vi "SO-FSRS Analysis 3.0.vi"() -> ()   [LabVIEW 2015]
uses:
  LabView vis/Control 1.ctl
  LabView vis/Control 3.ctl
  <vilib>/Math Plots/3D Math Plots/3D Surface/3D Surface XCtrl/3D Surface.xctl
  <vilib>/Math Plots/3D Math Plots/3D Scatter/3D Scatter XCtrl/3D Scatter.xctl
  <vilib>/gmath/NumericalOptimization/LM model function reference.ctl
  <vilib>/Utility/file.llb/Read Delimited Spreadsheet (DBL).vi
  <vilib>/Math Plots/3D Math Plots/3D Scatter/3D Scatter Datatype/Public/Plot Helper (Matrix).vi
  <vilib>/Math Plots/3D Math Plots/3D Surface/3D Surface Datatype/Public/Plot Helper (Vector).vi
  <vilib>/Utility/file.llb/Write Delimited Spreadsheet (DBL).vi
  <vilib>/gmath/NumericalOptimization/Nonlinear Curve Fit LM.vi
  <vilib>/Math Plots/3D Math Plots/3D Scatter/3D Scatter Datatype/Public/Plot Helper (Vector).vi
  <vilib>/Math Plots/3D Math Plots/3D Surface/3D Surface Datatype/3D Surface Datatype.lvclass
  <vilib>/Math Plots/3D Math Plots/3D Scatter/3D Scatter Datatype/3D Scatter Datatype.lvclass
  <vilib>/gmath/NI_Gmath.lvlib
  <vilib>/Analysis/NI_AALPro.lvlib
panel:
  out "Shiftx":T1=[-400.0, -600.0, -200.0, -2100.0, -10.0, 570.0, 1700.0, 980.0, 10000.0, -1100.0, 150.0, 320.0, -850.0, -1500.0, -5000.0]
  in  "Load shiftx":bool
  in  "error in":errorcluster
  out "error out":errorcluster
  in  "Main Tab":T2(tab)
  in  "Shorter Name":string
  in  "Do it?":bool
  in  "Index":i32
  in  "What you gonna do":u16(ring) items=["Delete", "Flip"]
  in  "Folder - Batch Files":path
  out "Built Arrays":dbl[][](graph)
  in  "?":bool
  in  "File Names":u16(ring) items=["pero_EGF1_h_0_0gr", "pero_EGF1_h_0_1gr", "pero_EGF1_h_0_2gr", "pero_EGF1_h_10_0gr", "pero_EGF1_h_10_1gr", "pero_EGF1_h_10_2gr", "pero_EGF1_h_11_0gr", "pero_EGF1_h_11_1gr", "pero_EGF1_h_11_2gr", "pero_EGF1_h_12_0gr", "pero_EGF1_h_12_1gr", "pero_EGF1_h_12_2gr", "pero_EGF1_h_13_0gr", "pero_EGF1_h_13_1gr", "pero_EGF1_h_13_2gr", "pero_EGF1_h_14_0gr", "pero_EGF1_h_14_1gr", "pero_EGF1_h_14_2gr", "pero_EGF1_h_15_0gr", "pero_EGF1_h_15_1gr", "pero_EGF1_h_15_2gr", "pero_EGF1_h_16_0gr", "pero_EGF1_h_16_1gr", "pero_EGF1_h_16_2gr", "pero_EGF1_h_17_0gr", "pero_EGF1_h_1_0gr", "pero_EGF1_h_1_1gr", "pero_EGF1_h_1_2gr", "pero_EGF1_h_2_0gr", "pero_EGF1_h_2_1gr", "pero_EGF1_h_2_2gr", "pero_EGF1_h_3_0gr", "pero_EGF1_h_3_1gr", "pero_EGF1_h_3_2gr", "pero_EGF1_h_4_0gr", "pero_EGF1_h_4_1gr", "pero_EGF1_h_4_2gr", "pero_EGF1_h_5_0gr", "pero_EGF1_h_5_1gr", "pero_EGF1_h_5_2gr", "pero_EGF1_h_6_0gr", "pero_EGF1_h_6_1gr", "pero_EGF1_h_6_2gr", "pero_EGF1_h_7_0gr", "pero_EGF1_h_7_1gr", "pero_EGF1_h_7_2gr", "pero_EGF1_h_8_0gr", "pero_EGF1_h_8_1gr", "pero_EGF1_h_8_2gr", "pero_EGF1_h_9_0gr", "pero_EGF1_h_9_1gr", "pero_EGF1_h_9_2gr", "pero_EGF1_h_m1m1_m0exe0", "pero_EGF1_h_m1m1_m0exe1", "pero_EGF1_h_m1m1_m0exe10", "pero_EGF1_h_m1m1_m0exe11", "pero_EGF1_h_m1m1_m0exe12", "pero_EGF1_h_m1m1_m0exe13", "pero_EGF1_h_m1m1_m0exe14", "pero_EGF1_h_m1m1_m0exe15", "pero_EGF1_h_m1m1_m0exe16", "pero_EGF1_h_m1m1_m0exe2", "pero_EGF1_h_m1m1_m0exe3", "pero_EGF1_h_m1m1_m0exe4", "pero_EGF1_h_m1m1_m0exe5", "pero_EGF1_h_m1m1_m0exe6", "pero_EGF1_h_m1m1_m0exe7", "pero_EGF1_h_m1m1_m0exe8", "pero_EGF1_h_m1m1_m0exe9", "pero_EGF1_h_m1m1_m100exe0", "pero_EGF1_h_m1m1_m100exe1", "pero_EGF1_h_m1m1_m100exe10", "pero_EGF1_h_m1m1_m100exe11", "pero_EGF1_h_m1m1_m100exe12", "pero_EGF1_h_m1m1_m100exe13", "pero_EGF1_h_m1m1_m100exe14", "pero_EGF1_h_m1m1_m100exe15", "pero_EGF1_h_m1m1_m100exe16", "pero_EGF1_h_m1m1_m100exe2", "pero_EGF1_h_m1m1_m100exe3", "pero_EGF1_h_m1m1_m100exe4", "pero_EGF1_h_m1m1_m100exe5", "pero_EGF1_h_m1m1_m100exe6", "pero_EGF1_h_m1m1_m100exe7", "pero_EGF1_h_m1m1_m100exe8", "pero_EGF1_h_m1m1_m100exe9", "pero_EGF1_h_m1m1_m200exe0", "pero_EGF1_h_m1m1_m200exe1", "pero_EGF1_h_m1m1_m200exe10", "pero_EGF1_h_m1m1_m200exe11", "pero_EGF1_h_m1m1_m200exe12", "pero_EGF1_h_m1m1_m200exe13", "pero_EGF1_h_m1m1_m200exe14", "pero_EGF1_h_m1m1_m200exe15", "pero_EGF1_h_m1m1_m200exe16", "pero_EGF1_h_m1m1_m200exe2", "pero_EGF1_h_m1m1_m200exe3", "pero_EGF1_h_m1m1_m200exe4", "pero_EGF1_h_m1m1_m200exe5", "pero_EGF1_h_m1m1_m200exe6", "pero_EGF1_h_m1m1_m200exe7", "pero_EGF1_h_m1m1_m200exe8", "pero_EGF1_h_m1m1_m200exe9", "pero_EGF1_h_m1m1_m300exe0", "pero_EGF1_h_m1m1_m300exe1", "pero_EGF1_h_m1m1_m300exe10", "pero_EGF1_h_m1m1_m300exe11", "pero_EGF1_h_m1m1_m300exe12", "pero_EGF1_h_m1m1_m300exe13", "pero_EGF1_h_m1m1_m300exe14", "pero_EGF1_h_m1m1_m300exe15", "pero_EGF1_h_m1m1_m300exe16", "pero_EGF1_h_m1m1_m300exe2", "pero_EGF1_h_m1m1_m300exe3", "pero_EGF1_h_m1m1_m300exe4", "pero_EGF1_h_m1m1_m300exe5", "pero_EGF1_h_m1m1_m300exe6", "pero_EGF1_h_m1m1_m300exe7", "pero_EGF1_h_m1m1_m300exe8", "pero_EGF1_h_m1m1_m300exe9", "pero_EGF1_h_m1m1_m5000exe0", "pero_EGF1_h_m1m1_m5000exe1", "pero_EGF1_h_m1m1_m5000exe10", "pero_EGF1_h_m1m1_m5000exe12", "pero_EGF1_h_m1m1_m5000exe13", "pero_EGF1_h_m1m1_m5000exe14", "pero_EGF1_h_m1m1_m5000exe15", "pero_EGF1_h_m1m1_m5000exe16", "pero_EGF1_h_m1m1_m5000exe2", "pero_EGF1_h_m1m1_m5000exe3", "pero_EGF1_h_m1m1_m5000exe4", "pero_EGF1_h_m1m1_m5000exe5", "pero_EGF1_h_m1m1_m5000exe6", "pero_EGF1_h_m1m1_m5000exe7", "pero_EGF1_h_m1m1_m5000exe8", "pero_EGF1_h_m1m1_m5000exe9", "pero_EGF1_h_m1m1_m500exe0", "pero_EGF1_h_m1m1_m500exe1", "pero_EGF1_h_m1m1_m500exe10", "pero_EGF1_h_m1m1_m500exe11", "pero_EGF1_h_m1m1_m500exe12", "pero_EGF1_h_m1m1_m500exe13", "pero_EGF1_h_m1m1_m500exe14", "pero_EGF1_h_m1m1_m500exe15", "pero_EGF1_h_m1m1_m500exe16", "pero_EGF1_h_m1m1_m500exe2", "pero_EGF1_h_m1m1_m500exe3", "pero_EGF1_h_m1m1_m500exe4", "pero_EGF1_h_m1m1_m500exe5", "pero_EGF1_h_m1m1_m500exe6", "pero_EGF1_h_m1m1_m500exe7", "pero_EGF1_h_m1m1_m500exe8", "pero_EGF1_h_m1m1_m500exe9", "pero_EGF1_h_m1m1_p100000exe0", "pero_EGF1_h_m1m1_p100000exe1", "pero_EGF1_h_m1m1_p100000exe10", "pero_EGF1_h_m1m1_p100000exe11", "pero_EGF1_h_m1m1_p100000exe12", "pero_EGF1_h_m1m1_p100000exe13", "pero_EGF1_h_m1m1_p100000exe14", "pero_EGF1_h_m1m1_p100000exe15", "pero_EGF1_h_m1m1_p100000exe16", "pero_EGF1_h_m1m1_p100000exe2", "pero_EGF1_h_m1m1_p100000exe3", "pero_EGF1_h_m1m1_p100000exe4", "pero_EGF1_h_m1m1_p100000exe5", "pero_EGF1_h_m1m1_p100000exe6", "pero_EGF1_h_m1m1_p100000exe7", "pero_EGF1_h_m1m1_p100000exe8", "pero_EGF1_h_m1m1_p100000exe9", "pero_EGF1_h_m1m1_p10000exe0", "pero_EGF1_h_m1m1_p10000exe1", "pero_EGF1_h_m1m1_p10000exe10", "pero_EGF1_h_m1m1_p10000exe11", "pero_EGF1_h_m1m1_p10000exe12", "pero_EGF1_h_m1m1_p10000exe13", "pero_EGF1_h_m1m1_p10000exe14", "pero_EGF1_h_m1m1_p10000exe15", "pero_EGF1_h_m1m1_p10000exe16", "pero_EGF1_h_m1m1_p10000exe2", "pero_EGF1_h_m1m1_p10000exe3", "pero_EGF1_h_m1m1_p10000exe4", "pero_EGF1_h_m1m1_p10000exe5", "pero_EGF1_h_m1m1_p10000exe6", "pero_EGF1_h_m1m1_p10000exe7", "pero_EGF1_h_m1m1_p10000exe8", "pero_EGF1_h_m1m1_p10000exe9", "pero_EGF1_h_m1m1_p1000exe0", "pero_EGF1_h_m1m1_p1000exe1", "pero_EGF1_h_m1m1_p1000exe10", "pero_EGF1_h_m1m1_p1000exe11", "pero_EGF1_h_m1m1_p1000exe12", "pero_EGF1_h_m1m1_p1000exe13", "pero_EGF1_h_m1m1_p1000exe14", "pero_EGF1_h_m1m1_p1000exe15", "pero_EGF1_h_m1m1_p1000exe16", "pero_EGF1_h_m1m1_p1000exe17", "pero_EGF1_h_m1m1_p1000exe2", "pero_EGF1_h_m1m1_p1000exe3", "pero_EGF1_h_m1m1_p1000exe4", "pero_EGF1_h_m1m1_p1000exe5", "pero_EGF1_h_m1m1_p1000exe6", "pero_EGF1_h_m1m1_p1000exe7", "pero_EGF1_h_m1m1_p1000exe8", "pero_EGF1_h_m1m1_p1000exe9", "pero_EGF1_h_m1m1_p100exe0", "pero_EGF1_h_m1m1_p100exe1", "pero_EGF1_h_m1m1_p100exe10", "pero_EGF1_h_m1m1_p100exe11", "pero_EGF1_h_m1m1_p100exe12", "pero_EGF1_h_m1m1_p100exe13", "pero_EGF1_h_m1m1_p100exe14", "pero_EGF1_h_m1m1_p100exe15", "pero_EGF1_h_m1m1_p100exe16", "pero_EGF1_h_m1m1_p100exe2", "pero_EGF1_h_m1m1_p100exe3", "pero_EGF1_h_m1m1_p100exe4", "pero_EGF1_h_m1m1_p100exe5", "pero_EGF1_h_m1m1_p100exe6", "pero_EGF1_h_m1m1_p100exe7", "pero_EGF1_h_m1m1_p100exe8", "pero_EGF1_h_m1m1_p100exe9", "pero_EGF1_h_m1m1_p1100exe0", "pero_EGF1_h_m1m1_p1100exe1", "pero_EGF1_h_m1m1_p1100exe10", "pero_EGF1_h_m1m1_p1100exe11", "pero_EGF1_h_m1m1_p1100exe12", "pero_EGF1_h_m1m1_p1100exe13", "pero_EGF1_h_m1m1_p1100exe14", "pero_EGF1_h_m1m1_p1100exe15", "pero_EGF1_h_m1m1_p1100exe16", "pero_EGF1_h_m1m1_p1100exe2", "pero_EGF1_h_m1m1_p1100exe3", "pero_EGF1_h_m1m1_p1100exe4", "pero_EGF1_h_m1m1_p1100exe5", "pero_EGF1_h_m1m1_p1100exe6", "pero_EGF1_h_m1m1_p1100exe7", "pero_EGF1_h_m1m1_p1100exe8", "pero_EGF1_h_m1m1_p1100exe9", "pero_EGF1_h_m1m1_p120000exe0", "pero_EGF1_h_m1m1_p120000exe1", "pero_EGF1_h_m1m1_p120000exe10", "pero_EGF1_h_m1m1_p120000exe11", "pero_EGF1_h_m1m1_p120000exe12", "pero_EGF1_h_m1m1_p120000exe13", "pero_EGF1_h_m1m1_p120000exe14", "pero_EGF1_h_m1m1_p120000exe15", "pero_EGF1_h_m1m1_p120000exe16", "pero_EGF1_h_m1m1_p120000exe2", "pero_EGF1_h_m1m1_p120000exe3", "pero_EGF1_h_m1m1_p120000exe4", "pero_EGF1_h_m1m1_p120000exe5", "pero_EGF1_h_m1m1_p120000exe6", "pero_EGF1_h_m1m1_p120000exe7", "pero_EGF1_h_m1m1_p120000exe8", "pero_EGF1_h_m1m1_p120000exe9", "pero_EGF1_h_m1m1_p1200exe0", "pero_EGF1_h_m1m1_p1200exe1", "pero_EGF1_h_m1m1_p1200exe10", "pero_EGF1_h_m1m1_p1200exe11", "pero_EGF1_h_m1m1_p1200exe12", "pero_EGF1_h_m1m1_p1200exe13", "pero_EGF1_h_m1m1_p1200exe14", "pero_EGF1_h_m1m1_p1200exe15", "pero_EGF1_h_m1m1_p1200exe16", "pero_EGF1_h_m1m1_p1200exe2", "pero_EGF1_h_m1m1_p1200exe3", "pero_EGF1_h_m1m1_p1200exe4", "pero_EGF1_h_m1m1_p1200exe5", "pero_EGF1_h_m1m1_p1200exe6", "pero_EGF1_h_m1m1_p1200exe7", "pero_EGF1_h_m1m1_p1200exe8", "pero_EGF1_h_m1m1_p1200exe9", "pero_EGF1_h_m1m1_p1300exe0", "pero_EGF1_h_m1m1_p1300exe1", "pero_EGF1_h_m1m1_p1300exe10", "pero_EGF1_h_m1m1_p1300exe11", "pero_EGF1_h_m1m1_p1300exe12", "pero_EGF1_h_m1m1_p1300exe13", "pero_EGF1_h_m1m1_p1300exe14", "pero_EGF1_h_m1m1_p1300exe15", "pero_EGF1_h_m1m1_p1300exe16", "pero_EGF1_h_m1m1_p1300exe2", "pero_EGF1_h_m1m1_p1300exe3", "pero_EGF1_h_m1m1_p1300exe4", "pero_EGF1_h_m1m1_p1300exe5", "pero_EGF1_h_m1m1_p1300exe6", "pero_EGF1_h_m1m1_p1300exe7", "pero_EGF1_h_m1m1_p1300exe8", "pero_EGF1_h_m1m1_p1300exe9", "pero_EGF1_h_m1m1_p140000exe0", "pero_EGF1_h_m1m1_p140000exe1", "pero_EGF1_h_m1m1_p140000exe10", "pero_EGF1_h_m1m1_p140000exe11", "pero_EGF1_h_m1m1_p140000exe12", "pero_EGF1_h_m1m1_p140000exe13", "pero_EGF1_h_m1m1_p140000exe14", "pero_EGF1_h_m1m1_p140000exe15", "pero_EGF1_h_m1m1_p140000exe16", "pero_EGF1_h_m1m1_p140000exe2", "pero_EGF1_h_m1m1_p140000exe3", "pero_EGF1_h_m1m1_p140000exe4", "pero_EGF1_h_m1m1_p140000exe5", "pero_EGF1_h_m1m1_p140000exe6", "pero_EGF1_h_m1m1_p140000exe7", "pero_EGF1_h_m1m1_p140000exe8", "pero_EGF1_h_m1m1_p140000exe9", "pero_EGF1_h_m1m1_p1400exe0", "pero_EGF1_h_m1m1_p1400exe1", "pero_EGF1_h_m1m1_p1400exe10", "pero_EGF1_h_m1m1_p1400exe11", "pero_EGF1_h_m1m1_p1400exe12", "pero_EGF1_h_m1m1_p1400exe13", "pero_EGF1_h_m1m1_p1400exe14", "pero_EGF1_h_m1m1_p1400exe15", "pero_EGF1_h_m1m1_p1400exe16", "pero_EGF1_h_m1m1_p1400exe2", "pero_EGF1_h_m1m1_p1400exe3", "pero_EGF1_h_m1m1_p1400exe4", "pero_EGF1_h_m1m1_p1400exe5", "pero_EGF1_h_m1m1_p1400exe6", "pero_EGF1_h_m1m1_p1400exe7", "pero_EGF1_h_m1m1_p1400exe8", "pero_EGF1_h_m1m1_p1400exe9", "pero_EGF1_h_m1m1_p1500exe0", "pero_EGF1_h_m1m1_p1500exe1", "pero_EGF1_h_m1m1_p1500exe10", "pero_EGF1_h_m1m1_p1500exe11", "pero_EGF1_h_m1m1_p1500exe12", "pero_EGF1_h_m1m1_p1500exe13", "pero_EGF1_h_m1m1_p1500exe14", "pero_EGF1_h_m1m1_p1500exe15", "pero_EGF1_h_m1m1_p1500exe16", "pero_EGF1_h_m1m1_p1500exe2", "pero_EGF1_h_m1m1_p1500exe3", "pero_EGF1_h_m1m1_p1500exe4", "pero_EGF1_h_m1m1_p1500exe5", "pero_EGF1_h_m1m1_p1500exe6", "pero_EGF1_h_m1m1_p1500exe7", "pero_EGF1_h_m1m1_p1500exe8", "pero_EGF1_h_m1m1_p1500exe9", "pero_EGF1_h_m1m1_p160000exe0", "pero_EGF1_h_m1m1_p160000exe1", "pero_EGF1_h_m1m1_p160000exe10", "pero_EGF1_h_m1m1_p160000exe11", "pero_EGF1_h_m1m1_p160000exe12", "pero_EGF1_h_m1m1_p160000exe13", "pero_EGF1_h_m1m1_p160000exe14", "pero_EGF1_h_m1m1_p160000exe15", "pero_EGF1_h_m1m1_p160000exe16", "pero_EGF1_h_m1m1_p160000exe2", "pero_EGF1_h_m1m1_p160000exe3", "pero_EGF1_h_m1m1_p160000exe4", "pero_EGF1_h_m1m1_p160000exe5", "pero_EGF1_h_m1m1_p160000exe6", "pero_EGF1_h_m1m1_p160000exe7", "pero_EGF1_h_m1m1_p160000exe8", "pero_EGF1_h_m1m1_p160000exe9", "pero_EGF1_h_m1m1_p1600exe0", "pero_EGF1_h_m1m1_p1600exe1", "pero_EGF1_h_m1m1_p1600exe10", "pero_EGF1_h_m1m1_p1600exe11", "pero_EGF1_h_m1m1_p1600exe12", "pero_EGF1_h_m1m1_p1600exe13", "pero_EGF1_h_m1m1_p1600exe14", "pero_EGF1_h_m1m1_p1600exe15", "pero_EGF1_h_m1m1_p1600exe16", "pero_EGF1_h_m1m1_p1600exe2", "pero_EGF1_h_m1m1_p1600exe3", "pero_EGF1_h_m1m1_p1600exe4", "pero_EGF1_h_m1m1_p1600exe5", "pero_EGF1_h_m1m1_p1600exe6", "pero_EGF1_h_m1m1_p1600exe7", "pero_EGF1_h_m1m1_p1600exe8", "pero_EGF1_h_m1m1_p1600exe9", "pero_EGF1_h_m1m1_p1700exe0", "pero_EGF1_h_m1m1_p1700exe1", "pero_EGF1_h_m1m1_p1700exe10", "pero_EGF1_h_m1m1_p1700exe11", "pero_EGF1_h_m1m1_p1700exe12", "pero_EGF1_h_m1m1_p1700exe13", "pero_EGF1_h_m1m1_p1700exe14", "pero_EGF1_h_m1m1_p1700exe15", "pero_EGF1_h_m1m1_p1700exe16", "pero_EGF1_h_m1m1_p1700exe2", "pero_EGF1_h_m1m1_p1700exe3", "pero_EGF1_h_m1m1_p1700exe4", "pero_EGF1_h_m1m1_p1700exe5", "pero_EGF1_h_m1m1_p1700exe6", "pero_EGF1_h_m1m1_p1700exe7", "pero_EGF1_h_m1m1_p1700exe8", "pero_EGF1_h_m1m1_p1700exe9", "pero_EGF1_h_m1m1_p180000exe0", "pero_EGF1_h_m1m1_p180000exe1", "pero_EGF1_h_m1m1_p180000exe10", "pero_EGF1_h_m1m1_p180000exe11", "pero_EGF1_h_m1m1_p180000exe12", "pero_EGF1_h_m1m1_p180000exe13", "pero_EGF1_h_m1m1_p180000exe14", "pero_EGF1_h_m1m1_p180000exe15", "pero_EGF1_h_m1m1_p180000exe16", "pero_EGF1_h_m1m1_p180000exe2", "pero_EGF1_h_m1m1_p180000exe3", "pero_EGF1_h_m1m1_p180000exe4", "pero_EGF1_h_m1m1_p180000exe5", "pero_EGF1_h_m1m1_p180000exe6", "pero_EGF1_h_m1m1_p180000exe7", "pero_EGF1_h_m1m1_p180000exe8", "pero_EGF1_h_m1m1_p180000exe9", "pero_EGF1_h_m1m1_p1800exe0", "pero_EGF1_h_m1m1_p1800exe1", "pero_EGF1_h_m1m1_p1800exe10", "pero_EGF1_h_m1m1_p1800exe11", "pero_EGF1_h_m1m1_p1800exe12", "pero_EGF1_h_m1m1_p1800exe13", "pero_EGF1_h_m1m1_p1800exe14", "pero_EGF1_h_m1m1_p1800exe15", "pero_EGF1_h_m1m1_p1800exe16", "pero_EGF1_h_m1m1_p1800exe2", "pero_EGF1_h_m1m1_p1800exe3", "pero_EGF1_h_m1m1_p1800exe4", "pero_EGF1_h_m1m1_p1800exe5", "pero_EGF1_h_m1m1_p1800exe6", "pero_EGF1_h_m1m1_p1800exe7", "pero_EGF1_h_m1m1_p1800exe8", "pero_EGF1_h_m1m1_p1800exe9", "pero_EGF1_h_m1m1_p1900exe0", "pero_EGF1_h_m1m1_p1900exe1", "pero_EGF1_h_m1m1_p1900exe10", "pero_EGF1_h_m1m1_p1900exe11", "pero_EGF1_h_m1m1_p1900exe12", "pero_EGF1_h_m1m1_p1900exe13", "pero_EGF1_h_m1m1_p1900exe14", "pero_EGF1_h_m1m1_p1900exe15", "pero_EGF1_h_m1m1_p1900exe16", "pero_EGF1_h_m1m1_p1900exe17", "pero_EGF1_h_m1m1_p1900exe2", "pero_EGF1_h_m1m1_p1900exe3", "pero_EGF1_h_m1m1_p1900exe4", "pero_EGF1_h_m1m1_p1900exe5", "pero_EGF1_h_m1m1_p1900exe6", "pero_EGF1_h_m1m1_p1900exe7", "pero_EGF1_h_m1m1_p1900exe8", "pero_EGF1_h_m1m1_p1900exe9", "pero_EGF1_h_m1m1_p200000exe0", "pero_EGF1_h_m1m1_p200000exe1", "pero_EGF1_h_m1m1_p200000exe10", "pero_EGF1_h_m1m1_p200000exe11", "pero_EGF1_h_m1m1_p200000exe12", "pero_EGF1_h_m1m1_p200000exe13", "pero_EGF1_h_m1m1_p200000exe14", "pero_EGF1_h_m1m1_p200000exe15", "pero_EGF1_h_m1m1_p200000exe16", "pero_EGF1_h_m1m1_p200000exe2", "pero_EGF1_h_m1m1_p200000exe3", "pero_EGF1_h_m1m1_p200000exe4", "pero_EGF1_h_m1m1_p200000exe5", "pero_EGF1_h_m1m1_p200000exe6", "pero_EGF1_h_m1m1_p200000exe7", "pero_EGF1_h_m1m1_p200000exe8", "pero_EGF1_h_m1m1_p200000exe9", "pero_EGF1_h_m1m1_p20000exe0", "pero_EGF1_h_m1m1_p20000exe1", "pero_EGF1_h_m1m1_p20000exe10", "pero_EGF1_h_m1m1_p20000exe11", "pero_EGF1_h_m1m1_p20000exe12", "pero_EGF1_h_m1m1_p20000exe13", "pero_EGF1_h_m1m1_p20000exe14", "pero_EGF1_h_m1m1_p20000exe15", "pero_EGF1_h_m1m1_p20000exe16", "pero_EGF1_h_m1m1_p20000exe2", "pero_EGF1_h_m1m1_p20000exe3", "pero_EGF1_h_m1m1_p20000exe4", "pero_EGF1_h_m1m1_p20000exe5", "pero_EGF1_h_m1m1_p20000exe6", "pero_EGF1_h_m1m1_p20000exe7", "pero_EGF1_h_m1m1_p20000exe8", "pero_EGF1_h_m1m1_p20000exe9", "pero_EGF1_h_m1m1_p2000exe0", "pero_EGF1_h_m1m1_p2000exe1", "pero_EGF1_h_m1m1_p2000exe10", "pero_EGF1_h_m1m1_p2000exe11", "pero_EGF1_h_m1m1_p2000exe12", "pero_EGF1_h_m1m1_p2000exe13", "pero_EGF1_h_m1m1_p2000exe14", "pero_EGF1_h_m1m1_p2000exe15", "pero_EGF1_h_m1m1_p2000exe16", "pero_EGF1_h_m1m1_p2000exe2", "pero_EGF1_h_m1m1_p2000exe3", "pero_EGF1_h_m1m1_p2000exe4", "pero_EGF1_h_m1m1_p2000exe5", "pero_EGF1_h_m1m1_p2000exe6", "pero_EGF1_h_m1m1_p2000exe7", "pero_EGF1_h_m1m1_p2000exe8", "pero_EGF1_h_m1m1_p2000exe9", "pero_EGF1_h_m1m1_p200exe0", "pero_EGF1_h_m1m1_p200exe1", "pero_EGF1_h_m1m1_p200exe10", "pero_EGF1_h_m1m1_p200exe11", "pero_EGF1_h_m1m1_p200exe12", "pero_EGF1_h_m1m1_p200exe13", "pero_EGF1_h_m1m1_p200exe14", "pero_EGF1_h_m1m1_p200exe15", "pero_EGF1_h_m1m1_p200exe16", "pero_EGF1_h_m1m1_p200exe2", "pero_EGF1_h_m1m1_p200exe3", "pero_EGF1_h_m1m1_p200exe4", "pero_EGF1_h_m1m1_p200exe5", "pero_EGF1_h_m1m1_p200exe6", "pero_EGF1_h_m1m1_p200exe7", "pero_EGF1_h_m1m1_p200exe8", "pero_EGF1_h_m1m1_p200exe9", "pero_EGF1_h_m1m1_p2100exe0", "pero_EGF1_h_m1m1_p2100exe1", "pero_EGF1_h_m1m1_p2100exe10", "pero_EGF1_h_m1m1_p2100exe11", "pero_EGF1_h_m1m1_p2100exe12", "pero_EGF1_h_m1m1_p2100exe13", "pero_EGF1_h_m1m1_p2100exe14", "pero_EGF1_h_m1m1_p2100exe15", "pero_EGF1_h_m1m1_p2100exe16", "pero_EGF1_h_m1m1_p2100exe2", "pero_EGF1_h_m1m1_p2100exe3", "pero_EGF1_h_m1m1_p2100exe4", "pero_EGF1_h_m1m1_p2100exe5", "pero_EGF1_h_m1m1_p2100exe6", "pero_EGF1_h_m1m1_p2100exe7", "pero_EGF1_h_m1m1_p2100exe8", "pero_EGF1_h_m1m1_p2100exe9", "pero_EGF1_h_m1m1_p220000exe0", "pero_EGF1_h_m1m1_p220000exe1", "pero_EGF1_h_m1m1_p220000exe10", "pero_EGF1_h_m1m1_p220000exe11", "pero_EGF1_h_m1m1_p220000exe12", "pero_EGF1_h_m1m1_p220000exe13", "pero_EGF1_h_m1m1_p220000exe14", "pero_EGF1_h_m1m1_p220000exe15", "pero_EGF1_h_m1m1_p220000exe16", "pero_EGF1_h_m1m1_p220000exe2", "pero_EGF1_h_m1m1_p220000exe3", "pero_EGF1_h_m1m1_p220000exe4", "pero_EGF1_h_m1m1_p220000exe5", "pero_EGF1_h_m1m1_p220000exe6", "pero_EGF1_h_m1m1_p220000exe7", "pero_EGF1_h_m1m1_p220000exe8", "pero_EGF1_h_m1m1_p220000exe9", "pero_EGF1_h_m1m1_p2200exe0", "pero_EGF1_h_m1m1_p2200exe1", "pero_EGF1_h_m1m1_p2200exe10", "pero_EGF1_h_m1m1_p2200exe11", "pero_EGF1_h_m1m1_p2200exe12", "pero_EGF1_h_m1m1_p2200exe13", "pero_EGF1_h_m1m1_p2200exe14", "pero_EGF1_h_m1m1_p2200exe15", "pero_EGF1_h_m1m1_p2200exe16", "pero_EGF1_h_m1m1_p2200exe2", "pero_EGF1_h_m1m1_p2200exe3", "pero_EGF1_h_m1m1_p2200exe4", "pero_EGF1_h_m1m1_p2200exe5", "pero_EGF1_h_m1m1_p2200exe6", "pero_EGF1_h_m1m1_p2200exe7", "pero_EGF1_h_m1m1_p2200exe8", "pero_EGF1_h_m1m1_p2200exe9", "pero_EGF1_h_m1m1_p2300exe0", "pero_EGF1_h_m1m1_p2300exe1", "pero_EGF1_h_m1m1_p2300exe10", "pero_EGF1_h_m1m1_p2300exe11", "pero_EGF1_h_m1m1_p2300exe12", "pero_EGF1_h_m1m1_p2300exe13", "pero_EGF1_h_m1m1_p2300exe14", "pero_EGF1_h_m1m1_p2300exe15", "pero_EGF1_h_m1m1_p2300exe16", "pero_EGF1_h_m1m1_p2300exe17", "pero_EGF1_h_m1m1_p2300exe2", "pero_EGF1_h_m1m1_p2300exe3", "pero_EGF1_h_m1m1_p2300exe4", "pero_EGF1_h_m1m1_p2300exe5", "pero_EGF1_h_m1m1_p2300exe6", "pero_EGF1_h_m1m1_p2300exe7", "pero_EGF1_h_m1m1_p2300exe8", "pero_EGF1_h_m1m1_p2300exe9", "pero_EGF1_h_m1m1_p240000exe0", "pero_EGF1_h_m1m1_p240000exe1", "pero_EGF1_h_m1m1_p240000exe10", "pero_EGF1_h_m1m1_p240000exe11", "pero_EGF1_h_m1m1_p240000exe12", "pero_EGF1_h_m1m1_p240000exe13", "pero_EGF1_h_m1m1_p240000exe14", "pero_EGF1_h_m1m1_p240000exe15", "pero_EGF1_h_m1m1_p240000exe16", "pero_EGF1_h_m1m1_p240000exe2", "pero_EGF1_h_m1m1_p240000exe3", "pero_EGF1_h_m1m1_p240000exe4", "pero_EGF1_h_m1m1_p240000exe5", "pero_EGF1_h_m1m1_p240000exe6", "pero_EGF1_h_m1m1_p240000exe7", "pero_EGF1_h_m1m1_p240000exe8", "pero_EGF1_h_m1m1_p240000exe9", "pero_EGF1_h_m1m1_p2400exe0", "pero_EGF1_h_m1m1_p2400exe1", "pero_EGF1_h_m1m1_p2400exe10", "pero_EGF1_h_m1m1_p2400exe11", "pero_EGF1_h_m1m1_p2400exe12", "pero_EGF1_h_m1m1_p2400exe13", "pero_EGF1_h_m1m1_p2400exe14", "pero_EGF1_h_m1m1_p2400exe15", "pero_EGF1_h_m1m1_p2400exe16", "pero_EGF1_h_m1m1_p2400exe2", "pero_EGF1_h_m1m1_p2400exe3", "pero_EGF1_h_m1m1_p2400exe4", "pero_EGF1_h_m1m1_p2400exe5", "pero_EGF1_h_m1m1_p2400exe6", "pero_EGF1_h_m1m1_p2400exe7", "pero_EGF1_h_m1m1_p2400exe8", "pero_EGF1_h_m1m1_p2400exe9", "pero_EGF1_h_m1m1_p2500exe0", "pero_EGF1_h_m1m1_p2500exe1", "pero_EGF1_h_m1m1_p2500exe10", "pero_EGF1_h_m1m1_p2500exe11", "pero_EGF1_h_m1m1_p2500exe12", "pero_EGF1_h_m1m1_p2500exe13", "pero_EGF1_h_m1m1_p2500exe14", "pero_EGF1_h_m1m1_p2500exe15", "pero_EGF1_h_m1m1_p2500exe16", "pero_EGF1_h_m1m1_p2500exe2", "pero_EGF1_h_m1m1_p2500exe3", "pero_EGF1_h_m1m1_p2500exe4", "pero_EGF1_h_m1m1_p2500exe5", "pero_EGF1_h_m1m1_p2500exe6", "pero_EGF1_h_m1m1_p2500exe7", "pero_EGF1_h_m1m1_p2500exe8", "pero_EGF1_h_m1m1_p2500exe9", "pero_EGF1_h_m1m1_p260000exe0", "pero_EGF1_h_m1m1_p260000exe1", "pero_EGF1_h_m1m1_p260000exe10", "pero_EGF1_h_m1m1_p260000exe11", "pero_EGF1_h_m1m1_p260000exe12", "pero_EGF1_h_m1m1_p260000exe13", "pero_EGF1_h_m1m1_p260000exe14", "pero_EGF1_h_m1m1_p260000exe15", "pero_EGF1_h_m1m1_p260000exe16", "pero_EGF1_h_m1m1_p260000exe2", "pero_EGF1_h_m1m1_p260000exe3", "pero_EGF1_h_m1m1_p260000exe4", "pero_EGF1_h_m1m1_p260000exe5", "pero_EGF1_h_m1m1_p260000exe6", "pero_EGF1_h_m1m1_p260000exe7", "pero_EGF1_h_m1m1_p260000exe8", "pero_EGF1_h_m1m1_p260000exe9", "pero_EGF1_h_m1m1_p2600exe0", "pero_EGF1_h_m1m1_p2600exe1", "pero_EGF1_h_m1m1_p2600exe10", "pero_EGF1_h_m1m1_p2600exe11", "pero_EGF1_h_m1m1_p2600exe12", "pero_EGF1_h_m1m1_p2600exe13", "pero_EGF1_h_m1m1_p2600exe14", "pero_EGF1_h_m1m1_p2600exe15", "pero_EGF1_h_m1m1_p2600exe16", "pero_EGF1_h_m1m1_p2600exe2", "pero_EGF1_h_m1m1_p2600exe3", "pero_EGF1_h_m1m1_p2600exe4", "pero_EGF1_h_m1m1_p2600exe5", "pero_EGF1_h_m1m1_p2600exe6", "pero_EGF1_h_m1m1_p2600exe7", "pero_EGF1_h_m1m1_p2600exe8", "pero_EGF1_h_m1m1_p2600exe9", "pero_EGF1_h_m1m1_p2700exe0", "pero_EGF1_h_m1m1_p2700exe1", "pero_EGF1_h_m1m1_p2700exe10", "pero_EGF1_h_m1m1_p2700exe11", "pero_EGF1_h_m1m1_p2700exe12", "pero_EGF1_h_m1m1_p2700exe13", "pero_EGF1_h_m1m1_p2700exe14", "pero_EGF1_h_m1m1_p2700exe15", "pero_EGF1_h_m1m1_p2700exe16", "pero_EGF1_h_m1m1_p2700exe2", "pero_EGF1_h_m1m1_p2700exe3", "pero_EGF1_h_m1m1_p2700exe4", "pero_EGF1_h_m1m1_p2700exe5", "pero_EGF1_h_m1m1_p2700exe6", "pero_EGF1_h_m1m1_p2700exe7", "pero_EGF1_h_m1m1_p2700exe8", "pero_EGF1_h_m1m1_p2700exe9", "pero_EGF1_h_m1m1_p280000exe0", "pero_EGF1_h_m1m1_p280000exe1", "pero_EGF1_h_m1m1_p280000exe10", "pero_EGF1_h_m1m1_p280000exe11", "pero_EGF1_h_m1m1_p280000exe12", "pero_EGF1_h_m1m1_p280000exe13", "pero_EGF1_h_m1m1_p280000exe14", "pero_EGF1_h_m1m1_p280000exe15", "pero_EGF1_h_m1m1_p280000exe16", "pero_EGF1_h_m1m1_p280000exe2", "pero_EGF1_h_m1m1_p280000exe3", "pero_EGF1_h_m1m1_p280000exe4", "pero_EGF1_h_m1m1_p280000exe5", "pero_EGF1_h_m1m1_p280000exe6", "pero_EGF1_h_m1m1_p280000exe7", "pero_EGF1_h_m1m1_p280000exe8", "pero_EGF1_h_m1m1_p280000exe9", "pero_EGF1_h_m1m1_p2800exe0", "pero_EGF1_h_m1m1_p2800exe1", "pero_EGF1_h_m1m1_p2800exe10", "pero_EGF1_h_m1m1_p2800exe11", "pero_EGF1_h_m1m1_p2800exe12", "pero_EGF1_h_m1m1_p2800exe13", "pero_EGF1_h_m1m1_p2800exe14", "pero_EGF1_h_m1m1_p2800exe15", "pero_EGF1_h_m1m1_p2800exe16", "pero_EGF1_h_m1m1_p2800exe2", "pero_EGF1_h_m1m1_p2800exe3", "pero_EGF1_h_m1m1_p2800exe4", "pero_EGF1_h_m1m1_p2800exe5", "pero_EGF1_h_m1m1_p2800exe6", "pero_EGF1_h_m1m1_p2800exe7", "pero_EGF1_h_m1m1_p2800exe8", "pero_EGF1_h_m1m1_p2800exe9", "pero_EGF1_h_m1m1_p2900exe0", "pero_EGF1_h_m1m1_p2900exe1", "pero_EGF1_h_m1m1_p2900exe10", "pero_EGF1_h_m1m1_p2900exe11", "pero_EGF1_h_m1m1_p2900exe12", "pero_EGF1_h_m1m1_p2900exe13", "pero_EGF1_h_m1m1_p2900exe14", "pero_EGF1_h_m1m1_p2900exe15", "pero_EGF1_h_m1m1_p2900exe16", "pero_EGF1_h_m1m1_p2900exe2", "pero_EGF1_h_m1m1_p2900exe3", "pero_EGF1_h_m1m1_p2900exe4", "pero_EGF1_h_m1m1_p2900exe5", "pero_EGF1_h_m1m1_p2900exe6", "pero_EGF1_h_m1m1_p2900exe7", "pero_EGF1_h_m1m1_p2900exe8", "pero_EGF1_h_m1m1_p2900exe9", "pero_EGF1_h_m1m1_p300000exe0", "pero_EGF1_h_m1m1_p300000exe1", "pero_EGF1_h_m1m1_p300000exe10", "pero_EGF1_h_m1m1_p300000exe11", "pero_EGF1_h_m1m1_p300000exe12", "pero_EGF1_h_m1m1_p300000exe13", "pero_EGF1_h_m1m1_p300000exe14", "pero_EGF1_h_m1m1_p300000exe15", "pero_EGF1_h_m1m1_p300000exe16", "pero_EGF1_h_m1m1_p300000exe2", "pero_EGF1_h_m1m1_p300000exe3", "pero_EGF1_h_m1m1_p300000exe4", "pero_EGF1_h_m1m1_p300000exe5", "pero_EGF1_h_m1m1_p300000exe6", "pero_EGF1_h_m1m1_p300000exe7", "pero_EGF1_h_m1m1_p300000exe8", "pero_EGF1_h_m1m1_p300000exe9", "pero_EGF1_h_m1m1_p30000exe0", "pero_EGF1_h_m1m1_p30000exe1", "pero_EGF1_h_m1m1_p30000exe10", "pero_EGF1_h_m1m1_p30000exe11", "pero_EGF1_h_m1m1_p30000exe12", "pero_EGF1_h_m1m1_p30000exe13", "pero_EGF1_h_m1m1_p30000exe14", "pero_EGF1_h_m1m1_p30000exe15", "pero_EGF1_h_m1m1_p30000exe16", "pero_EGF1_h_m1m1_p30000exe2", "pero_EGF1_h_m1m1_p30000exe3", "pero_EGF1_h_m1m1_p30000exe4", "pero_EGF1_h_m1m1_p30000exe5", "pero_EGF1_h_m1m1_p30000exe6", "pero_EGF1_h_m1m1_p30000exe7", "pero_EGF1_h_m1m1_p30000exe8", "pero_EGF1_h_m1m1_p30000exe9", "pero_EGF1_h_m1m1_p3000exe0", "pero_EGF1_h_m1m1_p3000exe1", "pero_EGF1_h_m1m1_p3000exe10", "pero_EGF1_h_m1m1_p3000exe11", "pero_EGF1_h_m1m1_p3000exe12", "pero_EGF1_h_m1m1_p3000exe13", "pero_EGF1_h_m1m1_p3000exe14", "pero_EGF1_h_m1m1_p3000exe15", "pero_EGF1_h_m1m1_p3000exe16", "pero_EGF1_h_m1m1_p3000exe17", "pero_EGF1_h_m1m1_p3000exe2", "pero_EGF1_h_m1m1_p3000exe3", "pero_EGF1_h_m1m1_p3000exe4", "pero_EGF1_h_m1m1_p3000exe5", "pero_EGF1_h_m1m1_p3000exe6", "pero_EGF1_h_m1m1_p3000exe7", "pero_EGF1_h_m1m1_p3000exe8", "pero_EGF1_h_m1m1_p3000exe9", "pero_EGF1_h_m1m1_p300exe0", "pero_EGF1_h_m1m1_p300exe1", "pero_EGF1_h_m1m1_p300exe10", "pero_EGF1_h_m1m1_p300exe11", "pero_EGF1_h_m1m1_p300exe12", "pero_EGF1_h_m1m1_p300exe13", "pero_EGF1_h_m1m1_p300exe14", "pero_EGF1_h_m1m1_p300exe15", "pero_EGF1_h_m1m1_p300exe16", "pero_EGF1_h_m1m1_p300exe2", "pero_EGF1_h_m1m1_p300exe3", "pero_EGF1_h_m1m1_p300exe4", "pero_EGF1_h_m1m1_p300exe5", "pero_EGF1_h_m1m1_p300exe6", "pero_EGF1_h_m1m1_p300exe7", "pero_EGF1_h_m1m1_p300exe8", "pero_EGF1_h_m1m1_p300exe9", "pero_EGF1_h_m1m1_p320000exe0", "pero_EGF1_h_m1m1_p320000exe1", "pero_EGF1_h_m1m1_p320000exe10", "pero_EGF1_h_m1m1_p320000exe11", "pero_EGF1_h_m1m1_p320000exe12", "pero_EGF1_h_m1m1_p320000exe13", "pero_EGF1_h_m1m1_p320000exe14", "pero_EGF1_h_m1m1_p320000exe15", "pero_EGF1_h_m1m1_p320000exe16", "pero_EGF1_h_m1m1_p320000exe2", "pero_EGF1_h_m1m1_p320000exe3", "pero_EGF1_h_m1m1_p320000exe4", "pero_EGF1_h_m1m1_p320000exe5", "pero_EGF1_h_m1m1_p320000exe6", "pero_EGF1_h_m1m1_p320000exe7", "pero_EGF1_h_m1m1_p320000exe8", "pero_EGF1_h_m1m1_p320000exe9", "pero_EGF1_h_m1m1_p340000exe0", "pero_EGF1_h_m1m1_p340000exe1", "pero_EGF1_h_m1m1_p340000exe10", "pero_EGF1_h_m1m1_p340000exe11", "pero_EGF1_h_m1m1_p340000exe12", "pero_EGF1_h_m1m1_p340000exe13", "pero_EGF1_h_m1m1_p340000exe14", "pero_EGF1_h_m1m1_p340000exe15", "pero_EGF1_h_m1m1_p340000exe16", "pero_EGF1_h_m1m1_p340000exe2", "pero_EGF1_h_m1m1_p340000exe3", "pero_EGF1_h_m1m1_p340000exe4", "pero_EGF1_h_m1m1_p340000exe5", "pero_EGF1_h_m1m1_p340000exe6", "pero_EGF1_h_m1m1_p340000exe7", "pero_EGF1_h_m1m1_p340000exe8", "pero_EGF1_h_m1m1_p340000exe9", "pero_EGF1_h_m1m1_p360000exe0", "pero_EGF1_h_m1m1_p360000exe1", "pero_EGF1_h_m1m1_p360000exe10", "pero_EGF1_h_m1m1_p360000exe11", "pero_EGF1_h_m1m1_p360000exe12", "pero_EGF1_h_m1m1_p360000exe13", "pero_EGF1_h_m1m1_p360000exe14", "pero_EGF1_h_m1m1_p360000exe15", "pero_EGF1_h_m1m1_p360000exe16", "pero_EGF1_h_m1m1_p360000exe2", "pero_EGF1_h_m1m1_p360000exe3", "pero_EGF1_h_m1m1_p360000exe4", "pero_EGF1_h_m1m1_p360000exe5", "pero_EGF1_h_m1m1_p360000exe6", "pero_EGF1_h_m1m1_p360000exe7", "pero_EGF1_h_m1m1_p360000exe8", "pero_EGF1_h_m1m1_p360000exe9", "pero_EGF1_h_m1m1_p380000exe0", "pero_EGF1_h_m1m1_p380000exe1", "pero_EGF1_h_m1m1_p380000exe10", "pero_EGF1_h_m1m1_p380000exe11", "pero_EGF1_h_m1m1_p380000exe12", "pero_EGF1_h_m1m1_p380000exe13", "pero_EGF1_h_m1m1_p380000exe14", "pero_EGF1_h_m1m1_p380000exe15", "pero_EGF1_h_m1m1_p380000exe16", "pero_EGF1_h_m1m1_p380000exe2", "pero_EGF1_h_m1m1_p380000exe3", "pero_EGF1_h_m1m1_p380000exe4", "pero_EGF1_h_m1m1_p380000exe5", "pero_EGF1_h_m1m1_p380000exe6", "pero_EGF1_h_m1m1_p380000exe7", "pero_EGF1_h_m1m1_p380000exe8", "pero_EGF1_h_m1m1_p380000exe9", "pero_EGF1_h_m1m1_p400000exe0", "pero_EGF1_h_m1m1_p400000exe1", "pero_EGF1_h_m1m1_p400000exe10", "pero_EGF1_h_m1m1_p400000exe11", "pero_EGF1_h_m1m1_p400000exe12", "pero_EGF1_h_m1m1_p400000exe13", "pero_EGF1_h_m1m1_p400000exe14", "pero_EGF1_h_m1m1_p400000exe15", "pero_EGF1_h_m1m1_p400000exe16", "pero_EGF1_h_m1m1_p400000exe2", "pero_EGF1_h_m1m1_p400000exe3", "pero_EGF1_h_m1m1_p400000exe4", "pero_EGF1_h_m1m1_p400000exe5", "pero_EGF1_h_m1m1_p400000exe6", "pero_EGF1_h_m1m1_p400000exe7", "pero_EGF1_h_m1m1_p400000exe8", "pero_EGF1_h_m1m1_p400000exe9", "pero_EGF1_h_m1m1_p40000exe0", "pero_EGF1_h_m1m1_p40000exe1", "pero_EGF1_h_m1m1_p40000exe10", "pero_EGF1_h_m1m1_p40000exe11", "pero_EGF1_h_m1m1_p40000exe12", "pero_EGF1_h_m1m1_p40000exe13", "pero_EGF1_h_m1m1_p40000exe14", "pero_EGF1_h_m1m1_p40000exe15", "pero_EGF1_h_m1m1_p40000exe16", "pero_EGF1_h_m1m1_p40000exe2", "pero_EGF1_h_m1m1_p40000exe3", "pero_EGF1_h_m1m1_p40000exe4", "pero_EGF1_h_m1m1_p40000exe5", "pero_EGF1_h_m1m1_p40000exe6", "pero_EGF1_h_m1m1_p40000exe7", "pero_EGF1_h_m1m1_p40000exe8", "pero_EGF1_h_m1m1_p40000exe9", "pero_EGF1_h_m1m1_p4000exe0", "pero_EGF1_h_m1m1_p4000exe1", "pero_EGF1_h_m1m1_p4000exe10", "pero_EGF1_h_m1m1_p4000exe11", "pero_EGF1_h_m1m1_p4000exe12", "pero_EGF1_h_m1m1_p4000exe13", "pero_EGF1_h_m1m1_p4000exe14", "pero_EGF1_h_m1m1_p4000exe15", "pero_EGF1_h_m1m1_p4000exe16", "pero_EGF1_h_m1m1_p4000exe2", "pero_EGF1_h_m1m1_p4000exe3", "pero_EGF1_h_m1m1_p4000exe4", "pero_EGF1_h_m1m1_p4000exe5", "pero_EGF1_h_m1m1_p4000exe6", "pero_EGF1_h_m1m1_p4000exe7", "pero_EGF1_h_m1m1_p4000exe8", "pero_EGF1_h_m1m1_p4000exe9", "pero_EGF1_h_m1m1_p400exe0", "pero_EGF1_h_m1m1_p400exe1", "pero_EGF1_h_m1m1_p400exe10", "pero_EGF1_h_m1m1_p400exe11", "pero_EGF1_h_m1m1_p400exe12", "pero_EGF1_h_m1m1_p400exe13", "pero_EGF1_h_m1m1_p400exe14", "pero_EGF1_h_m1m1_p400exe15", "pero_EGF1_h_m1m1_p400exe16", "pero_EGF1_h_m1m1_p400exe2", "pero_EGF1_h_m1m1_p400exe3", "pero_EGF1_h_m1m1_p400exe4", "pero_EGF1_h_m1m1_p400exe5", "pero_EGF1_h_m1m1_p400exe6", "pero_EGF1_h_m1m1_p400exe7", "pero_EGF1_h_m1m1_p400exe8", "pero_EGF1_h_m1m1_p400exe9", "pero_EGF1_h_m1m1_p420000exe0", "pero_EGF1_h_m1m1_p420000exe1", "pero_EGF1_h_m1m1_p420000exe10", "pero_EGF1_h_m1m1_p420000exe11", "pero_EGF1_h_m1m1_p420000exe12", "pero_EGF1_h_m1m1_p420000exe13", "pero_EGF1_h_m1m1_p420000exe14", "pero_EGF1_h_m1m1_p420000exe15", "pero_EGF1_h_m1m1_p420000exe16", "pero_EGF1_h_m1m1_p420000exe2", "pero_EGF1_h_m1m1_p420000exe3", "pero_EGF1_h_m1m1_p420000exe4", "pero_EGF1_h_m1m1_p420000exe5", "pero_EGF1_h_m1m1_p420000exe6", "pero_EGF1_h_m1m1_p420000exe7", "pero_EGF1_h_m1m1_p420000exe8", "pero_EGF1_h_m1m1_p420000exe9", "pero_EGF1_h_m1m1_p440000exe0", "pero_EGF1_h_m1m1_p440000exe1", "pero_EGF1_h_m1m1_p440000exe10", "pero_EGF1_h_m1m1_p440000exe11", "pero_EGF1_h_m1m1_p440000exe12", "pero_EGF1_h_m1m1_p440000exe13", "pero_EGF1_h_m1m1_p440000exe14", "pero_EGF1_h_m1m1_p440000exe15", "pero_EGF1_h_m1m1_p440000exe16", "pero_EGF1_h_m1m1_p440000exe2", "pero_EGF1_h_m1m1_p440000exe3", "pero_EGF1_h_m1m1_p440000exe4", "pero_EGF1_h_m1m1_p440000exe5", "pero_EGF1_h_m1m1_p440000exe6", "pero_EGF1_h_m1m1_p440000exe7", "pero_EGF1_h_m1m1_p440000exe8", "pero_EGF1_h_m1m1_p440000exe9", "pero_EGF1_h_m1m1_p480000exe0", "pero_EGF1_h_m1m1_p480000exe1", "pero_EGF1_h_m1m1_p480000exe10", "pero_EGF1_h_m1m1_p480000exe11", "pero_EGF1_h_m1m1_p480000exe12", "pero_EGF1_h_m1m1_p480000exe13", "pero_EGF1_h_m1m1_p480000exe14", "pero_EGF1_h_m1m1_p480000exe15", "pero_EGF1_h_m1m1_p480000exe16", "pero_EGF1_h_m1m1_p480000exe2", "pero_EGF1_h_m1m1_p480000exe3", "pero_EGF1_h_m1m1_p480000exe4", "pero_EGF1_h_m1m1_p480000exe5", "pero_EGF1_h_m1m1_p480000exe6", "pero_EGF1_h_m1m1_p480000exe7", "pero_EGF1_h_m1m1_p480000exe8", "pero_EGF1_h_m1m1_p480000exe9", "pero_EGF1_h_m1m1_p500000exe0", "pero_EGF1_h_m1m1_p500000exe1", "pero_EGF1_h_m1m1_p500000exe10", "pero_EGF1_h_m1m1_p500000exe11", "pero_EGF1_h_m1m1_p500000exe12", "pero_EGF1_h_m1m1_p500000exe13", "pero_EGF1_h_m1m1_p500000exe14", "pero_EGF1_h_m1m1_p500000exe15", "pero_EGF1_h_m1m1_p500000exe16", "pero_EGF1_h_m1m1_p500000exe2", "pero_EGF1_h_m1m1_p500000exe3", "pero_EGF1_h_m1m1_p500000exe4", "pero_EGF1_h_m1m1_p500000exe5", "pero_EGF1_h_m1m1_p500000exe6", "pero_EGF1_h_m1m1_p500000exe7", "pero_EGF1_h_m1m1_p500000exe8", "pero_EGF1_h_m1m1_p500000exe9", "pero_EGF1_h_m1m1_p50000exe0", "pero_EGF1_h_m1m1_p50000exe1", "pero_EGF1_h_m1m1_p50000exe10", "pero_EGF1_h_m1m1_p50000exe11", "pero_EGF1_h_m1m1_p50000exe12", "pero_EGF1_h_m1m1_p50000exe13", "pero_EGF1_h_m1m1_p50000exe14", "pero_EGF1_h_m1m1_p50000exe15", "pero_EGF1_h_m1m1_p50000exe16", "pero_EGF1_h_m1m1_p50000exe2", "pero_EGF1_h_m1m1_p50000exe3", "pero_EGF1_h_m1m1_p50000exe4", "pero_EGF1_h_m1m1_p50000exe5", "pero_EGF1_h_m1m1_p50000exe6", "pero_EGF1_h_m1m1_p50000exe7", "pero_EGF1_h_m1m1_p50000exe8", "pero_EGF1_h_m1m1_p50000exe9", "pero_EGF1_h_m1m1_p500exe0", "pero_EGF1_h_m1m1_p500exe1", "pero_EGF1_h_m1m1_p500exe10", "pero_EGF1_h_m1m1_p500exe11", "pero_EGF1_h_m1m1_p500exe12", "pero_EGF1_h_m1m1_p500exe13", "pero_EGF1_h_m1m1_p500exe14", "pero_EGF1_h_m1m1_p500exe15", "pero_EGF1_h_m1m1_p500exe16", "pero_EGF1_h_m1m1_p500exe2", "pero_EGF1_h_m1m1_p500exe3", "pero_EGF1_h_m1m1_p500exe4", "pero_EGF1_h_m1m1_p500exe5", "pero_EGF1_h_m1m1_p500exe6", "pero_EGF1_h_m1m1_p500exe7", "pero_EGF1_h_m1m1_p500exe8", "pero_EGF1_h_m1m1_p500exe9", "pero_EGF1_h_m1m1_p60000exe0", "pero_EGF1_h_m1m1_p60000exe1", "pero_EGF1_h_m1m1_p60000exe10", "pero_EGF1_h_m1m1_p60000exe11", "pero_EGF1_h_m1m1_p60000exe12", "pero_EGF1_h_m1m1_p60000exe13", "pero_EGF1_h_m1m1_p60000exe14", "pero_EGF1_h_m1m1_p60000exe15", "pero_EGF1_h_m1m1_p60000exe16", "pero_EGF1_h_m1m1_p60000exe2", "pero_EGF1_h_m1m1_p60000exe3", "pero_EGF1_h_m1m1_p60000exe4", "pero_EGF1_h_m1m1_p60000exe5", "pero_EGF1_h_m1m1_p60000exe6", "pero_EGF1_h_m1m1_p60000exe7", "pero_EGF1_h_m1m1_p60000exe8", "pero_EGF1_h_m1m1_p60000exe9", "pero_EGF1_h_m1m1_p6000exe0", "pero_EGF1_h_m1m1_p6000exe1", "pero_EGF1_h_m1m1_p6000exe10", "pero_EGF1_h_m1m1_p6000exe11", "pero_EGF1_h_m1m1_p6000exe12", "pero_EGF1_h_m1m1_p6000exe13", "pero_EGF1_h_m1m1_p6000exe14", "pero_EGF1_h_m1m1_p6000exe15", "pero_EGF1_h_m1m1_p6000exe16", "pero_EGF1_h_m1m1_p6000exe2", "pero_EGF1_h_m1m1_p6000exe3", "pero_EGF1_h_m1m1_p6000exe4", "pero_EGF1_h_m1m1_p6000exe5", "pero_EGF1_h_m1m1_p6000exe6", "pero_EGF1_h_m1m1_p6000exe7", "pero_EGF1_h_m1m1_p6000exe8", "pero_EGF1_h_m1m1_p6000exe9", "pero_EGF1_h_m1m1_p600exe0", "pero_EGF1_h_m1m1_p600exe1", "pero_EGF1_h_m1m1_p600exe10", "pero_EGF1_h_m1m1_p600exe11", "pero_EGF1_h_m1m1_p600exe12", "pero_EGF1_h_m1m1_p600exe13", "pero_EGF1_h_m1m1_p600exe14", "pero_EGF1_h_m1m1_p600exe15", "pero_EGF1_h_m1m1_p600exe16", "pero_EGF1_h_m1m1_p600exe17", "pero_EGF1_h_m1m1_p600exe2", "pero_EGF1_h_m1m1_p600exe3", "pero_EGF1_h_m1m1_p600exe4", "pero_EGF1_h_m1m1_p600exe5", "pero_EGF1_h_m1m1_p600exe6", "pero_EGF1_h_m1m1_p600exe7", "pero_EGF1_h_m1m1_p600exe8", "pero_EGF1_h_m1m1_p600exe9", "pero_EGF1_h_m1m1_p700exe0", "pero_EGF1_h_m1m1_p700exe1", "pero_EGF1_h_m1m1_p700exe10", "pero_EGF1_h_m1m1_p700exe11", "pero_EGF1_h_m1m1_p700exe12", "pero_EGF1_h_m1m1_p700exe13", "pero_EGF1_h_m1m1_p700exe14", "pero_EGF1_h_m1m1_p700exe15", "pero_EGF1_h_m1m1_p700exe16", "pero_EGF1_h_m1m1_p700exe2", "pero_EGF1_h_m1m1_p700exe3", "pero_EGF1_h_m1m1_p700exe4", "pero_EGF1_h_m1m1_p700exe5", "pero_EGF1_h_m1m1_p700exe6", "pero_EGF1_h_m1m1_p700exe7", "pero_EGF1_h_m1m1_p700exe8", "pero_EGF1_h_m1m1_p700exe9", "pero_EGF1_h_m1m1_p80000exe0", "pero_EGF1_h_m1m1_p80000exe1", "pero_EGF1_h_m1m1_p80000exe10", "pero_EGF1_h_m1m1_p80000exe11", "pero_EGF1_h_m1m1_p80000exe12", "pero_EGF1_h_m1m1_p80000exe13", "pero_EGF1_h_m1m1_p80000exe14", "pero_EGF1_h_m1m1_p80000exe15", "pero_EGF1_h_m1m1_p80000exe16", "pero_EGF1_h_m1m1_p80000exe2", "pero_EGF1_h_m1m1_p80000exe3", "pero_EGF1_h_m1m1_p80000exe4", "pero_EGF1_h_m1m1_p80000exe5", "pero_EGF1_h_m1m1_p80000exe6", "pero_EGF1_h_m1m1_p80000exe7", "pero_EGF1_h_m1m1_p80000exe8", "pero_EGF1_h_m1m1_p80000exe9", "pero_EGF1_h_m1m1_p800exe0", "pero_EGF1_h_m1m1_p800exe1", "pero_EGF1_h_m1m1_p800exe10", "pero_EGF1_h_m1m1_p800exe11", "pero_EGF1_h_m1m1_p800exe12", "pero_EGF1_h_m1m1_p800exe13", "pero_EGF1_h_m1m1_p800exe14", "pero_EGF1_h_m1m1_p800exe15", "pero_EGF1_h_m1m1_p800exe16", "pero_EGF1_h_m1m1_p800exe2", "pero_EGF1_h_m1m1_p800exe3", "pero_EGF1_h_m1m1_p800exe4", "pero_EGF1_h_m1m1_p800exe5", "pero_EGF1_h_m1m1_p800exe6", "pero_EGF1_h_m1m1_p800exe7", "pero_EGF1_h_m1m1_p800exe8", "pero_EGF1_h_m1m1_p800exe9", "pero_EGF1_h_m1m1_p900exe0", "pero_EGF1_h_m1m1_p900exe1", "pero_EGF1_h_m1m1_p900exe10", "pero_EGF1_h_m1m1_p900exe11", "pero_EGF1_h_m1m1_p900exe12", "pero_EGF1_h_m1m1_p900exe13", "pero_EGF1_h_m1m1_p900exe14", "pero_EGF1_h_m1m1_p900exe15", "pero_EGF1_h_m1m1_p900exe16", "pero_EGF1_h_m1m1_p900exe2", "pero_EGF1_h_m1m1_p900exe3", "pero_EGF1_h_m1m1_p900exe4", "pero_EGF1_h_m1m1_p900exe5", "pero_EGF1_h_m1m1_p900exe6", "pero_EGF1_h_m1m1_p900exe7", "pero_EGF1_h_m1m1_p900exe8", "pero_EGF1_h_m1m1_p900exe9", "pero_EGF1_h_m1p0_m0exe0", "pero_EGF1_h_m1p0_m0exe1", "pero_EGF1_h_m1p0_m0exe10", "pero_EGF1_h_m1p0_m0exe11", "pero_EGF1_h_m1p0_m0exe12", "pero_EGF1_h_m1p0_m0exe13", "pero_EGF1_h_m1p0_m0exe14", "pero_EGF1_h_m1p0_m0exe15", "pero_EGF1_h_m1p0_m0exe16", "pero_EGF1_h_m1p0_m0exe2", "pero_EGF1_h_m1p0_m0exe3", "pero_EGF1_h_m1p0_m0exe4", "pero_EGF1_h_m1p0_m0exe5", "pero_EGF1_h_m1p0_m0exe6", "pero_EGF1_h_m1p0_m0exe7", "pero_EGF1_h_m1p0_m0exe8", "pero_EGF1_h_m1p0_m0exe9", "pero_EGF1_h_m1p0_m100exe0", "pero_EGF1_h_m1p0_m100exe1", "pero_EGF1_h_m1p0_m100exe10", "pero_EGF1_h_m1p0_m100exe11", "pero_EGF1_h_m1p0_m100exe12", "pero_EGF1_h_m1p0_m100exe13", "pero_EGF1_h_m1p0_m100exe14", "pero_EGF1_h_m1p0_m100exe15", "pero_EGF1_h_m1p0_m100exe16", "pero_EGF1_h_m1p0_m100exe2", "pero_EGF1_h_m1p0_m100exe3", "pero_EGF1_h_m1p0_m100exe4", "pero_EGF1_h_m1p0_m100exe5", "pero_EGF1_h_m1p0_m100exe6", "pero_EGF1_h_m1p0_m100exe7", "pero_EGF1_h_m1p0_m100exe8", "pero_EGF1_h_m1p0_m100exe9", "pero_EGF1_h_m1p0_m200exe0", "pero_EGF1_h_m1p0_m200exe1", "pero_EGF1_h_m1p0_m200exe10", "pero_EGF1_h_m1p0_m200exe11", "pero_EGF1_h_m1p0_m200exe12", "pero_EGF1_h_m1p0_m200exe13", "pero_EGF1_h_m1p0_m200exe14", "pero_EGF1_h_m1p0_m200exe15", "pero_EGF1_h_m1p0_m200exe16", "pero_EGF1_h_m1p0_m200exe2", "pero_EGF1_h_m1p0_m200exe3", "pero_EGF1_h_m1p0_m200exe4", "pero_EGF1_h_m1p0_m200exe5", "pero_EGF1_h_m1p0_m200exe6", "pero_EGF1_h_m1p0_m200exe7", "pero_EGF1_h_m1p0_m200exe8", "pero_EGF1_h_m1p0_m200exe9", "pero_EGF1_h_m1p0_m300exe0", "pero_EGF1_h_m1p0_m300exe1", "pero_EGF1_h_m1p0_m300exe10", "pero_EGF1_h_m1p0_m300exe11", "pero_EGF1_h_m1p0_m300exe12", "pero_EGF1_h_m1p0_m300exe13", "pero_EGF1_h_m1p0_m300exe14", "pero_EGF1_h_m1p0_m300exe15", "pero_EGF1_h_m1p0_m300exe16", "pero_EGF1_h_m1p0_m300exe2", "pero_EGF1_h_m1p0_m300exe3", "pero_EGF1_h_m1p0_m300exe4", "pero_EGF1_h_m1p0_m300exe5", "pero_EGF1_h_m1p0_m300exe6", "pero_EGF1_h_m1p0_m300exe7", "pero_EGF1_h_m1p0_m300exe8", "pero_EGF1_h_m1p0_m300exe9", "pero_EGF1_h_m1p0_m5000exe0", "pero_EGF1_h_m1p0_m5000exe1", "pero_EGF1_h_m1p0_m5000exe10", "pero_EGF1_h_m1p0_m5000exe11", "pero_EGF1_h_m1p0_m5000exe12", "pero_EGF1_h_m1p0_m5000exe13", "pero_EGF1_h_m1p0_m5000exe14", "pero_EGF1_h_m1p0_m5000exe15", "pero_EGF1_h_m1p0_m5000exe16", "pero_EGF1_h_m1p0_m5000exe2", "pero_EGF1_h_m1p0_m5000exe3", "pero_EGF1_h_m1p0_m5000exe4", "pero_EGF1_h_m1p0_m5000exe5", "pero_EGF1_h_m1p0_m5000exe6", "pero_EGF1_h_m1p0_m5000exe7", "pero_EGF1_h_m1p0_m5000exe8", "pero_EGF1_h_m1p0_m5000exe9", "pero_EGF1_h_m1p0_m500exe0", "pero_EGF1_h_m1p0_m500exe1", "pero_EGF1_h_m1p0_m500exe10", "pero_EGF1_h_m1p0_m500exe11", "pero_EGF1_h_m1p0_m500exe12", "pero_EGF1_h_m1p0_m500exe13", "pero_EGF1_h_m1p0_m500exe14", "pero_EGF1_h_m1p0_m500exe15", "pero_EGF1_h_m1p0_m500exe16", "pero_EGF1_h_m1p0_m500exe2", "pero_EGF1_h_m1p0_m500exe3", "pero_EGF1_h_m1p0_m500exe4", "pero_EGF1_h_m1p0_m500exe5", "pero_EGF1_h_m1p0_m500exe6", "pero_EGF1_h_m1p0_m500exe7", "pero_EGF1_h_m1p0_m500exe8", "pero_EGF1_h_m1p0_m500exe9", "pero_EGF1_h_m1p0_p100000exe0", "pero_EGF1_h_m1p0_p100000exe1", "pero_EGF1_h_m1p0_p100000exe10", "pero_EGF1_h_m1p0_p100000exe11", "pero_EGF1_h_m1p0_p100000exe12", "pero_EGF1_h_m1p0_p100000exe13", "pero_EGF1_h_m1p0_p100000exe14", "pero_EGF1_h_m1p0_p100000exe15", "pero_EGF1_h_m1p0_p100000exe16", "pero_EGF1_h_m1p0_p100000exe2", "pero_EGF1_h_m1p0_p100000exe3", "pero_EGF1_h_m1p0_p100000exe4", "pero_EGF1_h_m1p0_p100000exe5", "pero_EGF1_h_m1p0_p100000exe6", "pero_EGF1_h_m1p0_p100000exe7", "pero_EGF1_h_m1p0_p100000exe8", "pero_EGF1_h_m1p0_p100000exe9", "pero_EGF1_h_m1p0_p10000exe0", "pero_EGF1_h_m1p0_p10000exe1", "pero_EGF1_h_m1p0_p10000exe10", "pero_EGF1_h_m1p0_p10000exe11", "pero_EGF1_h_m1p0_p10000exe12", "pero_EGF1_h_m1p0_p10000exe13", "pero_EGF1_h_m1p0_p10000exe14", "pero_EGF1_h_m1p0_p10000exe15", "pero_EGF1_h_m1p0_p10000exe16", "pero_EGF1_h_m1p0_p10000exe2", "pero_EGF1_h_m1p0_p10000exe3", "pero_EGF1_h_m1p0_p10000exe4", "pero_EGF1_h_m1p0_p10000exe5", "pero_EGF1_h_m1p0_p10000exe6", "pero_EGF1_h_m1p0_p10000exe7", "pero_EGF1_h_m1p0_p10000exe8", "pero_EGF1_h_m1p0_p10000exe9", "pero_EGF1_h_m1p0_p1000exe0", "pero_EGF1_h_m1p0_p1000exe1", "pero_EGF1_h_m1p0_p1000exe10", "pero_EGF1_h_m1p0_p1000exe11", "pero_EGF1_h_m1p0_p1000exe12", "pero_EGF1_h_m1p0_p1000exe13", "pero_EGF1_h_m1p0_p1000exe14", "pero_EGF1_h_m1p0_p1000exe15", "pero_EGF1_h_m1p0_p1000exe16", "pero_EGF1_h_m1p0_p1000exe17", "pero_EGF1_h_m1p0_p1000exe2", "pero_EGF1_h_m1p0_p1000exe3", "pero_EGF1_h_m1p0_p1000exe4", "pero_EGF1_h_m1p0_p1000exe5", "pero_EGF1_h_m1p0_p1000exe6", "pero_EGF1_h_m1p0_p1000exe7", "pero_EGF1_h_m1p0_p1000exe8", "pero_EGF1_h_m1p0_p1000exe9", "pero_EGF1_h_m1p0_p100exe0", "pero_EGF1_h_m1p0_p100exe1", "pero_EGF1_h_m1p0_p100exe10", "pero_EGF1_h_m1p0_p100exe11", "pero_EGF1_h_m1p0_p100exe12", "pero_EGF1_h_m1p0_p100exe13", "pero_EGF1_h_m1p0_p100exe14", "pero_EGF1_h_m1p0_p100exe15", "pero_EGF1_h_m1p0_p100exe16", "pero_EGF1_h_m1p0_p100exe2", "pero_EGF1_h_m1p0_p100exe3", "pero_EGF1_h_m1p0_p100exe4", "pero_EGF1_h_m1p0_p100exe5", "pero_EGF1_h_m1p0_p100exe6", "pero_EGF1_h_m1p0_p100exe7", "pero_EGF1_h_m1p0_p100exe8", "pero_EGF1_h_m1p0_p100exe9", "pero_EGF1_h_m1p0_p1100exe0", "pero_EGF1_h_m1p0_p1100exe1", "pero_EGF1_h_m1p0_p1100exe10", "pero_EGF1_h_m1p0_p1100exe11", "pero_EGF1_h_m1p0_p1100exe12", "pero_EGF1_h_m1p0_p1100exe13", "pero_EGF1_h_m1p0_p1100exe14", "pero_EGF1_h_m1p0_p1100exe15", "pero_EGF1_h_m1p0_p1100exe16", "pero_EGF1_h_m1p0_p1100exe2", "pero_EGF1_h_m1p0_p1100exe3", "pero_EGF1_h_m1p0_p1100exe4", "pero_EGF1_h_m1p0_p1100exe5", "pero_EGF1_h_m1p0_p1100exe6", "pero_EGF1_h_m1p0_p1100exe7", "pero_EGF1_h_m1p0_p1100exe8", "pero_EGF1_h_m1p0_p1100exe9", "pero_EGF1_h_m1p0_p120000exe0", "pero_EGF1_h_m1p0_p120000exe1", "pero_EGF1_h_m1p0_p120000exe10", "pero_EGF1_h_m1p0_p120000exe11", "pero_EGF1_h_m1p0_p120000exe12", "pero_EGF1_h_m1p0_p120000exe13", "pero_EGF1_h_m1p0_p120000exe14", "pero_EGF1_h_m1p0_p120000exe15", "pero_EGF1_h_m1p0_p120000exe16", "pero_EGF1_h_m1p0_p120000exe2", "pero_EGF1_h_m1p0_p120000exe3", "pero_EGF1_h_m1p0_p120000exe4", "pero_EGF1_h_m1p0_p120000exe5", "pero_EGF1_h_m1p0_p120000exe6", "pero_EGF1_h_m1p0_p120000exe7", "pero_EGF1_h_m1p0_p120000exe8", "pero_EGF1_h_m1p0_p120000exe9", "pero_EGF1_h_m1p0_p1200exe0", "pero_EGF1_h_m1p0_p1200exe1", "pero_EGF1_h_m1p0_p1200exe10", "pero_EGF1_h_m1p0_p1200exe11", "pero_EGF1_h_m1p0_p1200exe12", "pero_EGF1_h_m1p0_p1200exe13", "pero_EGF1_h_m1p0_p1200exe14", "pero_EGF1_h_m1p0_p1200exe15", "pero_EGF1_h_m1p0_p1200exe16", "pero_EGF1_h_m1p0_p1200exe2", "pero_EGF1_h_m1p0_p1200exe3", "pero_EGF1_h_m1p0_p1200exe4", "pero_EGF1_h_m1p0_p1200exe5", "pero_EGF1_h_m1p0_p1200exe6", "pero_EGF1_h_m1p0_p1200exe7", "pero_EGF1_h_m1p0_p1200exe8", "pero_EGF1_h_m1p0_p1200exe9", "pero_EGF1_h_m1p0_p1300exe0", "pero_EGF1_h_m1p0_p1300exe1", "pero_EGF1_h_m1p0_p1300exe10", "pero_EGF1_h_m1p0_p1300exe11", "pero_EGF1_h_m1p0_p1300exe12", "pero_EGF1_h_m1p0_p1300exe13", "pero_EGF1_h_m1p0_p1300exe14", "pero_EGF1_h_m1p0_p1300exe15", "pero_EGF1_h_m1p0_p1300exe16", "pero_EGF1_h_m1p0_p1300exe2", "pero_EGF1_h_m1p0_p1300exe3", "pero_EGF1_h_m1p0_p1300exe4", "pero_EGF1_h_m1p0_p1300exe5", "pero_EGF1_h_m1p0_p1300exe6", "pero_EGF1_h_m1p0_p1300exe7", "pero_EGF1_h_m1p0_p1300exe8", "pero_EGF1_h_m1p0_p1300exe9", "pero_EGF1_h_m1p0_p140000exe0", "pero_EGF1_h_m1p0_p140000exe1", "pero_EGF1_h_m1p0_p140000exe10", "pero_EGF1_h_m1p0_p140000exe11", "pero_EGF1_h_m1p0_p140000exe12", "pero_EGF1_h_m1p0_p140000exe13", "pero_EGF1_h_m1p0_p140000exe14", "pero_EGF1_h_m1p0_p140000exe15", "pero_EGF1_h_m1p0_p140000exe16", "pero_EGF1_h_m1p0_p140000exe2", "pero_EGF1_h_m1p0_p140000exe3", "pero_EGF1_h_m1p0_p140000exe4", "pero_EGF1_h_m1p0_p140000exe5", "pero_EGF1_h_m1p0_p140000exe6", "pero_EGF1_h_m1p0_p140000exe7", "pero_EGF1_h_m1p0_p140000exe8", "pero_EGF1_h_m1p0_p140000exe9", "pero_EGF1_h_m1p0_p1400exe0", "pero_EGF1_h_m1p0_p1400exe1", "pero_EGF1_h_m1p0_p1400exe10", "pero_EGF1_h_m1p0_p1400exe11", "pero_EGF1_h_m1p0_p1400exe12", "pero_EGF1_h_m1p0_p1400exe13", "pero_EGF1_h_m1p0_p1400exe14", "pero_EGF1_h_m1p0_p1400exe15", "pero_EGF1_h_m1p0_p1400exe16", "pero_EGF1_h_m1p0_p1400exe2", "pero_EGF1_h_m1p0_p1400exe3", "pero_EGF1_h_m1p0_p1400exe4", "pero_EGF1_h_m1p0_p1400exe5", "pero_EGF1_h_m1p0_p1400exe6", "pero_EGF1_h_m1p0_p1400exe7", "pero_EGF1_h_m1p0_p1400exe8", "pero_EGF1_h_m1p0_p1400exe9", "pero_EGF1_h_m1p0_p1500exe0", "pero_EGF1_h_m1p0_p1500exe1", "pero_EGF1_h_m1p0_p1500exe10", "pero_EGF1_h_m1p0_p1500exe11", "pero_EGF1_h_m1p0_p1500exe12", "pero_EGF1_h_m1p0_p1500exe13", "pero_EGF1_h_m1p0_p1500exe14", "pero_EGF1_h_m1p0_p1500exe15", "pero_EGF1_h_m1p0_p1500exe16", "pero_EGF1_h_m1p0_p1500exe2", "pero_EGF1_h_m1p0_p1500exe3", "pero_EGF1_h_m1p0_p1500exe4", "pero_EGF1_h_m1p0_p1500exe5", "pero_EGF1_h_m1p0_p1500exe6", "pero_EGF1_h_m1p0_p1500exe7", "pero_EGF1_h_m1p0_p1500exe8", "pero_EGF1_h_m1p0_p1500exe9", "pero_EGF1_h_m1p0_p160000exe0", "pero_EGF1_h_m1p0_p160000exe1", "pero_EGF1_h_m1p0_p160000exe10", "pero_EGF1_h_m1p0_p160000exe11", "pero_EGF1_h_m1p0_p160000exe12", "pero_EGF1_h_m1p0_p160000exe13", "pero_EGF1_h_m1p0_p160000exe14", "pero_EGF1_h_m1p0_p160000exe15", "pero_EGF1_h_m1p0_p160000exe16", "pero_EGF1_h_m1p0_p160000exe2", "pero_EGF1_h_m1p0_p160000exe3", "pero_EGF1_h_m1p0_p160000exe4", "pero_EGF1_h_m1p0_p160000exe5", "pero_EGF1_h_m1p0_p160000exe6", "pero_EGF1_h_m1p0_p160000exe7", "pero_EGF1_h_m1p0_p160000exe8", "pero_EGF1_h_m1p0_p160000exe9", "pero_EGF1_h_m1p0_p1600exe0", "pero_EGF1_h_m1p0_p1600exe1", "pero_EGF1_h_m1p0_p1600exe10", "pero_EGF1_h_m1p0_p1600exe11", "pero_EGF1_h_m1p0_p1600exe12", "pero_EGF1_h_m1p0_p1600exe13", "pero_EGF1_h_m1p0_p1600exe14", "pero_EGF1_h_m1p0_p1600exe15", "pero_EGF1_h_m1p0_p1600exe16", "pero_EGF1_h_m1p0_p1600exe2", "pero_EGF1_h_m1p0_p1600exe3", "pero_EGF1_h_m1p0_p1600exe4", "pero_EGF1_h_m1p0_p1600exe5", "pero_EGF1_h_m1p0_p1600exe6", "pero_EGF1_h_m1p0_p1600exe7", "pero_EGF1_h_m1p0_p1600exe8", "pero_EGF1_h_m1p0_p1600exe9", "pero_EGF1_h_m1p0_p1700exe0", "pero_EGF1_h_m1p0_p1700exe1", "pero_EGF1_h_m1p0_p1700exe10", "pero_EGF1_h_m1p0_p1700exe11", "pero_EGF1_h_m1p0_p1700exe12", "pero_EGF1_h_m1p0_p1700exe13", "pero_EGF1_h_m1p0_p1700exe14", "pero_EGF1_h_m1p0_p1700exe15", "pero_EGF1_h_m1p0_p1700exe16", "pero_EGF1_h_m1p0_p1700exe2", "pero_EGF1_h_m1p0_p1700exe3", "pero_EGF1_h_m1p0_p1700exe4", "pero_EGF1_h_m1p0_p1700exe5", "pero_EGF1_h_m1p0_p1700exe6", "pero_EGF1_h_m1p0_p1700exe7", "pero_EGF1_h_m1p0_p1700exe8", "pero_EGF1_h_m1p0_p1700exe9", "pero_EGF1_h_m1p0_p180000exe0", "pero_EGF1_h_m1p0_p180000exe1", "pero_EGF1_h_m1p0_p180000exe10", "pero_EGF1_h_m1p0_p180000exe11", "pero_EGF1_h_m1p0_p180000exe12", "pero_EGF1_h_m1p0_p180000exe13", "pero_EGF1_h_m1p0_p180000exe14", "pero_EGF1_h_m1p0_p180000exe15", "pero_EGF1_h_m1p0_p180000exe16", "pero_EGF1_h_m1p0_p180000exe2", "pero_EGF1_h_m1p0_p180000exe3", "pero_EGF1_h_m1p0_p180000exe4", "pero_EGF1_h_m1p0_p180000exe5", "pero_EGF1_h_m1p0_p180000exe6", "pero_EGF1_h_m1p0_p180000exe7", "pero_EGF1_h_m1p0_p180000exe8", "pero_EGF1_h_m1p0_p180000exe9", "pero_EGF1_h_m1p0_p1800exe0", "pero_EGF1_h_m1p0_p1800exe1", "pero_EGF1_h_m1p0_p1800exe10", "pero_EGF1_h_m1p0_p1800exe11", "pero_EGF1_h_m1p0_p1800exe12", "pero_EGF1_h_m1p0_p1800exe13", "pero_EGF1_h_m1p0_p1800exe14", "pero_EGF1_h_m1p0_p1800exe15", "pero_EGF1_h_m1p0_p1800exe16", "pero_EGF1_h_m1p0_p1800exe2", "pero_EGF1_h_m1p0_p1800exe3", "pero_EGF1_h_m1p0_p1800exe4", "pero_EGF1_h_m1p0_p1800exe5", "pero_EGF1_h_m1p0_p1800exe6", "pero_EGF1_h_m1p0_p1800exe7", "pero_EGF1_h_m1p0_p1800exe8", "pero_EGF1_h_m1p0_p1800exe9", "pero_EGF1_h_m1p0_p1900exe0", "pero_EGF1_h_m1p0_p1900exe1", "pero_EGF1_h_m1p0_p1900exe10", "pero_EGF1_h_m1p0_p1900exe11", "pero_EGF1_h_m1p0_p1900exe12", "pero_EGF1_h_m1p0_p1900exe13", "pero_EGF1_h_m1p0_p1900exe14", "pero_EGF1_h_m1p0_p1900exe15", "pero_EGF1_h_m1p0_p1900exe16", "pero_EGF1_h_m1p0_p1900exe17", "pero_EGF1_h_m1p0_p1900exe2", "pero_EGF1_h_m1p0_p1900exe3", "pero_EGF1_h_m1p0_p1900exe4", "pero_EGF1_h_m1p0_p1900exe5", "pero_EGF1_h_m1p0_p1900exe6", "pero_EGF1_h_m1p0_p1900exe7", "pero_EGF1_h_m1p0_p1900exe8", "pero_EGF1_h_m1p0_p1900exe9", "pero_EGF1_h_m1p0_p200000exe0", "pero_EGF1_h_m1p0_p200000exe1", "pero_EGF1_h_m1p0_p200000exe10", "pero_EGF1_h_m1p0_p200000exe11", "pero_EGF1_h_m1p0_p200000exe12", "pero_EGF1_h_m1p0_p200000exe13", "pero_EGF1_h_m1p0_p200000exe14", "pero_EGF1_h_m1p0_p200000exe15", "pero_EGF1_h_m1p0_p200000exe16", "pero_EGF1_h_m1p0_p200000exe2", "pero_EGF1_h_m1p0_p200000exe3", "pero_EGF1_h_m1p0_p200000exe4", "pero_EGF1_h_m1p0_p200000exe5", "pero_EGF1_h_m1p0_p200000exe6", "pero_EGF1_h_m1p0_p200000exe7", "pero_EGF1_h_m1p0_p200000exe8", "pero_EGF1_h_m1p0_p200000exe9", "pero_EGF1_h_m1p0_p20000exe0", "pero_EGF1_h_m1p0_p20000exe1", "pero_EGF1_h_m1p0_p20000exe10", "pero_EGF1_h_m1p0_p20000exe11", "pero_EGF1_h_m1p0_p20000exe12", "pero_EGF1_h_m1p0_p20000exe13", "pero_EGF1_h_m1p0_p20000exe14", "pero_EGF1_h_m1p0_p20000exe15", "pero_EGF1_h_m1p0_p20000exe16", "pero_EGF1_h_m1p0_p20000exe2", "pero_EGF1_h_m1p0_p20000exe3", "pero_EGF1_h_m1p0_p20000exe4", "pero_EGF1_h_m1p0_p20000exe5", "pero_EGF1_h_m1p0_p20000exe6", "pero_EGF1_h_m1p0_p20000exe7", "pero_EGF1_h_m1p0_p20000exe8", "pero_EGF1_h_m1p0_p20000exe9", "pero_EGF1_h_m1p0_p2000exe0", "pero_EGF1_h_m1p0_p2000exe1", "pero_EGF1_h_m1p0_p2000exe10", "pero_EGF1_h_m1p0_p2000exe11", "pero_EGF1_h_m1p0_p2000exe12", "pero_EGF1_h_m1p0_p2000exe13", "pero_EGF1_h_m1p0_p2000exe14", "pero_EGF1_h_m1p0_p2000exe15", "pero_EGF1_h_m1p0_p2000exe16", "pero_EGF1_h_m1p0_p2000exe2", "pero_EGF1_h_m1p0_p2000exe3", "pero_EGF1_h_m1p0_p2000exe4", "pero_EGF1_h_m1p0_p2000exe5", "pero_EGF1_h_m1p0_p2000exe6", "pero_EGF1_h_m1p0_p2000exe7", "pero_EGF1_h_m1p0_p2000exe8", "pero_EGF1_h_m1p0_p2000exe9", "pero_EGF1_h_m1p0_p200exe0", "pero_EGF1_h_m1p0_p200exe1", "pero_EGF1_h_m1p0_p200exe10", "pero_EGF1_h_m1p0_p200exe11", "pero_EGF1_h_m1p0_p200exe12", "pero_EGF1_h_m1p0_p200exe13", "pero_EGF1_h_m1p0_p200exe14", "pero_EGF1_h_m1p0_p200exe15", "pero_EGF1_h_m1p0_p200exe16", "pero_EGF1_h_m1p0_p200exe2", "pero_EGF1_h_m1p0_p200exe3", "pero_EGF1_h_m1p0_p200exe4", "pero_EGF1_h_m1p0_p200exe5", "pero_EGF1_h_m1p0_p200exe6", "pero_EGF1_h_m1p0_p200exe7", "pero_EGF1_h_m1p0_p200exe8", "pero_EGF1_h_m1p0_p200exe9", "pero_EGF1_h_m1p0_p2100exe0", "pero_EGF1_h_m1p0_p2100exe1", "pero_EGF1_h_m1p0_p2100exe10", "pero_EGF1_h_m1p0_p2100exe11", "pero_EGF1_h_m1p0_p2100exe12", "pero_EGF1_h_m1p0_p2100exe13", "pero_EGF1_h_m1p0_p2100exe14", "pero_EGF1_h_m1p0_p2100exe15", "pero_EGF1_h_m1p0_p2100exe16", "pero_EGF1_h_m1p0_p2100exe2", "pero_EGF1_h_m1p0_p2100exe3", "pero_EGF1_h_m1p0_p2100exe4", "pero_EGF1_h_m1p0_p2100exe5", "pero_EGF1_h_m1p0_p2100exe6", "pero_EGF1_h_m1p0_p2100exe7", "pero_EGF1_h_m1p0_p2100exe8", "pero_EGF1_h_m1p0_p2100exe9", "pero_EGF1_h_m1p0_p220000exe0", "pero_EGF1_h_m1p0_p220000exe1", "pero_EGF1_h_m1p0_p220000exe10", "pero_EGF1_h_m1p0_p220000exe11", "pero_EGF1_h_m1p0_p220000exe12", "pero_EGF1_h_m1p0_p220000exe13", "pero_EGF1_h_m1p0_p220000exe14", "pero_EGF1_h_m1p0_p220000exe15", "pero_EGF1_h_m1p0_p220000exe16", "pero_EGF1_h_m1p0_p220000exe2", "pero_EGF1_h_m1p0_p220000exe3", "pero_EGF1_h_m1p0_p220000exe4", "pero_EGF1_h_m1p0_p220000exe5", "pero_EGF1_h_m1p0_p220000exe6", "pero_EGF1_h_m1p0_p220000exe7", "pero_EGF1_h_m1p0_p220000exe8", "pero_EGF1_h_m1p0_p220000exe9", "pero_EGF1_h_m1p0_p2200exe0", "pero_EGF1_h_m1p0_p2200exe1", "pero_EGF1_h_m1p0_p2200exe10", "pero_EGF1_h_m1p0_p2200exe11", "pero_EGF1_h_m1p0_p2200exe12", "pero_EGF1_h_m1p0_p2200exe13", "pero_EGF1_h_m1p0_p2200exe14", "pero_EGF1_h_m1p0_p2200exe15", "pero_EGF1_h_m1p0_p2200exe16", "pero_EGF1_h_m1p0_p2200exe2", "pero_EGF1_h_m1p0_p2200exe3", "pero_EGF1_h_m1p0_p2200exe4", "pero_EGF1_h_m1p0_p2200exe5", "pero_EGF1_h_m1p0_p2200exe6", "pero_EGF1_h_m1p0_p2200exe7", "pero_EGF1_h_m1p0_p2200exe8", "pero_EGF1_h_m1p0_p2200exe9", "pero_EGF1_h_m1p0_p2300exe0", "pero_EGF1_h_m1p0_p2300exe1", "pero_EGF1_h_m1p0_p2300exe10", "pero_EGF1_h_m1p0_p2300exe11", "pero_EGF1_h_m1p0_p2300exe12", "pero_EGF1_h_m1p0_p2300exe13", "pero_EGF1_h_m1p0_p2300exe14", "pero_EGF1_h_m1p0_p2300exe15", "pero_EGF1_h_m1p0_p2300exe16", "pero_EGF1_h_m1p0_p2300exe17", "pero_EGF1_h_m1p0_p2300exe2", "pero_EGF1_h_m1p0_p2300exe3", "pero_EGF1_h_m1p0_p2300exe4", "pero_EGF1_h_m1p0_p2300exe5", "pero_EGF1_h_m1p0_p2300exe6", "pero_EGF1_h_m1p0_p2300exe7", "pero_EGF1_h_m1p0_p2300exe8", "pero_EGF1_h_m1p0_p2300exe9", "pero_EGF1_h_m1p0_p240000exe0", "pero_EGF1_h_m1p0_p240000exe1", "pero_EGF1_h_m1p0_p240000exe10", "pero_EGF1_h_m1p0_p240000exe11", "pero_EGF1_h_m1p0_p240000exe12", "pero_EGF1_h_m1p0_p240000exe13", "pero_EGF1_h_m1p0_p240000exe14", "pero_EGF1_h_m1p0_p240000exe15", "pero_EGF1_h_m1p0_p240000exe16", "pero_EGF1_h_m1p0_p240000exe2", "pero_EGF1_h_m1p0_p240000exe3", "pero_EGF1_h_m1p0_p240000exe4", "pero_EGF1_h_m1p0_p240000exe5", "pero_EGF1_h_m1p0_p240000exe6", "pero_EGF1_h_m1p0_p240000exe7", "pero_EGF1_h_m1p0_p240000exe8", "pero_EGF1_h_m1p0_p240000exe9", "pero_EGF1_h_m1p0_p2400exe0", "pero_EGF1_h_m1p0_p2400exe1", "pero_EGF1_h_m1p0_p2400exe10", "pero_EGF1_h_m1p0_p2400exe11", "pero_EGF1_h_m1p0_p2400exe12", "pero_EGF1_h_m1p0_p2400exe13", "pero_EGF1_h_m1p0_p2400exe14", "pero_EGF1_h_m1p0_p2400exe15", "pero_EGF1_h_m1p0_p2400exe16", "pero_EGF1_h_m1p0_p2400exe2", "pero_EGF1_h_m1p0_p2400exe3", "pero_EGF1_h_m1p0_p2400exe4", "pero_EGF1_h_m1p0_p2400exe5", "pero_EGF1_h_m1p0_p2400exe6", "pero_EGF1_h_m1p0_p2400exe7", "pero_EGF1_h_m1p0_p2400exe8", "pero_EGF1_h_m1p0_p2400exe9", "pero_EGF1_h_m1p0_p2500exe0", "pero_EGF1_h_m1p0_p2500exe1", "pero_EGF1_h_m1p0_p2500exe10", "pero_EGF1_h_m1p0_p2500exe11", "pero_EGF1_h_m1p0_p2500exe12", "pero_EGF1_h_m1p0_p2500exe13", "pero_EGF1_h_m1p0_p2500exe14", "pero_EGF1_h_m1p0_p2500exe15", "pero_EGF1_h_m1p0_p2500exe16", "pero_EGF1_h_m1p0_p2500exe2", "pero_EGF1_h_m1p0_p2500exe3", "pero_EGF1_h_m1p0_p2500exe4", "pero_EGF1_h_m1p0_p2500exe5", "pero_EGF1_h_m1p0_p2500exe6", "pero_EGF1_h_m1p0_p2500exe7", "pero_EGF1_h_m1p0_p2500exe8", "pero_EGF1_h_m1p0_p2500exe9", "pero_EGF1_h_m1p0_p260000exe0", "pero_EGF1_h_m1p0_p260000exe1", "pero_EGF1_h_m1p0_p260000exe10", "pero_EGF1_h_m1p0_p260000exe11", "pero_EGF1_h_m1p0_p260000exe12", "pero_EGF1_h_m1p0_p260000exe13", "pero_EGF1_h_m1p0_p260000exe14", "pero_EGF1_h_m1p0_p260000exe15", "pero_EGF1_h_m1p0_p260000exe16", "pero_EGF1_h_m1p0_p260000exe2", "pero_EGF1_h_m1p0_p260000exe3", "pero_EGF1_h_m1p0_p260000exe4", "pero_EGF1_h_m1p0_p260000exe5", "pero_EGF1_h_m1p0_p260000exe6", "pero_EGF1_h_m1p0_p260000exe7", "pero_EGF1_h_m1p0_p260000exe8", "pero_EGF1_h_m1p0_p260000exe9", "pero_EGF1_h_m1p0_p2600exe0", "pero_EGF1_h_m1p0_p2600exe1", "pero_EGF1_h_m1p0_p2600exe10", "pero_EGF1_h_m1p0_p2600exe11", "pero_EGF1_h_m1p0_p2600exe12", "pero_EGF1_h_m1p0_p2600exe13", "pero_EGF1_h_m1p0_p2600exe14", "pero_EGF1_h_m1p0_p2600exe15", "pero_EGF1_h_m1p0_p2600exe16", "pero_EGF1_h_m1p0_p2600exe2", "pero_EGF1_h_m1p0_p2600exe3", "pero_EGF1_h_m1p0_p2600exe4", "pero_EGF1_h_m1p0_p2600exe5", "pero_EGF1_h_m1p0_p2600exe6", "pero_EGF1_h_m1p0_p2600exe7", "pero_EGF1_h_m1p0_p2600exe8", "pero_EGF1_h_m1p0_p2600exe9", "pero_EGF1_h_m1p0_p2700exe0", "pero_EGF1_h_m1p0_p2700exe1", "pero_EGF1_h_m1p0_p2700exe10", "pero_EGF1_h_m1p0_p2700exe11", "pero_EGF1_h_m1p0_p2700exe12", "pero_EGF1_h_m1p0_p2700exe13", "pero_EGF1_h_m1p0_p2700exe14", "pero_EGF1_h_m1p0_p2700exe15", "pero_EGF1_h_m1p0_p2700exe16", "pero_EGF1_h_m1p0_p2700exe2", "pero_EGF1_h_m1p0_p2700exe3", "pero_EGF1_h_m1p0_p2700exe4", "pero_EGF1_h_m1p0_p2700exe5", "pero_EGF1_h_m1p0_p2700exe6", "pero_EGF1_h_m1p0_p2700exe7", "pero_EGF1_h_m1p0_p2700exe8", "pero_EGF1_h_m1p0_p2700exe9", "pero_EGF1_h_m1p0_p280000exe0", "pero_EGF1_h_m1p0_p280000exe1", "pero_EGF1_h_m1p0_p280000exe10", "pero_EGF1_h_m1p0_p280000exe11", "pero_EGF1_h_m1p0_p280000exe12", "pero_EGF1_h_m1p0_p280000exe13", "pero_EGF1_h_m1p0_p280000exe14", "pero_EGF1_h_m1p0_p280000exe15", "pero_EGF1_h_m1p0_p280000exe16", "pero_EGF1_h_m1p0_p280000exe2", "pero_EGF1_h_m1p0_p280000exe3", "pero_EGF1_h_m1p0_p280000exe4", "pero_EGF1_h_m1p0_p280000exe5", "pero_EGF1_h_m1p0_p280000exe6", "pero_EGF1_h_m1p0_p280000exe7", "pero_EGF1_h_m1p0_p280000exe8", "pero_EGF1_h_m1p0_p280000exe9", "pero_EGF1_h_m1p0_p2800exe0", "pero_EGF1_h_m1p0_p2800exe1", "pero_EGF1_h_m1p0_p2800exe10", "pero_EGF1_h_m1p0_p2800exe11", "pero_EGF1_h_m1p0_p2800exe12", "pero_EGF1_h_m1p0_p2800exe13", "pero_EGF1_h_m1p0_p2800exe14", "pero_EGF1_h_m1p0_p2800exe15", "pero_EGF1_h_m1p0_p2800exe16", "pero_EGF1_h_m1p0_p2800exe2", "pero_EGF1_h_m1p0_p2800exe3", "pero_EGF1_h_m1p0_p2800exe4", "pero_EGF1_h_m1p0_p2800exe5", "pero_EGF1_h_m1p0_p2800exe6", "pero_EGF1_h_m1p0_p2800exe7", "pero_EGF1_h_m1p0_p2800exe8", "pero_EGF1_h_m1p0_p2800exe9", "pero_EGF1_h_m1p0_p2900exe0", "pero_EGF1_h_m1p0_p2900exe1", "pero_EGF1_h_m1p0_p2900exe10", "pero_EGF1_h_m1p0_p2900exe11", "pero_EGF1_h_m1p0_p2900exe12", "pero_EGF1_h_m1p0_p2900exe13", "pero_EGF1_h_m1p0_p2900exe14", "pero_EGF1_h_m1p0_p2900exe15", "pero_EGF1_h_m1p0_p2900exe16", "pero_EGF1_h_m1p0_p2900exe2", "pero_EGF1_h_m1p0_p2900exe3", "pero_EGF1_h_m1p0_p2900exe4", "pero_EGF1_h_m1p0_p2900exe5", "pero_EGF1_h_m1p0_p2900exe6", "pero_EGF1_h_m1p0_p2900exe7", "pero_EGF1_h_m1p0_p2900exe8", "pero_EGF1_h_m1p0_p2900exe9", "pero_EGF1_h_m1p0_p300000exe0", "pero_EGF1_h_m1p0_p300000exe1", "pero_EGF1_h_m1p0_p300000exe10", "pero_EGF1_h_m1p0_p300000exe11", "pero_EGF1_h_m1p0_p300000exe12", "pero_EGF1_h_m1p0_p300000exe13", "pero_EGF1_h_m1p0_p300000exe14", "pero_EGF1_h_m1p0_p300000exe15", "pero_EGF1_h_m1p0_p300000exe16", "pero_EGF1_h_m1p0_p300000exe2", "pero_EGF1_h_m1p0_p300000exe3", "pero_EGF1_h_m1p0_p300000exe4", "pero_EGF1_h_m1p0_p300000exe5", "pero_EGF1_h_m1p0_p300000exe6", "pero_EGF1_h_m1p0_p300000exe7", "pero_EGF1_h_m1p0_p300000exe8", "pero_EGF1_h_m1p0_p300000exe9", "pero_EGF1_h_m1p0_p30000exe0", "pero_EGF1_h_m1p0_p30000exe1", "pero_EGF1_h_m1p0_p30000exe10", "pero_EGF1_h_m1p0_p30000exe11", "pero_EGF1_h_m1p0_p30000exe12", "pero_EGF1_h_m1p0_p30000exe13", "pero_EGF1_h_m1p0_p30000exe14", "pero_EGF1_h_m1p0_p30000exe15", "pero_EGF1_h_m1p0_p30000exe16", "pero_EGF1_h_m1p0_p30000exe2", "pero_EGF1_h_m1p0_p30000exe3", "pero_EGF1_h_m1p0_p30000exe4", "pero_EGF1_h_m1p0_p30000exe5", "pero_EGF1_h_m1p0_p30000exe6", "pero_EGF1_h_m1p0_p30000exe7", "pero_EGF1_h_m1p0_p30000exe8", "pero_EGF1_h_m1p0_p30000exe9", "pero_EGF1_h_m1p0_p3000exe0", "pero_EGF1_h_m1p0_p3000exe1", "pero_EGF1_h_m1p0_p3000exe10", "pero_EGF1_h_m1p0_p3000exe11", "pero_EGF1_h_m1p0_p3000exe12", "pero_EGF1_h_m1p0_p3000exe13", "pero_EGF1_h_m1p0_p3000exe14", "pero_EGF1_h_m1p0_p3000exe15", "pero_EGF1_h_m1p0_p3000exe16", "pero_EGF1_h_m1p0_p3000exe17", "pero_EGF1_h_m1p0_p3000exe2", "pero_EGF1_h_m1p0_p3000exe3", "pero_EGF1_h_m1p0_p3000exe4", "pero_EGF1_h_m1p0_p3000exe5", "pero_EGF1_h_m1p0_p3000exe6", "pero_EGF1_h_m1p0_p3000exe7", "pero_EGF1_h_m1p0_p3000exe8", "pero_EGF1_h_m1p0_p3000exe9", "pero_EGF1_h_m1p0_p300exe0", "pero_EGF1_h_m1p0_p300exe1", "pero_EGF1_h_m1p0_p300exe10", "pero_EGF1_h_m1p0_p300exe11", "pero_EGF1_h_m1p0_p300exe12", "pero_EGF1_h_m1p0_p300exe13", "pero_EGF1_h_m1p0_p300exe14", "pero_EGF1_h_m1p0_p300exe15", "pero_EGF1_h_m1p0_p300exe16", "pero_EGF1_h_m1p0_p300exe2", "pero_EGF1_h_m1p0_p300exe3", "pero_EGF1_h_m1p0_p300exe4", "pero_EGF1_h_m1p0_p300exe5", "pero_EGF1_h_m1p0_p300exe6", "pero_EGF1_h_m1p0_p300exe7", "pero_EGF1_h_m1p0_p300exe8", "pero_EGF1_h_m1p0_p300exe9", "pero_EGF1_h_m1p0_p320000exe0", "pero_EGF1_h_m1p0_p320000exe1", "pero_EGF1_h_m1p0_p320000exe10", "pero_EGF1_h_m1p0_p320000exe11", "pero_EGF1_h_m1p0_p320000exe12", "pero_EGF1_h_m1p0_p320000exe13", "pero_EGF1_h_m1p0_p320000exe14", "pero_EGF1_h_m1p0_p320000exe15", "pero_EGF1_h_m1p0_p320000exe16", "pero_EGF1_h_m1p0_p320000exe2", "pero_EGF1_h_m1p0_p320000exe3", "pero_EGF1_h_m1p0_p320000exe4", "pero_EGF1_h_m1p0_p320000exe5", "pero_EGF1_h_m1p0_p320000exe6", "pero_EGF1_h_m1p0_p320000exe7", "pero_EGF1_h_m1p0_p320000exe8", "pero_EGF1_h_m1p0_p320000exe9", "pero_EGF1_h_m1p0_p340000exe0", "pero_EGF1_h_m1p0_p340000exe1", "pero_EGF1_h_m1p0_p340000exe10", "pero_EGF1_h_m1p0_p340000exe11", "pero_EGF1_h_m1p0_p340000exe12", "pero_EGF1_h_m1p0_p340000exe13", "pero_EGF1_h_m1p0_p340000exe14", "pero_EGF1_h_m1p0_p340000exe15", "pero_EGF1_h_m1p0_p340000exe16", "pero_EGF1_h_m1p0_p340000exe2", "pero_EGF1_h_m1p0_p340000exe3", "pero_EGF1_h_m1p0_p340000exe4", "pero_EGF1_h_m1p0_p340000exe5", "pero_EGF1_h_m1p0_p340000exe6", "pero_EGF1_h_m1p0_p340000exe7", "pero_EGF1_h_m1p0_p340000exe8", "pero_EGF1_h_m1p0_p340000exe9", "pero_EGF1_h_m1p0_p360000exe0", "pero_EGF1_h_m1p0_p360000exe1", "pero_EGF1_h_m1p0_p360000exe10", "pero_EGF1_h_m1p0_p360000exe11", "pero_EGF1_h_m1p0_p360000exe12", "pero_EGF1_h_m1p0_p360000exe13", "pero_EGF1_h_m1p0_p360000exe14", "pero_EGF1_h_m1p0_p360000exe15", "pero_EGF1_h_m1p0_p360000exe16", "pero_EGF1_h_m1p0_p360000exe2", "pero_EGF1_h_m1p0_p360000exe3", "pero_EGF1_h_m1p0_p360000exe4", "pero_EGF1_h_m1p0_p360000exe5", "pero_EGF1_h_m1p0_p360000exe6", "pero_EGF1_h_m1p0_p360000exe7", "pero_EGF1_h_m1p0_p360000exe8", "pero_EGF1_h_m1p0_p360000exe9", "pero_EGF1_h_m1p0_p380000exe0", "pero_EGF1_h_m1p0_p380000exe1", "pero_EGF1_h_m1p0_p380000exe10", "pero_EGF1_h_m1p0_p380000exe11", "pero_EGF1_h_m1p0_p380000exe12", "pero_EGF1_h_m1p0_p380000exe13", "pero_EGF1_h_m1p0_p380000exe14", "pero_EGF1_h_m1p0_p380000exe15", "pero_EGF1_h_m1p0_p380000exe16", "pero_EGF1_h_m1p0_p380000exe2", "pero_EGF1_h_m1p0_p380000exe3", "pero_EGF1_h_m1p0_p380000exe4", "pero_EGF1_h_m1p0_p380000exe5", "pero_EGF1_h_m1p0_p380000exe6", "pero_EGF1_h_m1p0_p380000exe7", "pero_EGF1_h_m1p0_p380000exe8", "pero_EGF1_h_m1p0_p380000exe9", "pero_EGF1_h_m1p0_p400000exe0", "pero_EGF1_h_m1p0_p400000exe1", "pero_EGF1_h_m1p0_p400000exe10", "pero_EGF1_h_m1p0_p400000exe11", "pero_EGF1_h_m1p0_p400000exe12", "pero_EGF1_h_m1p0_p400000exe13", "pero_EGF1_h_m1p0_p400000exe14", "pero_EGF1_h_m1p0_p400000exe15", "pero_EGF1_h_m1p0_p400000exe16", "pero_EGF1_h_m1p0_p400000exe2", "pero_EGF1_h_m1p0_p400000exe3", "pero_EGF1_h_m1p0_p400000exe4", "pero_EGF1_h_m1p0_p400000exe5", "pero_EGF1_h_m1p0_p400000exe6", "pero_EGF1_h_m1p0_p400000exe7", "pero_EGF1_h_m1p0_p400000exe8", "pero_EGF1_h_m1p0_p400000exe9", "pero_EGF1_h_m1p0_p40000exe0", "pero_EGF1_h_m1p0_p40000exe1", "pero_EGF1_h_m1p0_p40000exe10", "pero_EGF1_h_m1p0_p40000exe11", "pero_EGF1_h_m1p0_p40000exe12", "pero_EGF1_h_m1p0_p40000exe13", "pero_EGF1_h_m1p0_p40000exe14", "pero_EGF1_h_m1p0_p40000exe15", "pero_EGF1_h_m1p0_p40000exe16", "pero_EGF1_h_m1p0_p40000exe2", "pero_EGF1_h_m1p0_p40000exe3", "pero_EGF1_h_m1p0_p40000exe4", "pero_EGF1_h_m1p0_p40000exe5", "pero_EGF1_h_m1p0_p40000exe6", "pero_EGF1_h_m1p0_p40000exe7", "pero_EGF1_h_m1p0_p40000exe8", "pero_EGF1_h_m1p0_p40000exe9", "pero_EGF1_h_m1p0_p4000exe0", "pero_EGF1_h_m1p0_p4000exe1", "pero_EGF1_h_m1p0_p4000exe10", "pero_EGF1_h_m1p0_p4000exe11", "pero_EGF1_h_m1p0_p4000exe12", "pero_EGF1_h_m1p0_p4000exe13", "pero_EGF1_h_m1p0_p4000exe14", "pero_EGF1_h_m1p0_p4000exe15", "pero_EGF1_h_m1p0_p4000exe16", "pero_EGF1_h_m1p0_p4000exe2", "pero_EGF1_h_m1p0_p4000exe3", "pero_EGF1_h_m1p0_p4000exe4", "pero_EGF1_h_m1p0_p4000exe5", "pero_EGF1_h_m1p0_p4000exe6", "pero_EGF1_h_m1p0_p4000exe7", "pero_EGF1_h_m1p0_p4000exe8", "pero_EGF1_h_m1p0_p4000exe9", "pero_EGF1_h_m1p0_p400exe0", "pero_EGF1_h_m1p0_p400exe1", "pero_EGF1_h_m1p0_p400exe10", "pero_EGF1_h_m1p0_p400exe11", "pero_EGF1_h_m1p0_p400exe12", "pero_EGF1_h_m1p0_p400exe13", "pero_EGF1_h_m1p0_p400exe14", "pero_EGF1_h_m1p0_p400exe15", "pero_EGF1_h_m1p0_p400exe16", "pero_EGF1_h_m1p0_p400exe2", "pero_EGF1_h_m1p0_p400exe3", "pero_EGF1_h_m1p0_p400exe4", "pero_EGF1_h_m1p0_p400exe5", "pero_EGF1_h_m1p0_p400exe6", "pero_EGF1_h_m1p0_p400exe7", "pero_EGF1_h_m1p0_p400exe8", "pero_EGF1_h_m1p0_p400exe9", "pero_EGF1_h_m1p0_p420000exe0", "pero_EGF1_h_m1p0_p420000exe1", "pero_EGF1_h_m1p0_p420000exe10", "pero_EGF1_h_m1p0_p420000exe11", "pero_EGF1_h_m1p0_p420000exe12", "pero_EGF1_h_m1p0_p420000exe13", "pero_EGF1_h_m1p0_p420000exe14", "pero_EGF1_h_m1p0_p420000exe15", "pero_EGF1_h_m1p0_p420000exe16", "pero_EGF1_h_m1p0_p420000exe2", "pero_EGF1_h_m1p0_p420000exe3", "pero_EGF1_h_m1p0_p420000exe4", "pero_EGF1_h_m1p0_p420000exe5", "pero_EGF1_h_m1p0_p420000exe6", "pero_EGF1_h_m1p0_p420000exe7", "pero_EGF1_h_m1p0_p420000exe8", "pero_EGF1_h_m1p0_p420000exe9", "pero_EGF1_h_m1p0_p440000exe0", "pero_EGF1_h_m1p0_p440000exe1", "pero_EGF1_h_m1p0_p440000exe10", "pero_EGF1_h_m1p0_p440000exe11", "pero_EGF1_h_m1p0_p440000exe12", "pero_EGF1_h_m1p0_p440000exe13", "pero_EGF1_h_m1p0_p440000exe14", "pero_EGF1_h_m1p0_p440000exe15", "pero_EGF1_h_m1p0_p440000exe16", "pero_EGF1_h_m1p0_p440000exe2", "pero_EGF1_h_m1p0_p440000exe3", "pero_EGF1_h_m1p0_p440000exe4", "pero_EGF1_h_m1p0_p440000exe5", "pero_EGF1_h_m1p0_p440000exe6", "pero_EGF1_h_m1p0_p440000exe7", "pero_EGF1_h_m1p0_p440000exe8", "pero_EGF1_h_m1p0_p440000exe9", "pero_EGF1_h_m1p0_p480000exe0", "pero_EGF1_h_m1p0_p480000exe1", "pero_EGF1_h_m1p0_p480000exe10", "pero_EGF1_h_m1p0_p480000exe11", "pero_EGF1_h_m1p0_p480000exe12", "pero_EGF1_h_m1p0_p480000exe13", "pero_EGF1_h_m1p0_p480000exe14", "pero_EGF1_h_m1p0_p480000exe15", "pero_EGF1_h_m1p0_p480000exe16", "pero_EGF1_h_m1p0_p480000exe2", "pero_EGF1_h_m1p0_p480000exe3", "pero_EGF1_h_m1p0_p480000exe4", "pero_EGF1_h_m1p0_p480000exe5", "pero_EGF1_h_m1p0_p480000exe6", "pero_EGF1_h_m1p0_p480000exe7", "pero_EGF1_h_m1p0_p480000exe8", "pero_EGF1_h_m1p0_p480000exe9", "pero_EGF1_h_m1p0_p500000exe0", "pero_EGF1_h_m1p0_p500000exe1", "pero_EGF1_h_m1p0_p500000exe10", "pero_EGF1_h_m1p0_p500000exe11", "pero_EGF1_h_m1p0_p500000exe12", "pero_EGF1_h_m1p0_p500000exe13", "pero_EGF1_h_m1p0_p500000exe14", "pero_EGF1_h_m1p0_p500000exe15", "pero_EGF1_h_m1p0_p500000exe16", "pero_EGF1_h_m1p0_p500000exe2", "pero_EGF1_h_m1p0_p500000exe3", "pero_EGF1_h_m1p0_p500000exe4", "pero_EGF1_h_m1p0_p500000exe5", "pero_EGF1_h_m1p0_p500000exe6", "pero_EGF1_h_m1p0_p500000exe7", "pero_EGF1_h_m1p0_p500000exe8", "pero_EGF1_h_m1p0_p500000exe9", "pero_EGF1_h_m1p0_p50000exe0", "pero_EGF1_h_m1p0_p50000exe1", "pero_EGF1_h_m1p0_p50000exe10", "pero_EGF1_h_m1p0_p50000exe11", "pero_EGF1_h_m1p0_p50000exe12", "pero_EGF1_h_m1p0_p50000exe13", "pero_EGF1_h_m1p0_p50000exe14", "pero_EGF1_h_m1p0_p50000exe15", "pero_EGF1_h_m1p0_p50000exe16", "pero_EGF1_h_m1p0_p50000exe2", "pero_EGF1_h_m1p0_p50000exe3", "pero_EGF1_h_m1p0_p50000exe4", "pero_EGF1_h_m1p0_p50000exe5", "pero_EGF1_h_m1p0_p50000exe6", "pero_EGF1_h_m1p0_p50000exe7", "pero_EGF1_h_m1p0_p50000exe8", "pero_EGF1_h_m1p0_p50000exe9", "pero_EGF1_h_m1p0_p500exe0", "pero_EGF1_h_m1p0_p500exe1", "pero_EGF1_h_m1p0_p500exe10", "pero_EGF1_h_m1p0_p500exe11", "pero_EGF1_h_m1p0_p500exe12", "pero_EGF1_h_m1p0_p500exe13", "pero_EGF1_h_m1p0_p500exe14", "pero_EGF1_h_m1p0_p500exe15", "pero_EGF1_h_m1p0_p500exe16", "pero_EGF1_h_m1p0_p500exe2", "pero_EGF1_h_m1p0_p500exe3", "pero_EGF1_h_m1p0_p500exe4", "pero_EGF1_h_m1p0_p500exe5", "pero_EGF1_h_m1p0_p500exe6", "pero_EGF1_h_m1p0_p500exe7", "pero_EGF1_h_m1p0_p500exe8", "pero_EGF1_h_m1p0_p500exe9", "pero_EGF1_h_m1p0_p60000exe0", "pero_EGF1_h_m1p0_p60000exe1", "pero_EGF1_h_m1p0_p60000exe10", "pero_EGF1_h_m1p0_p60000exe11", "pero_EGF1_h_m1p0_p60000exe12", "pero_EGF1_h_m1p0_p60000exe13", "pero_EGF1_h_m1p0_p60000exe14", "pero_EGF1_h_m1p0_p60000exe15", "pero_EGF1_h_m1p0_p60000exe16", "pero_EGF1_h_m1p0_p60000exe2", "pero_EGF1_h_m1p0_p60000exe3", "pero_EGF1_h_m1p0_p60000exe4", "pero_EGF1_h_m1p0_p60000exe5", "pero_EGF1_h_m1p0_p60000exe6", "pero_EGF1_h_m1p0_p60000exe7", "pero_EGF1_h_m1p0_p60000exe8", "pero_EGF1_h_m1p0_p60000exe9", "pero_EGF1_h_m1p0_p6000exe0", "pero_EGF1_h_m1p0_p6000exe1", "pero_EGF1_h_m1p0_p6000exe10", "pero_EGF1_h_m1p0_p6000exe11", "pero_EGF1_h_m1p0_p6000exe12", "pero_EGF1_h_m1p0_p6000exe13", "pero_EGF1_h_m1p0_p6000exe14", "pero_EGF1_h_m1p0_p6000exe15", "pero_EGF1_h_m1p0_p6000exe16", "pero_EGF1_h_m1p0_p6000exe2", "pero_EGF1_h_m1p0_p6000exe3", "pero_EGF1_h_m1p0_p6000exe4", "pero_EGF1_h_m1p0_p6000exe5", "pero_EGF1_h_m1p0_p6000exe6", "pero_EGF1_h_m1p0_p6000exe7", "pero_EGF1_h_m1p0_p6000exe8", "pero_EGF1_h_m1p0_p6000exe9", "pero_EGF1_h_m1p0_p600exe0", "pero_EGF1_h_m1p0_p600exe1", "pero_EGF1_h_m1p0_p600exe10", "pero_EGF1_h_m1p0_p600exe11", "pero_EGF1_h_m1p0_p600exe12", "pero_EGF1_h_m1p0_p600exe13", "pero_EGF1_h_m1p0_p600exe14", "pero_EGF1_h_m1p0_p600exe15", "pero_EGF1_h_m1p0_p600exe16", "pero_EGF1_h_m1p0_p600exe17", "pero_EGF1_h_m1p0_p600exe2", "pero_EGF1_h_m1p0_p600exe3", "pero_EGF1_h_m1p0_p600exe4", "pero_EGF1_h_m1p0_p600exe5", "pero_EGF1_h_m1p0_p600exe6", "pero_EGF1_h_m1p0_p600exe7", "pero_EGF1_h_m1p0_p600exe8", "pero_EGF1_h_m1p0_p600exe9", "pero_EGF1_h_m1p0_p700exe0", "pero_EGF1_h_m1p0_p700exe1", "pero_EGF1_h_m1p0_p700exe10", "pero_EGF1_h_m1p0_p700exe11", "pero_EGF1_h_m1p0_p700exe12", "pero_EGF1_h_m1p0_p700exe13", "pero_EGF1_h_m1p0_p700exe14", "pero_EGF1_h_m1p0_p700exe15", "pero_EGF1_h_m1p0_p700exe16", "pero_EGF1_h_m1p0_p700exe2", "pero_EGF1_h_m1p0_p700exe3", "pero_EGF1_h_m1p0_p700exe4", "pero_EGF1_h_m1p0_p700exe5", "pero_EGF1_h_m1p0_p700exe6", "pero_EGF1_h_m1p0_p700exe7", "pero_EGF1_h_m1p0_p700exe8", "pero_EGF1_h_m1p0_p700exe9", "pero_EGF1_h_m1p0_p80000exe0", "pero_EGF1_h_m1p0_p80000exe1", "pero_EGF1_h_m1p0_p80000exe10", "pero_EGF1_h_m1p0_p80000exe11", "pero_EGF1_h_m1p0_p80000exe12", "pero_EGF1_h_m1p0_p80000exe13", "pero_EGF1_h_m1p0_p80000exe14", "pero_EGF1_h_m1p0_p80000exe15", "pero_EGF1_h_m1p0_p80000exe16", "pero_EGF1_h_m1p0_p80000exe2", "pero_EGF1_h_m1p0_p80000exe3", "pero_EGF1_h_m1p0_p80000exe4", "pero_EGF1_h_m1p0_p80000exe5", "pero_EGF1_h_m1p0_p80000exe6", "pero_EGF1_h_m1p0_p80000exe7", "pero_EGF1_h_m1p0_p80000exe8", "pero_EGF1_h_m1p0_p80000exe9", "pero_EGF1_h_m1p0_p800exe0", "pero_EGF1_h_m1p0_p800exe1", "pero_EGF1_h_m1p0_p800exe10", "pero_EGF1_h_m1p0_p800exe11", "pero_EGF1_h_m1p0_p800exe12", "pero_EGF1_h_m1p0_p800exe13", "pero_EGF1_h_m1p0_p800exe14", "pero_EGF1_h_m1p0_p800exe15", "pero_EGF1_h_m1p0_p800exe16", "pero_EGF1_h_m1p0_p800exe2", "pero_EGF1_h_m1p0_p800exe3", "pero_EGF1_h_m1p0_p800exe4", "pero_EGF1_h_m1p0_p800exe5", "pero_EGF1_h_m1p0_p800exe6", "pero_EGF1_h_m1p0_p800exe7", "pero_EGF1_h_m1p0_p800exe8", "pero_EGF1_h_m1p0_p800exe9", "pero_EGF1_h_m1p0_p900exe0", "pero_EGF1_h_m1p0_p900exe1", "pero_EGF1_h_m1p0_p900exe10", "pero_EGF1_h_m1p0_p900exe11", "pero_EGF1_h_m1p0_p900exe12", "pero_EGF1_h_m1p0_p900exe13", "pero_EGF1_h_m1p0_p900exe14", "pero_EGF1_h_m1p0_p900exe15", "pero_EGF1_h_m1p0_p900exe16", "pero_EGF1_h_m1p0_p900exe2", "pero_EGF1_h_m1p0_p900exe3", "pero_EGF1_h_m1p0_p900exe4", "pero_EGF1_h_m1p0_p900exe5", "pero_EGF1_h_m1p0_p900exe6", "pero_EGF1_h_m1p0_p900exe7", "pero_EGF1_h_m1p0_p900exe8", "pero_EGF1_h_m1p0_p900exe9", "pero_EGF1_h_m1p1_m0exe0", "pero_EGF1_h_m1p1_m0exe1", "pero_EGF1_h_m1p1_m0exe10", "pero_EGF1_h_m1p1_m0exe11", "pero_EGF1_h_m1p1_m0exe12", "pero_EGF1_h_m1p1_m0exe13", "pero_EGF1_h_m1p1_m0exe14", "pero_EGF1_h_m1p1_m0exe15", "pero_EGF1_h_m1p1_m0exe16", "pero_EGF1_h_m1p1_m0exe2", "pero_EGF1_h_m1p1_m0exe3", "pero_EGF1_h_m1p1_m0exe4", "pero_EGF1_h_m1p1_m0exe5", "pero_EGF1_h_m1p1_m0exe6", "pero_EGF1_h_m1p1_m0exe7", "pero_EGF1_h_m1p1_m0exe8", "pero_EGF1_h_m1p1_m0exe9", "pero_EGF1_h_m1p1_m100exe0", "pero_EGF1_h_m1p1_m100exe1", "pero_EGF1_h_m1p1_m100exe10", "pero_EGF1_h_m1p1_m100exe11", "pero_EGF1_h_m1p1_m100exe12", "pero_EGF1_h_m1p1_m100exe13", "pero_EGF1_h_m1p1_m100exe14", "pero_EGF1_h_m1p1_m100exe15", "pero_EGF1_h_m1p1_m100exe16", "pero_EGF1_h_m1p1_m100exe2", "pero_EGF1_h_m1p1_m100exe3", "pero_EGF1_h_m1p1_m100exe4", "pero_EGF1_h_m1p1_m100exe5", "pero_EGF1_h_m1p1_m100exe6", "pero_EGF1_h_m1p1_m100exe7", "pero_EGF1_h_m1p1_m100exe8", "pero_EGF1_h_m1p1_m100exe9", "pero_EGF1_h_m1p1_m200exe0", "pero_EGF1_h_m1p1_m200exe1", "pero_EGF1_h_m1p1_m200exe10", "pero_EGF1_h_m1p1_m200exe11", "pero_EGF1_h_m1p1_m200exe12", "pero_EGF1_h_m1p1_m200exe13", "pero_EGF1_h_m1p1_m200exe14", "pero_EGF1_h_m1p1_m200exe15", "pero_EGF1_h_m1p1_m200exe16", "pero_EGF1_h_m1p1_m200exe2", "pero_EGF1_h_m1p1_m200exe3", "pero_EGF1_h_m1p1_m200exe4", "pero_EGF1_h_m1p1_m200exe5", "pero_EGF1_h_m1p1_m200exe6", "pero_EGF1_h_m1p1_m200exe7", "pero_EGF1_h_m1p1_m200exe8", "pero_EGF1_h_m1p1_m200exe9", "pero_EGF1_h_m1p1_m300exe0", "pero_EGF1_h_m1p1_m300exe1", "pero_EGF1_h_m1p1_m300exe10", "pero_EGF1_h_m1p1_m300exe11", "pero_EGF1_h_m1p1_m300exe12", "pero_EGF1_h_m1p1_m300exe13", "pero_EGF1_h_m1p1_m300exe14", "pero_EGF1_h_m1p1_m300exe15", "pero_EGF1_h_m1p1_m300exe16", "pero_EGF1_h_m1p1_m300exe2", "pero_EGF1_h_m1p1_m300exe3", "pero_EGF1_h_m1p1_m300exe4", "pero_EGF1_h_m1p1_m300exe5", "pero_EGF1_h_m1p1_m300exe6", "pero_EGF1_h_m1p1_m300exe7", "pero_EGF1_h_m1p1_m300exe8", "pero_EGF1_h_m1p1_m300exe9", "pero_EGF1_h_m1p1_m5000exe0", "pero_EGF1_h_m1p1_m5000exe1", "pero_EGF1_h_m1p1_m5000exe10", "pero_EGF1_h_m1p1_m5000exe11", "pero_EGF1_h_m1p1_m5000exe12", "pero_EGF1_h_m1p1_m5000exe13", "pero_EGF1_h_m1p1_m5000exe14", "pero_EGF1_h_m1p1_m5000exe15", "pero_EGF1_h_m1p1_m5000exe16", "pero_EGF1_h_m1p1_m5000exe2", "pero_EGF1_h_m1p1_m5000exe3", "pero_EGF1_h_m1p1_m5000exe4", "pero_EGF1_h_m1p1_m5000exe5", "pero_EGF1_h_m1p1_m5000exe6", "pero_EGF1_h_m1p1_m5000exe7", "pero_EGF1_h_m1p1_m5000exe8", "pero_EGF1_h_m1p1_m5000exe9", "pero_EGF1_h_m1p1_m500exe0", "pero_EGF1_h_m1p1_m500exe1", "pero_EGF1_h_m1p1_m500exe10", "pero_EGF1_h_m1p1_m500exe11", "pero_EGF1_h_m1p1_m500exe12", "pero_EGF1_h_m1p1_m500exe13", "pero_EGF1_h_m1p1_m500exe14", "pero_EGF1_h_m1p1_m500exe15", "pero_EGF1_h_m1p1_m500exe16", "pero_EGF1_h_m1p1_m500exe2", "pero_EGF1_h_m1p1_m500exe3", "pero_EGF1_h_m1p1_m500exe4", "pero_EGF1_h_m1p1_m500exe5", "pero_EGF1_h_m1p1_m500exe6", "pero_EGF1_h_m1p1_m500exe7", "pero_EGF1_h_m1p1_m500exe8", "pero_EGF1_h_m1p1_m500exe9", "pero_EGF1_h_m1p1_p100000exe0", "pero_EGF1_h_m1p1_p100000exe1", "pero_EGF1_h_m1p1_p100000exe10", "pero_EGF1_h_m1p1_p100000exe11", "pero_EGF1_h_m1p1_p100000exe12", "pero_EGF1_h_m1p1_p100000exe13", "pero_EGF1_h_m1p1_p100000exe14", "pero_EGF1_h_m1p1_p100000exe15", "pero_EGF1_h_m1p1_p100000exe16", "pero_EGF1_h_m1p1_p100000exe2", "pero_EGF1_h_m1p1_p100000exe3", "pero_EGF1_h_m1p1_p100000exe4", "pero_EGF1_h_m1p1_p100000exe5", "pero_EGF1_h_m1p1_p100000exe6", "pero_EGF1_h_m1p1_p100000exe7", "pero_EGF1_h_m1p1_p100000exe8", "pero_EGF1_h_m1p1_p100000exe9", "pero_EGF1_h_m1p1_p10000exe0", "pero_EGF1_h_m1p1_p10000exe1", "pero_EGF1_h_m1p1_p10000exe10", "pero_EGF1_h_m1p1_p10000exe11", "pero_EGF1_h_m1p1_p10000exe12", "pero_EGF1_h_m1p1_p10000exe13", "pero_EGF1_h_m1p1_p10000exe14", "pero_EGF1_h_m1p1_p10000exe15", "pero_EGF1_h_m1p1_p10000exe16", "pero_EGF1_h_m1p1_p10000exe2", "pero_EGF1_h_m1p1_p10000exe3", "pero_EGF1_h_m1p1_p10000exe4", "pero_EGF1_h_m1p1_p10000exe5", "pero_EGF1_h_m1p1_p10000exe6", "pero_EGF1_h_m1p1_p10000exe7", "pero_EGF1_h_m1p1_p10000exe8", "pero_EGF1_h_m1p1_p10000exe9", "pero_EGF1_h_m1p1_p1000exe0", "pero_EGF1_h_m1p1_p1000exe1", "pero_EGF1_h_m1p1_p1000exe10", "pero_EGF1_h_m1p1_p1000exe11", "pero_EGF1_h_m1p1_p1000exe12", "pero_EGF1_h_m1p1_p1000exe13", "pero_EGF1_h_m1p1_p1000exe14", "pero_EGF1_h_m1p1_p1000exe15", "pero_EGF1_h_m1p1_p1000exe16", "pero_EGF1_h_m1p1_p1000exe17", "pero_EGF1_h_m1p1_p1000exe2", "pero_EGF1_h_m1p1_p1000exe3", "pero_EGF1_h_m1p1_p1000exe4", "pero_EGF1_h_m1p1_p1000exe5", "pero_EGF1_h_m1p1_p1000exe6", "pero_EGF1_h_m1p1_p1000exe7", "pero_EGF1_h_m1p1_p1000exe8", "pero_EGF1_h_m1p1_p1000exe9", "pero_EGF1_h_m1p1_p100exe0", "pero_EGF1_h_m1p1_p100exe1", "pero_EGF1_h_m1p1_p100exe10", "pero_EGF1_h_m1p1_p100exe11", "pero_EGF1_h_m1p1_p100exe12", "pero_EGF1_h_m1p1_p100exe13", "pero_EGF1_h_m1p1_p100exe14", "pero_EGF1_h_m1p1_p100exe15", "pero_EGF1_h_m1p1_p100exe16", "pero_EGF1_h_m1p1_p100exe2", "pero_EGF1_h_m1p1_p100exe3", "pero_EGF1_h_m1p1_p100exe4", "pero_EGF1_h_m1p1_p100exe5", "pero_EGF1_h_m1p1_p100exe6", "pero_EGF1_h_m1p1_p100exe7", "pero_EGF1_h_m1p1_p100exe8", "pero_EGF1_h_m1p1_p100exe9", "pero_EGF1_h_m1p1_p1100exe0", "pero_EGF1_h_m1p1_p1100exe1", "pero_EGF1_h_m1p1_p1100exe10", "pero_EGF1_h_m1p1_p1100exe11", "pero_EGF1_h_m1p1_p1100exe12", "pero_EGF1_h_m1p1_p1100exe13", "pero_EGF1_h_m1p1_p1100exe14", "pero_EGF1_h_m1p1_p1100exe15", "pero_EGF1_h_m1p1_p1100exe16", "pero_EGF1_h_m1p1_p1100exe2", "pero_EGF1_h_m1p1_p1100exe3", "pero_EGF1_h_m1p1_p1100exe4", "pero_EGF1_h_m1p1_p1100exe5", "pero_EGF1_h_m1p1_p1100exe6", "pero_EGF1_h_m1p1_p1100exe7", "pero_EGF1_h_m1p1_p1100exe8", "pero_EGF1_h_m1p1_p1100exe9", "pero_EGF1_h_m1p1_p120000exe0", "pero_EGF1_h_m1p1_p120000exe1", "pero_EGF1_h_m1p1_p120000exe10", "pero_EGF1_h_m1p1_p120000exe11", "pero_EGF1_h_m1p1_p120000exe12", "pero_EGF1_h_m1p1_p120000exe13", "pero_EGF1_h_m1p1_p120000exe14", "pero_EGF1_h_m1p1_p120000exe15", "pero_EGF1_h_m1p1_p120000exe16", "pero_EGF1_h_m1p1_p120000exe2", "pero_EGF1_h_m1p1_p120000exe3", "pero_EGF1_h_m1p1_p120000exe4", "pero_EGF1_h_m1p1_p120000exe5", "pero_EGF1_h_m1p1_p120000exe6", "pero_EGF1_h_m1p1_p120000exe7", "pero_EGF1_h_m1p1_p120000exe8", "pero_EGF1_h_m1p1_p120000exe9", "pero_EGF1_h_m1p1_p1200exe0", "pero_EGF1_h_m1p1_p1200exe1", "pero_EGF1_h_m1p1_p1200exe10", "pero_EGF1_h_m1p1_p1200exe11", "pero_EGF1_h_m1p1_p1200exe12", "pero_EGF1_h_m1p1_p1200exe13", "pero_EGF1_h_m1p1_p1200exe14", "pero_EGF1_h_m1p1_p1200exe15", "pero_EGF1_h_m1p1_p1200exe16", "pero_EGF1_h_m1p1_p1200exe2", "pero_EGF1_h_m1p1_p1200exe3", "pero_EGF1_h_m1p1_p1200exe4", "pero_EGF1_h_m1p1_p1200exe5", "pero_EGF1_h_m1p1_p1200exe6", "pero_EGF1_h_m1p1_p1200exe7", "pero_EGF1_h_m1p1_p1200exe8", "pero_EGF1_h_m1p1_p1200exe9", "pero_EGF1_h_m1p1_p1300exe0", "pero_EGF1_h_m1p1_p1300exe1", "pero_EGF1_h_m1p1_p1300exe10", "pero_EGF1_h_m1p1_p1300exe11", "pero_EGF1_h_m1p1_p1300exe12", "pero_EGF1_h_m1p1_p1300exe13", "pero_EGF1_h_m1p1_p1300exe14", "pero_EGF1_h_m1p1_p1300exe15", "pero_EGF1_h_m1p1_p1300exe16", "pero_EGF1_h_m1p1_p1300exe2", "pero_EGF1_h_m1p1_p1300exe3", "pero_EGF1_h_m1p1_p1300exe4", "pero_EGF1_h_m1p1_p1300exe5", "pero_EGF1_h_m1p1_p1300exe6", "pero_EGF1_h_m1p1_p1300exe7", "pero_EGF1_h_m1p1_p1300exe8", "pero_EGF1_h_m1p1_p1300exe9", "pero_EGF1_h_m1p1_p140000exe0", "pero_EGF1_h_m1p1_p140000exe1", "pero_EGF1_h_m1p1_p140000exe10", "pero_EGF1_h_m1p1_p140000exe11", "pero_EGF1_h_m1p1_p140000exe12", "pero_EGF1_h_m1p1_p140000exe13", "pero_EGF1_h_m1p1_p140000exe14", "pero_EGF1_h_m1p1_p140000exe15", "pero_EGF1_h_m1p1_p140000exe16", "pero_EGF1_h_m1p1_p140000exe2", "pero_EGF1_h_m1p1_p140000exe3", "pero_EGF1_h_m1p1_p140000exe4", "pero_EGF1_h_m1p1_p140000exe5", "pero_EGF1_h_m1p1_p140000exe6", "pero_EGF1_h_m1p1_p140000exe7", "pero_EGF1_h_m1p1_p140000exe8", "pero_EGF1_h_m1p1_p140000exe9", "pero_EGF1_h_m1p1_p1400exe0", "pero_EGF1_h_m1p1_p1400exe1", "pero_EGF1_h_m1p1_p1400exe10", "pero_EGF1_h_m1p1_p1400exe11", "pero_EGF1_h_m1p1_p1400exe12", "pero_EGF1_h_m1p1_p1400exe13", "pero_EGF1_h_m1p1_p1400exe14", "pero_EGF1_h_m1p1_p1400exe15", "pero_EGF1_h_m1p1_p1400exe16", "pero_EGF1_h_m1p1_p1400exe2", "pero_EGF1_h_m1p1_p1400exe3", "pero_EGF1_h_m1p1_p1400exe4", "pero_EGF1_h_m1p1_p1400exe5", "pero_EGF1_h_m1p1_p1400exe6", "pero_EGF1_h_m1p1_p1400exe7", "pero_EGF1_h_m1p1_p1400exe8", "pero_EGF1_h_m1p1_p1400exe9", "pero_EGF1_h_m1p1_p1500exe0", "pero_EGF1_h_m1p1_p1500exe1", "pero_EGF1_h_m1p1_p1500exe10", "pero_EGF1_h_m1p1_p1500exe11", "pero_EGF1_h_m1p1_p1500exe12", "pero_EGF1_h_m1p1_p1500exe13", "pero_EGF1_h_m1p1_p1500exe14", "pero_EGF1_h_m1p1_p1500exe15", "pero_EGF1_h_m1p1_p1500exe16", "pero_EGF1_h_m1p1_p1500exe2", "pero_EGF1_h_m1p1_p1500exe3", "pero_EGF1_h_m1p1_p1500exe4", "pero_EGF1_h_m1p1_p1500exe5", "pero_EGF1_h_m1p1_p1500exe6", "pero_EGF1_h_m1p1_p1500exe7", "pero_EGF1_h_m1p1_p1500exe8", "pero_EGF1_h_m1p1_p1500exe9", "pero_EGF1_h_m1p1_p160000exe0", "pero_EGF1_h_m1p1_p160000exe1", "pero_EGF1_h_m1p1_p160000exe10", "pero_EGF1_h_m1p1_p160000exe11", "pero_EGF1_h_m1p1_p160000exe12", "pero_EGF1_h_m1p1_p160000exe13", "pero_EGF1_h_m1p1_p160000exe14", "pero_EGF1_h_m1p1_p160000exe15", "pero_EGF1_h_m1p1_p160000exe16", "pero_EGF1_h_m1p1_p160000exe2", "pero_EGF1_h_m1p1_p160000exe3", "pero_EGF1_h_m1p1_p160000exe4", "pero_EGF1_h_m1p1_p160000exe5", "pero_EGF1_h_m1p1_p160000exe6", "pero_EGF1_h_m1p1_p160000exe7", "pero_EGF1_h_m1p1_p160000exe8", "pero_EGF1_h_m1p1_p160000exe9", "pero_EGF1_h_m1p1_p1600exe0", "pero_EGF1_h_m1p1_p1600exe1", "pero_EGF1_h_m1p1_p1600exe10", "pero_EGF1_h_m1p1_p1600exe11", "pero_EGF1_h_m1p1_p1600exe12", "pero_EGF1_h_m1p1_p1600exe13", "pero_EGF1_h_m1p1_p1600exe14", "pero_EGF1_h_m1p1_p1600exe15", "pero_EGF1_h_m1p1_p1600exe16", "pero_EGF1_h_m1p1_p1600exe2", "pero_EGF1_h_m1p1_p1600exe3", "pero_EGF1_h_m1p1_p1600exe4", "pero_EGF1_h_m1p1_p1600exe5", "pero_EGF1_h_m1p1_p1600exe6", "pero_EGF1_h_m1p1_p1600exe7", "pero_EGF1_h_m1p1_p1600exe8", "pero_EGF1_h_m1p1_p1600exe9", "pero_EGF1_h_m1p1_p1700exe0", "pero_EGF1_h_m1p1_p1700exe1", "pero_EGF1_h_m1p1_p1700exe10", "pero_EGF1_h_m1p1_p1700exe11", "pero_EGF1_h_m1p1_p1700exe12", "pero_EGF1_h_m1p1_p1700exe13", "pero_EGF1_h_m1p1_p1700exe14", "pero_EGF1_h_m1p1_p1700exe15", "pero_EGF1_h_m1p1_p1700exe16", "pero_EGF1_h_m1p1_p1700exe2", "pero_EGF1_h_m1p1_p1700exe3", "pero_EGF1_h_m1p1_p1700exe4", "pero_EGF1_h_m1p1_p1700exe5", "pero_EGF1_h_m1p1_p1700exe6", "pero_EGF1_h_m1p1_p1700exe7", "pero_EGF1_h_m1p1_p1700exe8", "pero_EGF1_h_m1p1_p1700exe9", "pero_EGF1_h_m1p1_p180000exe0", "pero_EGF1_h_m1p1_p180000exe1", "pero_EGF1_h_m1p1_p180000exe10", "pero_EGF1_h_m1p1_p180000exe11", "pero_EGF1_h_m1p1_p180000exe12", "pero_EGF1_h_m1p1_p180000exe13", "pero_EGF1_h_m1p1_p180000exe14", "pero_EGF1_h_m1p1_p180000exe15", "pero_EGF1_h_m1p1_p180000exe16", "pero_EGF1_h_m1p1_p180000exe2", "pero_EGF1_h_m1p1_p180000exe3", "pero_EGF1_h_m1p1_p180000exe4", "pero_EGF1_h_m1p1_p180000exe5", "pero_EGF1_h_m1p1_p180000exe6", "pero_EGF1_h_m1p1_p180000exe7", "pero_EGF1_h_m1p1_p180000exe8", "pero_EGF1_h_m1p1_p180000exe9", "pero_EGF1_h_m1p1_p1800exe0", "pero_EGF1_h_m1p1_p1800exe1", "pero_EGF1_h_m1p1_p1800exe10", "pero_EGF1_h_m1p1_p1800exe11", "pero_EGF1_h_m1p1_p1800exe12", "pero_EGF1_h_m1p1_p1800exe13", "pero_EGF1_h_m1p1_p1800exe14", "pero_EGF1_h_m1p1_p1800exe15", "pero_EGF1_h_m1p1_p1800exe16", "pero_EGF1_h_m1p1_p1800exe2", "pero_EGF1_h_m1p1_p1800exe3", "pero_EGF1_h_m1p1_p1800exe4", "pero_EGF1_h_m1p1_p1800exe5", "pero_EGF1_h_m1p1_p1800exe6", "pero_EGF1_h_m1p1_p1800exe7", "pero_EGF1_h_m1p1_p1800exe8", "pero_EGF1_h_m1p1_p1800exe9", "pero_EGF1_h_m1p1_p1900exe0", "pero_EGF1_h_m1p1_p1900exe1", "pero_EGF1_h_m1p1_p1900exe10", "pero_EGF1_h_m1p1_p1900exe11", "pero_EGF1_h_m1p1_p1900exe12", "pero_EGF1_h_m1p1_p1900exe13", "pero_EGF1_h_m1p1_p1900exe14", "pero_EGF1_h_m1p1_p1900exe15", "pero_EGF1_h_m1p1_p1900exe16", "pero_EGF1_h_m1p1_p1900exe17", "pero_EGF1_h_m1p1_p1900exe2", "pero_EGF1_h_m1p1_p1900exe3", "pero_EGF1_h_m1p1_p1900exe4", "pero_EGF1_h_m1p1_p1900exe5", "pero_EGF1_h_m1p1_p1900exe6", "pero_EGF1_h_m1p1_p1900exe7", "pero_EGF1_h_m1p1_p1900exe8", "pero_EGF1_h_m1p1_p1900exe9", "pero_EGF1_h_m1p1_p200000exe0", "pero_EGF1_h_m1p1_p200000exe1", "pero_EGF1_h_m1p1_p200000exe10", "pero_EGF1_h_m1p1_p200000exe11", "pero_EGF1_h_m1p1_p200000exe12", "pero_EGF1_h_m1p1_p200000exe13", "pero_EGF1_h_m1p1_p200000exe14", "pero_EGF1_h_m1p1_p200000exe15", "pero_EGF1_h_m1p1_p200000exe16", "pero_EGF1_h_m1p1_p200000exe2", "pero_EGF1_h_m1p1_p200000exe3", "pero_EGF1_h_m1p1_p200000exe4", "pero_EGF1_h_m1p1_p200000exe5", "pero_EGF1_h_m1p1_p200000exe6", "pero_EGF1_h_m1p1_p200000exe7", "pero_EGF1_h_m1p1_p200000exe8", "pero_EGF1_h_m1p1_p200000exe9", "pero_EGF1_h_m1p1_p20000exe0", "pero_EGF1_h_m1p1_p20000exe1", "pero_EGF1_h_m1p1_p20000exe10", "pero_EGF1_h_m1p1_p20000exe11", "pero_EGF1_h_m1p1_p20000exe12", "pero_EGF1_h_m1p1_p20000exe13", "pero_EGF1_h_m1p1_p20000exe14", "pero_EGF1_h_m1p1_p20000exe15", "pero_EGF1_h_m1p1_p20000exe16", "pero_EGF1_h_m1p1_p20000exe2", "pero_EGF1_h_m1p1_p20000exe3", "pero_EGF1_h_m1p1_p20000exe4", "pero_EGF1_h_m1p1_p20000exe5", "pero_EGF1_h_m1p1_p20000exe6", "pero_EGF1_h_m1p1_p20000exe7", "pero_EGF1_h_m1p1_p20000exe8", "pero_EGF1_h_m1p1_p20000exe9", "pero_EGF1_h_m1p1_p2000exe0", "pero_EGF1_h_m1p1_p2000exe1", "pero_EGF1_h_m1p1_p2000exe10", "pero_EGF1_h_m1p1_p2000exe11", "pero_EGF1_h_m1p1_p2000exe12", "pero_EGF1_h_m1p1_p2000exe13", "pero_EGF1_h_m1p1_p2000exe14", "pero_EGF1_h_m1p1_p2000exe15", "pero_EGF1_h_m1p1_p2000exe16", "pero_EGF1_h_m1p1_p2000exe2", "pero_EGF1_h_m1p1_p2000exe3", "pero_EGF1_h_m1p1_p2000exe4", "pero_EGF1_h_m1p1_p2000exe5", "pero_EGF1_h_m1p1_p2000exe6", "pero_EGF1_h_m1p1_p2000exe7", "pero_EGF1_h_m1p1_p2000exe8", "pero_EGF1_h_m1p1_p2000exe9", "pero_EGF1_h_m1p1_p200exe0", "pero_EGF1_h_m1p1_p200exe1", "pero_EGF1_h_m1p1_p200exe10", "pero_EGF1_h_m1p1_p200exe11", "pero_EGF1_h_m1p1_p200exe12", "pero_EGF1_h_m1p1_p200exe13", "pero_EGF1_h_m1p1_p200exe14", "pero_EGF1_h_m1p1_p200exe15", "pero_EGF1_h_m1p1_p200exe16", "pero_EGF1_h_m1p1_p200exe2", "pero_EGF1_h_m1p1_p200exe3", "pero_EGF1_h_m1p1_p200exe4", "pero_EGF1_h_m1p1_p200exe5", "pero_EGF1_h_m1p1_p200exe6", "pero_EGF1_h_m1p1_p200exe7", "pero_EGF1_h_m1p1_p200exe8", "pero_EGF1_h_m1p1_p200exe9", "pero_EGF1_h_m1p1_p2100exe0", "pero_EGF1_h_m1p1_p2100exe1", "pero_EGF1_h_m1p1_p2100exe10", "pero_EGF1_h_m1p1_p2100exe11", "pero_EGF1_h_m1p1_p2100exe12", "pero_EGF1_h_m1p1_p2100exe13", "pero_EGF1_h_m1p1_p2100exe14", "pero_EGF1_h_m1p1_p2100exe15", "pero_EGF1_h_m1p1_p2100exe16", "pero_EGF1_h_m1p1_p2100exe2", "pero_EGF1_h_m1p1_p2100exe3", "pero_EGF1_h_m1p1_p2100exe4", "pero_EGF1_h_m1p1_p2100exe5", "pero_EGF1_h_m1p1_p2100exe6", "pero_EGF1_h_m1p1_p2100exe7", "pero_EGF1_h_m1p1_p2100exe8", "pero_EGF1_h_m1p1_p2100exe9", "pero_EGF1_h_m1p1_p220000exe0", "pero_EGF1_h_m1p1_p220000exe1", "pero_EGF1_h_m1p1_p220000exe10", "pero_EGF1_h_m1p1_p220000exe11", "pero_EGF1_h_m1p1_p220000exe12", "pero_EGF1_h_m1p1_p220000exe13", "pero_EGF1_h_m1p1_p220000exe14", "pero_EGF1_h_m1p1_p220000exe15", "pero_EGF1_h_m1p1_p220000exe16", "pero_EGF1_h_m1p1_p220000exe2", "pero_EGF1_h_m1p1_p220000exe3", "pero_EGF1_h_m1p1_p220000exe4", "pero_EGF1_h_m1p1_p220000exe5", "pero_EGF1_h_m1p1_p220000exe6", "pero_EGF1_h_m1p1_p220000exe7", "pero_EGF1_h_m1p1_p220000exe8", "pero_EGF1_h_m1p1_p220000exe9", "pero_EGF1_h_m1p1_p2200exe0", "pero_EGF1_h_m1p1_p2200exe1", "pero_EGF1_h_m1p1_p2200exe10", "pero_EGF1_h_m1p1_p2200exe11", "pero_EGF1_h_m1p1_p2200exe12", "pero_EGF1_h_m1p1_p2200exe13", "pero_EGF1_h_m1p1_p2200exe14", "pero_EGF1_h_m1p1_p2200exe15", "pero_EGF1_h_m1p1_p2200exe16", "pero_EGF1_h_m1p1_p2200exe2", "pero_EGF1_h_m1p1_p2200exe3", "pero_EGF1_h_m1p1_p2200exe4", "pero_EGF1_h_m1p1_p2200exe5", "pero_EGF1_h_m1p1_p2200exe6", "pero_EGF1_h_m1p1_p2200exe7", "pero_EGF1_h_m1p1_p2200exe8", "pero_EGF1_h_m1p1_p2200exe9", "pero_EGF1_h_m1p1_p2300exe0", "pero_EGF1_h_m1p1_p2300exe1", "pero_EGF1_h_m1p1_p2300exe10", "pero_EGF1_h_m1p1_p2300exe11", "pero_EGF1_h_m1p1_p2300exe12", "pero_EGF1_h_m1p1_p2300exe13", "pero_EGF1_h_m1p1_p2300exe14", "pero_EGF1_h_m1p1_p2300exe15", "pero_EGF1_h_m1p1_p2300exe16", "pero_EGF1_h_m1p1_p2300exe17", "pero_EGF1_h_m1p1_p2300exe2", "pero_EGF1_h_m1p1_p2300exe3", "pero_EGF1_h_m1p1_p2300exe4", "pero_EGF1_h_m1p1_p2300exe5", "pero_EGF1_h_m1p1_p2300exe6", "pero_EGF1_h_m1p1_p2300exe7", "pero_EGF1_h_m1p1_p2300exe8", "pero_EGF1_h_m1p1_p2300exe9", "pero_EGF1_h_m1p1_p240000exe0", "pero_EGF1_h_m1p1_p240000exe1", "pero_EGF1_h_m1p1_p240000exe10", "pero_EGF1_h_m1p1_p240000exe11", "pero_EGF1_h_m1p1_p240000exe12", "pero_EGF1_h_m1p1_p240000exe13", "pero_EGF1_h_m1p1_p240000exe14", "pero_EGF1_h_m1p1_p240000exe15", "pero_EGF1_h_m1p1_p240000exe16", "pero_EGF1_h_m1p1_p240000exe2", "pero_EGF1_h_m1p1_p240000exe3", "pero_EGF1_h_m1p1_p240000exe4", "pero_EGF1_h_m1p1_p240000exe5", "pero_EGF1_h_m1p1_p240000exe6", "pero_EGF1_h_m1p1_p240000exe7", "pero_EGF1_h_m1p1_p240000exe8", "pero_EGF1_h_m1p1_p240000exe9", "pero_EGF1_h_m1p1_p2400exe0", "pero_EGF1_h_m1p1_p2400exe1", "pero_EGF1_h_m1p1_p2400exe10", "pero_EGF1_h_m1p1_p2400exe11", "pero_EGF1_h_m1p1_p2400exe12", "pero_EGF1_h_m1p1_p2400exe13", "pero_EGF1_h_m1p1_p2400exe14", "pero_EGF1_h_m1p1_p2400exe15", "pero_EGF1_h_m1p1_p2400exe16", "pero_EGF1_h_m1p1_p2400exe2", "pero_EGF1_h_m1p1_p2400exe3", "pero_EGF1_h_m1p1_p2400exe4", "pero_EGF1_h_m1p1_p2400exe5", "pero_EGF1_h_m1p1_p2400exe6", "pero_EGF1_h_m1p1_p2400exe7", "pero_EGF1_h_m1p1_p2400exe8", "pero_EGF1_h_m1p1_p2400exe9", "pero_EGF1_h_m1p1_p2500exe0", "pero_EGF1_h_m1p1_p2500exe1", "pero_EGF1_h_m1p1_p2500exe10", "pero_EGF1_h_m1p1_p2500exe11", "pero_EGF1_h_m1p1_p2500exe12", "pero_EGF1_h_m1p1_p2500exe13", "pero_EGF1_h_m1p1_p2500exe14", "pero_EGF1_h_m1p1_p2500exe15", "pero_EGF1_h_m1p1_p2500exe16", "pero_EGF1_h_m1p1_p2500exe2", "pero_EGF1_h_m1p1_p2500exe3", "pero_EGF1_h_m1p1_p2500exe4", "pero_EGF1_h_m1p1_p2500exe5", "pero_EGF1_h_m1p1_p2500exe6", "pero_EGF1_h_m1p1_p2500exe7", "pero_EGF1_h_m1p1_p2500exe8", "pero_EGF1_h_m1p1_p2500exe9", "pero_EGF1_h_m1p1_p260000exe0", "pero_EGF1_h_m1p1_p260000exe1", "pero_EGF1_h_m1p1_p260000exe10", "pero_EGF1_h_m1p1_p260000exe11", "pero_EGF1_h_m1p1_p260000exe12", "pero_EGF1_h_m1p1_p260000exe13", "pero_EGF1_h_m1p1_p260000exe14", "pero_EGF1_h_m1p1_p260000exe15", "pero_EGF1_h_m1p1_p260000exe16", "pero_EGF1_h_m1p1_p260000exe2", "pero_EGF1_h_m1p1_p260000exe3", "pero_EGF1_h_m1p1_p260000exe4", "pero_EGF1_h_m1p1_p260000exe5", "pero_EGF1_h_m1p1_p260000exe6", "pero_EGF1_h_m1p1_p260000exe7", "pero_EGF1_h_m1p1_p260000exe8", "pero_EGF1_h_m1p1_p260000exe9", "pero_EGF1_h_m1p1_p2600exe0", "pero_EGF1_h_m1p1_p2600exe1", "pero_EGF1_h_m1p1_p2600exe10", "pero_EGF1_h_m1p1_p2600exe11", "pero_EGF1_h_m1p1_p2600exe12", "pero_EGF1_h_m1p1_p2600exe13", "pero_EGF1_h_m1p1_p2600exe14", "pero_EGF1_h_m1p1_p2600exe15", "pero_EGF1_h_m1p1_p2600exe16", "pero_EGF1_h_m1p1_p2600exe2", "pero_EGF1_h_m1p1_p2600exe3", "pero_EGF1_h_m1p1_p2600exe4", "pero_EGF1_h_m1p1_p2600exe5", "pero_EGF1_h_m1p1_p2600exe6", "pero_EGF1_h_m1p1_p2600exe7", "pero_EGF1_h_m1p1_p2600exe8", "pero_EGF1_h_m1p1_p2600exe9", "pero_EGF1_h_m1p1_p2700exe0", "pero_EGF1_h_m1p1_p2700exe1", "pero_EGF1_h_m1p1_p2700exe10", "pero_EGF1_h_m1p1_p2700exe11", "pero_EGF1_h_m1p1_p2700exe12", "pero_EGF1_h_m1p1_p2700exe13", "pero_EGF1_h_m1p1_p2700exe14", "pero_EGF1_h_m1p1_p2700exe15", "pero_EGF1_h_m1p1_p2700exe16", "pero_EGF1_h_m1p1_p2700exe2", "pero_EGF1_h_m1p1_p2700exe3", "pero_EGF1_h_m1p1_p2700exe4", "pero_EGF1_h_m1p1_p2700exe5", "pero_EGF1_h_m1p1_p2700exe6", "pero_EGF1_h_m1p1_p2700exe7", "pero_EGF1_h_m1p1_p2700exe8", "pero_EGF1_h_m1p1_p2700exe9", "pero_EGF1_h_m1p1_p280000exe0", "pero_EGF1_h_m1p1_p280000exe1", "pero_EGF1_h_m1p1_p280000exe10", "pero_EGF1_h_m1p1_p280000exe11", "pero_EGF1_h_m1p1_p280000exe12", "pero_EGF1_h_m1p1_p280000exe13", "pero_EGF1_h_m1p1_p280000exe14", "pero_EGF1_h_m1p1_p280000exe15", "pero_EGF1_h_m1p1_p280000exe16", "pero_EGF1_h_m1p1_p280000exe2", "pero_EGF1_h_m1p1_p280000exe3", "pero_EGF1_h_m1p1_p280000exe4", "pero_EGF1_h_m1p1_p280000exe5", "pero_EGF1_h_m1p1_p280000exe6", "pero_EGF1_h_m1p1_p280000exe7", "pero_EGF1_h_m1p1_p280000exe8", "pero_EGF1_h_m1p1_p280000exe9", "pero_EGF1_h_m1p1_p2800exe0", "pero_EGF1_h_m1p1_p2800exe1", "pero_EGF1_h_m1p1_p2800exe10", "pero_EGF1_h_m1p1_p2800exe11", "pero_EGF1_h_m1p1_p2800exe12", "pero_EGF1_h_m1p1_p2800exe13", "pero_EGF1_h_m1p1_p2800exe14", "pero_EGF1_h_m1p1_p2800exe15", "pero_EGF1_h_m1p1_p2800exe16", "pero_EGF1_h_m1p1_p2800exe2", "pero_EGF1_h_m1p1_p2800exe3", "pero_EGF1_h_m1p1_p2800exe4", "pero_EGF1_h_m1p1_p2800exe5", "pero_EGF1_h_m1p1_p2800exe6", "pero_EGF1_h_m1p1_p2800exe7", "pero_EGF1_h_m1p1_p2800exe8", "pero_EGF1_h_m1p1_p2800exe9", "pero_EGF1_h_m1p1_p2900exe0", "pero_EGF1_h_m1p1_p2900exe1", "pero_EGF1_h_m1p1_p2900exe10", "pero_EGF1_h_m1p1_p2900exe11", "pero_EGF1_h_m1p1_p2900exe12", "pero_EGF1_h_m1p1_p2900exe13", "pero_EGF1_h_m1p1_p2900exe14", "pero_EGF1_h_m1p1_p2900exe15", "pero_EGF1_h_m1p1_p2900exe16", "pero_EGF1_h_m1p1_p2900exe2", "pero_EGF1_h_m1p1_p2900exe3", "pero_EGF1_h_m1p1_p2900exe4", "pero_EGF1_h_m1p1_p2900exe5", "pero_EGF1_h_m1p1_p2900exe6", "pero_EGF1_h_m1p1_p2900exe7", "pero_EGF1_h_m1p1_p2900exe8", "pero_EGF1_h_m1p1_p2900exe9", "pero_EGF1_h_m1p1_p300000exe0", "pero_EGF1_h_m1p1_p300000exe1", "pero_EGF1_h_m1p1_p300000exe10", "pero_EGF1_h_m1p1_p300000exe11", "pero_EGF1_h_m1p1_p300000exe12", "pero_EGF1_h_m1p1_p300000exe13", "pero_EGF1_h_m1p1_p300000exe14", "pero_EGF1_h_m1p1_p300000exe15", "pero_EGF1_h_m1p1_p300000exe16", "pero_EGF1_h_m1p1_p300000exe2", "pero_EGF1_h_m1p1_p300000exe3", "pero_EGF1_h_m1p1_p300000exe4", "pero_EGF1_h_m1p1_p300000exe5", "pero_EGF1_h_m1p1_p300000exe6", "pero_EGF1_h_m1p1_p300000exe7", "pero_EGF1_h_m1p1_p300000exe8", "pero_EGF1_h_m1p1_p300000exe9", "pero_EGF1_h_m1p1_p30000exe0", "pero_EGF1_h_m1p1_p30000exe1", "pero_EGF1_h_m1p1_p30000exe10", "pero_EGF1_h_m1p1_p30000exe11", "pero_EGF1_h_m1p1_p30000exe12", "pero_EGF1_h_m1p1_p30000exe13", "pero_EGF1_h_m1p1_p30000exe14", "pero_EGF1_h_m1p1_p30000exe15", "pero_EGF1_h_m1p1_p30000exe16", "pero_EGF1_h_m1p1_p30000exe2", "pero_EGF1_h_m1p1_p30000exe3", "pero_EGF1_h_m1p1_p30000exe4", "pero_EGF1_h_m1p1_p30000exe5", "pero_EGF1_h_m1p1_p30000exe6", "pero_EGF1_h_m1p1_p30000exe7", "pero_EGF1_h_m1p1_p30000exe8", "pero_EGF1_h_m1p1_p30000exe9", "pero_EGF1_h_m1p1_p3000exe0", "pero_EGF1_h_m1p1_p3000exe1", "pero_EGF1_h_m1p1_p3000exe10", "pero_EGF1_h_m1p1_p3000exe11", "pero_EGF1_h_m1p1_p3000exe12", "pero_EGF1_h_m1p1_p3000exe13", "pero_EGF1_h_m1p1_p3000exe14", "pero_EGF1_h_m1p1_p3000exe15", "pero_EGF1_h_m1p1_p3000exe16", "pero_EGF1_h_m1p1_p3000exe17", "pero_EGF1_h_m1p1_p3000exe2", "pero_EGF1_h_m1p1_p3000exe3", "pero_EGF1_h_m1p1_p3000exe4", "pero_EGF1_h_m1p1_p3000exe5", "pero_EGF1_h_m1p1_p3000exe6", "pero_EGF1_h_m1p1_p3000exe7", "pero_EGF1_h_m1p1_p3000exe8", "pero_EGF1_h_m1p1_p3000exe9", "pero_EGF1_h_m1p1_p300exe0", "pero_EGF1_h_m1p1_p300exe1", "pero_EGF1_h_m1p1_p300exe10", "pero_EGF1_h_m1p1_p300exe11", "pero_EGF1_h_m1p1_p300exe12", "pero_EGF1_h_m1p1_p300exe13", "pero_EGF1_h_m1p1_p300exe14", "pero_EGF1_h_m1p1_p300exe15", "pero_EGF1_h_m1p1_p300exe16", "pero_EGF1_h_m1p1_p300exe2", "pero_EGF1_h_m1p1_p300exe3", "pero_EGF1_h_m1p1_p300exe4", "pero_EGF1_h_m1p1_p300exe5", "pero_EGF1_h_m1p1_p300exe6", "pero_EGF1_h_m1p1_p300exe7", "pero_EGF1_h_m1p1_p300exe8", "pero_EGF1_h_m1p1_p300exe9", "pero_EGF1_h_m1p1_p320000exe0", "pero_EGF1_h_m1p1_p320000exe1", "pero_EGF1_h_m1p1_p320000exe10", "pero_EGF1_h_m1p1_p320000exe11", "pero_EGF1_h_m1p1_p320000exe12", "pero_EGF1_h_m1p1_p320000exe13", "pero_EGF1_h_m1p1_p320000exe14", "pero_EGF1_h_m1p1_p320000exe15", "pero_EGF1_h_m1p1_p320000exe16", "pero_EGF1_h_m1p1_p320000exe2", "pero_EGF1_h_m1p1_p320000exe3", "pero_EGF1_h_m1p1_p320000exe4", "pero_EGF1_h_m1p1_p320000exe5", "pero_EGF1_h_m1p1_p320000exe6", "pero_EGF1_h_m1p1_p320000exe7", "pero_EGF1_h_m1p1_p320000exe8", "pero_EGF1_h_m1p1_p320000exe9", "pero_EGF1_h_m1p1_p340000exe0", "pero_EGF1_h_m1p1_p340000exe1", "pero_EGF1_h_m1p1_p340000exe10", "pero_EGF1_h_m1p1_p340000exe11", "pero_EGF1_h_m1p1_p340000exe12", "pero_EGF1_h_m1p1_p340000exe13", "pero_EGF1_h_m1p1_p340000exe14", "pero_EGF1_h_m1p1_p340000exe15", "pero_EGF1_h_m1p1_p340000exe16", "pero_EGF1_h_m1p1_p340000exe2", "pero_EGF1_h_m1p1_p340000exe3", "pero_EGF1_h_m1p1_p340000exe4", "pero_EGF1_h_m1p1_p340000exe5", "pero_EGF1_h_m1p1_p340000exe6", "pero_EGF1_h_m1p1_p340000exe7", "pero_EGF1_h_m1p1_p340000exe8", "pero_EGF1_h_m1p1_p340000exe9", "pero_EGF1_h_m1p1_p360000exe0", "pero_EGF1_h_m1p1_p360000exe1", "pero_EGF1_h_m1p1_p360000exe10", "pero_EGF1_h_m1p1_p360000exe11", "pero_EGF1_h_m1p1_p360000exe12", "pero_EGF1_h_m1p1_p360000exe13", "pero_EGF1_h_m1p1_p360000exe14", "pero_EGF1_h_m1p1_p360000exe15", "pero_EGF1_h_m1p1_p360000exe16", "pero_EGF1_h_m1p1_p360000exe2", "pero_EGF1_h_m1p1_p360000exe3", "pero_EGF1_h_m1p1_p360000exe4", "pero_EGF1_h_m1p1_p360000exe5", "pero_EGF1_h_m1p1_p360000exe6", "pero_EGF1_h_m1p1_p360000exe7", "pero_EGF1_h_m1p1_p360000exe8", "pero_EGF1_h_m1p1_p360000exe9", "pero_EGF1_h_m1p1_p380000exe0", "pero_EGF1_h_m1p1_p380000exe1", "pero_EGF1_h_m1p1_p380000exe10", "pero_EGF1_h_m1p1_p380000exe11", "pero_EGF1_h_m1p1_p380000exe12", "pero_EGF1_h_m1p1_p380000exe13", "pero_EGF1_h_m1p1_p380000exe14", "pero_EGF1_h_m1p1_p380000exe15", "pero_EGF1_h_m1p1_p380000exe16", "pero_EGF1_h_m1p1_p380000exe2", "pero_EGF1_h_m1p1_p380000exe3", "pero_EGF1_h_m1p1_p380000exe4", "pero_EGF1_h_m1p1_p380000exe5", "pero_EGF1_h_m1p1_p380000exe6", "pero_EGF1_h_m1p1_p380000exe7", "pero_EGF1_h_m1p1_p380000exe8", "pero_EGF1_h_m1p1_p380000exe9", "pero_EGF1_h_m1p1_p400000exe0", "pero_EGF1_h_m1p1_p400000exe1", "pero_EGF1_h_m1p1_p400000exe10", "pero_EGF1_h_m1p1_p400000exe11", "pero_EGF1_h_m1p1_p400000exe12", "pero_EGF1_h_m1p1_p400000exe13", "pero_EGF1_h_m1p1_p400000exe14", "pero_EGF1_h_m1p1_p400000exe15", "pero_EGF1_h_m1p1_p400000exe16", "pero_EGF1_h_m1p1_p400000exe2", "pero_EGF1_h_m1p1_p400000exe3", "pero_EGF1_h_m1p1_p400000exe4", "pero_EGF1_h_m1p1_p400000exe5", "pero_EGF1_h_m1p1_p400000exe6", "pero_EGF1_h_m1p1_p400000exe7", "pero_EGF1_h_m1p1_p400000exe8", "pero_EGF1_h_m1p1_p400000exe9", "pero_EGF1_h_m1p1_p40000exe0", "pero_EGF1_h_m1p1_p40000exe1", "pero_EGF1_h_m1p1_p40000exe10", "pero_EGF1_h_m1p1_p40000exe11", "pero_EGF1_h_m1p1_p40000exe12", "pero_EGF1_h_m1p1_p40000exe13", "pero_EGF1_h_m1p1_p40000exe14", "pero_EGF1_h_m1p1_p40000exe15", "pero_EGF1_h_m1p1_p40000exe16", "pero_EGF1_h_m1p1_p40000exe2", "pero_EGF1_h_m1p1_p40000exe3", "pero_EGF1_h_m1p1_p40000exe4", "pero_EGF1_h_m1p1_p40000exe5", "pero_EGF1_h_m1p1_p40000exe6", "pero_EGF1_h_m1p1_p40000exe7", "pero_EGF1_h_m1p1_p40000exe8", "pero_EGF1_h_m1p1_p40000exe9", "pero_EGF1_h_m1p1_p4000exe0", "pero_EGF1_h_m1p1_p4000exe1", "pero_EGF1_h_m1p1_p4000exe10", "pero_EGF1_h_m1p1_p4000exe11", "pero_EGF1_h_m1p1_p4000exe12", "pero_EGF1_h_m1p1_p4000exe13", "pero_EGF1_h_m1p1_p4000exe14", "pero_EGF1_h_m1p1_p4000exe15", "pero_EGF1_h_m1p1_p4000exe16", "pero_EGF1_h_m1p1_p4000exe2", "pero_EGF1_h_m1p1_p4000exe3", "pero_EGF1_h_m1p1_p4000exe4", "pero_EGF1_h_m1p1_p4000exe5", "pero_EGF1_h_m1p1_p4000exe6", "pero_EGF1_h_m1p1_p4000exe7", "pero_EGF1_h_m1p1_p4000exe8", "pero_EGF1_h_m1p1_p4000exe9", "pero_EGF1_h_m1p1_p400exe0", "pero_EGF1_h_m1p1_p400exe1", "pero_EGF1_h_m1p1_p400exe10", "pero_EGF1_h_m1p1_p400exe11", "pero_EGF1_h_m1p1_p400exe12", "pero_EGF1_h_m1p1_p400exe13", "pero_EGF1_h_m1p1_p400exe14", "pero_EGF1_h_m1p1_p400exe15", "pero_EGF1_h_m1p1_p400exe16", "pero_EGF1_h_m1p1_p400exe2", "pero_EGF1_h_m1p1_p400exe3", "pero_EGF1_h_m1p1_p400exe4", "pero_EGF1_h_m1p1_p400exe5", "pero_EGF1_h_m1p1_p400exe6", "pero_EGF1_h_m1p1_p400exe7", "pero_EGF1_h_m1p1_p400exe8", "pero_EGF1_h_m1p1_p400exe9", "pero_EGF1_h_m1p1_p420000exe0", "pero_EGF1_h_m1p1_p420000exe1", "pero_EGF1_h_m1p1_p420000exe10", "pero_EGF1_h_m1p1_p420000exe11", "pero_EGF1_h_m1p1_p420000exe12", "pero_EGF1_h_m1p1_p420000exe13", "pero_EGF1_h_m1p1_p420000exe14", "pero_EGF1_h_m1p1_p420000exe15", "pero_EGF1_h_m1p1_p420000exe16", "pero_EGF1_h_m1p1_p420000exe2", "pero_EGF1_h_m1p1_p420000exe3", "pero_EGF1_h_m1p1_p420000exe4", "pero_EGF1_h_m1p1_p420000exe5", "pero_EGF1_h_m1p1_p420000exe6", "pero_EGF1_h_m1p1_p420000exe7", "pero_EGF1_h_m1p1_p420000exe8", "pero_EGF1_h_m1p1_p420000exe9", "pero_EGF1_h_m1p1_p440000exe0", "pero_EGF1_h_m1p1_p440000exe1", "pero_EGF1_h_m1p1_p440000exe10", "pero_EGF1_h_m1p1_p440000exe11", "pero_EGF1_h_m1p1_p440000exe12", "pero_EGF1_h_m1p1_p440000exe13", "pero_EGF1_h_m1p1_p440000exe14", "pero_EGF1_h_m1p1_p440000exe15", "pero_EGF1_h_m1p1_p440000exe16", "pero_EGF1_h_m1p1_p440000exe2", "pero_EGF1_h_m1p1_p440000exe3", "pero_EGF1_h_m1p1_p440000exe4", "pero_EGF1_h_m1p1_p440000exe5", "pero_EGF1_h_m1p1_p440000exe6", "pero_EGF1_h_m1p1_p440000exe7", "pero_EGF1_h_m1p1_p440000exe8", "pero_EGF1_h_m1p1_p440000exe9", "pero_EGF1_h_m1p1_p480000exe0", "pero_EGF1_h_m1p1_p480000exe1", "pero_EGF1_h_m1p1_p480000exe10", "pero_EGF1_h_m1p1_p480000exe11", "pero_EGF1_h_m1p1_p480000exe12", "pero_EGF1_h_m1p1_p480000exe13", "pero_EGF1_h_m1p1_p480000exe14", "pero_EGF1_h_m1p1_p480000exe15", "pero_EGF1_h_m1p1_p480000exe16", "pero_EGF1_h_m1p1_p480000exe2", "pero_EGF1_h_m1p1_p480000exe3", "pero_EGF1_h_m1p1_p480000exe4", "pero_EGF1_h_m1p1_p480000exe5", "pero_EGF1_h_m1p1_p480000exe6", "pero_EGF1_h_m1p1_p480000exe7", "pero_EGF1_h_m1p1_p480000exe8", "pero_EGF1_h_m1p1_p480000exe9", "pero_EGF1_h_m1p1_p500000exe0", "pero_EGF1_h_m1p1_p500000exe1", "pero_EGF1_h_m1p1_p500000exe10", "pero_EGF1_h_m1p1_p500000exe11", "pero_EGF1_h_m1p1_p500000exe12", "pero_EGF1_h_m1p1_p500000exe13", "pero_EGF1_h_m1p1_p500000exe14", "pero_EGF1_h_m1p1_p500000exe15", "pero_EGF1_h_m1p1_p500000exe16", "pero_EGF1_h_m1p1_p500000exe2", "pero_EGF1_h_m1p1_p500000exe3", "pero_EGF1_h_m1p1_p500000exe4", "pero_EGF1_h_m1p1_p500000exe5", "pero_EGF1_h_m1p1_p500000exe6", "pero_EGF1_h_m1p1_p500000exe7", "pero_EGF1_h_m1p1_p500000exe8", "pero_EGF1_h_m1p1_p500000exe9", "pero_EGF1_h_m1p1_p50000exe0", "pero_EGF1_h_m1p1_p50000exe1", "pero_EGF1_h_m1p1_p50000exe10", "pero_EGF1_h_m1p1_p50000exe11", "pero_EGF1_h_m1p1_p50000exe12", "pero_EGF1_h_m1p1_p50000exe13", "pero_EGF1_h_m1p1_p50000exe14", "pero_EGF1_h_m1p1_p50000exe15", "pero_EGF1_h_m1p1_p50000exe16", "pero_EGF1_h_m1p1_p50000exe2", "pero_EGF1_h_m1p1_p50000exe3", "pero_EGF1_h_m1p1_p50000exe4", "pero_EGF1_h_m1p1_p50000exe5", "pero_EGF1_h_m1p1_p50000exe6", "pero_EGF1_h_m1p1_p50000exe7", "pero_EGF1_h_m1p1_p50000exe8", "pero_EGF1_h_m1p1_p50000exe9", "pero_EGF1_h_m1p1_p500exe0", "pero_EGF1_h_m1p1_p500exe1", "pero_EGF1_h_m1p1_p500exe10", "pero_EGF1_h_m1p1_p500exe11", "pero_EGF1_h_m1p1_p500exe12", "pero_EGF1_h_m1p1_p500exe13", "pero_EGF1_h_m1p1_p500exe14", "pero_EGF1_h_m1p1_p500exe15", "pero_EGF1_h_m1p1_p500exe16", "pero_EGF1_h_m1p1_p500exe2", "pero_EGF1_h_m1p1_p500exe3", "pero_EGF1_h_m1p1_p500exe4", "pero_EGF1_h_m1p1_p500exe5", "pero_EGF1_h_m1p1_p500exe6", "pero_EGF1_h_m1p1_p500exe7", "pero_EGF1_h_m1p1_p500exe8", "pero_EGF1_h_m1p1_p500exe9", "pero_EGF1_h_m1p1_p60000exe0", "pero_EGF1_h_m1p1_p60000exe1", "pero_EGF1_h_m1p1_p60000exe10", "pero_EGF1_h_m1p1_p60000exe11", "pero_EGF1_h_m1p1_p60000exe12", "pero_EGF1_h_m1p1_p60000exe13", "pero_EGF1_h_m1p1_p60000exe14", "pero_EGF1_h_m1p1_p60000exe15", "pero_EGF1_h_m1p1_p60000exe16", "pero_EGF1_h_m1p1_p60000exe2", "pero_EGF1_h_m1p1_p60000exe3", "pero_EGF1_h_m1p1_p60000exe4", "pero_EGF1_h_m1p1_p60000exe5", "pero_EGF1_h_m1p1_p60000exe6", "pero_EGF1_h_m1p1_p60000exe7", "pero_EGF1_h_m1p1_p60000exe8", "pero_EGF1_h_m1p1_p60000exe9", "pero_EGF1_h_m1p1_p6000exe0", "pero_EGF1_h_m1p1_p6000exe1", "pero_EGF1_h_m1p1_p6000exe10", "pero_EGF1_h_m1p1_p6000exe11", "pero_EGF1_h_m1p1_p6000exe12", "pero_EGF1_h_m1p1_p6000exe13", "pero_EGF1_h_m1p1_p6000exe14", "pero_EGF1_h_m1p1_p6000exe15", "pero_EGF1_h_m1p1_p6000exe16", "pero_EGF1_h_m1p1_p6000exe2", "pero_EGF1_h_m1p1_p6000exe3", "pero_EGF1_h_m1p1_p6000exe4", "pero_EGF1_h_m1p1_p6000exe5", "pero_EGF1_h_m1p1_p6000exe6", "pero_EGF1_h_m1p1_p6000exe7", "pero_EGF1_h_m1p1_p6000exe8", "pero_EGF1_h_m1p1_p6000exe9", "pero_EGF1_h_m1p1_p600exe0", "pero_EGF1_h_m1p1_p600exe1", "pero_EGF1_h_m1p1_p600exe10", "pero_EGF1_h_m1p1_p600exe11", "pero_EGF1_h_m1p1_p600exe12", "pero_EGF1_h_m1p1_p600exe13", "pero_EGF1_h_m1p1_p600exe14", "pero_EGF1_h_m1p1_p600exe15", "pero_EGF1_h_m1p1_p600exe16", "pero_EGF1_h_m1p1_p600exe17", "pero_EGF1_h_m1p1_p600exe2", "pero_EGF1_h_m1p1_p600exe3", "pero_EGF1_h_m1p1_p600exe4", "pero_EGF1_h_m1p1_p600exe5", "pero_EGF1_h_m1p1_p600exe6", "pero_EGF1_h_m1p1_p600exe7", "pero_EGF1_h_m1p1_p600exe8", "pero_EGF1_h_m1p1_p600exe9", "pero_EGF1_h_m1p1_p700exe0", "pero_EGF1_h_m1p1_p700exe1", "pero_EGF1_h_m1p1_p700exe10", "pero_EGF1_h_m1p1_p700exe11", "pero_EGF1_h_m1p1_p700exe12", "pero_EGF1_h_m1p1_p700exe13", "pero_EGF1_h_m1p1_p700exe14", "pero_EGF1_h_m1p1_p700exe15", "pero_EGF1_h_m1p1_p700exe16", "pero_EGF1_h_m1p1_p700exe2", "pero_EGF1_h_m1p1_p700exe3", "pero_EGF1_h_m1p1_p700exe4", "pero_EGF1_h_m1p1_p700exe5", "pero_EGF1_h_m1p1_p700exe6", "pero_EGF1_h_m1p1_p700exe7", "pero_EGF1_h_m1p1_p700exe8", "pero_EGF1_h_m1p1_p700exe9", "pero_EGF1_h_m1p1_p80000exe0", "pero_EGF1_h_m1p1_p80000exe1", "pero_EGF1_h_m1p1_p80000exe10", "pero_EGF1_h_m1p1_p80000exe11", "pero_EGF1_h_m1p1_p80000exe12", "pero_EGF1_h_m1p1_p80000exe13", "pero_EGF1_h_m1p1_p80000exe14", "pero_EGF1_h_m1p1_p80000exe15", "pero_EGF1_h_m1p1_p80000exe16", "pero_EGF1_h_m1p1_p80000exe2", "pero_EGF1_h_m1p1_p80000exe3", "pero_EGF1_h_m1p1_p80000exe4", "pero_EGF1_h_m1p1_p80000exe5", "pero_EGF1_h_m1p1_p80000exe6", "pero_EGF1_h_m1p1_p80000exe7", "pero_EGF1_h_m1p1_p80000exe8", "pero_EGF1_h_m1p1_p80000exe9", "pero_EGF1_h_m1p1_p800exe0", "pero_EGF1_h_m1p1_p800exe1", "pero_EGF1_h_m1p1_p800exe10", "pero_EGF1_h_m1p1_p800exe11", "pero_EGF1_h_m1p1_p800exe12", "pero_EGF1_h_m1p1_p800exe13", "pero_EGF1_h_m1p1_p800exe14", "pero_EGF1_h_m1p1_p800exe15", "pero_EGF1_h_m1p1_p800exe16", "pero_EGF1_h_m1p1_p800exe2", "pero_EGF1_h_m1p1_p800exe3", "pero_EGF1_h_m1p1_p800exe4", "pero_EGF1_h_m1p1_p800exe5", "pero_EGF1_h_m1p1_p800exe6", "pero_EGF1_h_m1p1_p800exe7", "pero_EGF1_h_m1p1_p800exe8", "pero_EGF1_h_m1p1_p800exe9", "pero_EGF1_h_m1p1_p900exe0", "pero_EGF1_h_m1p1_p900exe1", "pero_EGF1_h_m1p1_p900exe10", "pero_EGF1_h_m1p1_p900exe11", "pero_EGF1_h_m1p1_p900exe12", "pero_EGF1_h_m1p1_p900exe13", "pero_EGF1_h_m1p1_p900exe14", "pero_EGF1_h_m1p1_p900exe15", "pero_EGF1_h_m1p1_p900exe16", "pero_EGF1_h_m1p1_p900exe2", "pero_EGF1_h_m1p1_p900exe3", "pero_EGF1_h_m1p1_p900exe4", "pero_EGF1_h_m1p1_p900exe5", "pero_EGF1_h_m1p1_p900exe6", "pero_EGF1_h_m1p1_p900exe7", "pero_EGF1_h_m1p1_p900exe8", "pero_EGF1_h_m1p1_p900exe9", "pero_EGF1_h_p0m1_m0exe0", "pero_EGF1_h_p0m1_m0exe1", "pero_EGF1_h_p0m1_m0exe10", "pero_EGF1_h_p0m1_m0exe11", "pero_EGF1_h_p0m1_m0exe12", "pero_EGF1_h_p0m1_m0exe13", "pero_EGF1_h_p0m1_m0exe14", "pero_EGF1_h_p0m1_m0exe15", "pero_EGF1_h_p0m1_m0exe16", "pero_EGF1_h_p0m1_m0exe2", "pero_EGF1_h_p0m1_m0exe3", "pero_EGF1_h_p0m1_m0exe4", "pero_EGF1_h_p0m1_m0exe5", "pero_EGF1_h_p0m1_m0exe6", "pero_EGF1_h_p0m1_m0exe7", "pero_EGF1_h_p0m1_m0exe8", "pero_EGF1_h_p0m1_m0exe9", "pero_EGF1_h_p0m1_m100exe0", "pero_EGF1_h_p0m1_m100exe1", "pero_EGF1_h_p0m1_m100exe10", "pero_EGF1_h_p0m1_m100exe11", "pero_EGF1_h_p0m1_m100exe12", "pero_EGF1_h_p0m1_m100exe13", "pero_EGF1_h_p0m1_m100exe14", "pero_EGF1_h_p0m1_m100exe15", "pero_EGF1_h_p0m1_m100exe16", "pero_EGF1_h_p0m1_m100exe2", "pero_EGF1_h_p0m1_m100exe3", "pero_EGF1_h_p0m1_m100exe4", "pero_EGF1_h_p0m1_m100exe5", "pero_EGF1_h_p0m1_m100exe6", "pero_EGF1_h_p0m1_m100exe7", "pero_EGF1_h_p0m1_m100exe8", "pero_EGF1_h_p0m1_m100exe9", "pero_EGF1_h_p0m1_m200exe0", "pero_EGF1_h_p0m1_m200exe1", "pero_EGF1_h_p0m1_m200exe10", "pero_EGF1_h_p0m1_m200exe11", "pero_EGF1_h_p0m1_m200exe12", "pero_EGF1_h_p0m1_m200exe13", "pero_EGF1_h_p0m1_m200exe14", "pero_EGF1_h_p0m1_m200exe15", "pero_EGF1_h_p0m1_m200exe16", "pero_EGF1_h_p0m1_m200exe2", "pero_EGF1_h_p0m1_m200exe3", "pero_EGF1_h_p0m1_m200exe4", "pero_EGF1_h_p0m1_m200exe5", "pero_EGF1_h_p0m1_m200exe6", "pero_EGF1_h_p0m1_m200exe7", "pero_EGF1_h_p0m1_m200exe8", "pero_EGF1_h_p0m1_m200exe9", "pero_EGF1_h_p0m1_m300exe0", "pero_EGF1_h_p0m1_m300exe1", "pero_EGF1_h_p0m1_m300exe10", "pero_EGF1_h_p0m1_m300exe11", "pero_EGF1_h_p0m1_m300exe12", "pero_EGF1_h_p0m1_m300exe13", "pero_EGF1_h_p0m1_m300exe14", "pero_EGF1_h_p0m1_m300exe15", "pero_EGF1_h_p0m1_m300exe16", "pero_EGF1_h_p0m1_m300exe2", "pero_EGF1_h_p0m1_m300exe3", "pero_EGF1_h_p0m1_m300exe4", "pero_EGF1_h_p0m1_m300exe5", "pero_EGF1_h_p0m1_m300exe6", "pero_EGF1_h_p0m1_m300exe7", "pero_EGF1_h_p0m1_m300exe8", "pero_EGF1_h_p0m1_m300exe9", "pero_EGF1_h_p0m1_m5000exe0", "pero_EGF1_h_p0m1_m5000exe1", "pero_EGF1_h_p0m1_m5000exe10", "pero_EGF1_h_p0m1_m5000exe11", "pero_EGF1_h_p0m1_m5000exe12", "pero_EGF1_h_p0m1_m5000exe13", "pero_EGF1_h_p0m1_m5000exe14", "pero_EGF1_h_p0m1_m5000exe15", "pero_EGF1_h_p0m1_m5000exe16", "pero_EGF1_h_p0m1_m5000exe2", "pero_EGF1_h_p0m1_m5000exe3", "pero_EGF1_h_p0m1_m5000exe4", "pero_EGF1_h_p0m1_m5000exe5", "pero_EGF1_h_p0m1_m5000exe6", "pero_EGF1_h_p0m1_m5000exe7", "pero_EGF1_h_p0m1_m5000exe8", "pero_EGF1_h_p0m1_m5000exe9", "pero_EGF1_h_p0m1_m500exe0", "pero_EGF1_h_p0m1_m500exe1", "pero_EGF1_h_p0m1_m500exe10", "pero_EGF1_h_p0m1_m500exe11", "pero_EGF1_h_p0m1_m500exe12", "pero_EGF1_h_p0m1_m500exe13", "pero_EGF1_h_p0m1_m500exe14", "pero_EGF1_h_p0m1_m500exe15", "pero_EGF1_h_p0m1_m500exe16", "pero_EGF1_h_p0m1_m500exe2", "pero_EGF1_h_p0m1_m500exe3", "pero_EGF1_h_p0m1_m500exe4", "pero_EGF1_h_p0m1_m500exe5", "pero_EGF1_h_p0m1_m500exe6", "pero_EGF1_h_p0m1_m500exe7", "pero_EGF1_h_p0m1_m500exe8", "pero_EGF1_h_p0m1_m500exe9", "pero_EGF1_h_p0m1_p100000exe0", "pero_EGF1_h_p0m1_p100000exe1", "pero_EGF1_h_p0m1_p100000exe10", "pero_EGF1_h_p0m1_p100000exe11", "pero_EGF1_h_p0m1_p100000exe12", "pero_EGF1_h_p0m1_p100000exe13", "pero_EGF1_h_p0m1_p100000exe14", "pero_EGF1_h_p0m1_p100000exe15", "pero_EGF1_h_p0m1_p100000exe16", "pero_EGF1_h_p0m1_p100000exe2", "pero_EGF1_h_p0m1_p100000exe3", "pero_EGF1_h_p0m1_p100000exe4", "pero_EGF1_h_p0m1_p100000exe5", "pero_EGF1_h_p0m1_p100000exe6", "pero_EGF1_h_p0m1_p100000exe7", "pero_EGF1_h_p0m1_p100000exe8", "pero_EGF1_h_p0m1_p100000exe9", "pero_EGF1_h_p0m1_p10000exe0", "pero_EGF1_h_p0m1_p10000exe1", "pero_EGF1_h_p0m1_p10000exe10", "pero_EGF1_h_p0m1_p10000exe11", "pero_EGF1_h_p0m1_p10000exe12", "pero_EGF1_h_p0m1_p10000exe13", "pero_EGF1_h_p0m1_p10000exe14", "pero_EGF1_h_p0m1_p10000exe15", "pero_EGF1_h_p0m1_p10000exe16", "pero_EGF1_h_p0m1_p10000exe2", "pero_EGF1_h_p0m1_p10000exe3", "pero_EGF1_h_p0m1_p10000exe4", "pero_EGF1_h_p0m1_p10000exe5", "pero_EGF1_h_p0m1_p10000exe6", "pero_EGF1_h_p0m1_p10000exe7", "pero_EGF1_h_p0m1_p10000exe8", "pero_EGF1_h_p0m1_p10000exe9", "pero_EGF1_h_p0m1_p1000exe0", "pero_EGF1_h_p0m1_p1000exe1", "pero_EGF1_h_p0m1_p1000exe10", "pero_EGF1_h_p0m1_p1000exe11", "pero_EGF1_h_p0m1_p1000exe12", "pero_EGF1_h_p0m1_p1000exe13", "pero_EGF1_h_p0m1_p1000exe14", "pero_EGF1_h_p0m1_p1000exe15", "pero_EGF1_h_p0m1_p1000exe16", "pero_EGF1_h_p0m1_p1000exe17", "pero_EGF1_h_p0m1_p1000exe2", "pero_EGF1_h_p0m1_p1000exe3", "pero_EGF1_h_p0m1_p1000exe4", "pero_EGF1_h_p0m1_p1000exe5", "pero_EGF1_h_p0m1_p1000exe6", "pero_EGF1_h_p0m1_p1000exe7", "pero_EGF1_h_p0m1_p1000exe8", "pero_EGF1_h_p0m1_p1000exe9", "pero_EGF1_h_p0m1_p100exe0", "pero_EGF1_h_p0m1_p100exe1", "pero_EGF1_h_p0m1_p100exe10", "pero_EGF1_h_p0m1_p100exe11", "pero_EGF1_h_p0m1_p100exe12", "pero_EGF1_h_p0m1_p100exe13", "pero_EGF1_h_p0m1_p100exe14", "pero_EGF1_h_p0m1_p100exe15", "pero_EGF1_h_p0m1_p100exe16", "pero_EGF1_h_p0m1_p100exe2", "pero_EGF1_h_p0m1_p100exe3", "pero_EGF1_h_p0m1_p100exe4", "pero_EGF1_h_p0m1_p100exe5", "pero_EGF1_h_p0m1_p100exe6", "pero_EGF1_h_p0m1_p100exe7", "pero_EGF1_h_p0m1_p100exe8", "pero_EGF1_h_p0m1_p100exe9", "pero_EGF1_h_p0m1_p1100exe0", "pero_EGF1_h_p0m1_p1100exe1", "pero_EGF1_h_p0m1_p1100exe10", "pero_EGF1_h_p0m1_p1100exe11", "pero_EGF1_h_p0m1_p1100exe12", "pero_EGF1_h_p0m1_p1100exe13", "pero_EGF1_h_p0m1_p1100exe14", "pero_EGF1_h_p0m1_p1100exe15", "pero_EGF1_h_p0m1_p1100exe16", "pero_EGF1_h_p0m1_p1100exe2", "pero_EGF1_h_p0m1_p1100exe3", "pero_EGF1_h_p0m1_p1100exe4", "pero_EGF1_h_p0m1_p1100exe5", "pero_EGF1_h_p0m1_p1100exe6", "pero_EGF1_h_p0m1_p1100exe7", "pero_EGF1_h_p0m1_p1100exe8", "pero_EGF1_h_p0m1_p1100exe9", "pero_EGF1_h_p0m1_p120000exe0", "pero_EGF1_h_p0m1_p120000exe1", "pero_EGF1_h_p0m1_p120000exe10", "pero_EGF1_h_p0m1_p120000exe11", "pero_EGF1_h_p0m1_p120000exe12", "pero_EGF1_h_p0m1_p120000exe13", "pero_EGF1_h_p0m1_p120000exe14", "pero_EGF1_h_p0m1_p120000exe15", "pero_EGF1_h_p0m1_p120000exe16", "pero_EGF1_h_p0m1_p120000exe2", "pero_EGF1_h_p0m1_p120000exe3", "pero_EGF1_h_p0m1_p120000exe4", "pero_EGF1_h_p0m1_p120000exe5", "pero_EGF1_h_p0m1_p120000exe6", "pero_EGF1_h_p0m1_p120000exe7", "pero_EGF1_h_p0m1_p120000exe8", "pero_EGF1_h_p0m1_p120000exe9", "pero_EGF1_h_p0m1_p1200exe0", "pero_EGF1_h_p0m1_p1200exe1", "pero_EGF1_h_p0m1_p1200exe10", "pero_EGF1_h_p0m1_p1200exe11", "pero_EGF1_h_p0m1_p1200exe12", "pero_EGF1_h_p0m1_p1200exe13", "pero_EGF1_h_p0m1_p1200exe14", "pero_EGF1_h_p0m1_p1200exe15", "pero_EGF1_h_p0m1_p1200exe16", "pero_EGF1_h_p0m1_p1200exe2", "pero_EGF1_h_p0m1_p1200exe3", "pero_EGF1_h_p0m1_p1200exe4", "pero_EGF1_h_p0m1_p1200exe5", "pero_EGF1_h_p0m1_p1200exe6", "pero_EGF1_h_p0m1_p1200exe7", "pero_EGF1_h_p0m1_p1200exe8", "pero_EGF1_h_p0m1_p1200exe9", "pero_EGF1_h_p0m1_p1300exe0", "pero_EGF1_h_p0m1_p1300exe1", "pero_EGF1_h_p0m1_p1300exe10", "pero_EGF1_h_p0m1_p1300exe11", "pero_EGF1_h_p0m1_p1300exe12", "pero_EGF1_h_p0m1_p1300exe13", "pero_EGF1_h_p0m1_p1300exe14", "pero_EGF1_h_p0m1_p1300exe15", "pero_EGF1_h_p0m1_p1300exe16", "pero_EGF1_h_p0m1_p1300exe2", "pero_EGF1_h_p0m1_p1300exe3", "pero_EGF1_h_p0m1_p1300exe4", "pero_EGF1_h_p0m1_p1300exe5", "pero_EGF1_h_p0m1_p1300exe6", "pero_EGF1_h_p0m1_p1300exe7", "pero_EGF1_h_p0m1_p1300exe8", "pero_EGF1_h_p0m1_p1300exe9", "pero_EGF1_h_p0m1_p140000exe0", "pero_EGF1_h_p0m1_p140000exe1", "pero_EGF1_h_p0m1_p140000exe10", "pero_EGF1_h_p0m1_p140000exe11", "pero_EGF1_h_p0m1_p140000exe12", "pero_EGF1_h_p0m1_p140000exe13", "pero_EGF1_h_p0m1_p140000exe14", "pero_EGF1_h_p0m1_p140000exe15", "pero_EGF1_h_p0m1_p140000exe16", "pero_EGF1_h_p0m1_p140000exe2", "pero_EGF1_h_p0m1_p140000exe3", "pero_EGF1_h_p0m1_p140000exe4", "pero_EGF1_h_p0m1_p140000exe5", "pero_EGF1_h_p0m1_p140000exe6", "pero_EGF1_h_p0m1_p140000exe7", "pero_EGF1_h_p0m1_p140000exe8", "pero_EGF1_h_p0m1_p140000exe9", "pero_EGF1_h_p0m1_p1400exe0", "pero_EGF1_h_p0m1_p1400exe1", "pero_EGF1_h_p0m1_p1400exe10", "pero_EGF1_h_p0m1_p1400exe11", "pero_EGF1_h_p0m1_p1400exe12", "pero_EGF1_h_p0m1_p1400exe13", "pero_EGF1_h_p0m1_p1400exe14", "pero_EGF1_h_p0m1_p1400exe15", "pero_EGF1_h_p0m1_p1400exe16", "pero_EGF1_h_p0m1_p1400exe2", "pero_EGF1_h_p0m1_p1400exe3", "pero_EGF1_h_p0m1_p1400exe4", "pero_EGF1_h_p0m1_p1400exe5", "pero_EGF1_h_p0m1_p1400exe6", "pero_EGF1_h_p0m1_p1400exe7", "pero_EGF1_h_p0m1_p1400exe8", "pero_EGF1_h_p0m1_p1400exe9", "pero_EGF1_h_p0m1_p1500exe0", "pero_EGF1_h_p0m1_p1500exe1", "pero_EGF1_h_p0m1_p1500exe10", "pero_EGF1_h_p0m1_p1500exe11", "pero_EGF1_h_p0m1_p1500exe12", "pero_EGF1_h_p0m1_p1500exe13", "pero_EGF1_h_p0m1_p1500exe14", "pero_EGF1_h_p0m1_p1500exe15", "pero_EGF1_h_p0m1_p1500exe16", "pero_EGF1_h_p0m1_p1500exe2", "pero_EGF1_h_p0m1_p1500exe3", "pero_EGF1_h_p0m1_p1500exe4", "pero_EGF1_h_p0m1_p1500exe5", "pero_EGF1_h_p0m1_p1500exe6", "pero_EGF1_h_p0m1_p1500exe7", "pero_EGF1_h_p0m1_p1500exe8", "pero_EGF1_h_p0m1_p1500exe9", "pero_EGF1_h_p0m1_p160000exe0", "pero_EGF1_h_p0m1_p160000exe1", "pero_EGF1_h_p0m1_p160000exe10", "pero_EGF1_h_p0m1_p160000exe11", "pero_EGF1_h_p0m1_p160000exe12", "pero_EGF1_h_p0m1_p160000exe13", "pero_EGF1_h_p0m1_p160000exe14", "pero_EGF1_h_p0m1_p160000exe15", "pero_EGF1_h_p0m1_p160000exe16", "pero_EGF1_h_p0m1_p160000exe2", "pero_EGF1_h_p0m1_p160000exe3", "pero_EGF1_h_p0m1_p160000exe4", "pero_EGF1_h_p0m1_p160000exe5", "pero_EGF1_h_p0m1_p160000exe6", "pero_EGF1_h_p0m1_p160000exe7", "pero_EGF1_h_p0m1_p160000exe8", "pero_EGF1_h_p0m1_p160000exe9", "pero_EGF1_h_p0m1_p1600exe0", "pero_EGF1_h_p0m1_p1600exe1", "pero_EGF1_h_p0m1_p1600exe10", "pero_EGF1_h_p0m1_p1600exe11", "pero_EGF1_h_p0m1_p1600exe12", "pero_EGF1_h_p0m1_p1600exe13", "pero_EGF1_h_p0m1_p1600exe14", "pero_EGF1_h_p0m1_p1600exe15", "pero_EGF1_h_p0m1_p1600exe16", "pero_EGF1_h_p0m1_p1600exe2", "pero_EGF1_h_p0m1_p1600exe3", "pero_EGF1_h_p0m1_p1600exe4", "pero_EGF1_h_p0m1_p1600exe5", "pero_EGF1_h_p0m1_p1600exe6", "pero_EGF1_h_p0m1_p1600exe7", "pero_EGF1_h_p0m1_p1600exe8", "pero_EGF1_h_p0m1_p1600exe9", "pero_EGF1_h_p0m1_p1700exe0", "pero_EGF1_h_p0m1_p1700exe1", "pero_EGF1_h_p0m1_p1700exe10", "pero_EGF1_h_p0m1_p1700exe11", "pero_EGF1_h_p0m1_p1700exe12", "pero_EGF1_h_p0m1_p1700exe13", "pero_EGF1_h_p0m1_p1700exe14", "pero_EGF1_h_p0m1_p1700exe15", "pero_EGF1_h_p0m1_p1700exe16", "pero_EGF1_h_p0m1_p1700exe2", "pero_EGF1_h_p0m1_p1700exe3", "pero_EGF1_h_p0m1_p1700exe4", "pero_EGF1_h_p0m1_p1700exe5", "pero_EGF1_h_p0m1_p1700exe6", "pero_EGF1_h_p0m1_p1700exe7", "pero_EGF1_h_p0m1_p1700exe8", "pero_EGF1_h_p0m1_p1700exe9", "pero_EGF1_h_p0m1_p180000exe0", "pero_EGF1_h_p0m1_p180000exe1", "pero_EGF1_h_p0m1_p180000exe10", "pero_EGF1_h_p0m1_p180000exe11", "pero_EGF1_h_p0m1_p180000exe12", "pero_EGF1_h_p0m1_p180000exe13", "pero_EGF1_h_p0m1_p180000exe14", "pero_EGF1_h_p0m1_p180000exe15", "pero_EGF1_h_p0m1_p180000exe16", "pero_EGF1_h_p0m1_p180000exe2", "pero_EGF1_h_p0m1_p180000exe3", "pero_EGF1_h_p0m1_p180000exe4", "pero_EGF1_h_p0m1_p180000exe5", "pero_EGF1_h_p0m1_p180000exe6", "pero_EGF1_h_p0m1_p180000exe7", "pero_EGF1_h_p0m1_p180000exe8", "pero_EGF1_h_p0m1_p180000exe9", "pero_EGF1_h_p0m1_p1800exe0", "pero_EGF1_h_p0m1_p1800exe1", "pero_EGF1_h_p0m1_p1800exe10", "pero_EGF1_h_p0m1_p1800exe11", "pero_EGF1_h_p0m1_p1800exe12", "pero_EGF1_h_p0m1_p1800exe13", "pero_EGF1_h_p0m1_p1800exe14", "pero_EGF1_h_p0m1_p1800exe15", "pero_EGF1_h_p0m1_p1800exe16", "pero_EGF1_h_p0m1_p1800exe2", "pero_EGF1_h_p0m1_p1800exe3", "pero_EGF1_h_p0m1_p1800exe4", "pero_EGF1_h_p0m1_p1800exe5", "pero_EGF1_h_p0m1_p1800exe6", "pero_EGF1_h_p0m1_p1800exe7", "pero_EGF1_h_p0m1_p1800exe8", "pero_EGF1_h_p0m1_p1800exe9", "pero_EGF1_h_p0m1_p1900exe0", "pero_EGF1_h_p0m1_p1900exe1", "pero_EGF1_h_p0m1_p1900exe10", "pero_EGF1_h_p0m1_p1900exe11", "pero_EGF1_h_p0m1_p1900exe12", "pero_EGF1_h_p0m1_p1900exe13", "pero_EGF1_h_p0m1_p1900exe14", "pero_EGF1_h_p0m1_p1900exe15", "pero_EGF1_h_p0m1_p1900exe16", "pero_EGF1_h_p0m1_p1900exe17", "pero_EGF1_h_p0m1_p1900exe2", "pero_EGF1_h_p0m1_p1900exe3", "pero_EGF1_h_p0m1_p1900exe4", "pero_EGF1_h_p0m1_p1900exe5", "pero_EGF1_h_p0m1_p1900exe6", "pero_EGF1_h_p0m1_p1900exe7", "pero_EGF1_h_p0m1_p1900exe8", "pero_EGF1_h_p0m1_p1900exe9", "pero_EGF1_h_p0m1_p200000exe0", "pero_EGF1_h_p0m1_p200000exe1", "pero_EGF1_h_p0m1_p200000exe10", "pero_EGF1_h_p0m1_p200000exe11", "pero_EGF1_h_p0m1_p200000exe12", "pero_EGF1_h_p0m1_p200000exe13", "pero_EGF1_h_p0m1_p200000exe14", "pero_EGF1_h_p0m1_p200000exe15", "pero_EGF1_h_p0m1_p200000exe16", "pero_EGF1_h_p0m1_p200000exe2", "pero_EGF1_h_p0m1_p200000exe3", "pero_EGF1_h_p0m1_p200000exe4", "pero_EGF1_h_p0m1_p200000exe5", "pero_EGF1_h_p0m1_p200000exe6", "pero_EGF1_h_p0m1_p200000exe7", "pero_EGF1_h_p0m1_p200000exe8", "pero_EGF1_h_p0m1_p200000exe9", "pero_EGF1_h_p0m1_p20000exe0", "pero_EGF1_h_p0m1_p20000exe1", "pero_EGF1_h_p0m1_p20000exe10", "pero_EGF1_h_p0m1_p20000exe11", "pero_EGF1_h_p0m1_p20000exe12", "pero_EGF1_h_p0m1_p20000exe13", "pero_EGF1_h_p0m1_p20000exe14", "pero_EGF1_h_p0m1_p20000exe15", "pero_EGF1_h_p0m1_p20000exe16", "pero_EGF1_h_p0m1_p20000exe2", "pero_EGF1_h_p0m1_p20000exe3", "pero_EGF1_h_p0m1_p20000exe4", "pero_EGF1_h_p0m1_p20000exe5", "pero_EGF1_h_p0m1_p20000exe6", "pero_EGF1_h_p0m1_p20000exe7", "pero_EGF1_h_p0m1_p20000exe8", "pero_EGF1_h_p0m1_p20000exe9", "pero_EGF1_h_p0m1_p2000exe0", "pero_EGF1_h_p0m1_p2000exe1", "pero_EGF1_h_p0m1_p2000exe10", "pero_EGF1_h_p0m1_p2000exe11", "pero_EGF1_h_p0m1_p2000exe12", "pero_EGF1_h_p0m1_p2000exe13", "pero_EGF1_h_p0m1_p2000exe14", "pero_EGF1_h_p0m1_p2000exe15", "pero_EGF1_h_p0m1_p2000exe16", "pero_EGF1_h_p0m1_p2000exe2", "pero_EGF1_h_p0m1_p2000exe3", "pero_EGF1_h_p0m1_p2000exe4", "pero_EGF1_h_p0m1_p2000exe5", "pero_EGF1_h_p0m1_p2000exe6", "pero_EGF1_h_p0m1_p2000exe7", "pero_EGF1_h_p0m1_p2000exe8", "pero_EGF1_h_p0m1_p2000exe9", "pero_EGF1_h_p0m1_p200exe0", "pero_EGF1_h_p0m1_p200exe1", "pero_EGF1_h_p0m1_p200exe10", "pero_EGF1_h_p0m1_p200exe11", "pero_EGF1_h_p0m1_p200exe12", "pero_EGF1_h_p0m1_p200exe13", "pero_EGF1_h_p0m1_p200exe14", "pero_EGF1_h_p0m1_p200exe15", "pero_EGF1_h_p0m1_p200exe16", "pero_EGF1_h_p0m1_p200exe2", "pero_EGF1_h_p0m1_p200exe3", "pero_EGF1_h_p0m1_p200exe4", "pero_EGF1_h_p0m1_p200exe5", "pero_EGF1_h_p0m1_p200exe6", "pero_EGF1_h_p0m1_p200exe7", "pero_EGF1_h_p0m1_p200exe8", "pero_EGF1_h_p0m1_p200exe9", "pero_EGF1_h_p0m1_p2100exe0", "pero_EGF1_h_p0m1_p2100exe1", "pero_EGF1_h_p0m1_p2100exe10", "pero_EGF1_h_p0m1_p2100exe11", "pero_EGF1_h_p0m1_p2100exe12", "pero_EGF1_h_p0m1_p2100exe13", "pero_EGF1_h_p0m1_p2100exe14", "pero_EGF1_h_p0m1_p2100exe15", "pero_EGF1_h_p0m1_p2100exe16", "pero_EGF1_h_p0m1_p2100exe2", "pero_EGF1_h_p0m1_p2100exe3", "pero_EGF1_h_p0m1_p2100exe4", "pero_EGF1_h_p0m1_p2100exe5", "pero_EGF1_h_p0m1_p2100exe6", "pero_EGF1_h_p0m1_p2100exe7", "pero_EGF1_h_p0m1_p2100exe8", "pero_EGF1_h_p0m1_p2100exe9", "pero_EGF1_h_p0m1_p220000exe0", "pero_EGF1_h_p0m1_p220000exe1", "pero_EGF1_h_p0m1_p220000exe10", "pero_EGF1_h_p0m1_p220000exe11", "pero_EGF1_h_p0m1_p220000exe12", "pero_EGF1_h_p0m1_p220000exe13", "pero_EGF1_h_p0m1_p220000exe14", "pero_EGF1_h_p0m1_p220000exe15", "pero_EGF1_h_p0m1_p220000exe16", "pero_EGF1_h_p0m1_p220000exe2", "pero_EGF1_h_p0m1_p220000exe3", "pero_EGF1_h_p0m1_p220000exe4", "pero_EGF1_h_p0m1_p220000exe5", "pero_EGF1_h_p0m1_p220000exe6", "pero_EGF1_h_p0m1_p220000exe7", "pero_EGF1_h_p0m1_p220000exe8", "pero_EGF1_h_p0m1_p220000exe9", "pero_EGF1_h_p0m1_p2200exe0", "pero_EGF1_h_p0m1_p2200exe1", "pero_EGF1_h_p0m1_p2200exe10", "pero_EGF1_h_p0m1_p2200exe11", "pero_EGF1_h_p0m1_p2200exe12", "pero_EGF1_h_p0m1_p2200exe13", "pero_EGF1_h_p0m1_p2200exe14", "pero_EGF1_h_p0m1_p2200exe15", "pero_EGF1_h_p0m1_p2200exe16", "pero_EGF1_h_p0m1_p2200exe2", "pero_EGF1_h_p0m1_p2200exe3", "pero_EGF1_h_p0m1_p2200exe4", "pero_EGF1_h_p0m1_p2200exe5", "pero_EGF1_h_p0m1_p2200exe6", "pero_EGF1_h_p0m1_p2200exe7", "pero_EGF1_h_p0m1_p2200exe8", "pero_EGF1_h_p0m1_p2200exe9", "pero_EGF1_h_p0m1_p2300exe0", "pero_EGF1_h_p0m1_p2300exe1", "pero_EGF1_h_p0m1_p2300exe10", "pero_EGF1_h_p0m1_p2300exe11", "pero_EGF1_h_p0m1_p2300exe12", "pero_EGF1_h_p0m1_p2300exe13", "pero_EGF1_h_p0m1_p2300exe14", "pero_EGF1_h_p0m1_p2300exe15", "pero_EGF1_h_p0m1_p2300exe16", "pero_EGF1_h_p0m1_p2300exe17", "pero_EGF1_h_p0m1_p2300exe2", "pero_EGF1_h_p0m1_p2300exe3", "pero_EGF1_h_p0m1_p2300exe4", "pero_EGF1_h_p0m1_p2300exe5", "pero_EGF1_h_p0m1_p2300exe6", "pero_EGF1_h_p0m1_p2300exe7", "pero_EGF1_h_p0m1_p2300exe8", "pero_EGF1_h_p0m1_p2300exe9", "pero_EGF1_h_p0m1_p240000exe0", "pero_EGF1_h_p0m1_p240000exe1", "pero_EGF1_h_p0m1_p240000exe10", "pero_EGF1_h_p0m1_p240000exe11", "pero_EGF1_h_p0m1_p240000exe12", "pero_EGF1_h_p0m1_p240000exe13", "pero_EGF1_h_p0m1_p240000exe14", "pero_EGF1_h_p0m1_p240000exe15", "pero_EGF1_h_p0m1_p240000exe16", "pero_EGF1_h_p0m1_p240000exe2", "pero_EGF1_h_p0m1_p240000exe3", "pero_EGF1_h_p0m1_p240000exe4", "pero_EGF1_h_p0m1_p240000exe5", "pero_EGF1_h_p0m1_p240000exe6", "pero_EGF1_h_p0m1_p240000exe7", "pero_EGF1_h_p0m1_p240000exe8", "pero_EGF1_h_p0m1_p240000exe9", "pero_EGF1_h_p0m1_p2400exe0", "pero_EGF1_h_p0m1_p2400exe1", "pero_EGF1_h_p0m1_p2400exe10", "pero_EGF1_h_p0m1_p2400exe11", "pero_EGF1_h_p0m1_p2400exe12", "pero_EGF1_h_p0m1_p2400exe13", "pero_EGF1_h_p0m1_p2400exe14", "pero_EGF1_h_p0m1_p2400exe15", "pero_EGF1_h_p0m1_p2400exe16", "pero_EGF1_h_p0m1_p2400exe2", "pero_EGF1_h_p0m1_p2400exe3", "pero_EGF1_h_p0m1_p2400exe4", "pero_EGF1_h_p0m1_p2400exe5", "pero_EGF1_h_p0m1_p2400exe6", "pero_EGF1_h_p0m1_p2400exe7", "pero_EGF1_h_p0m1_p2400exe8", "pero_EGF1_h_p0m1_p2400exe9", "pero_EGF1_h_p0m1_p2500exe0", "pero_EGF1_h_p0m1_p2500exe1", "pero_EGF1_h_p0m1_p2500exe10", "pero_EGF1_h_p0m1_p2500exe11", "pero_EGF1_h_p0m1_p2500exe12", "pero_EGF1_h_p0m1_p2500exe13", "pero_EGF1_h_p0m1_p2500exe14", "pero_EGF1_h_p0m1_p2500exe15", "pero_EGF1_h_p0m1_p2500exe16", "pero_EGF1_h_p0m1_p2500exe2", "pero_EGF1_h_p0m1_p2500exe3", "pero_EGF1_h_p0m1_p2500exe4", "pero_EGF1_h_p0m1_p2500exe5", "pero_EGF1_h_p0m1_p2500exe6", "pero_EGF1_h_p0m1_p2500exe7", "pero_EGF1_h_p0m1_p2500exe8", "pero_EGF1_h_p0m1_p2500exe9", "pero_EGF1_h_p0m1_p260000exe0", "pero_EGF1_h_p0m1_p260000exe1", "pero_EGF1_h_p0m1_p260000exe10", "pero_EGF1_h_p0m1_p260000exe11", "pero_EGF1_h_p0m1_p260000exe12", "pero_EGF1_h_p0m1_p260000exe13", "pero_EGF1_h_p0m1_p260000exe14", "pero_EGF1_h_p0m1_p260000exe15", "pero_EGF1_h_p0m1_p260000exe16", "pero_EGF1_h_p0m1_p260000exe2", "pero_EGF1_h_p0m1_p260000exe3", "pero_EGF1_h_p0m1_p260000exe4", "pero_EGF1_h_p0m1_p260000exe5", "pero_EGF1_h_p0m1_p260000exe6", "pero_EGF1_h_p0m1_p260000exe7", "pero_EGF1_h_p0m1_p260000exe8", "pero_EGF1_h_p0m1_p260000exe9", "pero_EGF1_h_p0m1_p2600exe0", "pero_EGF1_h_p0m1_p2600exe1", "pero_EGF1_h_p0m1_p2600exe10", "pero_EGF1_h_p0m1_p2600exe11", "pero_EGF1_h_p0m1_p2600exe12", "pero_EGF1_h_p0m1_p2600exe13", "pero_EGF1_h_p0m1_p2600exe14", "pero_EGF1_h_p0m1_p2600exe15", "pero_EGF1_h_p0m1_p2600exe16", "pero_EGF1_h_p0m1_p2600exe2", "pero_EGF1_h_p0m1_p2600exe3", "pero_EGF1_h_p0m1_p2600exe4", "pero_EGF1_h_p0m1_p2600exe5", "pero_EGF1_h_p0m1_p2600exe6", "pero_EGF1_h_p0m1_p2600exe7", "pero_EGF1_h_p0m1_p2600exe8", "pero_EGF1_h_p0m1_p2600exe9", "pero_EGF1_h_p0m1_p2700exe0", "pero_EGF1_h_p0m1_p2700exe1", "pero_EGF1_h_p0m1_p2700exe10", "pero_EGF1_h_p0m1_p2700exe11", "pero_EGF1_h_p0m1_p2700exe12", "pero_EGF1_h_p0m1_p2700exe13", "pero_EGF1_h_p0m1_p2700exe14", "pero_EGF1_h_p0m1_p2700exe15", "pero_EGF1_h_p0m1_p2700exe16", "pero_EGF1_h_p0m1_p2700exe2", "pero_EGF1_h_p0m1_p2700exe3", "pero_EGF1_h_p0m1_p2700exe4", "pero_EGF1_h_p0m1_p2700exe5", "pero_EGF1_h_p0m1_p2700exe6", "pero_EGF1_h_p0m1_p2700exe7", "pero_EGF1_h_p0m1_p2700exe8", "pero_EGF1_h_p0m1_p2700exe9", "pero_EGF1_h_p0m1_p280000exe0", "pero_EGF1_h_p0m1_p280000exe1", "pero_EGF1_h_p0m1_p280000exe10", "pero_EGF1_h_p0m1_p280000exe11", "pero_EGF1_h_p0m1_p280000exe12", "pero_EGF1_h_p0m1_p280000exe13", "pero_EGF1_h_p0m1_p280000exe14", "pero_EGF1_h_p0m1_p280000exe15", "pero_EGF1_h_p0m1_p280000exe16", "pero_EGF1_h_p0m1_p280000exe2", "pero_EGF1_h_p0m1_p280000exe3", "pero_EGF1_h_p0m1_p280000exe4", "pero_EGF1_h_p0m1_p280000exe5", "pero_EGF1_h_p0m1_p280000exe6", "pero_EGF1_h_p0m1_p280000exe7", "pero_EGF1_h_p0m1_p280000exe8", "pero_EGF1_h_p0m1_p280000exe9", "pero_EGF1_h_p0m1_p2800exe0", "pero_EGF1_h_p0m1_p2800exe1", "pero_EGF1_h_p0m1_p2800exe10", "pero_EGF1_h_p0m1_p2800exe11", "pero_EGF1_h_p0m1_p2800exe12", "pero_EGF1_h_p0m1_p2800exe13", "pero_EGF1_h_p0m1_p2800exe14", "pero_EGF1_h_p0m1_p2800exe15", "pero_EGF1_h_p0m1_p2800exe16", "pero_EGF1_h_p0m1_p2800exe2", "pero_EGF1_h_p0m1_p2800exe3", "pero_EGF1_h_p0m1_p2800exe4", "pero_EGF1_h_p0m1_p2800exe5", "pero_EGF1_h_p0m1_p2800exe6", "pero_EGF1_h_p0m1_p2800exe7", "pero_EGF1_h_p0m1_p2800exe8", "pero_EGF1_h_p0m1_p2800exe9", "pero_EGF1_h_p0m1_p2900exe0", "pero_EGF1_h_p0m1_p2900exe1", "pero_EGF1_h_p0m1_p2900exe10", "pero_EGF1_h_p0m1_p2900exe11", "pero_EGF1_h_p0m1_p2900exe12", "pero_EGF1_h_p0m1_p2900exe13", "pero_EGF1_h_p0m1_p2900exe14", "pero_EGF1_h_p0m1_p2900exe15", "pero_EGF1_h_p0m1_p2900exe16", "pero_EGF1_h_p0m1_p2900exe2", "pero_EGF1_h_p0m1_p2900exe3", "pero_EGF1_h_p0m1_p2900exe4", "pero_EGF1_h_p0m1_p2900exe5", "pero_EGF1_h_p0m1_p2900exe6", "pero_EGF1_h_p0m1_p2900exe7", "pero_EGF1_h_p0m1_p2900exe8", "pero_EGF1_h_p0m1_p2900exe9", "pero_EGF1_h_p0m1_p300000exe0", "pero_EGF1_h_p0m1_p300000exe1", "pero_EGF1_h_p0m1_p300000exe10", "pero_EGF1_h_p0m1_p300000exe11", "pero_EGF1_h_p0m1_p300000exe12", "pero_EGF1_h_p0m1_p300000exe13", "pero_EGF1_h_p0m1_p300000exe14", "pero_EGF1_h_p0m1_p300000exe15", "pero_EGF1_h_p0m1_p300000exe16", "pero_EGF1_h_p0m1_p300000exe2", "pero_EGF1_h_p0m1_p300000exe3", "pero_EGF1_h_p0m1_p300000exe4", "pero_EGF1_h_p0m1_p300000exe5", "pero_EGF1_h_p0m1_p300000exe6", "pero_EGF1_h_p0m1_p300000exe7", "pero_EGF1_h_p0m1_p300000exe8", "pero_EGF1_h_p0m1_p300000exe9", "pero_EGF1_h_p0m1_p30000exe0", "pero_EGF1_h_p0m1_p30000exe1", "pero_EGF1_h_p0m1_p30000exe10", "pero_EGF1_h_p0m1_p30000exe11", "pero_EGF1_h_p0m1_p30000exe12", "pero_EGF1_h_p0m1_p30000exe13", "pero_EGF1_h_p0m1_p30000exe14", "pero_EGF1_h_p0m1_p30000exe15", "pero_EGF1_h_p0m1_p30000exe16", "pero_EGF1_h_p0m1_p30000exe2", "pero_EGF1_h_p0m1_p30000exe3", "pero_EGF1_h_p0m1_p30000exe4", "pero_EGF1_h_p0m1_p30000exe5", "pero_EGF1_h_p0m1_p30000exe6", "pero_EGF1_h_p0m1_p30000exe7", "pero_EGF1_h_p0m1_p30000exe8", "pero_EGF1_h_p0m1_p30000exe9", "pero_EGF1_h_p0m1_p3000exe0", "pero_EGF1_h_p0m1_p3000exe1", "pero_EGF1_h_p0m1_p3000exe10", "pero_EGF1_h_p0m1_p3000exe11", "pero_EGF1_h_p0m1_p3000exe12", "pero_EGF1_h_p0m1_p3000exe13", "pero_EGF1_h_p0m1_p3000exe14", "pero_EGF1_h_p0m1_p3000exe15", "pero_EGF1_h_p0m1_p3000exe16", "pero_EGF1_h_p0m1_p3000exe17", "pero_EGF1_h_p0m1_p3000exe2", "pero_EGF1_h_p0m1_p3000exe3", "pero_EGF1_h_p0m1_p3000exe4", "pero_EGF1_h_p0m1_p3000exe5", "pero_EGF1_h_p0m1_p3000exe6", "pero_EGF1_h_p0m1_p3000exe7", "pero_EGF1_h_p0m1_p3000exe8", "pero_EGF1_h_p0m1_p3000exe9", "pero_EGF1_h_p0m1_p300exe0", "pero_EGF1_h_p0m1_p300exe1", "pero_EGF1_h_p0m1_p300exe10", "pero_EGF1_h_p0m1_p300exe11", "pero_EGF1_h_p0m1_p300exe12", "pero_EGF1_h_p0m1_p300exe13", "pero_EGF1_h_p0m1_p300exe14", "pero_EGF1_h_p0m1_p300exe15", "pero_EGF1_h_p0m1_p300exe16", "pero_EGF1_h_p0m1_p300exe2", "pero_EGF1_h_p0m1_p300exe3", "pero_EGF1_h_p0m1_p300exe4", "pero_EGF1_h_p0m1_p300exe5", "pero_EGF1_h_p0m1_p300exe6", "pero_EGF1_h_p0m1_p300exe7", "pero_EGF1_h_p0m1_p300exe8", "pero_EGF1_h_p0m1_p300exe9", "pero_EGF1_h_p0m1_p320000exe0", "pero_EGF1_h_p0m1_p320000exe1", "pero_EGF1_h_p0m1_p320000exe10", "pero_EGF1_h_p0m1_p320000exe11", "pero_EGF1_h_p0m1_p320000exe12", "pero_EGF1_h_p0m1_p320000exe13", "pero_EGF1_h_p0m1_p320000exe14", "pero_EGF1_h_p0m1_p320000exe15", "pero_EGF1_h_p0m1_p320000exe16", "pero_EGF1_h_p0m1_p320000exe2", "pero_EGF1_h_p0m1_p320000exe3", "pero_EGF1_h_p0m1_p320000exe4", "pero_EGF1_h_p0m1_p320000exe5", "pero_EGF1_h_p0m1_p320000exe6", "pero_EGF1_h_p0m1_p320000exe7", "pero_EGF1_h_p0m1_p320000exe8", "pero_EGF1_h_p0m1_p320000exe9", "pero_EGF1_h_p0m1_p340000exe0", "pero_EGF1_h_p0m1_p340000exe1", "pero_EGF1_h_p0m1_p340000exe10", "pero_EGF1_h_p0m1_p340000exe11", "pero_EGF1_h_p0m1_p340000exe12", "pero_EGF1_h_p0m1_p340000exe13", "pero_EGF1_h_p0m1_p340000exe14", "pero_EGF1_h_p0m1_p340000exe15", "pero_EGF1_h_p0m1_p340000exe16", "pero_EGF1_h_p0m1_p340000exe2", "pero_EGF1_h_p0m1_p340000exe3", "pero_EGF1_h_p0m1_p340000exe4", "pero_EGF1_h_p0m1_p340000exe5", "pero_EGF1_h_p0m1_p340000exe6", "pero_EGF1_h_p0m1_p340000exe7", "pero_EGF1_h_p0m1_p340000exe8", "pero_EGF1_h_p0m1_p340000exe9", "pero_EGF1_h_p0m1_p360000exe0", "pero_EGF1_h_p0m1_p360000exe1", "pero_EGF1_h_p0m1_p360000exe10", "pero_EGF1_h_p0m1_p360000exe11", "pero_EGF1_h_p0m1_p360000exe12", "pero_EGF1_h_p0m1_p360000exe13", "pero_EGF1_h_p0m1_p360000exe14", "pero_EGF1_h_p0m1_p360000exe15", "pero_EGF1_h_p0m1_p360000exe16", "pero_EGF1_h_p0m1_p360000exe2", "pero_EGF1_h_p0m1_p360000exe3", "pero_EGF1_h_p0m1_p360000exe4", "pero_EGF1_h_p0m1_p360000exe5", "pero_EGF1_h_p0m1_p360000exe6", "pero_EGF1_h_p0m1_p360000exe7", "pero_EGF1_h_p0m1_p360000exe8", "pero_EGF1_h_p0m1_p360000exe9", "pero_EGF1_h_p0m1_p380000exe0", "pero_EGF1_h_p0m1_p380000exe1", "pero_EGF1_h_p0m1_p380000exe10", "pero_EGF1_h_p0m1_p380000exe11", "pero_EGF1_h_p0m1_p380000exe12", "pero_EGF1_h_p0m1_p380000exe13", "pero_EGF1_h_p0m1_p380000exe14", "pero_EGF1_h_p0m1_p380000exe15", "pero_EGF1_h_p0m1_p380000exe16", "pero_EGF1_h_p0m1_p380000exe2", "pero_EGF1_h_p0m1_p380000exe3", "pero_EGF1_h_p0m1_p380000exe4", "pero_EGF1_h_p0m1_p380000exe5", "pero_EGF1_h_p0m1_p380000exe6", "pero_EGF1_h_p0m1_p380000exe7", "pero_EGF1_h_p0m1_p380000exe8", "pero_EGF1_h_p0m1_p380000exe9", "pero_EGF1_h_p0m1_p400000exe0", "pero_EGF1_h_p0m1_p400000exe1", "pero_EGF1_h_p0m1_p400000exe10", "pero_EGF1_h_p0m1_p400000exe11", "pero_EGF1_h_p0m1_p400000exe12", "pero_EGF1_h_p0m1_p400000exe13", "pero_EGF1_h_p0m1_p400000exe14", "pero_EGF1_h_p0m1_p400000exe15", "pero_EGF1_h_p0m1_p400000exe16", "pero_EGF1_h_p0m1_p400000exe2", "pero_EGF1_h_p0m1_p400000exe3", "pero_EGF1_h_p0m1_p400000exe4", "pero_EGF1_h_p0m1_p400000exe5", "pero_EGF1_h_p0m1_p400000exe6", "pero_EGF1_h_p0m1_p400000exe7", "pero_EGF1_h_p0m1_p400000exe8", "pero_EGF1_h_p0m1_p400000exe9", "pero_EGF1_h_p0m1_p40000exe0", "pero_EGF1_h_p0m1_p40000exe1", "pero_EGF1_h_p0m1_p40000exe10", "pero_EGF1_h_p0m1_p40000exe11", "pero_EGF1_h_p0m1_p40000exe12", "pero_EGF1_h_p0m1_p40000exe13", "pero_EGF1_h_p0m1_p40000exe14", "pero_EGF1_h_p0m1_p40000exe15", "pero_EGF1_h_p0m1_p40000exe16", "pero_EGF1_h_p0m1_p40000exe2", "pero_EGF1_h_p0m1_p40000exe3", "pero_EGF1_h_p0m1_p40000exe4", "pero_EGF1_h_p0m1_p40000exe5", "pero_EGF1_h_p0m1_p40000exe6", "pero_EGF1_h_p0m1_p40000exe7", "pero_EGF1_h_p0m1_p40000exe8", "pero_EGF1_h_p0m1_p40000exe9", "pero_EGF1_h_p0m1_p4000exe0", "pero_EGF1_h_p0m1_p4000exe1", "pero_EGF1_h_p0m1_p4000exe10", "pero_EGF1_h_p0m1_p4000exe11", "pero_EGF1_h_p0m1_p4000exe12", "pero_EGF1_h_p0m1_p4000exe13", "pero_EGF1_h_p0m1_p4000exe14", "pero_EGF1_h_p0m1_p4000exe15", "pero_EGF1_h_p0m1_p4000exe16", "pero_EGF1_h_p0m1_p4000exe2", "pero_EGF1_h_p0m1_p4000exe3", "pero_EGF1_h_p0m1_p4000exe4", "pero_EGF1_h_p0m1_p4000exe5", "pero_EGF1_h_p0m1_p4000exe6", "pero_EGF1_h_p0m1_p4000exe7", "pero_EGF1_h_p0m1_p4000exe8", "pero_EGF1_h_p0m1_p4000exe9", "pero_EGF1_h_p0m1_p400exe0", "pero_EGF1_h_p0m1_p400exe1", "pero_EGF1_h_p0m1_p400exe10", "pero_EGF1_h_p0m1_p400exe11", "pero_EGF1_h_p0m1_p400exe12", "pero_EGF1_h_p0m1_p400exe13", "pero_EGF1_h_p0m1_p400exe14", "pero_EGF1_h_p0m1_p400exe15", "pero_EGF1_h_p0m1_p400exe16", "pero_EGF1_h_p0m1_p400exe2", "pero_EGF1_h_p0m1_p400exe3", "pero_EGF1_h_p0m1_p400exe4", "pero_EGF1_h_p0m1_p400exe5", "pero_EGF1_h_p0m1_p400exe6", "pero_EGF1_h_p0m1_p400exe7", "pero_EGF1_h_p0m1_p400exe8", "pero_EGF1_h_p0m1_p400exe9", "pero_EGF1_h_p0m1_p420000exe0", "pero_EGF1_h_p0m1_p420000exe1", "pero_EGF1_h_p0m1_p420000exe10", "pero_EGF1_h_p0m1_p420000exe11", "pero_EGF1_h_p0m1_p420000exe12", "pero_EGF1_h_p0m1_p420000exe13", "pero_EGF1_h_p0m1_p420000exe14", "pero_EGF1_h_p0m1_p420000exe15", "pero_EGF1_h_p0m1_p420000exe16", "pero_EGF1_h_p0m1_p420000exe2", "pero_EGF1_h_p0m1_p420000exe3", "pero_EGF1_h_p0m1_p420000exe4", "pero_EGF1_h_p0m1_p420000exe5", "pero_EGF1_h_p0m1_p420000exe6", "pero_EGF1_h_p0m1_p420000exe7", "pero_EGF1_h_p0m1_p420000exe8", "pero_EGF1_h_p0m1_p420000exe9", "pero_EGF1_h_p0m1_p440000exe0", "pero_EGF1_h_p0m1_p440000exe1", "pero_EGF1_h_p0m1_p440000exe10", "pero_EGF1_h_p0m1_p440000exe11", "pero_EGF1_h_p0m1_p440000exe12", "pero_EGF1_h_p0m1_p440000exe13", "pero_EGF1_h_p0m1_p440000exe14", "pero_EGF1_h_p0m1_p440000exe15", "pero_EGF1_h_p0m1_p440000exe16", "pero_EGF1_h_p0m1_p440000exe2", "pero_EGF1_h_p0m1_p440000exe3", "pero_EGF1_h_p0m1_p440000exe4", "pero_EGF1_h_p0m1_p440000exe5", "pero_EGF1_h_p0m1_p440000exe6", "pero_EGF1_h_p0m1_p440000exe7", "pero_EGF1_h_p0m1_p440000exe8", "pero_EGF1_h_p0m1_p440000exe9", "pero_EGF1_h_p0m1_p480000exe0", "pero_EGF1_h_p0m1_p480000exe1", "pero_EGF1_h_p0m1_p480000exe10", "pero_EGF1_h_p0m1_p480000exe11", "pero_EGF1_h_p0m1_p480000exe12", "pero_EGF1_h_p0m1_p480000exe13", "pero_EGF1_h_p0m1_p480000exe14", "pero_EGF1_h_p0m1_p480000exe15", "pero_EGF1_h_p0m1_p480000exe16", "pero_EGF1_h_p0m1_p480000exe2", "pero_EGF1_h_p0m1_p480000exe3", "pero_EGF1_h_p0m1_p480000exe4", "pero_EGF1_h_p0m1_p480000exe5", "pero_EGF1_h_p0m1_p480000exe6", "pero_EGF1_h_p0m1_p480000exe7", "pero_EGF1_h_p0m1_p480000exe8", "pero_EGF1_h_p0m1_p480000exe9", "pero_EGF1_h_p0m1_p500000exe0", "pero_EGF1_h_p0m1_p500000exe1", "pero_EGF1_h_p0m1_p500000exe10", "pero_EGF1_h_p0m1_p500000exe11", "pero_EGF1_h_p0m1_p500000exe12", "pero_EGF1_h_p0m1_p500000exe13", "pero_EGF1_h_p0m1_p500000exe14", "pero_EGF1_h_p0m1_p500000exe15", "pero_EGF1_h_p0m1_p500000exe16", "pero_EGF1_h_p0m1_p500000exe2", "pero_EGF1_h_p0m1_p500000exe3", "pero_EGF1_h_p0m1_p500000exe4", "pero_EGF1_h_p0m1_p500000exe5", "pero_EGF1_h_p0m1_p500000exe6", "pero_EGF1_h_p0m1_p500000exe7", "pero_EGF1_h_p0m1_p500000exe8", "pero_EGF1_h_p0m1_p500000exe9", "pero_EGF1_h_p0m1_p50000exe0", "pero_EGF1_h_p0m1_p50000exe1", "pero_EGF1_h_p0m1_p50000exe10", "pero_EGF1_h_p0m1_p50000exe11", "pero_EGF1_h_p0m1_p50000exe12", "pero_EGF1_h_p0m1_p50000exe13", "pero_EGF1_h_p0m1_p50000exe14", "pero_EGF1_h_p0m1_p50000exe15", "pero_EGF1_h_p0m1_p50000exe16", "pero_EGF1_h_p0m1_p50000exe2", "pero_EGF1_h_p0m1_p50000exe3", "pero_EGF1_h_p0m1_p50000exe4", "pero_EGF1_h_p0m1_p50000exe5", "pero_EGF1_h_p0m1_p50000exe6", "pero_EGF1_h_p0m1_p50000exe7", "pero_EGF1_h_p0m1_p50000exe8", "pero_EGF1_h_p0m1_p50000exe9", "pero_EGF1_h_p0m1_p500exe0", "pero_EGF1_h_p0m1_p500exe1", "pero_EGF1_h_p0m1_p500exe10", "pero_EGF1_h_p0m1_p500exe11", "pero_EGF1_h_p0m1_p500exe12", "pero_EGF1_h_p0m1_p500exe13", "pero_EGF1_h_p0m1_p500exe14", "pero_EGF1_h_p0m1_p500exe15", "pero_EGF1_h_p0m1_p500exe16", "pero_EGF1_h_p0m1_p500exe2", "pero_EGF1_h_p0m1_p500exe3", "pero_EGF1_h_p0m1_p500exe4", "pero_EGF1_h_p0m1_p500exe5", "pero_EGF1_h_p0m1_p500exe6", "pero_EGF1_h_p0m1_p500exe7", "pero_EGF1_h_p0m1_p500exe8", "pero_EGF1_h_p0m1_p500exe9", "pero_EGF1_h_p0m1_p60000exe0", "pero_EGF1_h_p0m1_p60000exe1", "pero_EGF1_h_p0m1_p60000exe10", "pero_EGF1_h_p0m1_p60000exe11", "pero_EGF1_h_p0m1_p60000exe12", "pero_EGF1_h_p0m1_p60000exe13", "pero_EGF1_h_p0m1_p60000exe14", "pero_EGF1_h_p0m1_p60000exe15", "pero_EGF1_h_p0m1_p60000exe16", "pero_EGF1_h_p0m1_p60000exe2", "pero_EGF1_h_p0m1_p60000exe3", "pero_EGF1_h_p0m1_p60000exe4", "pero_EGF1_h_p0m1_p60000exe5", "pero_EGF1_h_p0m1_p60000exe6", "pero_EGF1_h_p0m1_p60000exe7", "pero_EGF1_h_p0m1_p60000exe8", "pero_EGF1_h_p0m1_p60000exe9", "pero_EGF1_h_p0m1_p6000exe0", "pero_EGF1_h_p0m1_p6000exe1", "pero_EGF1_h_p0m1_p6000exe10", "pero_EGF1_h_p0m1_p6000exe11", "pero_EGF1_h_p0m1_p6000exe12", "pero_EGF1_h_p0m1_p6000exe13", "pero_EGF1_h_p0m1_p6000exe14", "pero_EGF1_h_p0m1_p6000exe15", "pero_EGF1_h_p0m1_p6000exe16", "pero_EGF1_h_p0m1_p6000exe2", "pero_EGF1_h_p0m1_p6000exe3", "pero_EGF1_h_p0m1_p6000exe4", "pero_EGF1_h_p0m1_p6000exe5", "pero_EGF1_h_p0m1_p6000exe6", "pero_EGF1_h_p0m1_p6000exe7", "pero_EGF1_h_p0m1_p6000exe8", "pero_EGF1_h_p0m1_p6000exe9", "pero_EGF1_h_p0m1_p600exe0", "pero_EGF1_h_p0m1_p600exe1", "pero_EGF1_h_p0m1_p600exe10", "pero_EGF1_h_p0m1_p600exe11", "pero_EGF1_h_p0m1_p600exe12", "pero_EGF1_h_p0m1_p600exe13", "pero_EGF1_h_p0m1_p600exe14", "pero_EGF1_h_p0m1_p600exe15", "pero_EGF1_h_p0m1_p600exe16", "pero_EGF1_h_p0m1_p600exe17", "pero_EGF1_h_p0m1_p600exe2", "pero_EGF1_h_p0m1_p600exe3", "pero_EGF1_h_p0m1_p600exe4", "pero_EGF1_h_p0m1_p600exe5", "pero_EGF1_h_p0m1_p600exe6", "pero_EGF1_h_p0m1_p600exe7", "pero_EGF1_h_p0m1_p600exe8", "pero_EGF1_h_p0m1_p600exe9", "pero_EGF1_h_p0m1_p700exe0", "pero_EGF1_h_p0m1_p700exe1", "pero_EGF1_h_p0m1_p700exe10", "pero_EGF1_h_p0m1_p700exe11", "pero_EGF1_h_p0m1_p700exe12", "pero_EGF1_h_p0m1_p700exe13", "pero_EGF1_h_p0m1_p700exe14", "pero_EGF1_h_p0m1_p700exe15", "pero_EGF1_h_p0m1_p700exe16", "pero_EGF1_h_p0m1_p700exe2", "pero_EGF1_h_p0m1_p700exe3", "pero_EGF1_h_p0m1_p700exe4", "pero_EGF1_h_p0m1_p700exe5", "pero_EGF1_h_p0m1_p700exe6", "pero_EGF1_h_p0m1_p700exe7", "pero_EGF1_h_p0m1_p700exe8", "pero_EGF1_h_p0m1_p700exe9", "pero_EGF1_h_p0m1_p80000exe0", "pero_EGF1_h_p0m1_p80000exe1", "pero_EGF1_h_p0m1_p80000exe10", "pero_EGF1_h_p0m1_p80000exe11", "pero_EGF1_h_p0m1_p80000exe12", "pero_EGF1_h_p0m1_p80000exe13", "pero_EGF1_h_p0m1_p80000exe14", "pero_EGF1_h_p0m1_p80000exe15", "pero_EGF1_h_p0m1_p80000exe16", "pero_EGF1_h_p0m1_p80000exe2", "pero_EGF1_h_p0m1_p80000exe3", "pero_EGF1_h_p0m1_p80000exe4", "pero_EGF1_h_p0m1_p80000exe5", "pero_EGF1_h_p0m1_p80000exe6", "pero_EGF1_h_p0m1_p80000exe7", "pero_EGF1_h_p0m1_p80000exe8", "pero_EGF1_h_p0m1_p80000exe9", "pero_EGF1_h_p0m1_p800exe0", "pero_EGF1_h_p0m1_p800exe1", "pero_EGF1_h_p0m1_p800exe10", "pero_EGF1_h_p0m1_p800exe11", "pero_EGF1_h_p0m1_p800exe12", "pero_EGF1_h_p0m1_p800exe13", "pero_EGF1_h_p0m1_p800exe14", "pero_EGF1_h_p0m1_p800exe15", "pero_EGF1_h_p0m1_p800exe16", "pero_EGF1_h_p0m1_p800exe2", "pero_EGF1_h_p0m1_p800exe3", "pero_EGF1_h_p0m1_p800exe4", "pero_EGF1_h_p0m1_p800exe5", "pero_EGF1_h_p0m1_p800exe6", "pero_EGF1_h_p0m1_p800exe7", "pero_EGF1_h_p0m1_p800exe8", "pero_EGF1_h_p0m1_p800exe9", "pero_EGF1_h_p0m1_p900exe0", "pero_EGF1_h_p0m1_p900exe1", "pero_EGF1_h_p0m1_p900exe10", "pero_EGF1_h_p0m1_p900exe11", "pero_EGF1_h_p0m1_p900exe12", "pero_EGF1_h_p0m1_p900exe13", "pero_EGF1_h_p0m1_p900exe14", "pero_EGF1_h_p0m1_p900exe15", "pero_EGF1_h_p0m1_p900exe16", "pero_EGF1_h_p0m1_p900exe2", "pero_EGF1_h_p0m1_p900exe3", "pero_EGF1_h_p0m1_p900exe4", "pero_EGF1_h_p0m1_p900exe5", "pero_EGF1_h_p0m1_p900exe6", "pero_EGF1_h_p0m1_p900exe7", "pero_EGF1_h_p0m1_p900exe8", "pero_EGF1_h_p0m1_p900exe9", "pero_EGF1_h_p0p0_m0exe0", "pero_EGF1_h_p0p0_m0exe1", "pero_EGF1_h_p0p0_m0exe10", "pero_EGF1_h_p0p0_m0exe11", "pero_EGF1_h_p0p0_m0exe12", "pero_EGF1_h_p0p0_m0exe13", "pero_EGF1_h_p0p0_m0exe14", "pero_EGF1_h_p0p0_m0exe15", "pero_EGF1_h_p0p0_m0exe16", "pero_EGF1_h_p0p0_m0exe2", "pero_EGF1_h_p0p0_m0exe3", "pero_EGF1_h_p0p0_m0exe4", "pero_EGF1_h_p0p0_m0exe5", "pero_EGF1_h_p0p0_m0exe6", "pero_EGF1_h_p0p0_m0exe7", "pero_EGF1_h_p0p0_m0exe8", "pero_EGF1_h_p0p0_m0exe9", "pero_EGF1_h_p0p0_m100exe0", "pero_EGF1_h_p0p0_m100exe1", "pero_EGF1_h_p0p0_m100exe10", "pero_EGF1_h_p0p0_m100exe11", "pero_EGF1_h_p0p0_m100exe12", "pero_EGF1_h_p0p0_m100exe13", "pero_EGF1_h_p0p0_m100exe14", "pero_EGF1_h_p0p0_m100exe15", "pero_EGF1_h_p0p0_m100exe16", "pero_EGF1_h_p0p0_m100exe2", "pero_EGF1_h_p0p0_m100exe3", "pero_EGF1_h_p0p0_m100exe4", "pero_EGF1_h_p0p0_m100exe5", "pero_EGF1_h_p0p0_m100exe6", "pero_EGF1_h_p0p0_m100exe7", "pero_EGF1_h_p0p0_m100exe8", "pero_EGF1_h_p0p0_m100exe9", "pero_EGF1_h_p0p0_m200exe0", "pero_EGF1_h_p0p0_m200exe1", "pero_EGF1_h_p0p0_m200exe10", "pero_EGF1_h_p0p0_m200exe11", "pero_EGF1_h_p0p0_m200exe12", "pero_EGF1_h_p0p0_m200exe13", "pero_EGF1_h_p0p0_m200exe14", "pero_EGF1_h_p0p0_m200exe15", "pero_EGF1_h_p0p0_m200exe16", "pero_EGF1_h_p0p0_m200exe2", "pero_EGF1_h_p0p0_m200exe3", "pero_EGF1_h_p0p0_m200exe4", "pero_EGF1_h_p0p0_m200exe5", "pero_EGF1_h_p0p0_m200exe6", "pero_EGF1_h_p0p0_m200exe7", "pero_EGF1_h_p0p0_m200exe8", "pero_EGF1_h_p0p0_m200exe9", "pero_EGF1_h_p0p0_m300exe0", "pero_EGF1_h_p0p0_m300exe1", "pero_EGF1_h_p0p0_m300exe10", "pero_EGF1_h_p0p0_m300exe11", "pero_EGF1_h_p0p0_m300exe12", "pero_EGF1_h_p0p0_m300exe13", "pero_EGF1_h_p0p0_m300exe14", "pero_EGF1_h_p0p0_m300exe15", "pero_EGF1_h_p0p0_m300exe16", "pero_EGF1_h_p0p0_m300exe2", "pero_EGF1_h_p0p0_m300exe3", "pero_EGF1_h_p0p0_m300exe4", "pero_EGF1_h_p0p0_m300exe5", "pero_EGF1_h_p0p0_m300exe6", "pero_EGF1_h_p0p0_m300exe7", "pero_EGF1_h_p0p0_m300exe8", "pero_EGF1_h_p0p0_m300exe9", "pero_EGF1_h_p0p0_m5000exe0", "pero_EGF1_h_p0p0_m5000exe1", "pero_EGF1_h_p0p0_m5000exe10", "pero_EGF1_h_p0p0_m5000exe11", "pero_EGF1_h_p0p0_m5000exe12", "pero_EGF1_h_p0p0_m5000exe13", "pero_EGF1_h_p0p0_m5000exe14", "pero_EGF1_h_p0p0_m5000exe15", "pero_EGF1_h_p0p0_m5000exe16", "pero_EGF1_h_p0p0_m5000exe2", "pero_EGF1_h_p0p0_m5000exe3", "pero_EGF1_h_p0p0_m5000exe4", "pero_EGF1_h_p0p0_m5000exe5", "pero_EGF1_h_p0p0_m5000exe6", "pero_EGF1_h_p0p0_m5000exe7", "pero_EGF1_h_p0p0_m5000exe8", "pero_EGF1_h_p0p0_m5000exe9", "pero_EGF1_h_p0p0_m500exe0", "pero_EGF1_h_p0p0_m500exe1", "pero_EGF1_h_p0p0_m500exe10", "pero_EGF1_h_p0p0_m500exe11", "pero_EGF1_h_p0p0_m500exe12", "pero_EGF1_h_p0p0_m500exe13", "pero_EGF1_h_p0p0_m500exe14", "pero_EGF1_h_p0p0_m500exe15", "pero_EGF1_h_p0p0_m500exe16", "pero_EGF1_h_p0p0_m500exe2", "pero_EGF1_h_p0p0_m500exe3", "pero_EGF1_h_p0p0_m500exe4", "pero_EGF1_h_p0p0_m500exe5", "pero_EGF1_h_p0p0_m500exe6", "pero_EGF1_h_p0p0_m500exe7", "pero_EGF1_h_p0p0_m500exe8", "pero_EGF1_h_p0p0_m500exe9", "pero_EGF1_h_p0p0_p100000exe0", "pero_EGF1_h_p0p0_p100000exe1", "pero_EGF1_h_p0p0_p100000exe10", "pero_EGF1_h_p0p0_p100000exe11", "pero_EGF1_h_p0p0_p100000exe12", "pero_EGF1_h_p0p0_p100000exe13", "pero_EGF1_h_p0p0_p100000exe14", "pero_EGF1_h_p0p0_p100000exe15", "pero_EGF1_h_p0p0_p100000exe16", "pero_EGF1_h_p0p0_p100000exe2", "pero_EGF1_h_p0p0_p100000exe3", "pero_EGF1_h_p0p0_p100000exe4", "pero_EGF1_h_p0p0_p100000exe5", "pero_EGF1_h_p0p0_p100000exe6", "pero_EGF1_h_p0p0_p100000exe7", "pero_EGF1_h_p0p0_p100000exe8", "pero_EGF1_h_p0p0_p100000exe9", "pero_EGF1_h_p0p0_p10000exe0", "pero_EGF1_h_p0p0_p10000exe1", "pero_EGF1_h_p0p0_p10000exe10", "pero_EGF1_h_p0p0_p10000exe11", "pero_EGF1_h_p0p0_p10000exe12", "pero_EGF1_h_p0p0_p10000exe13", "pero_EGF1_h_p0p0_p10000exe14", "pero_EGF1_h_p0p0_p10000exe15", "pero_EGF1_h_p0p0_p10000exe16", "pero_EGF1_h_p0p0_p10000exe2", "pero_EGF1_h_p0p0_p10000exe3", "pero_EGF1_h_p0p0_p10000exe4", "pero_EGF1_h_p0p0_p10000exe5", "pero_EGF1_h_p0p0_p10000exe6", "pero_EGF1_h_p0p0_p10000exe7", "pero_EGF1_h_p0p0_p10000exe8", "pero_EGF1_h_p0p0_p10000exe9", "pero_EGF1_h_p0p0_p1000exe0", "pero_EGF1_h_p0p0_p1000exe1", "pero_EGF1_h_p0p0_p1000exe10", "pero_EGF1_h_p0p0_p1000exe11", "pero_EGF1_h_p0p0_p1000exe12", "pero_EGF1_h_p0p0_p1000exe13", "pero_EGF1_h_p0p0_p1000exe14", "pero_EGF1_h_p0p0_p1000exe15", "pero_EGF1_h_p0p0_p1000exe16", "pero_EGF1_h_p0p0_p1000exe17", "pero_EGF1_h_p0p0_p1000exe2", "pero_EGF1_h_p0p0_p1000exe3", "pero_EGF1_h_p0p0_p1000exe4", "pero_EGF1_h_p0p0_p1000exe5", "pero_EGF1_h_p0p0_p1000exe6", "pero_EGF1_h_p0p0_p1000exe7", "pero_EGF1_h_p0p0_p1000exe8", "pero_EGF1_h_p0p0_p1000exe9", "pero_EGF1_h_p0p0_p100exe0", "pero_EGF1_h_p0p0_p100exe1", "pero_EGF1_h_p0p0_p100exe10", "pero_EGF1_h_p0p0_p100exe11", "pero_EGF1_h_p0p0_p100exe12", "pero_EGF1_h_p0p0_p100exe13", "pero_EGF1_h_p0p0_p100exe14", "pero_EGF1_h_p0p0_p100exe15", "pero_EGF1_h_p0p0_p100exe16", "pero_EGF1_h_p0p0_p100exe2", "pero_EGF1_h_p0p0_p100exe3", "pero_EGF1_h_p0p0_p100exe4", "pero_EGF1_h_p0p0_p100exe5", "pero_EGF1_h_p0p0_p100exe6", "pero_EGF1_h_p0p0_p100exe7", "pero_EGF1_h_p0p0_p100exe8", "pero_EGF1_h_p0p0_p100exe9", "pero_EGF1_h_p0p0_p1100exe0", "pero_EGF1_h_p0p0_p1100exe1", "pero_EGF1_h_p0p0_p1100exe10", "pero_EGF1_h_p0p0_p1100exe11", "pero_EGF1_h_p0p0_p1100exe12", "pero_EGF1_h_p0p0_p1100exe13", "pero_EGF1_h_p0p0_p1100exe14", "pero_EGF1_h_p0p0_p1100exe15", "pero_EGF1_h_p0p0_p1100exe16", "pero_EGF1_h_p0p0_p1100exe2", "pero_EGF1_h_p0p0_p1100exe3", "pero_EGF1_h_p0p0_p1100exe4", "pero_EGF1_h_p0p0_p1100exe5", "pero_EGF1_h_p0p0_p1100exe6", "pero_EGF1_h_p0p0_p1100exe7", "pero_EGF1_h_p0p0_p1100exe8", "pero_EGF1_h_p0p0_p1100exe9", "pero_EGF1_h_p0p0_p120000exe0", "pero_EGF1_h_p0p0_p120000exe1", "pero_EGF1_h_p0p0_p120000exe10", "pero_EGF1_h_p0p0_p120000exe11", "pero_EGF1_h_p0p0_p120000exe12", "pero_EGF1_h_p0p0_p120000exe13", "pero_EGF1_h_p0p0_p120000exe14", "pero_EGF1_h_p0p0_p120000exe15", "pero_EGF1_h_p0p0_p120000exe16", "pero_EGF1_h_p0p0_p120000exe2", "pero_EGF1_h_p0p0_p120000exe3", "pero_EGF1_h_p0p0_p120000exe4", "pero_EGF1_h_p0p0_p120000exe5", "pero_EGF1_h_p0p0_p120000exe6", "pero_EGF1_h_p0p0_p120000exe7", "pero_EGF1_h_p0p0_p120000exe8", "pero_EGF1_h_p0p0_p120000exe9", "pero_EGF1_h_p0p0_p1200exe0", "pero_EGF1_h_p0p0_p1200exe1", "pero_EGF1_h_p0p0_p1200exe10", "pero_EGF1_h_p0p0_p1200exe11", "pero_EGF1_h_p0p0_p1200exe12", "pero_EGF1_h_p0p0_p1200exe13", "pero_EGF1_h_p0p0_p1200exe14", "pero_EGF1_h_p0p0_p1200exe15", "pero_EGF1_h_p0p0_p1200exe16", "pero_EGF1_h_p0p0_p1200exe2", "pero_EGF1_h_p0p0_p1200exe3", "pero_EGF1_h_p0p0_p1200exe4", "pero_EGF1_h_p0p0_p1200exe5", "pero_EGF1_h_p0p0_p1200exe6", "pero_EGF1_h_p0p0_p1200exe7", "pero_EGF1_h_p0p0_p1200exe8", "pero_EGF1_h_p0p0_p1200exe9", "pero_EGF1_h_p0p0_p1300exe0", "pero_EGF1_h_p0p0_p1300exe1", "pero_EGF1_h_p0p0_p1300exe10", "pero_EGF1_h_p0p0_p1300exe11", "pero_EGF1_h_p0p0_p1300exe12", "pero_EGF1_h_p0p0_p1300exe13", "pero_EGF1_h_p0p0_p1300exe14", "pero_EGF1_h_p0p0_p1300exe15", "pero_EGF1_h_p0p0_p1300exe16", "pero_EGF1_h_p0p0_p1300exe2", "pero_EGF1_h_p0p0_p1300exe3", "pero_EGF1_h_p0p0_p1300exe4", "pero_EGF1_h_p0p0_p1300exe5", "pero_EGF1_h_p0p0_p1300exe6", "pero_EGF1_h_p0p0_p1300exe7", "pero_EGF1_h_p0p0_p1300exe8", "pero_EGF1_h_p0p0_p1300exe9", "pero_EGF1_h_p0p0_p140000exe0", "pero_EGF1_h_p0p0_p140000exe1", "pero_EGF1_h_p0p0_p140000exe10", "pero_EGF1_h_p0p0_p140000exe11", "pero_EGF1_h_p0p0_p140000exe12", "pero_EGF1_h_p0p0_p140000exe13", "pero_EGF1_h_p0p0_p140000exe14", "pero_EGF1_h_p0p0_p140000exe15", "pero_EGF1_h_p0p0_p140000exe16", "pero_EGF1_h_p0p0_p140000exe2", "pero_EGF1_h_p0p0_p140000exe3", "pero_EGF1_h_p0p0_p140000exe4", "pero_EGF1_h_p0p0_p140000exe5", "pero_EGF1_h_p0p0_p140000exe6", "pero_EGF1_h_p0p0_p140000exe7", "pero_EGF1_h_p0p0_p140000exe8", "pero_EGF1_h_p0p0_p140000exe9", "pero_EGF1_h_p0p0_p1400exe0", "pero_EGF1_h_p0p0_p1400exe1", "pero_EGF1_h_p0p0_p1400exe10", "pero_EGF1_h_p0p0_p1400exe11", "pero_EGF1_h_p0p0_p1400exe12", "pero_EGF1_h_p0p0_p1400exe13", "pero_EGF1_h_p0p0_p1400exe14", "pero_EGF1_h_p0p0_p1400exe15", "pero_EGF1_h_p0p0_p1400exe16", "pero_EGF1_h_p0p0_p1400exe2", "pero_EGF1_h_p0p0_p1400exe3", "pero_EGF1_h_p0p0_p1400exe4", "pero_EGF1_h_p0p0_p1400exe5", "pero_EGF1_h_p0p0_p1400exe6", "pero_EGF1_h_p0p0_p1400exe7", "pero_EGF1_h_p0p0_p1400exe8", "pero_EGF1_h_p0p0_p1400exe9", "pero_EGF1_h_p0p0_p1500exe0", "pero_EGF1_h_p0p0_p1500exe1", "pero_EGF1_h_p0p0_p1500exe10", "pero_EGF1_h_p0p0_p1500exe11", "pero_EGF1_h_p0p0_p1500exe12", "pero_EGF1_h_p0p0_p1500exe13", "pero_EGF1_h_p0p0_p1500exe14", "pero_EGF1_h_p0p0_p1500exe15", "pero_EGF1_h_p0p0_p1500exe16", "pero_EGF1_h_p0p0_p1500exe2", "pero_EGF1_h_p0p0_p1500exe3", "pero_EGF1_h_p0p0_p1500exe4", "pero_EGF1_h_p0p0_p1500exe5", "pero_EGF1_h_p0p0_p1500exe6", "pero_EGF1_h_p0p0_p1500exe7", "pero_EGF1_h_p0p0_p1500exe8", "pero_EGF1_h_p0p0_p1500exe9", "pero_EGF1_h_p0p0_p160000exe0", "pero_EGF1_h_p0p0_p160000exe1", "pero_EGF1_h_p0p0_p160000exe10", "pero_EGF1_h_p0p0_p160000exe11", "pero_EGF1_h_p0p0_p160000exe12", "pero_EGF1_h_p0p0_p160000exe13", "pero_EGF1_h_p0p0_p160000exe14", "pero_EGF1_h_p0p0_p160000exe15", "pero_EGF1_h_p0p0_p160000exe16", "pero_EGF1_h_p0p0_p160000exe2", "pero_EGF1_h_p0p0_p160000exe3", "pero_EGF1_h_p0p0_p160000exe4", "pero_EGF1_h_p0p0_p160000exe5", "pero_EGF1_h_p0p0_p160000exe6", "pero_EGF1_h_p0p0_p160000exe7", "pero_EGF1_h_p0p0_p160000exe8", "pero_EGF1_h_p0p0_p160000exe9", "pero_EGF1_h_p0p0_p1600exe0", "pero_EGF1_h_p0p0_p1600exe1", "pero_EGF1_h_p0p0_p1600exe10", "pero_EGF1_h_p0p0_p1600exe11", "pero_EGF1_h_p0p0_p1600exe12", "pero_EGF1_h_p0p0_p1600exe13", "pero_EGF1_h_p0p0_p1600exe14", "pero_EGF1_h_p0p0_p1600exe15", "pero_EGF1_h_p0p0_p1600exe16", "pero_EGF1_h_p0p0_p1600exe2", "pero_EGF1_h_p0p0_p1600exe3", "pero_EGF1_h_p0p0_p1600exe4", "pero_EGF1_h_p0p0_p1600exe5", "pero_EGF1_h_p0p0_p1600exe6", "pero_EGF1_h_p0p0_p1600exe7", "pero_EGF1_h_p0p0_p1600exe8", "pero_EGF1_h_p0p0_p1600exe9", "pero_EGF1_h_p0p0_p1700exe0", "pero_EGF1_h_p0p0_p1700exe1", "pero_EGF1_h_p0p0_p1700exe10", "pero_EGF1_h_p0p0_p1700exe11", "pero_EGF1_h_p0p0_p1700exe12", "pero_EGF1_h_p0p0_p1700exe13", "pero_EGF1_h_p0p0_p1700exe14", "pero_EGF1_h_p0p0_p1700exe15", "pero_EGF1_h_p0p0_p1700exe16", "pero_EGF1_h_p0p0_p1700exe2", "pero_EGF1_h_p0p0_p1700exe3", "pero_EGF1_h_p0p0_p1700exe4", "pero_EGF1_h_p0p0_p1700exe5", "pero_EGF1_h_p0p0_p1700exe6", "pero_EGF1_h_p0p0_p1700exe7", "pero_EGF1_h_p0p0_p1700exe8", "pero_EGF1_h_p0p0_p1700exe9", "pero_EGF1_h_p0p0_p180000exe0", "pero_EGF1_h_p0p0_p180000exe1", "pero_EGF1_h_p0p0_p180000exe10", "pero_EGF1_h_p0p0_p180000exe11", "pero_EGF1_h_p0p0_p180000exe12", "pero_EGF1_h_p0p0_p180000exe13", "pero_EGF1_h_p0p0_p180000exe14", "pero_EGF1_h_p0p0_p180000exe15", "pero_EGF1_h_p0p0_p180000exe16", "pero_EGF1_h_p0p0_p180000exe2", "pero_EGF1_h_p0p0_p180000exe3", "pero_EGF1_h_p0p0_p180000exe4", "pero_EGF1_h_p0p0_p180000exe5", "pero_EGF1_h_p0p0_p180000exe6", "pero_EGF1_h_p0p0_p180000exe7", "pero_EGF1_h_p0p0_p180000exe8", "pero_EGF1_h_p0p0_p180000exe9", "pero_EGF1_h_p0p0_p1800exe0", "pero_EGF1_h_p0p0_p1800exe1", "pero_EGF1_h_p0p0_p1800exe10", "pero_EGF1_h_p0p0_p1800exe11", "pero_EGF1_h_p0p0_p1800exe12", "pero_EGF1_h_p0p0_p1800exe13", "pero_EGF1_h_p0p0_p1800exe14", "pero_EGF1_h_p0p0_p1800exe15", "pero_EGF1_h_p0p0_p1800exe16", "pero_EGF1_h_p0p0_p1800exe2", "pero_EGF1_h_p0p0_p1800exe3", "pero_EGF1_h_p0p0_p1800exe4", "pero_EGF1_h_p0p0_p1800exe5", "pero_EGF1_h_p0p0_p1800exe6", "pero_EGF1_h_p0p0_p1800exe7", "pero_EGF1_h_p0p0_p1800exe8", "pero_EGF1_h_p0p0_p1800exe9", "pero_EGF1_h_p0p0_p1900exe0", "pero_EGF1_h_p0p0_p1900exe1", "pero_EGF1_h_p0p0_p1900exe10", "pero_EGF1_h_p0p0_p1900exe11", "pero_EGF1_h_p0p0_p1900exe12", "pero_EGF1_h_p0p0_p1900exe13", "pero_EGF1_h_p0p0_p1900exe14", "pero_EGF1_h_p0p0_p1900exe15", "pero_EGF1_h_p0p0_p1900exe16", "pero_EGF1_h_p0p0_p1900exe17", "pero_EGF1_h_p0p0_p1900exe2", "pero_EGF1_h_p0p0_p1900exe3", "pero_EGF1_h_p0p0_p1900exe4", "pero_EGF1_h_p0p0_p1900exe5", "pero_EGF1_h_p0p0_p1900exe6", "pero_EGF1_h_p0p0_p1900exe7", "pero_EGF1_h_p0p0_p1900exe8", "pero_EGF1_h_p0p0_p1900exe9", "pero_EGF1_h_p0p0_p200000exe0", "pero_EGF1_h_p0p0_p200000exe1", "pero_EGF1_h_p0p0_p200000exe10", "pero_EGF1_h_p0p0_p200000exe11", "pero_EGF1_h_p0p0_p200000exe12", "pero_EGF1_h_p0p0_p200000exe13", "pero_EGF1_h_p0p0_p200000exe14", "pero_EGF1_h_p0p0_p200000exe15", "pero_EGF1_h_p0p0_p200000exe16", "pero_EGF1_h_p0p0_p200000exe2", "pero_EGF1_h_p0p0_p200000exe3", "pero_EGF1_h_p0p0_p200000exe4", "pero_EGF1_h_p0p0_p200000exe5", "pero_EGF1_h_p0p0_p200000exe6", "pero_EGF1_h_p0p0_p200000exe7", "pero_EGF1_h_p0p0_p200000exe8", "pero_EGF1_h_p0p0_p200000exe9", "pero_EGF1_h_p0p0_p20000exe0", "pero_EGF1_h_p0p0_p20000exe1", "pero_EGF1_h_p0p0_p20000exe10", "pero_EGF1_h_p0p0_p20000exe11", "pero_EGF1_h_p0p0_p20000exe12", "pero_EGF1_h_p0p0_p20000exe13", "pero_EGF1_h_p0p0_p20000exe14", "pero_EGF1_h_p0p0_p20000exe15", "pero_EGF1_h_p0p0_p20000exe16", "pero_EGF1_h_p0p0_p20000exe2", "pero_EGF1_h_p0p0_p20000exe3", "pero_EGF1_h_p0p0_p20000exe4", "pero_EGF1_h_p0p0_p20000exe5", "pero_EGF1_h_p0p0_p20000exe6", "pero_EGF1_h_p0p0_p20000exe7", "pero_EGF1_h_p0p0_p20000exe8", "pero_EGF1_h_p0p0_p20000exe9", "pero_EGF1_h_p0p0_p2000exe0", "pero_EGF1_h_p0p0_p2000exe1", "pero_EGF1_h_p0p0_p2000exe10", "pero_EGF1_h_p0p0_p2000exe11", "pero_EGF1_h_p0p0_p2000exe12", "pero_EGF1_h_p0p0_p2000exe13", "pero_EGF1_h_p0p0_p2000exe14", "pero_EGF1_h_p0p0_p2000exe15", "pero_EGF1_h_p0p0_p2000exe16", "pero_EGF1_h_p0p0_p2000exe2", "pero_EGF1_h_p0p0_p2000exe3", "pero_EGF1_h_p0p0_p2000exe4", "pero_EGF1_h_p0p0_p2000exe5", "pero_EGF1_h_p0p0_p2000exe6", "pero_EGF1_h_p0p0_p2000exe7", "pero_EGF1_h_p0p0_p2000exe8", "pero_EGF1_h_p0p0_p2000exe9", "pero_EGF1_h_p0p0_p200exe0", "pero_EGF1_h_p0p0_p200exe1", "pero_EGF1_h_p0p0_p200exe10", "pero_EGF1_h_p0p0_p200exe11", "pero_EGF1_h_p0p0_p200exe12", "pero_EGF1_h_p0p0_p200exe13", "pero_EGF1_h_p0p0_p200exe14", "pero_EGF1_h_p0p0_p200exe15", "pero_EGF1_h_p0p0_p200exe16", "pero_EGF1_h_p0p0_p200exe2", "pero_EGF1_h_p0p0_p200exe3", "pero_EGF1_h_p0p0_p200exe4", "pero_EGF1_h_p0p0_p200exe5", "pero_EGF1_h_p0p0_p200exe6", "pero_EGF1_h_p0p0_p200exe7", "pero_EGF1_h_p0p0_p200exe8", "pero_EGF1_h_p0p0_p200exe9", "pero_EGF1_h_p0p0_p2100exe0", "pero_EGF1_h_p0p0_p2100exe1", "pero_EGF1_h_p0p0_p2100exe10", "pero_EGF1_h_p0p0_p2100exe11", "pero_EGF1_h_p0p0_p2100exe12", "pero_EGF1_h_p0p0_p2100exe13", "pero_EGF1_h_p0p0_p2100exe14", "pero_EGF1_h_p0p0_p2100exe15", "pero_EGF1_h_p0p0_p2100exe16", "pero_EGF1_h_p0p0_p2100exe2", "pero_EGF1_h_p0p0_p2100exe3", "pero_EGF1_h_p0p0_p2100exe4", "pero_EGF1_h_p0p0_p2100exe5", "pero_EGF1_h_p0p0_p2100exe6", "pero_EGF1_h_p0p0_p2100exe7", "pero_EGF1_h_p0p0_p2100exe8", "pero_EGF1_h_p0p0_p2100exe9", "pero_EGF1_h_p0p0_p220000exe0", "pero_EGF1_h_p0p0_p220000exe1", "pero_EGF1_h_p0p0_p220000exe10", "pero_EGF1_h_p0p0_p220000exe11", "pero_EGF1_h_p0p0_p220000exe12", "pero_EGF1_h_p0p0_p220000exe13", "pero_EGF1_h_p0p0_p220000exe14", "pero_EGF1_h_p0p0_p220000exe15", "pero_EGF1_h_p0p0_p220000exe16", "pero_EGF1_h_p0p0_p220000exe2", "pero_EGF1_h_p0p0_p220000exe3", "pero_EGF1_h_p0p0_p220000exe4", "pero_EGF1_h_p0p0_p220000exe5", "pero_EGF1_h_p0p0_p220000exe6", "pero_EGF1_h_p0p0_p220000exe7", "pero_EGF1_h_p0p0_p220000exe8", "pero_EGF1_h_p0p0_p220000exe9", "pero_EGF1_h_p0p0_p2200exe0", "pero_EGF1_h_p0p0_p2200exe1", "pero_EGF1_h_p0p0_p2200exe10", "pero_EGF1_h_p0p0_p2200exe11", "pero_EGF1_h_p0p0_p2200exe12", "pero_EGF1_h_p0p0_p2200exe13", "pero_EGF1_h_p0p0_p2200exe14", "pero_EGF1_h_p0p0_p2200exe15", "pero_EGF1_h_p0p0_p2200exe16", "pero_EGF1_h_p0p0_p2200exe2", "pero_EGF1_h_p0p0_p2200exe3", "pero_EGF1_h_p0p0_p2200exe4", "pero_EGF1_h_p0p0_p2200exe5", "pero_EGF1_h_p0p0_p2200exe6", "pero_EGF1_h_p0p0_p2200exe7", "pero_EGF1_h_p0p0_p2200exe8", "pero_EGF1_h_p0p0_p2200exe9", "pero_EGF1_h_p0p0_p2300exe0", "pero_EGF1_h_p0p0_p2300exe1", "pero_EGF1_h_p0p0_p2300exe10", "pero_EGF1_h_p0p0_p2300exe11", "pero_EGF1_h_p0p0_p2300exe12", "pero_EGF1_h_p0p0_p2300exe13", "pero_EGF1_h_p0p0_p2300exe14", "pero_EGF1_h_p0p0_p2300exe15", "pero_EGF1_h_p0p0_p2300exe16", "pero_EGF1_h_p0p0_p2300exe17", "pero_EGF1_h_p0p0_p2300exe2", "pero_EGF1_h_p0p0_p2300exe3", "pero_EGF1_h_p0p0_p2300exe4", "pero_EGF1_h_p0p0_p2300exe5", "pero_EGF1_h_p0p0_p2300exe6", "pero_EGF1_h_p0p0_p2300exe7", "pero_EGF1_h_p0p0_p2300exe8", "pero_EGF1_h_p0p0_p2300exe9", "pero_EGF1_h_p0p0_p240000exe0", "pero_EGF1_h_p0p0_p240000exe1", "pero_EGF1_h_p0p0_p240000exe10", "pero_EGF1_h_p0p0_p240000exe11", "pero_EGF1_h_p0p0_p240000exe12", "pero_EGF1_h_p0p0_p240000exe13", "pero_EGF1_h_p0p0_p240000exe14", "pero_EGF1_h_p0p0_p240000exe15", "pero_EGF1_h_p0p0_p240000exe16", "pero_EGF1_h_p0p0_p240000exe2", "pero_EGF1_h_p0p0_p240000exe3", "pero_EGF1_h_p0p0_p240000exe4", "pero_EGF1_h_p0p0_p240000exe5", "pero_EGF1_h_p0p0_p240000exe6", "pero_EGF1_h_p0p0_p240000exe7", "pero_EGF1_h_p0p0_p240000exe8", "pero_EGF1_h_p0p0_p240000exe9", "pero_EGF1_h_p0p0_p2400exe0", "pero_EGF1_h_p0p0_p2400exe1", "pero_EGF1_h_p0p0_p2400exe10", "pero_EGF1_h_p0p0_p2400exe11", "pero_EGF1_h_p0p0_p2400exe12", "pero_EGF1_h_p0p0_p2400exe13", "pero_EGF1_h_p0p0_p2400exe14", "pero_EGF1_h_p0p0_p2400exe15", "pero_EGF1_h_p0p0_p2400exe16", "pero_EGF1_h_p0p0_p2400exe2", "pero_EGF1_h_p0p0_p2400exe3", "pero_EGF1_h_p0p0_p2400exe4", "pero_EGF1_h_p0p0_p2400exe5", "pero_EGF1_h_p0p0_p2400exe6", "pero_EGF1_h_p0p0_p2400exe7", "pero_EGF1_h_p0p0_p2400exe8", "pero_EGF1_h_p0p0_p2400exe9", "pero_EGF1_h_p0p0_p2500exe0", "pero_EGF1_h_p0p0_p2500exe1", "pero_EGF1_h_p0p0_p2500exe10", "pero_EGF1_h_p0p0_p2500exe11", "pero_EGF1_h_p0p0_p2500exe12", "pero_EGF1_h_p0p0_p2500exe13", "pero_EGF1_h_p0p0_p2500exe14", "pero_EGF1_h_p0p0_p2500exe15", "pero_EGF1_h_p0p0_p2500exe16", "pero_EGF1_h_p0p0_p2500exe2", "pero_EGF1_h_p0p0_p2500exe3", "pero_EGF1_h_p0p0_p2500exe4", "pero_EGF1_h_p0p0_p2500exe5", "pero_EGF1_h_p0p0_p2500exe6", "pero_EGF1_h_p0p0_p2500exe7", "pero_EGF1_h_p0p0_p2500exe8", "pero_EGF1_h_p0p0_p2500exe9", "pero_EGF1_h_p0p0_p260000exe0", "pero_EGF1_h_p0p0_p260000exe1", "pero_EGF1_h_p0p0_p260000exe10", "pero_EGF1_h_p0p0_p260000exe11", "pero_EGF1_h_p0p0_p260000exe12", "pero_EGF1_h_p0p0_p260000exe13", "pero_EGF1_h_p0p0_p260000exe14", "pero_EGF1_h_p0p0_p260000exe15", "pero_EGF1_h_p0p0_p260000exe16", "pero_EGF1_h_p0p0_p260000exe2", "pero_EGF1_h_p0p0_p260000exe3", "pero_EGF1_h_p0p0_p260000exe4", "pero_EGF1_h_p0p0_p260000exe5", "pero_EGF1_h_p0p0_p260000exe6", "pero_EGF1_h_p0p0_p260000exe7", "pero_EGF1_h_p0p0_p260000exe8", "pero_EGF1_h_p0p0_p260000exe9", "pero_EGF1_h_p0p0_p2600exe0", "pero_EGF1_h_p0p0_p2600exe1", "pero_EGF1_h_p0p0_p2600exe10", "pero_EGF1_h_p0p0_p2600exe11", "pero_EGF1_h_p0p0_p2600exe12", "pero_EGF1_h_p0p0_p2600exe13", "pero_EGF1_h_p0p0_p2600exe14", "pero_EGF1_h_p0p0_p2600exe15", "pero_EGF1_h_p0p0_p2600exe16", "pero_EGF1_h_p0p0_p2600exe2", "pero_EGF1_h_p0p0_p2600exe3", "pero_EGF1_h_p0p0_p2600exe4", "pero_EGF1_h_p0p0_p2600exe5", "pero_EGF1_h_p0p0_p2600exe6", "pero_EGF1_h_p0p0_p2600exe7", "pero_EGF1_h_p0p0_p2600exe8", "pero_EGF1_h_p0p0_p2600exe9", "pero_EGF1_h_p0p0_p2700exe0", "pero_EGF1_h_p0p0_p2700exe1", "pero_EGF1_h_p0p0_p2700exe10", "pero_EGF1_h_p0p0_p2700exe11", "pero_EGF1_h_p0p0_p2700exe12", "pero_EGF1_h_p0p0_p2700exe13", "pero_EGF1_h_p0p0_p2700exe14", "pero_EGF1_h_p0p0_p2700exe15", "pero_EGF1_h_p0p0_p2700exe16", "pero_EGF1_h_p0p0_p2700exe2", "pero_EGF1_h_p0p0_p2700exe3", "pero_EGF1_h_p0p0_p2700exe4", "pero_EGF1_h_p0p0_p2700exe5", "pero_EGF1_h_p0p0_p2700exe6", "pero_EGF1_h_p0p0_p2700exe7", "pero_EGF1_h_p0p0_p2700exe8", "pero_EGF1_h_p0p0_p2700exe9", "pero_EGF1_h_p0p0_p280000exe0", "pero_EGF1_h_p0p0_p280000exe1", "pero_EGF1_h_p0p0_p280000exe10", "pero_EGF1_h_p0p0_p280000exe11", "pero_EGF1_h_p0p0_p280000exe12", "pero_EGF1_h_p0p0_p280000exe13", "pero_EGF1_h_p0p0_p280000exe14", "pero_EGF1_h_p0p0_p280000exe15", "pero_EGF1_h_p0p0_p280000exe16", "pero_EGF1_h_p0p0_p280000exe2", "pero_EGF1_h_p0p0_p280000exe3", "pero_EGF1_h_p0p0_p280000exe4", "pero_EGF1_h_p0p0_p280000exe5", "pero_EGF1_h_p0p0_p280000exe6", "pero_EGF1_h_p0p0_p280000exe7", "pero_EGF1_h_p0p0_p280000exe8", "pero_EGF1_h_p0p0_p280000exe9", "pero_EGF1_h_p0p0_p2800exe0", "pero_EGF1_h_p0p0_p2800exe1", "pero_EGF1_h_p0p0_p2800exe10", "pero_EGF1_h_p0p0_p2800exe11", "pero_EGF1_h_p0p0_p2800exe12", "pero_EGF1_h_p0p0_p2800exe13", "pero_EGF1_h_p0p0_p2800exe14", "pero_EGF1_h_p0p0_p2800exe15", "pero_EGF1_h_p0p0_p2800exe16", "pero_EGF1_h_p0p0_p2800exe2", "pero_EGF1_h_p0p0_p2800exe3", "pero_EGF1_h_p0p0_p2800exe4", "pero_EGF1_h_p0p0_p2800exe5", "pero_EGF1_h_p0p0_p2800exe6", "pero_EGF1_h_p0p0_p2800exe7", "pero_EGF1_h_p0p0_p2800exe8", "pero_EGF1_h_p0p0_p2800exe9", "pero_EGF1_h_p0p0_p2900exe0", "pero_EGF1_h_p0p0_p2900exe1", "pero_EGF1_h_p0p0_p2900exe10", "pero_EGF1_h_p0p0_p2900exe11", "pero_EGF1_h_p0p0_p2900exe12", "pero_EGF1_h_p0p0_p2900exe13", "pero_EGF1_h_p0p0_p2900exe14", "pero_EGF1_h_p0p0_p2900exe15", "pero_EGF1_h_p0p0_p2900exe16", "pero_EGF1_h_p0p0_p2900exe2", "pero_EGF1_h_p0p0_p2900exe3", "pero_EGF1_h_p0p0_p2900exe4", "pero_EGF1_h_p0p0_p2900exe5", "pero_EGF1_h_p0p0_p2900exe6", "pero_EGF1_h_p0p0_p2900exe7", "pero_EGF1_h_p0p0_p2900exe8", "pero_EGF1_h_p0p0_p2900exe9", "pero_EGF1_h_p0p0_p300000exe0", "pero_EGF1_h_p0p0_p300000exe1", "pero_EGF1_h_p0p0_p300000exe10", "pero_EGF1_h_p0p0_p300000exe11", "pero_EGF1_h_p0p0_p300000exe12", "pero_EGF1_h_p0p0_p300000exe13", "pero_EGF1_h_p0p0_p300000exe14", "pero_EGF1_h_p0p0_p300000exe15", "pero_EGF1_h_p0p0_p300000exe16", "pero_EGF1_h_p0p0_p300000exe2", "pero_EGF1_h_p0p0_p300000exe3", "pero_EGF1_h_p0p0_p300000exe4", "pero_EGF1_h_p0p0_p300000exe5", "pero_EGF1_h_p0p0_p300000exe6", "pero_EGF1_h_p0p0_p300000exe7", "pero_EGF1_h_p0p0_p300000exe8", "pero_EGF1_h_p0p0_p300000exe9", "pero_EGF1_h_p0p0_p30000exe0", "pero_EGF1_h_p0p0_p30000exe1", "pero_EGF1_h_p0p0_p30000exe10", "pero_EGF1_h_p0p0_p30000exe11", "pero_EGF1_h_p0p0_p30000exe12", "pero_EGF1_h_p0p0_p30000exe13", "pero_EGF1_h_p0p0_p30000exe14", "pero_EGF1_h_p0p0_p30000exe15", "pero_EGF1_h_p0p0_p30000exe16", "pero_EGF1_h_p0p0_p30000exe2", "pero_EGF1_h_p0p0_p30000exe3", "pero_EGF1_h_p0p0_p30000exe4", "pero_EGF1_h_p0p0_p30000exe5", "pero_EGF1_h_p0p0_p30000exe6", "pero_EGF1_h_p0p0_p30000exe7", "pero_EGF1_h_p0p0_p30000exe8", "pero_EGF1_h_p0p0_p30000exe9", "pero_EGF1_h_p0p0_p3000exe0", "pero_EGF1_h_p0p0_p3000exe1", "pero_EGF1_h_p0p0_p3000exe10", "pero_EGF1_h_p0p0_p3000exe11", "pero_EGF1_h_p0p0_p3000exe12", "pero_EGF1_h_p0p0_p3000exe13", "pero_EGF1_h_p0p0_p3000exe14", "pero_EGF1_h_p0p0_p3000exe15", "pero_EGF1_h_p0p0_p3000exe16", "pero_EGF1_h_p0p0_p3000exe17", "pero_EGF1_h_p0p0_p3000exe2", "pero_EGF1_h_p0p0_p3000exe3", "pero_EGF1_h_p0p0_p3000exe4", "pero_EGF1_h_p0p0_p3000exe5", "pero_EGF1_h_p0p0_p3000exe6", "pero_EGF1_h_p0p0_p3000exe7", "pero_EGF1_h_p0p0_p3000exe8", "pero_EGF1_h_p0p0_p3000exe9", "pero_EGF1_h_p0p0_p300exe0", "pero_EGF1_h_p0p0_p300exe1", "pero_EGF1_h_p0p0_p300exe10", "pero_EGF1_h_p0p0_p300exe11", "pero_EGF1_h_p0p0_p300exe12", "pero_EGF1_h_p0p0_p300exe13", "pero_EGF1_h_p0p0_p300exe14", "pero_EGF1_h_p0p0_p300exe15", "pero_EGF1_h_p0p0_p300exe16", "pero_EGF1_h_p0p0_p300exe2", "pero_EGF1_h_p0p0_p300exe3", "pero_EGF1_h_p0p0_p300exe4", "pero_EGF1_h_p0p0_p300exe5", "pero_EGF1_h_p0p0_p300exe6", "pero_EGF1_h_p0p0_p300exe7", "pero_EGF1_h_p0p0_p300exe8", "pero_EGF1_h_p0p0_p300exe9", "pero_EGF1_h_p0p0_p320000exe0", "pero_EGF1_h_p0p0_p320000exe1", "pero_EGF1_h_p0p0_p320000exe10", "pero_EGF1_h_p0p0_p320000exe11", "pero_EGF1_h_p0p0_p320000exe12", "pero_EGF1_h_p0p0_p320000exe13", "pero_EGF1_h_p0p0_p320000exe14", "pero_EGF1_h_p0p0_p320000exe15", "pero_EGF1_h_p0p0_p320000exe16", "pero_EGF1_h_p0p0_p320000exe2", "pero_EGF1_h_p0p0_p320000exe3", "pero_EGF1_h_p0p0_p320000exe4", "pero_EGF1_h_p0p0_p320000exe5", "pero_EGF1_h_p0p0_p320000exe6", "pero_EGF1_h_p0p0_p320000exe7", "pero_EGF1_h_p0p0_p320000exe8", "pero_EGF1_h_p0p0_p320000exe9", "pero_EGF1_h_p0p0_p340000exe0", "pero_EGF1_h_p0p0_p340000exe1", "pero_EGF1_h_p0p0_p340000exe10", "pero_EGF1_h_p0p0_p340000exe11", "pero_EGF1_h_p0p0_p340000exe12", "pero_EGF1_h_p0p0_p340000exe13", "pero_EGF1_h_p0p0_p340000exe14", "pero_EGF1_h_p0p0_p340000exe15", "pero_EGF1_h_p0p0_p340000exe16", "pero_EGF1_h_p0p0_p340000exe2", "pero_EGF1_h_p0p0_p340000exe3", "pero_EGF1_h_p0p0_p340000exe4", "pero_EGF1_h_p0p0_p340000exe5", "pero_EGF1_h_p0p0_p340000exe6", "pero_EGF1_h_p0p0_p340000exe7", "pero_EGF1_h_p0p0_p340000exe8", "pero_EGF1_h_p0p0_p340000exe9", "pero_EGF1_h_p0p0_p360000exe0", "pero_EGF1_h_p0p0_p360000exe1", "pero_EGF1_h_p0p0_p360000exe10", "pero_EGF1_h_p0p0_p360000exe11", "pero_EGF1_h_p0p0_p360000exe12", "pero_EGF1_h_p0p0_p360000exe13", "pero_EGF1_h_p0p0_p360000exe14", "pero_EGF1_h_p0p0_p360000exe15", "pero_EGF1_h_p0p0_p360000exe16", "pero_EGF1_h_p0p0_p360000exe2", "pero_EGF1_h_p0p0_p360000exe3", "pero_EGF1_h_p0p0_p360000exe4", "pero_EGF1_h_p0p0_p360000exe5", "pero_EGF1_h_p0p0_p360000exe6", "pero_EGF1_h_p0p0_p360000exe7", "pero_EGF1_h_p0p0_p360000exe8", "pero_EGF1_h_p0p0_p360000exe9", "pero_EGF1_h_p0p0_p380000exe0", "pero_EGF1_h_p0p0_p380000exe1", "pero_EGF1_h_p0p0_p380000exe10", "pero_EGF1_h_p0p0_p380000exe11", "pero_EGF1_h_p0p0_p380000exe12", "pero_EGF1_h_p0p0_p380000exe13", "pero_EGF1_h_p0p0_p380000exe14", "pero_EGF1_h_p0p0_p380000exe15", "pero_EGF1_h_p0p0_p380000exe16", "pero_EGF1_h_p0p0_p380000exe2", "pero_EGF1_h_p0p0_p380000exe3", "pero_EGF1_h_p0p0_p380000exe4", "pero_EGF1_h_p0p0_p380000exe5", "pero_EGF1_h_p0p0_p380000exe6", "pero_EGF1_h_p0p0_p380000exe7", "pero_EGF1_h_p0p0_p380000exe8", "pero_EGF1_h_p0p0_p380000exe9", "pero_EGF1_h_p0p0_p400000exe0", "pero_EGF1_h_p0p0_p400000exe1", "pero_EGF1_h_p0p0_p400000exe10", "pero_EGF1_h_p0p0_p400000exe11", "pero_EGF1_h_p0p0_p400000exe12", "pero_EGF1_h_p0p0_p400000exe13", "pero_EGF1_h_p0p0_p400000exe14", "pero_EGF1_h_p0p0_p400000exe15", "pero_EGF1_h_p0p0_p400000exe16", "pero_EGF1_h_p0p0_p400000exe2", "pero_EGF1_h_p0p0_p400000exe3", "pero_EGF1_h_p0p0_p400000exe4", "pero_EGF1_h_p0p0_p400000exe5", "pero_EGF1_h_p0p0_p400000exe6", "pero_EGF1_h_p0p0_p400000exe7", "pero_EGF1_h_p0p0_p400000exe8", "pero_EGF1_h_p0p0_p400000exe9", "pero_EGF1_h_p0p0_p40000exe0", "pero_EGF1_h_p0p0_p40000exe1", "pero_EGF1_h_p0p0_p40000exe10", "pero_EGF1_h_p0p0_p40000exe11", "pero_EGF1_h_p0p0_p40000exe12", "pero_EGF1_h_p0p0_p40000exe13", "pero_EGF1_h_p0p0_p40000exe14", "pero_EGF1_h_p0p0_p40000exe15", "pero_EGF1_h_p0p0_p40000exe16", "pero_EGF1_h_p0p0_p40000exe2", "pero_EGF1_h_p0p0_p40000exe3", "pero_EGF1_h_p0p0_p40000exe4", "pero_EGF1_h_p0p0_p40000exe5", "pero_EGF1_h_p0p0_p40000exe6", "pero_EGF1_h_p0p0_p40000exe7", "pero_EGF1_h_p0p0_p40000exe8", "pero_EGF1_h_p0p0_p40000exe9", "pero_EGF1_h_p0p0_p4000exe0", "pero_EGF1_h_p0p0_p4000exe1", "pero_EGF1_h_p0p0_p4000exe10", "pero_EGF1_h_p0p0_p4000exe11", "pero_EGF1_h_p0p0_p4000exe12", "pero_EGF1_h_p0p0_p4000exe13", "pero_EGF1_h_p0p0_p4000exe14", "pero_EGF1_h_p0p0_p4000exe15", "pero_EGF1_h_p0p0_p4000exe16", "pero_EGF1_h_p0p0_p4000exe2", "pero_EGF1_h_p0p0_p4000exe3", "pero_EGF1_h_p0p0_p4000exe4", "pero_EGF1_h_p0p0_p4000exe5", "pero_EGF1_h_p0p0_p4000exe6", "pero_EGF1_h_p0p0_p4000exe7", "pero_EGF1_h_p0p0_p4000exe8", "pero_EGF1_h_p0p0_p4000exe9", "pero_EGF1_h_p0p0_p400exe0", "pero_EGF1_h_p0p0_p400exe1", "pero_EGF1_h_p0p0_p400exe10", "pero_EGF1_h_p0p0_p400exe11", "pero_EGF1_h_p0p0_p400exe12", "pero_EGF1_h_p0p0_p400exe13", "pero_EGF1_h_p0p0_p400exe14", "pero_EGF1_h_p0p0_p400exe15", "pero_EGF1_h_p0p0_p400exe16", "pero_EGF1_h_p0p0_p400exe2", "pero_EGF1_h_p0p0_p400exe3", "pero_EGF1_h_p0p0_p400exe4", "pero_EGF1_h_p0p0_p400exe5", "pero_EGF1_h_p0p0_p400exe6", "pero_EGF1_h_p0p0_p400exe7", "pero_EGF1_h_p0p0_p400exe8", "pero_EGF1_h_p0p0_p400exe9", "pero_EGF1_h_p0p0_p420000exe0", "pero_EGF1_h_p0p0_p420000exe1", "pero_EGF1_h_p0p0_p420000exe10", "pero_EGF1_h_p0p0_p420000exe11", "pero_EGF1_h_p0p0_p420000exe12", "pero_EGF1_h_p0p0_p420000exe13", "pero_EGF1_h_p0p0_p420000exe14", "pero_EGF1_h_p0p0_p420000exe15", "pero_EGF1_h_p0p0_p420000exe16", "pero_EGF1_h_p0p0_p420000exe2", "pero_EGF1_h_p0p0_p420000exe3", "pero_EGF1_h_p0p0_p420000exe4", "pero_EGF1_h_p0p0_p420000exe5", "pero_EGF1_h_p0p0_p420000exe6", "pero_EGF1_h_p0p0_p420000exe7", "pero_EGF1_h_p0p0_p420000exe8", "pero_EGF1_h_p0p0_p420000exe9", "pero_EGF1_h_p0p0_p440000exe0", "pero_EGF1_h_p0p0_p440000exe1", "pero_EGF1_h_p0p0_p440000exe10", "pero_EGF1_h_p0p0_p440000exe11", "pero_EGF1_h_p0p0_p440000exe12", "pero_EGF1_h_p0p0_p440000exe13", "pero_EGF1_h_p0p0_p440000exe14", "pero_EGF1_h_p0p0_p440000exe15", "pero_EGF1_h_p0p0_p440000exe16", "pero_EGF1_h_p0p0_p440000exe2", "pero_EGF1_h_p0p0_p440000exe3", "pero_EGF1_h_p0p0_p440000exe4", "pero_EGF1_h_p0p0_p440000exe5", "pero_EGF1_h_p0p0_p440000exe6", "pero_EGF1_h_p0p0_p440000exe7", "pero_EGF1_h_p0p0_p440000exe8", "pero_EGF1_h_p0p0_p440000exe9", "pero_EGF1_h_p0p0_p480000exe0", "pero_EGF1_h_p0p0_p480000exe1", "pero_EGF1_h_p0p0_p480000exe10", "pero_EGF1_h_p0p0_p480000exe11", "pero_EGF1_h_p0p0_p480000exe12", "pero_EGF1_h_p0p0_p480000exe13", "pero_EGF1_h_p0p0_p480000exe14", "pero_EGF1_h_p0p0_p480000exe15", "pero_EGF1_h_p0p0_p480000exe16", "pero_EGF1_h_p0p0_p480000exe2", "pero_EGF1_h_p0p0_p480000exe3", "pero_EGF1_h_p0p0_p480000exe4", "pero_EGF1_h_p0p0_p480000exe5", "pero_EGF1_h_p0p0_p480000exe6", "pero_EGF1_h_p0p0_p480000exe7", "pero_EGF1_h_p0p0_p480000exe8", "pero_EGF1_h_p0p0_p480000exe9", "pero_EGF1_h_p0p0_p500000exe0", "pero_EGF1_h_p0p0_p500000exe1", "pero_EGF1_h_p0p0_p500000exe10", "pero_EGF1_h_p0p0_p500000exe11", "pero_EGF1_h_p0p0_p500000exe12", "pero_EGF1_h_p0p0_p500000exe13", "pero_EGF1_h_p0p0_p500000exe14", "pero_EGF1_h_p0p0_p500000exe15", "pero_EGF1_h_p0p0_p500000exe16", "pero_EGF1_h_p0p0_p500000exe2", "pero_EGF1_h_p0p0_p500000exe3", "pero_EGF1_h_p0p0_p500000exe4", "pero_EGF1_h_p0p0_p500000exe5", "pero_EGF1_h_p0p0_p500000exe6", "pero_EGF1_h_p0p0_p500000exe7", "pero_EGF1_h_p0p0_p500000exe8", "pero_EGF1_h_p0p0_p500000exe9", "pero_EGF1_h_p0p0_p50000exe0", "pero_EGF1_h_p0p0_p50000exe1", "pero_EGF1_h_p0p0_p50000exe10", "pero_EGF1_h_p0p0_p50000exe11", "pero_EGF1_h_p0p0_p50000exe12", "pero_EGF1_h_p0p0_p50000exe13", "pero_EGF1_h_p0p0_p50000exe14", "pero_EGF1_h_p0p0_p50000exe15", "pero_EGF1_h_p0p0_p50000exe16", "pero_EGF1_h_p0p0_p50000exe2", "pero_EGF1_h_p0p0_p50000exe3", "pero_EGF1_h_p0p0_p50000exe4", "pero_EGF1_h_p0p0_p50000exe5", "pero_EGF1_h_p0p0_p50000exe6", "pero_EGF1_h_p0p0_p50000exe7", "pero_EGF1_h_p0p0_p50000exe8", "pero_EGF1_h_p0p0_p50000exe9", "pero_EGF1_h_p0p0_p500exe0", "pero_EGF1_h_p0p0_p500exe1", "pero_EGF1_h_p0p0_p500exe10", "pero_EGF1_h_p0p0_p500exe11", "pero_EGF1_h_p0p0_p500exe12", "pero_EGF1_h_p0p0_p500exe13", "pero_EGF1_h_p0p0_p500exe14", "pero_EGF1_h_p0p0_p500exe15", "pero_EGF1_h_p0p0_p500exe16", "pero_EGF1_h_p0p0_p500exe2", "pero_EGF1_h_p0p0_p500exe3", "pero_EGF1_h_p0p0_p500exe4", "pero_EGF1_h_p0p0_p500exe5", "pero_EGF1_h_p0p0_p500exe6", "pero_EGF1_h_p0p0_p500exe7", "pero_EGF1_h_p0p0_p500exe8", "pero_EGF1_h_p0p0_p500exe9", "pero_EGF1_h_p0p0_p60000exe0", "pero_EGF1_h_p0p0_p60000exe1", "pero_EGF1_h_p0p0_p60000exe10", "pero_EGF1_h_p0p0_p60000exe11", "pero_EGF1_h_p0p0_p60000exe12", "pero_EGF1_h_p0p0_p60000exe13", "pero_EGF1_h_p0p0_p60000exe14", "pero_EGF1_h_p0p0_p60000exe15", "pero_EGF1_h_p0p0_p60000exe16", "pero_EGF1_h_p0p0_p60000exe2", "pero_EGF1_h_p0p0_p60000exe3", "pero_EGF1_h_p0p0_p60000exe4", "pero_EGF1_h_p0p0_p60000exe5", "pero_EGF1_h_p0p0_p60000exe6", "pero_EGF1_h_p0p0_p60000exe7", "pero_EGF1_h_p0p0_p60000exe8", "pero_EGF1_h_p0p0_p60000exe9", "pero_EGF1_h_p0p0_p6000exe0", "pero_EGF1_h_p0p0_p6000exe1", "pero_EGF1_h_p0p0_p6000exe10", "pero_EGF1_h_p0p0_p6000exe11", "pero_EGF1_h_p0p0_p6000exe12", "pero_EGF1_h_p0p0_p6000exe13", "pero_EGF1_h_p0p0_p6000exe14", "pero_EGF1_h_p0p0_p6000exe15", "pero_EGF1_h_p0p0_p6000exe16", "pero_EGF1_h_p0p0_p6000exe2", "pero_EGF1_h_p0p0_p6000exe3", "pero_EGF1_h_p0p0_p6000exe4", "pero_EGF1_h_p0p0_p6000exe5", "pero_EGF1_h_p0p0_p6000exe6", "pero_EGF1_h_p0p0_p6000exe7", "pero_EGF1_h_p0p0_p6000exe8", "pero_EGF1_h_p0p0_p6000exe9", "pero_EGF1_h_p0p0_p600exe0", "pero_EGF1_h_p0p0_p600exe1", "pero_EGF1_h_p0p0_p600exe10", "pero_EGF1_h_p0p0_p600exe11", "pero_EGF1_h_p0p0_p600exe12", "pero_EGF1_h_p0p0_p600exe13", "pero_EGF1_h_p0p0_p600exe14", "pero_EGF1_h_p0p0_p600exe15", "pero_EGF1_h_p0p0_p600exe16", "pero_EGF1_h_p0p0_p600exe17", "pero_EGF1_h_p0p0_p600exe2", "pero_EGF1_h_p0p0_p600exe3", "pero_EGF1_h_p0p0_p600exe4", "pero_EGF1_h_p0p0_p600exe5", "pero_EGF1_h_p0p0_p600exe6", "pero_EGF1_h_p0p0_p600exe7", "pero_EGF1_h_p0p0_p600exe8", "pero_EGF1_h_p0p0_p600exe9", "pero_EGF1_h_p0p0_p700exe0", "pero_EGF1_h_p0p0_p700exe1", "pero_EGF1_h_p0p0_p700exe10", "pero_EGF1_h_p0p0_p700exe11", "pero_EGF1_h_p0p0_p700exe12", "pero_EGF1_h_p0p0_p700exe13", "pero_EGF1_h_p0p0_p700exe14", "pero_EGF1_h_p0p0_p700exe15", "pero_EGF1_h_p0p0_p700exe16", "pero_EGF1_h_p0p0_p700exe2", "pero_EGF1_h_p0p0_p700exe3", "pero_EGF1_h_p0p0_p700exe4", "pero_EGF1_h_p0p0_p700exe5", "pero_EGF1_h_p0p0_p700exe6", "pero_EGF1_h_p0p0_p700exe7", "pero_EGF1_h_p0p0_p700exe8", "pero_EGF1_h_p0p0_p700exe9", "pero_EGF1_h_p0p0_p80000exe0", "pero_EGF1_h_p0p0_p80000exe1", "pero_EGF1_h_p0p0_p80000exe10", "pero_EGF1_h_p0p0_p80000exe11", "pero_EGF1_h_p0p0_p80000exe12", "pero_EGF1_h_p0p0_p80000exe13", "pero_EGF1_h_p0p0_p80000exe14", "pero_EGF1_h_p0p0_p80000exe15", "pero_EGF1_h_p0p0_p80000exe16", "pero_EGF1_h_p0p0_p80000exe2", "pero_EGF1_h_p0p0_p80000exe3", "pero_EGF1_h_p0p0_p80000exe4", "pero_EGF1_h_p0p0_p80000exe5", "pero_EGF1_h_p0p0_p80000exe6", "pero_EGF1_h_p0p0_p80000exe7", "pero_EGF1_h_p0p0_p80000exe8", "pero_EGF1_h_p0p0_p80000exe9", "pero_EGF1_h_p0p0_p800exe0", "pero_EGF1_h_p0p0_p800exe1", "pero_EGF1_h_p0p0_p800exe10", "pero_EGF1_h_p0p0_p800exe11", "pero_EGF1_h_p0p0_p800exe12", "pero_EGF1_h_p0p0_p800exe13", "pero_EGF1_h_p0p0_p800exe14", "pero_EGF1_h_p0p0_p800exe15", "pero_EGF1_h_p0p0_p800exe16", "pero_EGF1_h_p0p0_p800exe2", "pero_EGF1_h_p0p0_p800exe3", "pero_EGF1_h_p0p0_p800exe4", "pero_EGF1_h_p0p0_p800exe5", "pero_EGF1_h_p0p0_p800exe6", "pero_EGF1_h_p0p0_p800exe7", "pero_EGF1_h_p0p0_p800exe8", "pero_EGF1_h_p0p0_p800exe9", "pero_EGF1_h_p0p0_p900exe0", "pero_EGF1_h_p0p0_p900exe1", "pero_EGF1_h_p0p0_p900exe10", "pero_EGF1_h_p0p0_p900exe11", "pero_EGF1_h_p0p0_p900exe12", "pero_EGF1_h_p0p0_p900exe13", "pero_EGF1_h_p0p0_p900exe14", "pero_EGF1_h_p0p0_p900exe15", "pero_EGF1_h_p0p0_p900exe16", "pero_EGF1_h_p0p0_p900exe2", "pero_EGF1_h_p0p0_p900exe3", "pero_EGF1_h_p0p0_p900exe4", "pero_EGF1_h_p0p0_p900exe5", "pero_EGF1_h_p0p0_p900exe6", "pero_EGF1_h_p0p0_p900exe7", "pero_EGF1_h_p0p0_p900exe8", "pero_EGF1_h_p0p0_p900exe9", "pero_EGF1_h_p0p1_m0exe0", "pero_EGF1_h_p0p1_m0exe1", "pero_EGF1_h_p0p1_m0exe10", "pero_EGF1_h_p0p1_m0exe11", "pero_EGF1_h_p0p1_m0exe12", "pero_EGF1_h_p0p1_m0exe13", "pero_EGF1_h_p0p1_m0exe14", "pero_EGF1_h_p0p1_m0exe15", "pero_EGF1_h_p0p1_m0exe16", "pero_EGF1_h_p0p1_m0exe2", "pero_EGF1_h_p0p1_m0exe3", "pero_EGF1_h_p0p1_m0exe4", "pero_EGF1_h_p0p1_m0exe5", "pero_EGF1_h_p0p1_m0exe6", "pero_EGF1_h_p0p1_m0exe7", "pero_EGF1_h_p0p1_m0exe8", "pero_EGF1_h_p0p1_m0exe9", "pero_EGF1_h_p0p1_m100exe0", "pero_EGF1_h_p0p1_m100exe1", "pero_EGF1_h_p0p1_m100exe10", "pero_EGF1_h_p0p1_m100exe11", "pero_EGF1_h_p0p1_m100exe12", "pero_EGF1_h_p0p1_m100exe13", "pero_EGF1_h_p0p1_m100exe14", "pero_EGF1_h_p0p1_m100exe15", "pero_EGF1_h_p0p1_m100exe16", "pero_EGF1_h_p0p1_m100exe2", "pero_EGF1_h_p0p1_m100exe3", "pero_EGF1_h_p0p1_m100exe4", "pero_EGF1_h_p0p1_m100exe5", "pero_EGF1_h_p0p1_m100exe6", "pero_EGF1_h_p0p1_m100exe7", "pero_EGF1_h_p0p1_m100exe8", "pero_EGF1_h_p0p1_m100exe9", "pero_EGF1_h_p0p1_m200exe0", "pero_EGF1_h_p0p1_m200exe1", "pero_EGF1_h_p0p1_m200exe10", "pero_EGF1_h_p0p1_m200exe11", "pero_EGF1_h_p0p1_m200exe12", "pero_EGF1_h_p0p1_m200exe13", "pero_EGF1_h_p0p1_m200exe14", "pero_EGF1_h_p0p1_m200exe15", "pero_EGF1_h_p0p1_m200exe16", "pero_EGF1_h_p0p1_m200exe2", "pero_EGF1_h_p0p1_m200exe3", "pero_EGF1_h_p0p1_m200exe4", "pero_EGF1_h_p0p1_m200exe5", "pero_EGF1_h_p0p1_m200exe6", "pero_EGF1_h_p0p1_m200exe7", "pero_EGF1_h_p0p1_m200exe8", "pero_EGF1_h_p0p1_m200exe9", "pero_EGF1_h_p0p1_m300exe0", "pero_EGF1_h_p0p1_m300exe1", "pero_EGF1_h_p0p1_m300exe10", "pero_EGF1_h_p0p1_m300exe11", "pero_EGF1_h_p0p1_m300exe12", "pero_EGF1_h_p0p1_m300exe13", "pero_EGF1_h_p0p1_m300exe14", "pero_EGF1_h_p0p1_m300exe15", "pero_EGF1_h_p0p1_m300exe16", "pero_EGF1_h_p0p1_m300exe2", "pero_EGF1_h_p0p1_m300exe3", "pero_EGF1_h_p0p1_m300exe4", "pero_EGF1_h_p0p1_m300exe5", "pero_EGF1_h_p0p1_m300exe6", "pero_EGF1_h_p0p1_m300exe7", "pero_EGF1_h_p0p1_m300exe8", "pero_EGF1_h_p0p1_m300exe9", "pero_EGF1_h_p0p1_m5000exe0", "pero_EGF1_h_p0p1_m5000exe1", "pero_EGF1_h_p0p1_m5000exe10", "pero_EGF1_h_p0p1_m5000exe11", "pero_EGF1_h_p0p1_m5000exe12", "pero_EGF1_h_p0p1_m5000exe13", "pero_EGF1_h_p0p1_m5000exe14", "pero_EGF1_h_p0p1_m5000exe15", "pero_EGF1_h_p0p1_m5000exe16", "pero_EGF1_h_p0p1_m5000exe2", "pero_EGF1_h_p0p1_m5000exe3", "pero_EGF1_h_p0p1_m5000exe4", "pero_EGF1_h_p0p1_m5000exe5", "pero_EGF1_h_p0p1_m5000exe6", "pero_EGF1_h_p0p1_m5000exe7", "pero_EGF1_h_p0p1_m5000exe8", "pero_EGF1_h_p0p1_m5000exe9", "pero_EGF1_h_p0p1_m500exe0", "pero_EGF1_h_p0p1_m500exe1", "pero_EGF1_h_p0p1_m500exe10", "pero_EGF1_h_p0p1_m500exe11", "pero_EGF1_h_p0p1_m500exe12", "pero_EGF1_h_p0p1_m500exe13", "pero_EGF1_h_p0p1_m500exe14", "pero_EGF1_h_p0p1_m500exe15", "pero_EGF1_h_p0p1_m500exe16", "pero_EGF1_h_p0p1_m500exe2", "pero_EGF1_h_p0p1_m500exe3", "pero_EGF1_h_p0p1_m500exe4", "pero_EGF1_h_p0p1_m500exe5", "pero_EGF1_h_p0p1_m500exe6", "pero_EGF1_h_p0p1_m500exe7", "pero_EGF1_h_p0p1_m500exe8", "pero_EGF1_h_p0p1_m500exe9", "pero_EGF1_h_p0p1_p100000exe0", "pero_EGF1_h_p0p1_p100000exe1", "pero_EGF1_h_p0p1_p100000exe10", "pero_EGF1_h_p0p1_p100000exe11", "pero_EGF1_h_p0p1_p100000exe12", "pero_EGF1_h_p0p1_p100000exe13", "pero_EGF1_h_p0p1_p100000exe14", "pero_EGF1_h_p0p1_p100000exe15", "pero_EGF1_h_p0p1_p100000exe16", "pero_EGF1_h_p0p1_p100000exe2", "pero_EGF1_h_p0p1_p100000exe3", "pero_EGF1_h_p0p1_p100000exe4", "pero_EGF1_h_p0p1_p100000exe5", "pero_EGF1_h_p0p1_p100000exe6", "pero_EGF1_h_p0p1_p100000exe7", "pero_EGF1_h_p0p1_p100000exe8", "pero_EGF1_h_p0p1_p100000exe9", "pero_EGF1_h_p0p1_p10000exe0", "pero_EGF1_h_p0p1_p10000exe1", "pero_EGF1_h_p0p1_p10000exe10", "pero_EGF1_h_p0p1_p10000exe11", "pero_EGF1_h_p0p1_p10000exe12", "pero_EGF1_h_p0p1_p10000exe13", "pero_EGF1_h_p0p1_p10000exe14", "pero_EGF1_h_p0p1_p10000exe15", "pero_EGF1_h_p0p1_p10000exe16", "pero_EGF1_h_p0p1_p10000exe2", "pero_EGF1_h_p0p1_p10000exe3", "pero_EGF1_h_p0p1_p10000exe4", "pero_EGF1_h_p0p1_p10000exe5", "pero_EGF1_h_p0p1_p10000exe6", "pero_EGF1_h_p0p1_p10000exe7", "pero_EGF1_h_p0p1_p10000exe8", "pero_EGF1_h_p0p1_p10000exe9", "pero_EGF1_h_p0p1_p1000exe0", "pero_EGF1_h_p0p1_p1000exe1", "pero_EGF1_h_p0p1_p1000exe10", "pero_EGF1_h_p0p1_p1000exe11", "pero_EGF1_h_p0p1_p1000exe12", "pero_EGF1_h_p0p1_p1000exe13", "pero_EGF1_h_p0p1_p1000exe14", "pero_EGF1_h_p0p1_p1000exe15", "pero_EGF1_h_p0p1_p1000exe16", "pero_EGF1_h_p0p1_p1000exe17", "pero_EGF1_h_p0p1_p1000exe2", "pero_EGF1_h_p0p1_p1000exe3", "pero_EGF1_h_p0p1_p1000exe4", "pero_EGF1_h_p0p1_p1000exe5", "pero_EGF1_h_p0p1_p1000exe6", "pero_EGF1_h_p0p1_p1000exe7", "pero_EGF1_h_p0p1_p1000exe8", "pero_EGF1_h_p0p1_p1000exe9", "pero_EGF1_h_p0p1_p100exe0", "pero_EGF1_h_p0p1_p100exe1", "pero_EGF1_h_p0p1_p100exe10", "pero_EGF1_h_p0p1_p100exe11", "pero_EGF1_h_p0p1_p100exe12", "pero_EGF1_h_p0p1_p100exe13", "pero_EGF1_h_p0p1_p100exe14", "pero_EGF1_h_p0p1_p100exe15", "pero_EGF1_h_p0p1_p100exe16", "pero_EGF1_h_p0p1_p100exe2", "pero_EGF1_h_p0p1_p100exe3", "pero_EGF1_h_p0p1_p100exe4", "pero_EGF1_h_p0p1_p100exe5", "pero_EGF1_h_p0p1_p100exe6", "pero_EGF1_h_p0p1_p100exe7", "pero_EGF1_h_p0p1_p100exe8", "pero_EGF1_h_p0p1_p100exe9", "pero_EGF1_h_p0p1_p1100exe0", "pero_EGF1_h_p0p1_p1100exe1", "pero_EGF1_h_p0p1_p1100exe10", "pero_EGF1_h_p0p1_p1100exe11", "pero_EGF1_h_p0p1_p1100exe12", "pero_EGF1_h_p0p1_p1100exe13", "pero_EGF1_h_p0p1_p1100exe14", "pero_EGF1_h_p0p1_p1100exe15", "pero_EGF1_h_p0p1_p1100exe16", "pero_EGF1_h_p0p1_p1100exe2", "pero_EGF1_h_p0p1_p1100exe3", "pero_EGF1_h_p0p1_p1100exe4", "pero_EGF1_h_p0p1_p1100exe5", "pero_EGF1_h_p0p1_p1100exe6", "pero_EGF1_h_p0p1_p1100exe7", "pero_EGF1_h_p0p1_p1100exe8", "pero_EGF1_h_p0p1_p1100exe9", "pero_EGF1_h_p0p1_p120000exe0", "pero_EGF1_h_p0p1_p120000exe1", "pero_EGF1_h_p0p1_p120000exe10", "pero_EGF1_h_p0p1_p120000exe11", "pero_EGF1_h_p0p1_p120000exe12", "pero_EGF1_h_p0p1_p120000exe13", "pero_EGF1_h_p0p1_p120000exe14", "pero_EGF1_h_p0p1_p120000exe15", "pero_EGF1_h_p0p1_p120000exe16", "pero_EGF1_h_p0p1_p120000exe2", "pero_EGF1_h_p0p1_p120000exe3", "pero_EGF1_h_p0p1_p120000exe4", "pero_EGF1_h_p0p1_p120000exe5", "pero_EGF1_h_p0p1_p120000exe6", "pero_EGF1_h_p0p1_p120000exe7", "pero_EGF1_h_p0p1_p120000exe8", "pero_EGF1_h_p0p1_p120000exe9", "pero_EGF1_h_p0p1_p1200exe0", "pero_EGF1_h_p0p1_p1200exe1", "pero_EGF1_h_p0p1_p1200exe10", "pero_EGF1_h_p0p1_p1200exe11", "pero_EGF1_h_p0p1_p1200exe12", "pero_EGF1_h_p0p1_p1200exe13", "pero_EGF1_h_p0p1_p1200exe14", "pero_EGF1_h_p0p1_p1200exe15", "pero_EGF1_h_p0p1_p1200exe16", "pero_EGF1_h_p0p1_p1200exe2", "pero_EGF1_h_p0p1_p1200exe3", "pero_EGF1_h_p0p1_p1200exe4", "pero_EGF1_h_p0p1_p1200exe5", "pero_EGF1_h_p0p1_p1200exe6", "pero_EGF1_h_p0p1_p1200exe7", "pero_EGF1_h_p0p1_p1200exe8", "pero_EGF1_h_p0p1_p1200exe9", "pero_EGF1_h_p0p1_p1300exe0", "pero_EGF1_h_p0p1_p1300exe1", "pero_EGF1_h_p0p1_p1300exe10", "pero_EGF1_h_p0p1_p1300exe11", "pero_EGF1_h_p0p1_p1300exe12", "pero_EGF1_h_p0p1_p1300exe13", "pero_EGF1_h_p0p1_p1300exe14", "pero_EGF1_h_p0p1_p1300exe15", "pero_EGF1_h_p0p1_p1300exe16", "pero_EGF1_h_p0p1_p1300exe2", "pero_EGF1_h_p0p1_p1300exe3", "pero_EGF1_h_p0p1_p1300exe4", "pero_EGF1_h_p0p1_p1300exe5", "pero_EGF1_h_p0p1_p1300exe6", "pero_EGF1_h_p0p1_p1300exe7", "pero_EGF1_h_p0p1_p1300exe8", "pero_EGF1_h_p0p1_p1300exe9", "pero_EGF1_h_p0p1_p140000exe0", "pero_EGF1_h_p0p1_p140000exe1", "pero_EGF1_h_p0p1_p140000exe10", "pero_EGF1_h_p0p1_p140000exe11", "pero_EGF1_h_p0p1_p140000exe12", "pero_EGF1_h_p0p1_p140000exe13", "pero_EGF1_h_p0p1_p140000exe14", "pero_EGF1_h_p0p1_p140000exe15", "pero_EGF1_h_p0p1_p140000exe16", "pero_EGF1_h_p0p1_p140000exe2", "pero_EGF1_h_p0p1_p140000exe3", "pero_EGF1_h_p0p1_p140000exe4", "pero_EGF1_h_p0p1_p140000exe5", "pero_EGF1_h_p0p1_p140000exe6", "pero_EGF1_h_p0p1_p140000exe7", "pero_EGF1_h_p0p1_p140000exe8", "pero_EGF1_h_p0p1_p140000exe9", "pero_EGF1_h_p0p1_p1400exe0", "pero_EGF1_h_p0p1_p1400exe1", "pero_EGF1_h_p0p1_p1400exe10", "pero_EGF1_h_p0p1_p1400exe11", "pero_EGF1_h_p0p1_p1400exe12", "pero_EGF1_h_p0p1_p1400exe13", "pero_EGF1_h_p0p1_p1400exe14", "pero_EGF1_h_p0p1_p1400exe15", "pero_EGF1_h_p0p1_p1400exe16", "pero_EGF1_h_p0p1_p1400exe2", "pero_EGF1_h_p0p1_p1400exe3", "pero_EGF1_h_p0p1_p1400exe4", "pero_EGF1_h_p0p1_p1400exe5", "pero_EGF1_h_p0p1_p1400exe6", "pero_EGF1_h_p0p1_p1400exe7", "pero_EGF1_h_p0p1_p1400exe8", "pero_EGF1_h_p0p1_p1400exe9", "pero_EGF1_h_p0p1_p1500exe0", "pero_EGF1_h_p0p1_p1500exe1", "pero_EGF1_h_p0p1_p1500exe10", "pero_EGF1_h_p0p1_p1500exe11", "pero_EGF1_h_p0p1_p1500exe12", "pero_EGF1_h_p0p1_p1500exe13", "pero_EGF1_h_p0p1_p1500exe14", "pero_EGF1_h_p0p1_p1500exe15", "pero_EGF1_h_p0p1_p1500exe16", "pero_EGF1_h_p0p1_p1500exe2", "pero_EGF1_h_p0p1_p1500exe3", "pero_EGF1_h_p0p1_p1500exe4", "pero_EGF1_h_p0p1_p1500exe5", "pero_EGF1_h_p0p1_p1500exe6", "pero_EGF1_h_p0p1_p1500exe7", "pero_EGF1_h_p0p1_p1500exe8", "pero_EGF1_h_p0p1_p1500exe9", "pero_EGF1_h_p0p1_p160000exe0", "pero_EGF1_h_p0p1_p160000exe1", "pero_EGF1_h_p0p1_p160000exe10", "pero_EGF1_h_p0p1_p160000exe11", "pero_EGF1_h_p0p1_p160000exe12", "pero_EGF1_h_p0p1_p160000exe13", "pero_EGF1_h_p0p1_p160000exe14", "pero_EGF1_h_p0p1_p160000exe15", "pero_EGF1_h_p0p1_p160000exe16", "pero_EGF1_h_p0p1_p160000exe2", "pero_EGF1_h_p0p1_p160000exe3", "pero_EGF1_h_p0p1_p160000exe4", "pero_EGF1_h_p0p1_p160000exe5", "pero_EGF1_h_p0p1_p160000exe6", "pero_EGF1_h_p0p1_p160000exe7", "pero_EGF1_h_p0p1_p160000exe8", "pero_EGF1_h_p0p1_p160000exe9", "pero_EGF1_h_p0p1_p1600exe0", "pero_EGF1_h_p0p1_p1600exe1", "pero_EGF1_h_p0p1_p1600exe10", "pero_EGF1_h_p0p1_p1600exe11", "pero_EGF1_h_p0p1_p1600exe12", "pero_EGF1_h_p0p1_p1600exe13", "pero_EGF1_h_p0p1_p1600exe14", "pero_EGF1_h_p0p1_p1600exe15", "pero_EGF1_h_p0p1_p1600exe16", "pero_EGF1_h_p0p1_p1600exe2", "pero_EGF1_h_p0p1_p1600exe3", "pero_EGF1_h_p0p1_p1600exe4", "pero_EGF1_h_p0p1_p1600exe5", "pero_EGF1_h_p0p1_p1600exe6", "pero_EGF1_h_p0p1_p1600exe7", "pero_EGF1_h_p0p1_p1600exe8", "pero_EGF1_h_p0p1_p1600exe9", "pero_EGF1_h_p0p1_p1700exe0", "pero_EGF1_h_p0p1_p1700exe1", "pero_EGF1_h_p0p1_p1700exe10", "pero_EGF1_h_p0p1_p1700exe11", "pero_EGF1_h_p0p1_p1700exe12", "pero_EGF1_h_p0p1_p1700exe13", "pero_EGF1_h_p0p1_p1700exe14", "pero_EGF1_h_p0p1_p1700exe15", "pero_EGF1_h_p0p1_p1700exe16", "pero_EGF1_h_p0p1_p1700exe2", "pero_EGF1_h_p0p1_p1700exe3", "pero_EGF1_h_p0p1_p1700exe4", "pero_EGF1_h_p0p1_p1700exe5", "pero_EGF1_h_p0p1_p1700exe6", "pero_EGF1_h_p0p1_p1700exe7", "pero_EGF1_h_p0p1_p1700exe8", "pero_EGF1_h_p0p1_p1700exe9", "pero_EGF1_h_p0p1_p180000exe0", "pero_EGF1_h_p0p1_p180000exe1", "pero_EGF1_h_p0p1_p180000exe10", "pero_EGF1_h_p0p1_p180000exe11", "pero_EGF1_h_p0p1_p180000exe12", "pero_EGF1_h_p0p1_p180000exe13", "pero_EGF1_h_p0p1_p180000exe14", "pero_EGF1_h_p0p1_p180000exe15", "pero_EGF1_h_p0p1_p180000exe16", "pero_EGF1_h_p0p1_p180000exe2", "pero_EGF1_h_p0p1_p180000exe3", "pero_EGF1_h_p0p1_p180000exe4", "pero_EGF1_h_p0p1_p180000exe5", "pero_EGF1_h_p0p1_p180000exe6", "pero_EGF1_h_p0p1_p180000exe7", "pero_EGF1_h_p0p1_p180000exe8", "pero_EGF1_h_p0p1_p180000exe9", "pero_EGF1_h_p0p1_p1800exe0", "pero_EGF1_h_p0p1_p1800exe1", "pero_EGF1_h_p0p1_p1800exe10", "pero_EGF1_h_p0p1_p1800exe11", "pero_EGF1_h_p0p1_p1800exe12", "pero_EGF1_h_p0p1_p1800exe13", "pero_EGF1_h_p0p1_p1800exe14", "pero_EGF1_h_p0p1_p1800exe15", "pero_EGF1_h_p0p1_p1800exe16", "pero_EGF1_h_p0p1_p1800exe2", "pero_EGF1_h_p0p1_p1800exe3", "pero_EGF1_h_p0p1_p1800exe4", "pero_EGF1_h_p0p1_p1800exe5", "pero_EGF1_h_p0p1_p1800exe6", "pero_EGF1_h_p0p1_p1800exe7", "pero_EGF1_h_p0p1_p1800exe8", "pero_EGF1_h_p0p1_p1800exe9", "pero_EGF1_h_p0p1_p1900exe0", "pero_EGF1_h_p0p1_p1900exe1", "pero_EGF1_h_p0p1_p1900exe10", "pero_EGF1_h_p0p1_p1900exe11", "pero_EGF1_h_p0p1_p1900exe12", "pero_EGF1_h_p0p1_p1900exe13", "pero_EGF1_h_p0p1_p1900exe14", "pero_EGF1_h_p0p1_p1900exe15", "pero_EGF1_h_p0p1_p1900exe16", "pero_EGF1_h_p0p1_p1900exe17", "pero_EGF1_h_p0p1_p1900exe2", "pero_EGF1_h_p0p1_p1900exe3", "pero_EGF1_h_p0p1_p1900exe4", "pero_EGF1_h_p0p1_p1900exe5", "pero_EGF1_h_p0p1_p1900exe6", "pero_EGF1_h_p0p1_p1900exe7", "pero_EGF1_h_p0p1_p1900exe8", "pero_EGF1_h_p0p1_p1900exe9", "pero_EGF1_h_p0p1_p200000exe0", "pero_EGF1_h_p0p1_p200000exe1", "pero_EGF1_h_p0p1_p200000exe10", "pero_EGF1_h_p0p1_p200000exe11", "pero_EGF1_h_p0p1_p200000exe12", "pero_EGF1_h_p0p1_p200000exe13", "pero_EGF1_h_p0p1_p200000exe14", "pero_EGF1_h_p0p1_p200000exe15", "pero_EGF1_h_p0p1_p200000exe16", "pero_EGF1_h_p0p1_p200000exe2", "pero_EGF1_h_p0p1_p200000exe3", "pero_EGF1_h_p0p1_p200000exe4", "pero_EGF1_h_p0p1_p200000exe5", "pero_EGF1_h_p0p1_p200000exe6", "pero_EGF1_h_p0p1_p200000exe7", "pero_EGF1_h_p0p1_p200000exe8", "pero_EGF1_h_p0p1_p200000exe9", "pero_EGF1_h_p0p1_p20000exe0", "pero_EGF1_h_p0p1_p20000exe1", "pero_EGF1_h_p0p1_p20000exe10", "pero_EGF1_h_p0p1_p20000exe11", "pero_EGF1_h_p0p1_p20000exe12", "pero_EGF1_h_p0p1_p20000exe13", "pero_EGF1_h_p0p1_p20000exe14", "pero_EGF1_h_p0p1_p20000exe15", "pero_EGF1_h_p0p1_p20000exe16", "pero_EGF1_h_p0p1_p20000exe2", "pero_EGF1_h_p0p1_p20000exe3", "pero_EGF1_h_p0p1_p20000exe4", "pero_EGF1_h_p0p1_p20000exe5", "pero_EGF1_h_p0p1_p20000exe6", "pero_EGF1_h_p0p1_p20000exe7", "pero_EGF1_h_p0p1_p20000exe8", "pero_EGF1_h_p0p1_p20000exe9", "pero_EGF1_h_p0p1_p2000exe0", "pero_EGF1_h_p0p1_p2000exe1", "pero_EGF1_h_p0p1_p2000exe10", "pero_EGF1_h_p0p1_p2000exe11", "pero_EGF1_h_p0p1_p2000exe12", "pero_EGF1_h_p0p1_p2000exe13", "pero_EGF1_h_p0p1_p2000exe14", "pero_EGF1_h_p0p1_p2000exe15", "pero_EGF1_h_p0p1_p2000exe16", "pero_EGF1_h_p0p1_p2000exe2", "pero_EGF1_h_p0p1_p2000exe3", "pero_EGF1_h_p0p1_p2000exe4", "pero_EGF1_h_p0p1_p2000exe5", "pero_EGF1_h_p0p1_p2000exe6", "pero_EGF1_h_p0p1_p2000exe7", "pero_EGF1_h_p0p1_p2000exe8", "pero_EGF1_h_p0p1_p2000exe9", "pero_EGF1_h_p0p1_p200exe0", "pero_EGF1_h_p0p1_p200exe1", "pero_EGF1_h_p0p1_p200exe10", "pero_EGF1_h_p0p1_p200exe11", "pero_EGF1_h_p0p1_p200exe12", "pero_EGF1_h_p0p1_p200exe13", "pero_EGF1_h_p0p1_p200exe14", "pero_EGF1_h_p0p1_p200exe15", "pero_EGF1_h_p0p1_p200exe16", "pero_EGF1_h_p0p1_p200exe2", "pero_EGF1_h_p0p1_p200exe3", "pero_EGF1_h_p0p1_p200exe4", "pero_EGF1_h_p0p1_p200exe5", "pero_EGF1_h_p0p1_p200exe6", "pero_EGF1_h_p0p1_p200exe7", "pero_EGF1_h_p0p1_p200exe8", "pero_EGF1_h_p0p1_p200exe9", "pero_EGF1_h_p0p1_p2100exe0", "pero_EGF1_h_p0p1_p2100exe1", "pero_EGF1_h_p0p1_p2100exe10", "pero_EGF1_h_p0p1_p2100exe11", "pero_EGF1_h_p0p1_p2100exe12", "pero_EGF1_h_p0p1_p2100exe13", "pero_EGF1_h_p0p1_p2100exe14", "pero_EGF1_h_p0p1_p2100exe15", "pero_EGF1_h_p0p1_p2100exe16", "pero_EGF1_h_p0p1_p2100exe2", "pero_EGF1_h_p0p1_p2100exe3", "pero_EGF1_h_p0p1_p2100exe4", "pero_EGF1_h_p0p1_p2100exe5", "pero_EGF1_h_p0p1_p2100exe6", "pero_EGF1_h_p0p1_p2100exe7", "pero_EGF1_h_p0p1_p2100exe8", "pero_EGF1_h_p0p1_p2100exe9", "pero_EGF1_h_p0p1_p220000exe0", "pero_EGF1_h_p0p1_p220000exe1", "pero_EGF1_h_p0p1_p220000exe10", "pero_EGF1_h_p0p1_p220000exe11", "pero_EGF1_h_p0p1_p220000exe12", "pero_EGF1_h_p0p1_p220000exe13", "pero_EGF1_h_p0p1_p220000exe14", "pero_EGF1_h_p0p1_p220000exe15", "pero_EGF1_h_p0p1_p220000exe16", "pero_EGF1_h_p0p1_p220000exe2", "pero_EGF1_h_p0p1_p220000exe3", "pero_EGF1_h_p0p1_p220000exe4", "pero_EGF1_h_p0p1_p220000exe5", "pero_EGF1_h_p0p1_p220000exe6", "pero_EGF1_h_p0p1_p220000exe7", "pero_EGF1_h_p0p1_p220000exe8", "pero_EGF1_h_p0p1_p220000exe9", "pero_EGF1_h_p0p1_p2200exe0", "pero_EGF1_h_p0p1_p2200exe1", "pero_EGF1_h_p0p1_p2200exe10", "pero_EGF1_h_p0p1_p2200exe11", "pero_EGF1_h_p0p1_p2200exe12", "pero_EGF1_h_p0p1_p2200exe13", "pero_EGF1_h_p0p1_p2200exe14", "pero_EGF1_h_p0p1_p2200exe15", "pero_EGF1_h_p0p1_p2200exe16", "pero_EGF1_h_p0p1_p2200exe2", "pero_EGF1_h_p0p1_p2200exe3", "pero_EGF1_h_p0p1_p2200exe4", "pero_EGF1_h_p0p1_p2200exe5", "pero_EGF1_h_p0p1_p2200exe6", "pero_EGF1_h_p0p1_p2200exe7", "pero_EGF1_h_p0p1_p2200exe8", "pero_EGF1_h_p0p1_p2200exe9", "pero_EGF1_h_p0p1_p2300exe0", "pero_EGF1_h_p0p1_p2300exe1", "pero_EGF1_h_p0p1_p2300exe10", "pero_EGF1_h_p0p1_p2300exe11", "pero_EGF1_h_p0p1_p2300exe12", "pero_EGF1_h_p0p1_p2300exe13", "pero_EGF1_h_p0p1_p2300exe14", "pero_EGF1_h_p0p1_p2300exe15", "pero_EGF1_h_p0p1_p2300exe16", "pero_EGF1_h_p0p1_p2300exe17", "pero_EGF1_h_p0p1_p2300exe2", "pero_EGF1_h_p0p1_p2300exe3", "pero_EGF1_h_p0p1_p2300exe4", "pero_EGF1_h_p0p1_p2300exe5", "pero_EGF1_h_p0p1_p2300exe6", "pero_EGF1_h_p0p1_p2300exe7", "pero_EGF1_h_p0p1_p2300exe8", "pero_EGF1_h_p0p1_p2300exe9", "pero_EGF1_h_p0p1_p240000exe0", "pero_EGF1_h_p0p1_p240000exe1", "pero_EGF1_h_p0p1_p240000exe10", "pero_EGF1_h_p0p1_p240000exe11", "pero_EGF1_h_p0p1_p240000exe12", "pero_EGF1_h_p0p1_p240000exe13", "pero_EGF1_h_p0p1_p240000exe14", "pero_EGF1_h_p0p1_p240000exe15", "pero_EGF1_h_p0p1_p240000exe16", "pero_EGF1_h_p0p1_p240000exe2", "pero_EGF1_h_p0p1_p240000exe3", "pero_EGF1_h_p0p1_p240000exe4", "pero_EGF1_h_p0p1_p240000exe5", "pero_EGF1_h_p0p1_p240000exe6", "pero_EGF1_h_p0p1_p240000exe7", "pero_EGF1_h_p0p1_p240000exe8", "pero_EGF1_h_p0p1_p240000exe9", "pero_EGF1_h_p0p1_p2400exe0", "pero_EGF1_h_p0p1_p2400exe1", "pero_EGF1_h_p0p1_p2400exe10", "pero_EGF1_h_p0p1_p2400exe11", "pero_EGF1_h_p0p1_p2400exe12", "pero_EGF1_h_p0p1_p2400exe13", "pero_EGF1_h_p0p1_p2400exe14", "pero_EGF1_h_p0p1_p2400exe15", "pero_EGF1_h_p0p1_p2400exe16", "pero_EGF1_h_p0p1_p2400exe2", "pero_EGF1_h_p0p1_p2400exe3", "pero_EGF1_h_p0p1_p2400exe4", "pero_EGF1_h_p0p1_p2400exe5", "pero_EGF1_h_p0p1_p2400exe6", "pero_EGF1_h_p0p1_p2400exe7", "pero_EGF1_h_p0p1_p2400exe8", "pero_EGF1_h_p0p1_p2400exe9", "pero_EGF1_h_p0p1_p2500exe0", "pero_EGF1_h_p0p1_p2500exe1", "pero_EGF1_h_p0p1_p2500exe10", "pero_EGF1_h_p0p1_p2500exe11", "pero_EGF1_h_p0p1_p2500exe12", "pero_EGF1_h_p0p1_p2500exe13", "pero_EGF1_h_p0p1_p2500exe14", "pero_EGF1_h_p0p1_p2500exe15", "pero_EGF1_h_p0p1_p2500exe16", "pero_EGF1_h_p0p1_p2500exe2", "pero_EGF1_h_p0p1_p2500exe3", "pero_EGF1_h_p0p1_p2500exe4", "pero_EGF1_h_p0p1_p2500exe5", "pero_EGF1_h_p0p1_p2500exe6", "pero_EGF1_h_p0p1_p2500exe7", "pero_EGF1_h_p0p1_p2500exe8", "pero_EGF1_h_p0p1_p2500exe9", "pero_EGF1_h_p0p1_p260000exe0", "pero_EGF1_h_p0p1_p260000exe1", "pero_EGF1_h_p0p1_p260000exe10", "pero_EGF1_h_p0p1_p260000exe11", "pero_EGF1_h_p0p1_p260000exe12", "pero_EGF1_h_p0p1_p260000exe13", "pero_EGF1_h_p0p1_p260000exe14", "pero_EGF1_h_p0p1_p260000exe15", "pero_EGF1_h_p0p1_p260000exe16", "pero_EGF1_h_p0p1_p260000exe2", "pero_EGF1_h_p0p1_p260000exe3", "pero_EGF1_h_p0p1_p260000exe4", "pero_EGF1_h_p0p1_p260000exe5", "pero_EGF1_h_p0p1_p260000exe6", "pero_EGF1_h_p0p1_p260000exe7", "pero_EGF1_h_p0p1_p260000exe8", "pero_EGF1_h_p0p1_p260000exe9", "pero_EGF1_h_p0p1_p2600exe0", "pero_EGF1_h_p0p1_p2600exe1", "pero_EGF1_h_p0p1_p2600exe10", "pero_EGF1_h_p0p1_p2600exe11", "pero_EGF1_h_p0p1_p2600exe12", "pero_EGF1_h_p0p1_p2600exe13", "pero_EGF1_h_p0p1_p2600exe14", "pero_EGF1_h_p0p1_p2600exe15", "pero_EGF1_h_p0p1_p2600exe16", "pero_EGF1_h_p0p1_p2600exe2", "pero_EGF1_h_p0p1_p2600exe3", "pero_EGF1_h_p0p1_p2600exe4", "pero_EGF1_h_p0p1_p2600exe5", "pero_EGF1_h_p0p1_p2600exe6", "pero_EGF1_h_p0p1_p2600exe7", "pero_EGF1_h_p0p1_p2600exe8", "pero_EGF1_h_p0p1_p2600exe9", "pero_EGF1_h_p0p1_p2700exe0", "pero_EGF1_h_p0p1_p2700exe1", "pero_EGF1_h_p0p1_p2700exe10", "pero_EGF1_h_p0p1_p2700exe11", "pero_EGF1_h_p0p1_p2700exe12", "pero_EGF1_h_p0p1_p2700exe13", "pero_EGF1_h_p0p1_p2700exe14", "pero_EGF1_h_p0p1_p2700exe15", "pero_EGF1_h_p0p1_p2700exe16", "pero_EGF1_h_p0p1_p2700exe2", "pero_EGF1_h_p0p1_p2700exe3", "pero_EGF1_h_p0p1_p2700exe4", "pero_EGF1_h_p0p1_p2700exe5", "pero_EGF1_h_p0p1_p2700exe6", "pero_EGF1_h_p0p1_p2700exe7", "pero_EGF1_h_p0p1_p2700exe8", "pero_EGF1_h_p0p1_p2700exe9", "pero_EGF1_h_p0p1_p280000exe0", "pero_EGF1_h_p0p1_p280000exe1", "pero_EGF1_h_p0p1_p280000exe10", "pero_EGF1_h_p0p1_p280000exe11", "pero_EGF1_h_p0p1_p280000exe12", "pero_EGF1_h_p0p1_p280000exe13", "pero_EGF1_h_p0p1_p280000exe14", "pero_EGF1_h_p0p1_p280000exe15", "pero_EGF1_h_p0p1_p280000exe16", "pero_EGF1_h_p0p1_p280000exe2", "pero_EGF1_h_p0p1_p280000exe3", "pero_EGF1_h_p0p1_p280000exe4", "pero_EGF1_h_p0p1_p280000exe5", "pero_EGF1_h_p0p1_p280000exe6", "pero_EGF1_h_p0p1_p280000exe7", "pero_EGF1_h_p0p1_p280000exe8", "pero_EGF1_h_p0p1_p280000exe9", "pero_EGF1_h_p0p1_p2800exe0", "pero_EGF1_h_p0p1_p2800exe1", "pero_EGF1_h_p0p1_p2800exe10", "pero_EGF1_h_p0p1_p2800exe11", "pero_EGF1_h_p0p1_p2800exe12", "pero_EGF1_h_p0p1_p2800exe13", "pero_EGF1_h_p0p1_p2800exe14", "pero_EGF1_h_p0p1_p2800exe15", "pero_EGF1_h_p0p1_p2800exe16", "pero_EGF1_h_p0p1_p2800exe2", "pero_EGF1_h_p0p1_p2800exe3", "pero_EGF1_h_p0p1_p2800exe4", "pero_EGF1_h_p0p1_p2800exe5", "pero_EGF1_h_p0p1_p2800exe6", "pero_EGF1_h_p0p1_p2800exe7", "pero_EGF1_h_p0p1_p2800exe8", "pero_EGF1_h_p0p1_p2800exe9", "pero_EGF1_h_p0p1_p2900exe0", "pero_EGF1_h_p0p1_p2900exe1", "pero_EGF1_h_p0p1_p2900exe10", "pero_EGF1_h_p0p1_p2900exe11", "pero_EGF1_h_p0p1_p2900exe12", "pero_EGF1_h_p0p1_p2900exe13", "pero_EGF1_h_p0p1_p2900exe14", "pero_EGF1_h_p0p1_p2900exe15", "pero_EGF1_h_p0p1_p2900exe16", "pero_EGF1_h_p0p1_p2900exe2", "pero_EGF1_h_p0p1_p2900exe3", "pero_EGF1_h_p0p1_p2900exe4", "pero_EGF1_h_p0p1_p2900exe5", "pero_EGF1_h_p0p1_p2900exe6", "pero_EGF1_h_p0p1_p2900exe7", "pero_EGF1_h_p0p1_p2900exe8", "pero_EGF1_h_p0p1_p2900exe9", "pero_EGF1_h_p0p1_p300000exe0", "pero_EGF1_h_p0p1_p300000exe1", "pero_EGF1_h_p0p1_p300000exe10", "pero_EGF1_h_p0p1_p300000exe11", "pero_EGF1_h_p0p1_p300000exe12", "pero_EGF1_h_p0p1_p300000exe13", "pero_EGF1_h_p0p1_p300000exe14", "pero_EGF1_h_p0p1_p300000exe15", "pero_EGF1_h_p0p1_p300000exe16", "pero_EGF1_h_p0p1_p300000exe2", "pero_EGF1_h_p0p1_p300000exe3", "pero_EGF1_h_p0p1_p300000exe4", "pero_EGF1_h_p0p1_p300000exe5", "pero_EGF1_h_p0p1_p300000exe6", "pero_EGF1_h_p0p1_p300000exe7", "pero_EGF1_h_p0p1_p300000exe8", "pero_EGF1_h_p0p1_p300000exe9", "pero_EGF1_h_p0p1_p30000exe0", "pero_EGF1_h_p0p1_p30000exe1", "pero_EGF1_h_p0p1_p30000exe10", "pero_EGF1_h_p0p1_p30000exe11", "pero_EGF1_h_p0p1_p30000exe12", "pero_EGF1_h_p0p1_p30000exe13", "pero_EGF1_h_p0p1_p30000exe14", "pero_EGF1_h_p0p1_p30000exe15", "pero_EGF1_h_p0p1_p30000exe16", "pero_EGF1_h_p0p1_p30000exe2", "pero_EGF1_h_p0p1_p30000exe3", "pero_EGF1_h_p0p1_p30000exe4", "pero_EGF1_h_p0p1_p30000exe5", "pero_EGF1_h_p0p1_p30000exe6", "pero_EGF1_h_p0p1_p30000exe7", "pero_EGF1_h_p0p1_p30000exe8", "pero_EGF1_h_p0p1_p30000exe9", "pero_EGF1_h_p0p1_p3000exe0", "pero_EGF1_h_p0p1_p3000exe1", "pero_EGF1_h_p0p1_p3000exe10", "pero_EGF1_h_p0p1_p3000exe11", "pero_EGF1_h_p0p1_p3000exe12", "pero_EGF1_h_p0p1_p3000exe13", "pero_EGF1_h_p0p1_p3000exe14", "pero_EGF1_h_p0p1_p3000exe15", "pero_EGF1_h_p0p1_p3000exe16", "pero_EGF1_h_p0p1_p3000exe17", "pero_EGF1_h_p0p1_p3000exe2", "pero_EGF1_h_p0p1_p3000exe3", "pero_EGF1_h_p0p1_p3000exe4", "pero_EGF1_h_p0p1_p3000exe5", "pero_EGF1_h_p0p1_p3000exe6", "pero_EGF1_h_p0p1_p3000exe7", "pero_EGF1_h_p0p1_p3000exe8", "pero_EGF1_h_p0p1_p3000exe9", "pero_EGF1_h_p0p1_p300exe0", "pero_EGF1_h_p0p1_p300exe1", "pero_EGF1_h_p0p1_p300exe10", "pero_EGF1_h_p0p1_p300exe11", "pero_EGF1_h_p0p1_p300exe12", "pero_EGF1_h_p0p1_p300exe13", "pero_EGF1_h_p0p1_p300exe14", "pero_EGF1_h_p0p1_p300exe15", "pero_EGF1_h_p0p1_p300exe16", "pero_EGF1_h_p0p1_p300exe2", "pero_EGF1_h_p0p1_p300exe3", "pero_EGF1_h_p0p1_p300exe4", "pero_EGF1_h_p0p1_p300exe5", "pero_EGF1_h_p0p1_p300exe6", "pero_EGF1_h_p0p1_p300exe7", "pero_EGF1_h_p0p1_p300exe8", "pero_EGF1_h_p0p1_p300exe9", "pero_EGF1_h_p0p1_p320000exe0", "pero_EGF1_h_p0p1_p320000exe1", "pero_EGF1_h_p0p1_p320000exe10", "pero_EGF1_h_p0p1_p320000exe11", "pero_EGF1_h_p0p1_p320000exe12", "pero_EGF1_h_p0p1_p320000exe13", "pero_EGF1_h_p0p1_p320000exe14", "pero_EGF1_h_p0p1_p320000exe15", "pero_EGF1_h_p0p1_p320000exe16", "pero_EGF1_h_p0p1_p320000exe2", "pero_EGF1_h_p0p1_p320000exe3", "pero_EGF1_h_p0p1_p320000exe4", "pero_EGF1_h_p0p1_p320000exe5", "pero_EGF1_h_p0p1_p320000exe6", "pero_EGF1_h_p0p1_p320000exe7", "pero_EGF1_h_p0p1_p320000exe8", "pero_EGF1_h_p0p1_p320000exe9", "pero_EGF1_h_p0p1_p340000exe0", "pero_EGF1_h_p0p1_p340000exe1", "pero_EGF1_h_p0p1_p340000exe10", "pero_EGF1_h_p0p1_p340000exe11", "pero_EGF1_h_p0p1_p340000exe12", "pero_EGF1_h_p0p1_p340000exe13", "pero_EGF1_h_p0p1_p340000exe14", "pero_EGF1_h_p0p1_p340000exe15", "pero_EGF1_h_p0p1_p340000exe16", "pero_EGF1_h_p0p1_p340000exe2", "pero_EGF1_h_p0p1_p340000exe3", "pero_EGF1_h_p0p1_p340000exe4", "pero_EGF1_h_p0p1_p340000exe5", "pero_EGF1_h_p0p1_p340000exe6", "pero_EGF1_h_p0p1_p340000exe7", "pero_EGF1_h_p0p1_p340000exe8", "pero_EGF1_h_p0p1_p340000exe9", "pero_EGF1_h_p0p1_p360000exe0", "pero_EGF1_h_p0p1_p360000exe1", "pero_EGF1_h_p0p1_p360000exe10", "pero_EGF1_h_p0p1_p360000exe11", "pero_EGF1_h_p0p1_p360000exe12", "pero_EGF1_h_p0p1_p360000exe13", "pero_EGF1_h_p0p1_p360000exe14", "pero_EGF1_h_p0p1_p360000exe15", "pero_EGF1_h_p0p1_p360000exe16", "pero_EGF1_h_p0p1_p360000exe2", "pero_EGF1_h_p0p1_p360000exe3", "pero_EGF1_h_p0p1_p360000exe4", "pero_EGF1_h_p0p1_p360000exe5", "pero_EGF1_h_p0p1_p360000exe6", "pero_EGF1_h_p0p1_p360000exe7", "pero_EGF1_h_p0p1_p360000exe8", "pero_EGF1_h_p0p1_p360000exe9", "pero_EGF1_h_p0p1_p380000exe0", "pero_EGF1_h_p0p1_p380000exe1", "pero_EGF1_h_p0p1_p380000exe10", "pero_EGF1_h_p0p1_p380000exe11", "pero_EGF1_h_p0p1_p380000exe12", "pero_EGF1_h_p0p1_p380000exe13", "pero_EGF1_h_p0p1_p380000exe14", "pero_EGF1_h_p0p1_p380000exe15", "pero_EGF1_h_p0p1_p380000exe16", "pero_EGF1_h_p0p1_p380000exe2", "pero_EGF1_h_p0p1_p380000exe3", "pero_EGF1_h_p0p1_p380000exe4", "pero_EGF1_h_p0p1_p380000exe5", "pero_EGF1_h_p0p1_p380000exe6", "pero_EGF1_h_p0p1_p380000exe7", "pero_EGF1_h_p0p1_p380000exe8", "pero_EGF1_h_p0p1_p380000exe9", "pero_EGF1_h_p0p1_p400000exe0", "pero_EGF1_h_p0p1_p400000exe1", "pero_EGF1_h_p0p1_p400000exe10", "pero_EGF1_h_p0p1_p400000exe11", "pero_EGF1_h_p0p1_p400000exe12", "pero_EGF1_h_p0p1_p400000exe13", "pero_EGF1_h_p0p1_p400000exe14", "pero_EGF1_h_p0p1_p400000exe15", "pero_EGF1_h_p0p1_p400000exe16", "pero_EGF1_h_p0p1_p400000exe2", "pero_EGF1_h_p0p1_p400000exe3", "pero_EGF1_h_p0p1_p400000exe4", "pero_EGF1_h_p0p1_p400000exe5", "pero_EGF1_h_p0p1_p400000exe6", "pero_EGF1_h_p0p1_p400000exe7", "pero_EGF1_h_p0p1_p400000exe8", "pero_EGF1_h_p0p1_p400000exe9", "pero_EGF1_h_p0p1_p40000exe0", "pero_EGF1_h_p0p1_p40000exe1", "pero_EGF1_h_p0p1_p40000exe10", "pero_EGF1_h_p0p1_p40000exe11", "pero_EGF1_h_p0p1_p40000exe12", "pero_EGF1_h_p0p1_p40000exe13", "pero_EGF1_h_p0p1_p40000exe14", "pero_EGF1_h_p0p1_p40000exe15", "pero_EGF1_h_p0p1_p40000exe16", "pero_EGF1_h_p0p1_p40000exe2", "pero_EGF1_h_p0p1_p40000exe3", "pero_EGF1_h_p0p1_p40000exe4", "pero_EGF1_h_p0p1_p40000exe5", "pero_EGF1_h_p0p1_p40000exe6", "pero_EGF1_h_p0p1_p40000exe7", "pero_EGF1_h_p0p1_p40000exe8", "pero_EGF1_h_p0p1_p40000exe9", "pero_EGF1_h_p0p1_p4000exe0", "pero_EGF1_h_p0p1_p4000exe1", "pero_EGF1_h_p0p1_p4000exe10", "pero_EGF1_h_p0p1_p4000exe11", "pero_EGF1_h_p0p1_p4000exe12", "pero_EGF1_h_p0p1_p4000exe13", "pero_EGF1_h_p0p1_p4000exe14", "pero_EGF1_h_p0p1_p4000exe15", "pero_EGF1_h_p0p1_p4000exe16", "pero_EGF1_h_p0p1_p4000exe2", "pero_EGF1_h_p0p1_p4000exe3", "pero_EGF1_h_p0p1_p4000exe4", "pero_EGF1_h_p0p1_p4000exe5", "pero_EGF1_h_p0p1_p4000exe6", "pero_EGF1_h_p0p1_p4000exe7", "pero_EGF1_h_p0p1_p4000exe8", "pero_EGF1_h_p0p1_p4000exe9", "pero_EGF1_h_p0p1_p400exe0", "pero_EGF1_h_p0p1_p400exe1", "pero_EGF1_h_p0p1_p400exe10", "pero_EGF1_h_p0p1_p400exe11", "pero_EGF1_h_p0p1_p400exe12", "pero_EGF1_h_p0p1_p400exe13", "pero_EGF1_h_p0p1_p400exe14", "pero_EGF1_h_p0p1_p400exe15", "pero_EGF1_h_p0p1_p400exe16", "pero_EGF1_h_p0p1_p400exe2", "pero_EGF1_h_p0p1_p400exe3", "pero_EGF1_h_p0p1_p400exe4", "pero_EGF1_h_p0p1_p400exe5", "pero_EGF1_h_p0p1_p400exe6", "pero_EGF1_h_p0p1_p400exe7", "pero_EGF1_h_p0p1_p400exe8", "pero_EGF1_h_p0p1_p400exe9", "pero_EGF1_h_p0p1_p420000exe0", "pero_EGF1_h_p0p1_p420000exe1", "pero_EGF1_h_p0p1_p420000exe10", "pero_EGF1_h_p0p1_p420000exe11", "pero_EGF1_h_p0p1_p420000exe12", "pero_EGF1_h_p0p1_p420000exe13", "pero_EGF1_h_p0p1_p420000exe14", "pero_EGF1_h_p0p1_p420000exe15", "pero_EGF1_h_p0p1_p420000exe16", "pero_EGF1_h_p0p1_p420000exe2", "pero_EGF1_h_p0p1_p420000exe3", "pero_EGF1_h_p0p1_p420000exe4", "pero_EGF1_h_p0p1_p420000exe5", "pero_EGF1_h_p0p1_p420000exe6", "pero_EGF1_h_p0p1_p420000exe7", "pero_EGF1_h_p0p1_p420000exe8", "pero_EGF1_h_p0p1_p420000exe9", "pero_EGF1_h_p0p1_p440000exe0", "pero_EGF1_h_p0p1_p440000exe1", "pero_EGF1_h_p0p1_p440000exe10", "pero_EGF1_h_p0p1_p440000exe11", "pero_EGF1_h_p0p1_p440000exe12", "pero_EGF1_h_p0p1_p440000exe13", "pero_EGF1_h_p0p1_p440000exe14", "pero_EGF1_h_p0p1_p440000exe15", "pero_EGF1_h_p0p1_p440000exe16", "pero_EGF1_h_p0p1_p440000exe2", "pero_EGF1_h_p0p1_p440000exe3", "pero_EGF1_h_p0p1_p440000exe4", "pero_EGF1_h_p0p1_p440000exe5", "pero_EGF1_h_p0p1_p440000exe6", "pero_EGF1_h_p0p1_p440000exe7", "pero_EGF1_h_p0p1_p440000exe8", "pero_EGF1_h_p0p1_p440000exe9", "pero_EGF1_h_p0p1_p480000exe0", "pero_EGF1_h_p0p1_p480000exe1", "pero_EGF1_h_p0p1_p480000exe10", "pero_EGF1_h_p0p1_p480000exe11", "pero_EGF1_h_p0p1_p480000exe12", "pero_EGF1_h_p0p1_p480000exe13", "pero_EGF1_h_p0p1_p480000exe14", "pero_EGF1_h_p0p1_p480000exe15", "pero_EGF1_h_p0p1_p480000exe16", "pero_EGF1_h_p0p1_p480000exe2", "pero_EGF1_h_p0p1_p480000exe3", "pero_EGF1_h_p0p1_p480000exe4", "pero_EGF1_h_p0p1_p480000exe5", "pero_EGF1_h_p0p1_p480000exe6", "pero_EGF1_h_p0p1_p480000exe7", "pero_EGF1_h_p0p1_p480000exe8", "pero_EGF1_h_p0p1_p480000exe9", "pero_EGF1_h_p0p1_p500000exe0", "pero_EGF1_h_p0p1_p500000exe1", "pero_EGF1_h_p0p1_p500000exe10", "pero_EGF1_h_p0p1_p500000exe11", "pero_EGF1_h_p0p1_p500000exe12", "pero_EGF1_h_p0p1_p500000exe13", "pero_EGF1_h_p0p1_p500000exe14", "pero_EGF1_h_p0p1_p500000exe15", "pero_EGF1_h_p0p1_p500000exe16", "pero_EGF1_h_p0p1_p500000exe2", "pero_EGF1_h_p0p1_p500000exe3", "pero_EGF1_h_p0p1_p500000exe4", "pero_EGF1_h_p0p1_p500000exe5", "pero_EGF1_h_p0p1_p500000exe6", "pero_EGF1_h_p0p1_p500000exe7", "pero_EGF1_h_p0p1_p500000exe8", "pero_EGF1_h_p0p1_p500000exe9", "pero_EGF1_h_p0p1_p50000exe0", "pero_EGF1_h_p0p1_p50000exe1", "pero_EGF1_h_p0p1_p50000exe10", "pero_EGF1_h_p0p1_p50000exe11", "pero_EGF1_h_p0p1_p50000exe12", "pero_EGF1_h_p0p1_p50000exe13", "pero_EGF1_h_p0p1_p50000exe14", "pero_EGF1_h_p0p1_p50000exe15", "pero_EGF1_h_p0p1_p50000exe16", "pero_EGF1_h_p0p1_p50000exe2", "pero_EGF1_h_p0p1_p50000exe3", "pero_EGF1_h_p0p1_p50000exe4", "pero_EGF1_h_p0p1_p50000exe5", "pero_EGF1_h_p0p1_p50000exe6", "pero_EGF1_h_p0p1_p50000exe7", "pero_EGF1_h_p0p1_p50000exe8", "pero_EGF1_h_p0p1_p50000exe9", "pero_EGF1_h_p0p1_p500exe0", "pero_EGF1_h_p0p1_p500exe1", "pero_EGF1_h_p0p1_p500exe10", "pero_EGF1_h_p0p1_p500exe11", "pero_EGF1_h_p0p1_p500exe12", "pero_EGF1_h_p0p1_p500exe13", "pero_EGF1_h_p0p1_p500exe14", "pero_EGF1_h_p0p1_p500exe15", "pero_EGF1_h_p0p1_p500exe16", "pero_EGF1_h_p0p1_p500exe2", "pero_EGF1_h_p0p1_p500exe3", "pero_EGF1_h_p0p1_p500exe4", "pero_EGF1_h_p0p1_p500exe5", "pero_EGF1_h_p0p1_p500exe6", "pero_EGF1_h_p0p1_p500exe7", "pero_EGF1_h_p0p1_p500exe8", "pero_EGF1_h_p0p1_p500exe9", "pero_EGF1_h_p0p1_p60000exe0", "pero_EGF1_h_p0p1_p60000exe1", "pero_EGF1_h_p0p1_p60000exe10", "pero_EGF1_h_p0p1_p60000exe11", "pero_EGF1_h_p0p1_p60000exe12", "pero_EGF1_h_p0p1_p60000exe13", "pero_EGF1_h_p0p1_p60000exe14", "pero_EGF1_h_p0p1_p60000exe15", "pero_EGF1_h_p0p1_p60000exe16", "pero_EGF1_h_p0p1_p60000exe2", "pero_EGF1_h_p0p1_p60000exe3", "pero_EGF1_h_p0p1_p60000exe4", "pero_EGF1_h_p0p1_p60000exe5", "pero_EGF1_h_p0p1_p60000exe6", "pero_EGF1_h_p0p1_p60000exe7", "pero_EGF1_h_p0p1_p60000exe8", "pero_EGF1_h_p0p1_p60000exe9", "pero_EGF1_h_p0p1_p6000exe0", "pero_EGF1_h_p0p1_p6000exe1", "pero_EGF1_h_p0p1_p6000exe10", "pero_EGF1_h_p0p1_p6000exe11", "pero_EGF1_h_p0p1_p6000exe12", "pero_EGF1_h_p0p1_p6000exe13", "pero_EGF1_h_p0p1_p6000exe14", "pero_EGF1_h_p0p1_p6000exe15", "pero_EGF1_h_p0p1_p6000exe16", "pero_EGF1_h_p0p1_p6000exe2", "pero_EGF1_h_p0p1_p6000exe3", "pero_EGF1_h_p0p1_p6000exe4", "pero_EGF1_h_p0p1_p6000exe5", "pero_EGF1_h_p0p1_p6000exe6", "pero_EGF1_h_p0p1_p6000exe7", "pero_EGF1_h_p0p1_p6000exe8", "pero_EGF1_h_p0p1_p6000exe9", "pero_EGF1_h_p0p1_p600exe0", "pero_EGF1_h_p0p1_p600exe1", "pero_EGF1_h_p0p1_p600exe10", "pero_EGF1_h_p0p1_p600exe11", "pero_EGF1_h_p0p1_p600exe12", "pero_EGF1_h_p0p1_p600exe13", "pero_EGF1_h_p0p1_p600exe14", "pero_EGF1_h_p0p1_p600exe15", "pero_EGF1_h_p0p1_p600exe16", "pero_EGF1_h_p0p1_p600exe17", "pero_EGF1_h_p0p1_p600exe2", "pero_EGF1_h_p0p1_p600exe3", "pero_EGF1_h_p0p1_p600exe4", "pero_EGF1_h_p0p1_p600exe5", "pero_EGF1_h_p0p1_p600exe6", "pero_EGF1_h_p0p1_p600exe7", "pero_EGF1_h_p0p1_p600exe8", "pero_EGF1_h_p0p1_p600exe9", "pero_EGF1_h_p0p1_p700exe0", "pero_EGF1_h_p0p1_p700exe1", "pero_EGF1_h_p0p1_p700exe10", "pero_EGF1_h_p0p1_p700exe11", "pero_EGF1_h_p0p1_p700exe12", "pero_EGF1_h_p0p1_p700exe13", "pero_EGF1_h_p0p1_p700exe14", "pero_EGF1_h_p0p1_p700exe15", "pero_EGF1_h_p0p1_p700exe16", "pero_EGF1_h_p0p1_p700exe2", "pero_EGF1_h_p0p1_p700exe3", "pero_EGF1_h_p0p1_p700exe4", "pero_EGF1_h_p0p1_p700exe5", "pero_EGF1_h_p0p1_p700exe6", "pero_EGF1_h_p0p1_p700exe7", "pero_EGF1_h_p0p1_p700exe8", "pero_EGF1_h_p0p1_p700exe9", "pero_EGF1_h_p0p1_p80000exe0", "pero_EGF1_h_p0p1_p80000exe1", "pero_EGF1_h_p0p1_p80000exe10", "pero_EGF1_h_p0p1_p80000exe11", "pero_EGF1_h_p0p1_p80000exe12", "pero_EGF1_h_p0p1_p80000exe13", "pero_EGF1_h_p0p1_p80000exe14", "pero_EGF1_h_p0p1_p80000exe15", "pero_EGF1_h_p0p1_p80000exe16", "pero_EGF1_h_p0p1_p80000exe2", "pero_EGF1_h_p0p1_p80000exe3", "pero_EGF1_h_p0p1_p80000exe4", "pero_EGF1_h_p0p1_p80000exe5", "pero_EGF1_h_p0p1_p80000exe6", "pero_EGF1_h_p0p1_p80000exe7", "pero_EGF1_h_p0p1_p80000exe8", "pero_EGF1_h_p0p1_p80000exe9", "pero_EGF1_h_p0p1_p800exe0", "pero_EGF1_h_p0p1_p800exe1", "pero_EGF1_h_p0p1_p800exe10", "pero_EGF1_h_p0p1_p800exe11", "pero_EGF1_h_p0p1_p800exe12", "pero_EGF1_h_p0p1_p800exe13", "pero_EGF1_h_p0p1_p800exe14", "pero_EGF1_h_p0p1_p800exe15", "pero_EGF1_h_p0p1_p800exe16", "pero_EGF1_h_p0p1_p800exe2", "pero_EGF1_h_p0p1_p800exe3", "pero_EGF1_h_p0p1_p800exe4", "pero_EGF1_h_p0p1_p800exe5", "pero_EGF1_h_p0p1_p800exe6", "pero_EGF1_h_p0p1_p800exe7", "pero_EGF1_h_p0p1_p800exe8", "pero_EGF1_h_p0p1_p800exe9", "pero_EGF1_h_p0p1_p900exe0", "pero_EGF1_h_p0p1_p900exe1", "pero_EGF1_h_p0p1_p900exe10", "pero_EGF1_h_p0p1_p900exe11", "pero_EGF1_h_p0p1_p900exe12", "pero_EGF1_h_p0p1_p900exe13", "pero_EGF1_h_p0p1_p900exe14", "pero_EGF1_h_p0p1_p900exe15", "pero_EGF1_h_p0p1_p900exe16", "pero_EGF1_h_p0p1_p900exe2", "pero_EGF1_h_p0p1_p900exe3", "pero_EGF1_h_p0p1_p900exe4", "pero_EGF1_h_p0p1_p900exe5", "pero_EGF1_h_p0p1_p900exe6", "pero_EGF1_h_p0p1_p900exe7", "pero_EGF1_h_p0p1_p900exe8", "pero_EGF1_h_p0p1_p900exe9", "pero_EGF1_h_p1m1_m0exe0", "pero_EGF1_h_p1m1_m0exe1", "pero_EGF1_h_p1m1_m0exe10", "pero_EGF1_h_p1m1_m0exe11", "pero_EGF1_h_p1m1_m0exe12", "pero_EGF1_h_p1m1_m0exe13", "pero_EGF1_h_p1m1_m0exe14", "pero_EGF1_h_p1m1_m0exe15", "pero_EGF1_h_p1m1_m0exe16", "pero_EGF1_h_p1m1_m0exe2", "pero_EGF1_h_p1m1_m0exe3", "pero_EGF1_h_p1m1_m0exe4", "pero_EGF1_h_p1m1_m0exe5", "pero_EGF1_h_p1m1_m0exe6", "pero_EGF1_h_p1m1_m0exe7", "pero_EGF1_h_p1m1_m0exe8", "pero_EGF1_h_p1m1_m0exe9", "pero_EGF1_h_p1m1_m100exe0", "pero_EGF1_h_p1m1_m100exe1", "pero_EGF1_h_p1m1_m100exe10", "pero_EGF1_h_p1m1_m100exe11", "pero_EGF1_h_p1m1_m100exe12", "pero_EGF1_h_p1m1_m100exe13", "pero_EGF1_h_p1m1_m100exe14", "pero_EGF1_h_p1m1_m100exe15", "pero_EGF1_h_p1m1_m100exe16", "pero_EGF1_h_p1m1_m100exe2", "pero_EGF1_h_p1m1_m100exe3", "pero_EGF1_h_p1m1_m100exe4", "pero_EGF1_h_p1m1_m100exe5", "pero_EGF1_h_p1m1_m100exe6", "pero_EGF1_h_p1m1_m100exe7", "pero_EGF1_h_p1m1_m100exe8", "pero_EGF1_h_p1m1_m100exe9", "pero_EGF1_h_p1m1_m200exe0", "pero_EGF1_h_p1m1_m200exe1", "pero_EGF1_h_p1m1_m200exe10", "pero_EGF1_h_p1m1_m200exe11", "pero_EGF1_h_p1m1_m200exe12", "pero_EGF1_h_p1m1_m200exe13", "pero_EGF1_h_p1m1_m200exe14", "pero_EGF1_h_p1m1_m200exe15", "pero_EGF1_h_p1m1_m200exe16", "pero_EGF1_h_p1m1_m200exe2", "pero_EGF1_h_p1m1_m200exe3", "pero_EGF1_h_p1m1_m200exe4", "pero_EGF1_h_p1m1_m200exe5", "pero_EGF1_h_p1m1_m200exe6", "pero_EGF1_h_p1m1_m200exe7", "pero_EGF1_h_p1m1_m200exe8", "pero_EGF1_h_p1m1_m200exe9", "pero_EGF1_h_p1m1_m300exe0", "pero_EGF1_h_p1m1_m300exe1", "pero_EGF1_h_p1m1_m300exe10", "pero_EGF1_h_p1m1_m300exe11", "pero_EGF1_h_p1m1_m300exe12", "pero_EGF1_h_p1m1_m300exe13", "pero_EGF1_h_p1m1_m300exe14", "pero_EGF1_h_p1m1_m300exe15", "pero_EGF1_h_p1m1_m300exe16", "pero_EGF1_h_p1m1_m300exe2", "pero_EGF1_h_p1m1_m300exe3", "pero_EGF1_h_p1m1_m300exe4", "pero_EGF1_h_p1m1_m300exe5", "pero_EGF1_h_p1m1_m300exe6", "pero_EGF1_h_p1m1_m300exe7", "pero_EGF1_h_p1m1_m300exe8", "pero_EGF1_h_p1m1_m300exe9", "pero_EGF1_h_p1m1_m5000exe0", "pero_EGF1_h_p1m1_m5000exe1", "pero_EGF1_h_p1m1_m5000exe10", "pero_EGF1_h_p1m1_m5000exe11", "pero_EGF1_h_p1m1_m5000exe12", "pero_EGF1_h_p1m1_m5000exe13", "pero_EGF1_h_p1m1_m5000exe14", "pero_EGF1_h_p1m1_m5000exe15", "pero_EGF1_h_p1m1_m5000exe16", "pero_EGF1_h_p1m1_m5000exe2", "pero_EGF1_h_p1m1_m5000exe3", "pero_EGF1_h_p1m1_m5000exe4", "pero_EGF1_h_p1m1_m5000exe5", "pero_EGF1_h_p1m1_m5000exe6", "pero_EGF1_h_p1m1_m5000exe7", "pero_EGF1_h_p1m1_m5000exe8", "pero_EGF1_h_p1m1_m5000exe9", "pero_EGF1_h_p1m1_m500exe0", "pero_EGF1_h_p1m1_m500exe1", "pero_EGF1_h_p1m1_m500exe10", "pero_EGF1_h_p1m1_m500exe11", "pero_EGF1_h_p1m1_m500exe12", "pero_EGF1_h_p1m1_m500exe13", "pero_EGF1_h_p1m1_m500exe14", "pero_EGF1_h_p1m1_m500exe15", "pero_EGF1_h_p1m1_m500exe16", "pero_EGF1_h_p1m1_m500exe2", "pero_EGF1_h_p1m1_m500exe3", "pero_EGF1_h_p1m1_m500exe4", "pero_EGF1_h_p1m1_m500exe5", "pero_EGF1_h_p1m1_m500exe6", "pero_EGF1_h_p1m1_m500exe7", "pero_EGF1_h_p1m1_m500exe8", "pero_EGF1_h_p1m1_m500exe9", "pero_EGF1_h_p1m1_p100000exe0", "pero_EGF1_h_p1m1_p100000exe1", "pero_EGF1_h_p1m1_p100000exe10", "pero_EGF1_h_p1m1_p100000exe11", "pero_EGF1_h_p1m1_p100000exe12", "pero_EGF1_h_p1m1_p100000exe13", "pero_EGF1_h_p1m1_p100000exe14", "pero_EGF1_h_p1m1_p100000exe15", "pero_EGF1_h_p1m1_p100000exe16", "pero_EGF1_h_p1m1_p100000exe2", "pero_EGF1_h_p1m1_p100000exe3", "pero_EGF1_h_p1m1_p100000exe4", "pero_EGF1_h_p1m1_p100000exe5", "pero_EGF1_h_p1m1_p100000exe6", "pero_EGF1_h_p1m1_p100000exe7", "pero_EGF1_h_p1m1_p100000exe8", "pero_EGF1_h_p1m1_p100000exe9", "pero_EGF1_h_p1m1_p10000exe0", "pero_EGF1_h_p1m1_p10000exe1", "pero_EGF1_h_p1m1_p10000exe10", "pero_EGF1_h_p1m1_p10000exe11", "pero_EGF1_h_p1m1_p10000exe12", "pero_EGF1_h_p1m1_p10000exe13", "pero_EGF1_h_p1m1_p10000exe14", "pero_EGF1_h_p1m1_p10000exe15", "pero_EGF1_h_p1m1_p10000exe16", "pero_EGF1_h_p1m1_p10000exe2", "pero_EGF1_h_p1m1_p10000exe3", "pero_EGF1_h_p1m1_p10000exe4", "pero_EGF1_h_p1m1_p10000exe5", "pero_EGF1_h_p1m1_p10000exe6", "pero_EGF1_h_p1m1_p10000exe7", "pero_EGF1_h_p1m1_p10000exe8", "pero_EGF1_h_p1m1_p10000exe9", "pero_EGF1_h_p1m1_p1000exe0", "pero_EGF1_h_p1m1_p1000exe1", "pero_EGF1_h_p1m1_p1000exe10", "pero_EGF1_h_p1m1_p1000exe11", "pero_EGF1_h_p1m1_p1000exe12", "pero_EGF1_h_p1m1_p1000exe13", "pero_EGF1_h_p1m1_p1000exe14", "pero_EGF1_h_p1m1_p1000exe15", "pero_EGF1_h_p1m1_p1000exe16", "pero_EGF1_h_p1m1_p1000exe17", "pero_EGF1_h_p1m1_p1000exe2", "pero_EGF1_h_p1m1_p1000exe3", "pero_EGF1_h_p1m1_p1000exe4", "pero_EGF1_h_p1m1_p1000exe5", "pero_EGF1_h_p1m1_p1000exe6", "pero_EGF1_h_p1m1_p1000exe7", "pero_EGF1_h_p1m1_p1000exe8", "pero_EGF1_h_p1m1_p1000exe9", "pero_EGF1_h_p1m1_p100exe0", "pero_EGF1_h_p1m1_p100exe1", "pero_EGF1_h_p1m1_p100exe10", "pero_EGF1_h_p1m1_p100exe11", "pero_EGF1_h_p1m1_p100exe12", "pero_EGF1_h_p1m1_p100exe13", "pero_EGF1_h_p1m1_p100exe14", "pero_EGF1_h_p1m1_p100exe15", "pero_EGF1_h_p1m1_p100exe16", "pero_EGF1_h_p1m1_p100exe2", "pero_EGF1_h_p1m1_p100exe3", "pero_EGF1_h_p1m1_p100exe4", "pero_EGF1_h_p1m1_p100exe5", "pero_EGF1_h_p1m1_p100exe6", "pero_EGF1_h_p1m1_p100exe7", "pero_EGF1_h_p1m1_p100exe8", "pero_EGF1_h_p1m1_p100exe9", "pero_EGF1_h_p1m1_p1100exe0", "pero_EGF1_h_p1m1_p1100exe1", "pero_EGF1_h_p1m1_p1100exe10", "pero_EGF1_h_p1m1_p1100exe11", "pero_EGF1_h_p1m1_p1100exe12", "pero_EGF1_h_p1m1_p1100exe13", "pero_EGF1_h_p1m1_p1100exe14", "pero_EGF1_h_p1m1_p1100exe15", "pero_EGF1_h_p1m1_p1100exe16", "pero_EGF1_h_p1m1_p1100exe2", "pero_EGF1_h_p1m1_p1100exe3", "pero_EGF1_h_p1m1_p1100exe4", "pero_EGF1_h_p1m1_p1100exe5", "pero_EGF1_h_p1m1_p1100exe6", "pero_EGF1_h_p1m1_p1100exe7", "pero_EGF1_h_p1m1_p1100exe8", "pero_EGF1_h_p1m1_p1100exe9", "pero_EGF1_h_p1m1_p120000exe0", "pero_EGF1_h_p1m1_p120000exe1", "pero_EGF1_h_p1m1_p120000exe10", "pero_EGF1_h_p1m1_p120000exe11", "pero_EGF1_h_p1m1_p120000exe12", "pero_EGF1_h_p1m1_p120000exe13", "pero_EGF1_h_p1m1_p120000exe14", "pero_EGF1_h_p1m1_p120000exe15", "pero_EGF1_h_p1m1_p120000exe16", "pero_EGF1_h_p1m1_p120000exe2", "pero_EGF1_h_p1m1_p120000exe3", "pero_EGF1_h_p1m1_p120000exe4", "pero_EGF1_h_p1m1_p120000exe5", "pero_EGF1_h_p1m1_p120000exe6", "pero_EGF1_h_p1m1_p120000exe7", "pero_EGF1_h_p1m1_p120000exe8", "pero_EGF1_h_p1m1_p120000exe9", "pero_EGF1_h_p1m1_p1200exe0", "pero_EGF1_h_p1m1_p1200exe1", "pero_EGF1_h_p1m1_p1200exe10", "pero_EGF1_h_p1m1_p1200exe11", "pero_EGF1_h_p1m1_p1200exe12", "pero_EGF1_h_p1m1_p1200exe13", "pero_EGF1_h_p1m1_p1200exe14", "pero_EGF1_h_p1m1_p1200exe15", "pero_EGF1_h_p1m1_p1200exe16", "pero_EGF1_h_p1m1_p1200exe2", "pero_EGF1_h_p1m1_p1200exe3", "pero_EGF1_h_p1m1_p1200exe4", "pero_EGF1_h_p1m1_p1200exe5", "pero_EGF1_h_p1m1_p1200exe6", "pero_EGF1_h_p1m1_p1200exe7", "pero_EGF1_h_p1m1_p1200exe8", "pero_EGF1_h_p1m1_p1200exe9", "pero_EGF1_h_p1m1_p1300exe0", "pero_EGF1_h_p1m1_p1300exe1", "pero_EGF1_h_p1m1_p1300exe10", "pero_EGF1_h_p1m1_p1300exe11", "pero_EGF1_h_p1m1_p1300exe12", "pero_EGF1_h_p1m1_p1300exe13", "pero_EGF1_h_p1m1_p1300exe14", "pero_EGF1_h_p1m1_p1300exe15", "pero_EGF1_h_p1m1_p1300exe16", "pero_EGF1_h_p1m1_p1300exe2", "pero_EGF1_h_p1m1_p1300exe3", "pero_EGF1_h_p1m1_p1300exe4", "pero_EGF1_h_p1m1_p1300exe5", "pero_EGF1_h_p1m1_p1300exe6", "pero_EGF1_h_p1m1_p1300exe7", "pero_EGF1_h_p1m1_p1300exe8", "pero_EGF1_h_p1m1_p1300exe9", "pero_EGF1_h_p1m1_p140000exe0", "pero_EGF1_h_p1m1_p140000exe1", "pero_EGF1_h_p1m1_p140000exe10", "pero_EGF1_h_p1m1_p140000exe11", "pero_EGF1_h_p1m1_p140000exe12", "pero_EGF1_h_p1m1_p140000exe13", "pero_EGF1_h_p1m1_p140000exe14", "pero_EGF1_h_p1m1_p140000exe15", "pero_EGF1_h_p1m1_p140000exe16", "pero_EGF1_h_p1m1_p140000exe2", "pero_EGF1_h_p1m1_p140000exe3", "pero_EGF1_h_p1m1_p140000exe4", "pero_EGF1_h_p1m1_p140000exe5", "pero_EGF1_h_p1m1_p140000exe6", "pero_EGF1_h_p1m1_p140000exe7", "pero_EGF1_h_p1m1_p140000exe8", "pero_EGF1_h_p1m1_p140000exe9", "pero_EGF1_h_p1m1_p1400exe0", "pero_EGF1_h_p1m1_p1400exe1", "pero_EGF1_h_p1m1_p1400exe10", "pero_EGF1_h_p1m1_p1400exe11", "pero_EGF1_h_p1m1_p1400exe12", "pero_EGF1_h_p1m1_p1400exe13", "pero_EGF1_h_p1m1_p1400exe14", "pero_EGF1_h_p1m1_p1400exe15", "pero_EGF1_h_p1m1_p1400exe16", "pero_EGF1_h_p1m1_p1400exe2", "pero_EGF1_h_p1m1_p1400exe3", "pero_EGF1_h_p1m1_p1400exe4", "pero_EGF1_h_p1m1_p1400exe5", "pero_EGF1_h_p1m1_p1400exe6", "pero_EGF1_h_p1m1_p1400exe7", "pero_EGF1_h_p1m1_p1400exe8", "pero_EGF1_h_p1m1_p1400exe9", "pero_EGF1_h_p1m1_p1500exe0", "pero_EGF1_h_p1m1_p1500exe1", "pero_EGF1_h_p1m1_p1500exe10", "pero_EGF1_h_p1m1_p1500exe11", "pero_EGF1_h_p1m1_p1500exe12", "pero_EGF1_h_p1m1_p1500exe13", "pero_EGF1_h_p1m1_p1500exe14", "pero_EGF1_h_p1m1_p1500exe15", "pero_EGF1_h_p1m1_p1500exe16", "pero_EGF1_h_p1m1_p1500exe2", "pero_EGF1_h_p1m1_p1500exe3", "pero_EGF1_h_p1m1_p1500exe4", "pero_EGF1_h_p1m1_p1500exe5", "pero_EGF1_h_p1m1_p1500exe6", "pero_EGF1_h_p1m1_p1500exe7", "pero_EGF1_h_p1m1_p1500exe8", "pero_EGF1_h_p1m1_p1500exe9", "pero_EGF1_h_p1m1_p160000exe0", "pero_EGF1_h_p1m1_p160000exe1", "pero_EGF1_h_p1m1_p160000exe10", "pero_EGF1_h_p1m1_p160000exe11", "pero_EGF1_h_p1m1_p160000exe12", "pero_EGF1_h_p1m1_p160000exe13", "pero_EGF1_h_p1m1_p160000exe14", "pero_EGF1_h_p1m1_p160000exe15", "pero_EGF1_h_p1m1_p160000exe16", "pero_EGF1_h_p1m1_p160000exe2", "pero_EGF1_h_p1m1_p160000exe3", "pero_EGF1_h_p1m1_p160000exe4", "pero_EGF1_h_p1m1_p160000exe5", "pero_EGF1_h_p1m1_p160000exe6", "pero_EGF1_h_p1m1_p160000exe7", "pero_EGF1_h_p1m1_p160000exe8", "pero_EGF1_h_p1m1_p160000exe9", "pero_EGF1_h_p1m1_p1600exe0", "pero_EGF1_h_p1m1_p1600exe1", "pero_EGF1_h_p1m1_p1600exe10", "pero_EGF1_h_p1m1_p1600exe11", "pero_EGF1_h_p1m1_p1600exe12", "pero_EGF1_h_p1m1_p1600exe13", "pero_EGF1_h_p1m1_p1600exe14", "pero_EGF1_h_p1m1_p1600exe15", "pero_EGF1_h_p1m1_p1600exe16", "pero_EGF1_h_p1m1_p1600exe2", "pero_EGF1_h_p1m1_p1600exe3", "pero_EGF1_h_p1m1_p1600exe4", "pero_EGF1_h_p1m1_p1600exe5", "pero_EGF1_h_p1m1_p1600exe6", "pero_EGF1_h_p1m1_p1600exe7", "pero_EGF1_h_p1m1_p1600exe8", "pero_EGF1_h_p1m1_p1600exe9", "pero_EGF1_h_p1m1_p1700exe0", "pero_EGF1_h_p1m1_p1700exe1", "pero_EGF1_h_p1m1_p1700exe10", "pero_EGF1_h_p1m1_p1700exe11", "pero_EGF1_h_p1m1_p1700exe12", "pero_EGF1_h_p1m1_p1700exe13", "pero_EGF1_h_p1m1_p1700exe14", "pero_EGF1_h_p1m1_p1700exe15", "pero_EGF1_h_p1m1_p1700exe16", "pero_EGF1_h_p1m1_p1700exe2", "pero_EGF1_h_p1m1_p1700exe3", "pero_EGF1_h_p1m1_p1700exe4", "pero_EGF1_h_p1m1_p1700exe5", "pero_EGF1_h_p1m1_p1700exe6", "pero_EGF1_h_p1m1_p1700exe7", "pero_EGF1_h_p1m1_p1700exe8", "pero_EGF1_h_p1m1_p1700exe9", "pero_EGF1_h_p1m1_p180000exe0", "pero_EGF1_h_p1m1_p180000exe1", "pero_EGF1_h_p1m1_p180000exe10", "pero_EGF1_h_p1m1_p180000exe11", "pero_EGF1_h_p1m1_p180000exe12", "pero_EGF1_h_p1m1_p180000exe13", "pero_EGF1_h_p1m1_p180000exe14", "pero_EGF1_h_p1m1_p180000exe15", "pero_EGF1_h_p1m1_p180000exe16", "pero_EGF1_h_p1m1_p180000exe2", "pero_EGF1_h_p1m1_p180000exe3", "pero_EGF1_h_p1m1_p180000exe4", "pero_EGF1_h_p1m1_p180000exe5", "pero_EGF1_h_p1m1_p180000exe6", "pero_EGF1_h_p1m1_p180000exe7", "pero_EGF1_h_p1m1_p180000exe8", "pero_EGF1_h_p1m1_p180000exe9", "pero_EGF1_h_p1m1_p1800exe0", "pero_EGF1_h_p1m1_p1800exe1", "pero_EGF1_h_p1m1_p1800exe10", "pero_EGF1_h_p1m1_p1800exe11", "pero_EGF1_h_p1m1_p1800exe12", "pero_EGF1_h_p1m1_p1800exe13", "pero_EGF1_h_p1m1_p1800exe14", "pero_EGF1_h_p1m1_p1800exe15", "pero_EGF1_h_p1m1_p1800exe16", "pero_EGF1_h_p1m1_p1800exe2", "pero_EGF1_h_p1m1_p1800exe3", "pero_EGF1_h_p1m1_p1800exe4", "pero_EGF1_h_p1m1_p1800exe5", "pero_EGF1_h_p1m1_p1800exe6", "pero_EGF1_h_p1m1_p1800exe7", "pero_EGF1_h_p1m1_p1800exe8", "pero_EGF1_h_p1m1_p1800exe9", "pero_EGF1_h_p1m1_p1900exe0", "pero_EGF1_h_p1m1_p1900exe1", "pero_EGF1_h_p1m1_p1900exe10", "pero_EGF1_h_p1m1_p1900exe11", "pero_EGF1_h_p1m1_p1900exe12", "pero_EGF1_h_p1m1_p1900exe13", "pero_EGF1_h_p1m1_p1900exe14", "pero_EGF1_h_p1m1_p1900exe15", "pero_EGF1_h_p1m1_p1900exe16", "pero_EGF1_h_p1m1_p1900exe17", "pero_EGF1_h_p1m1_p1900exe2", "pero_EGF1_h_p1m1_p1900exe3", "pero_EGF1_h_p1m1_p1900exe4", "pero_EGF1_h_p1m1_p1900exe5", "pero_EGF1_h_p1m1_p1900exe6", "pero_EGF1_h_p1m1_p1900exe7", "pero_EGF1_h_p1m1_p1900exe8", "pero_EGF1_h_p1m1_p1900exe9", "pero_EGF1_h_p1m1_p200000exe0", "pero_EGF1_h_p1m1_p200000exe1", "pero_EGF1_h_p1m1_p200000exe10", "pero_EGF1_h_p1m1_p200000exe11", "pero_EGF1_h_p1m1_p200000exe12", "pero_EGF1_h_p1m1_p200000exe13", "pero_EGF1_h_p1m1_p200000exe14", "pero_EGF1_h_p1m1_p200000exe15", "pero_EGF1_h_p1m1_p200000exe16", "pero_EGF1_h_p1m1_p200000exe2", "pero_EGF1_h_p1m1_p200000exe3", "pero_EGF1_h_p1m1_p200000exe4", "pero_EGF1_h_p1m1_p200000exe5", "pero_EGF1_h_p1m1_p200000exe6", "pero_EGF1_h_p1m1_p200000exe7", "pero_EGF1_h_p1m1_p200000exe8", "pero_EGF1_h_p1m1_p200000exe9", "pero_EGF1_h_p1m1_p20000exe0", "pero_EGF1_h_p1m1_p20000exe1", "pero_EGF1_h_p1m1_p20000exe10", "pero_EGF1_h_p1m1_p20000exe11", "pero_EGF1_h_p1m1_p20000exe12", "pero_EGF1_h_p1m1_p20000exe13", "pero_EGF1_h_p1m1_p20000exe14", "pero_EGF1_h_p1m1_p20000exe15", "pero_EGF1_h_p1m1_p20000exe16", "pero_EGF1_h_p1m1_p20000exe2", "pero_EGF1_h_p1m1_p20000exe3", "pero_EGF1_h_p1m1_p20000exe4", "pero_EGF1_h_p1m1_p20000exe5", "pero_EGF1_h_p1m1_p20000exe6", "pero_EGF1_h_p1m1_p20000exe7", "pero_EGF1_h_p1m1_p20000exe8", "pero_EGF1_h_p1m1_p20000exe9", "pero_EGF1_h_p1m1_p2000exe0", "pero_EGF1_h_p1m1_p2000exe1", "pero_EGF1_h_p1m1_p2000exe10", "pero_EGF1_h_p1m1_p2000exe11", "pero_EGF1_h_p1m1_p2000exe12", "pero_EGF1_h_p1m1_p2000exe13", "pero_EGF1_h_p1m1_p2000exe14", "pero_EGF1_h_p1m1_p2000exe15", "pero_EGF1_h_p1m1_p2000exe16", "pero_EGF1_h_p1m1_p2000exe2", "pero_EGF1_h_p1m1_p2000exe3", "pero_EGF1_h_p1m1_p2000exe4", "pero_EGF1_h_p1m1_p2000exe5", "pero_EGF1_h_p1m1_p2000exe6", "pero_EGF1_h_p1m1_p2000exe7", "pero_EGF1_h_p1m1_p2000exe8", "pero_EGF1_h_p1m1_p2000exe9", "pero_EGF1_h_p1m1_p200exe0", "pero_EGF1_h_p1m1_p200exe1", "pero_EGF1_h_p1m1_p200exe10", "pero_EGF1_h_p1m1_p200exe11", "pero_EGF1_h_p1m1_p200exe12", "pero_EGF1_h_p1m1_p200exe13", "pero_EGF1_h_p1m1_p200exe14", "pero_EGF1_h_p1m1_p200exe15", "pero_EGF1_h_p1m1_p200exe16", "pero_EGF1_h_p1m1_p200exe2", "pero_EGF1_h_p1m1_p200exe3", "pero_EGF1_h_p1m1_p200exe4", "pero_EGF1_h_p1m1_p200exe5", "pero_EGF1_h_p1m1_p200exe6", "pero_EGF1_h_p1m1_p200exe7", "pero_EGF1_h_p1m1_p200exe8", "pero_EGF1_h_p1m1_p200exe9", "pero_EGF1_h_p1m1_p2100exe0", "pero_EGF1_h_p1m1_p2100exe1", "pero_EGF1_h_p1m1_p2100exe10", "pero_EGF1_h_p1m1_p2100exe11", "pero_EGF1_h_p1m1_p2100exe12", "pero_EGF1_h_p1m1_p2100exe13", "pero_EGF1_h_p1m1_p2100exe14", "pero_EGF1_h_p1m1_p2100exe15", "pero_EGF1_h_p1m1_p2100exe16", "pero_EGF1_h_p1m1_p2100exe2", "pero_EGF1_h_p1m1_p2100exe3", "pero_EGF1_h_p1m1_p2100exe4", "pero_EGF1_h_p1m1_p2100exe5", "pero_EGF1_h_p1m1_p2100exe6", "pero_EGF1_h_p1m1_p2100exe7", "pero_EGF1_h_p1m1_p2100exe8", "pero_EGF1_h_p1m1_p2100exe9", "pero_EGF1_h_p1m1_p220000exe0", "pero_EGF1_h_p1m1_p220000exe1", "pero_EGF1_h_p1m1_p220000exe10", "pero_EGF1_h_p1m1_p220000exe11", "pero_EGF1_h_p1m1_p220000exe12", "pero_EGF1_h_p1m1_p220000exe13", "pero_EGF1_h_p1m1_p220000exe14", "pero_EGF1_h_p1m1_p220000exe15", "pero_EGF1_h_p1m1_p220000exe16", "pero_EGF1_h_p1m1_p220000exe2", "pero_EGF1_h_p1m1_p220000exe3", "pero_EGF1_h_p1m1_p220000exe4", "pero_EGF1_h_p1m1_p220000exe5", "pero_EGF1_h_p1m1_p220000exe6", "pero_EGF1_h_p1m1_p220000exe7", "pero_EGF1_h_p1m1_p220000exe8", "pero_EGF1_h_p1m1_p220000exe9", "pero_EGF1_h_p1m1_p2200exe0", "pero_EGF1_h_p1m1_p2200exe1", "pero_EGF1_h_p1m1_p2200exe10", "pero_EGF1_h_p1m1_p2200exe11", "pero_EGF1_h_p1m1_p2200exe12", "pero_EGF1_h_p1m1_p2200exe13", "pero_EGF1_h_p1m1_p2200exe14", "pero_EGF1_h_p1m1_p2200exe15", "pero_EGF1_h_p1m1_p2200exe16", "pero_EGF1_h_p1m1_p2200exe2", "pero_EGF1_h_p1m1_p2200exe3", "pero_EGF1_h_p1m1_p2200exe4", "pero_EGF1_h_p1m1_p2200exe5", "pero_EGF1_h_p1m1_p2200exe6", "pero_EGF1_h_p1m1_p2200exe7", "pero_EGF1_h_p1m1_p2200exe8", "pero_EGF1_h_p1m1_p2200exe9", "pero_EGF1_h_p1m1_p2300exe0", "pero_EGF1_h_p1m1_p2300exe1", "pero_EGF1_h_p1m1_p2300exe10", "pero_EGF1_h_p1m1_p2300exe11", "pero_EGF1_h_p1m1_p2300exe12", "pero_EGF1_h_p1m1_p2300exe13", "pero_EGF1_h_p1m1_p2300exe14", "pero_EGF1_h_p1m1_p2300exe15", "pero_EGF1_h_p1m1_p2300exe16", "pero_EGF1_h_p1m1_p2300exe17", "pero_EGF1_h_p1m1_p2300exe2", "pero_EGF1_h_p1m1_p2300exe3", "pero_EGF1_h_p1m1_p2300exe4", "pero_EGF1_h_p1m1_p2300exe5", "pero_EGF1_h_p1m1_p2300exe6", "pero_EGF1_h_p1m1_p2300exe7", "pero_EGF1_h_p1m1_p2300exe8", "pero_EGF1_h_p1m1_p2300exe9", "pero_EGF1_h_p1m1_p240000exe0", "pero_EGF1_h_p1m1_p240000exe1", "pero_EGF1_h_p1m1_p240000exe10", "pero_EGF1_h_p1m1_p240000exe11", "pero_EGF1_h_p1m1_p240000exe12", "pero_EGF1_h_p1m1_p240000exe13", "pero_EGF1_h_p1m1_p240000exe14", "pero_EGF1_h_p1m1_p240000exe15", "pero_EGF1_h_p1m1_p240000exe16", "pero_EGF1_h_p1m1_p240000exe2", "pero_EGF1_h_p1m1_p240000exe3", "pero_EGF1_h_p1m1_p240000exe4", "pero_EGF1_h_p1m1_p240000exe5", "pero_EGF1_h_p1m1_p240000exe6", "pero_EGF1_h_p1m1_p240000exe7", "pero_EGF1_h_p1m1_p240000exe8", "pero_EGF1_h_p1m1_p240000exe9", "pero_EGF1_h_p1m1_p2400exe0", "pero_EGF1_h_p1m1_p2400exe1", "pero_EGF1_h_p1m1_p2400exe10", "pero_EGF1_h_p1m1_p2400exe11", "pero_EGF1_h_p1m1_p2400exe12", "pero_EGF1_h_p1m1_p2400exe13", "pero_EGF1_h_p1m1_p2400exe14", "pero_EGF1_h_p1m1_p2400exe15", "pero_EGF1_h_p1m1_p2400exe16", "pero_EGF1_h_p1m1_p2400exe2", "pero_EGF1_h_p1m1_p2400exe3", "pero_EGF1_h_p1m1_p2400exe4", "pero_EGF1_h_p1m1_p2400exe5", "pero_EGF1_h_p1m1_p2400exe6", "pero_EGF1_h_p1m1_p2400exe7", "pero_EGF1_h_p1m1_p2400exe8", "pero_EGF1_h_p1m1_p2400exe9", "pero_EGF1_h_p1m1_p2500exe0", "pero_EGF1_h_p1m1_p2500exe1", "pero_EGF1_h_p1m1_p2500exe10", "pero_EGF1_h_p1m1_p2500exe11", "pero_EGF1_h_p1m1_p2500exe12", "pero_EGF1_h_p1m1_p2500exe13", "pero_EGF1_h_p1m1_p2500exe14", "pero_EGF1_h_p1m1_p2500exe15", "pero_EGF1_h_p1m1_p2500exe16", "pero_EGF1_h_p1m1_p2500exe2", "pero_EGF1_h_p1m1_p2500exe3", "pero_EGF1_h_p1m1_p2500exe4", "pero_EGF1_h_p1m1_p2500exe5", "pero_EGF1_h_p1m1_p2500exe6", "pero_EGF1_h_p1m1_p2500exe7", "pero_EGF1_h_p1m1_p2500exe8", "pero_EGF1_h_p1m1_p2500exe9", "pero_EGF1_h_p1m1_p260000exe0", "pero_EGF1_h_p1m1_p260000exe1", "pero_EGF1_h_p1m1_p260000exe10", "pero_EGF1_h_p1m1_p260000exe11", "pero_EGF1_h_p1m1_p260000exe12", "pero_EGF1_h_p1m1_p260000exe13", "pero_EGF1_h_p1m1_p260000exe14", "pero_EGF1_h_p1m1_p260000exe15", "pero_EGF1_h_p1m1_p260000exe16", "pero_EGF1_h_p1m1_p260000exe2", "pero_EGF1_h_p1m1_p260000exe3", "pero_EGF1_h_p1m1_p260000exe4", "pero_EGF1_h_p1m1_p260000exe5", "pero_EGF1_h_p1m1_p260000exe6", "pero_EGF1_h_p1m1_p260000exe7", "pero_EGF1_h_p1m1_p260000exe8", "pero_EGF1_h_p1m1_p260000exe9", "pero_EGF1_h_p1m1_p2600exe0", "pero_EGF1_h_p1m1_p2600exe1", "pero_EGF1_h_p1m1_p2600exe10", "pero_EGF1_h_p1m1_p2600exe11", "pero_EGF1_h_p1m1_p2600exe12", "pero_EGF1_h_p1m1_p2600exe13", "pero_EGF1_h_p1m1_p2600exe14", "pero_EGF1_h_p1m1_p2600exe15", "pero_EGF1_h_p1m1_p2600exe16", "pero_EGF1_h_p1m1_p2600exe2", "pero_EGF1_h_p1m1_p2600exe3", "pero_EGF1_h_p1m1_p2600exe4", "pero_EGF1_h_p1m1_p2600exe5", "pero_EGF1_h_p1m1_p2600exe6", "pero_EGF1_h_p1m1_p2600exe7", "pero_EGF1_h_p1m1_p2600exe8", "pero_EGF1_h_p1m1_p2600exe9", "pero_EGF1_h_p1m1_p2700exe0", "pero_EGF1_h_p1m1_p2700exe1", "pero_EGF1_h_p1m1_p2700exe10", "pero_EGF1_h_p1m1_p2700exe11", "pero_EGF1_h_p1m1_p2700exe12", "pero_EGF1_h_p1m1_p2700exe13", "pero_EGF1_h_p1m1_p2700exe14", "pero_EGF1_h_p1m1_p2700exe15", "pero_EGF1_h_p1m1_p2700exe16", "pero_EGF1_h_p1m1_p2700exe2", "pero_EGF1_h_p1m1_p2700exe3", "pero_EGF1_h_p1m1_p2700exe4", "pero_EGF1_h_p1m1_p2700exe5", "pero_EGF1_h_p1m1_p2700exe6", "pero_EGF1_h_p1m1_p2700exe7", "pero_EGF1_h_p1m1_p2700exe8", "pero_EGF1_h_p1m1_p2700exe9", "pero_EGF1_h_p1m1_p280000exe0", "pero_EGF1_h_p1m1_p280000exe1", "pero_EGF1_h_p1m1_p280000exe10", "pero_EGF1_h_p1m1_p280000exe11", "pero_EGF1_h_p1m1_p280000exe12", "pero_EGF1_h_p1m1_p280000exe13", "pero_EGF1_h_p1m1_p280000exe14", "pero_EGF1_h_p1m1_p280000exe15", "pero_EGF1_h_p1m1_p280000exe16", "pero_EGF1_h_p1m1_p280000exe2", "pero_EGF1_h_p1m1_p280000exe3", "pero_EGF1_h_p1m1_p280000exe4", "pero_EGF1_h_p1m1_p280000exe5", "pero_EGF1_h_p1m1_p280000exe6", "pero_EGF1_h_p1m1_p280000exe7", "pero_EGF1_h_p1m1_p280000exe8", "pero_EGF1_h_p1m1_p280000exe9", "pero_EGF1_h_p1m1_p2800exe0", "pero_EGF1_h_p1m1_p2800exe1", "pero_EGF1_h_p1m1_p2800exe10", "pero_EGF1_h_p1m1_p2800exe11", "pero_EGF1_h_p1m1_p2800exe12", "pero_EGF1_h_p1m1_p2800exe13", "pero_EGF1_h_p1m1_p2800exe14", "pero_EGF1_h_p1m1_p2800exe15", "pero_EGF1_h_p1m1_p2800exe16", "pero_EGF1_h_p1m1_p2800exe2", "pero_EGF1_h_p1m1_p2800exe3", "pero_EGF1_h_p1m1_p2800exe4", "pero_EGF1_h_p1m1_p2800exe5", "pero_EGF1_h_p1m1_p2800exe6", "pero_EGF1_h_p1m1_p2800exe7", "pero_EGF1_h_p1m1_p2800exe8", "pero_EGF1_h_p1m1_p2800exe9", "pero_EGF1_h_p1m1_p2900exe0", "pero_EGF1_h_p1m1_p2900exe1", "pero_EGF1_h_p1m1_p2900exe10", "pero_EGF1_h_p1m1_p2900exe11", "pero_EGF1_h_p1m1_p2900exe12", "pero_EGF1_h_p1m1_p2900exe13", "pero_EGF1_h_p1m1_p2900exe14", "pero_EGF1_h_p1m1_p2900exe15", "pero_EGF1_h_p1m1_p2900exe16", "pero_EGF1_h_p1m1_p2900exe2", "pero_EGF1_h_p1m1_p2900exe3", "pero_EGF1_h_p1m1_p2900exe4", "pero_EGF1_h_p1m1_p2900exe5", "pero_EGF1_h_p1m1_p2900exe6", "pero_EGF1_h_p1m1_p2900exe7", "pero_EGF1_h_p1m1_p2900exe8", "pero_EGF1_h_p1m1_p2900exe9", "pero_EGF1_h_p1m1_p300000exe0", "pero_EGF1_h_p1m1_p300000exe1", "pero_EGF1_h_p1m1_p300000exe10", "pero_EGF1_h_p1m1_p300000exe11", "pero_EGF1_h_p1m1_p300000exe12", "pero_EGF1_h_p1m1_p300000exe13", "pero_EGF1_h_p1m1_p300000exe14", "pero_EGF1_h_p1m1_p300000exe15", "pero_EGF1_h_p1m1_p300000exe16", "pero_EGF1_h_p1m1_p300000exe2", "pero_EGF1_h_p1m1_p300000exe3", "pero_EGF1_h_p1m1_p300000exe4", "pero_EGF1_h_p1m1_p300000exe5", "pero_EGF1_h_p1m1_p300000exe6", "pero_EGF1_h_p1m1_p300000exe7", "pero_EGF1_h_p1m1_p300000exe8", "pero_EGF1_h_p1m1_p300000exe9", "pero_EGF1_h_p1m1_p30000exe0", "pero_EGF1_h_p1m1_p30000exe1", "pero_EGF1_h_p1m1_p30000exe10", "pero_EGF1_h_p1m1_p30000exe11", "pero_EGF1_h_p1m1_p30000exe12", "pero_EGF1_h_p1m1_p30000exe13", "pero_EGF1_h_p1m1_p30000exe14", "pero_EGF1_h_p1m1_p30000exe15", "pero_EGF1_h_p1m1_p30000exe16", "pero_EGF1_h_p1m1_p30000exe2", "pero_EGF1_h_p1m1_p30000exe3", "pero_EGF1_h_p1m1_p30000exe4", "pero_EGF1_h_p1m1_p30000exe5", "pero_EGF1_h_p1m1_p30000exe6", "pero_EGF1_h_p1m1_p30000exe7", "pero_EGF1_h_p1m1_p30000exe8", "pero_EGF1_h_p1m1_p30000exe9", "pero_EGF1_h_p1m1_p3000exe0", "pero_EGF1_h_p1m1_p3000exe1", "pero_EGF1_h_p1m1_p3000exe10", "pero_EGF1_h_p1m1_p3000exe11", "pero_EGF1_h_p1m1_p3000exe12", "pero_EGF1_h_p1m1_p3000exe13", "pero_EGF1_h_p1m1_p3000exe14", "pero_EGF1_h_p1m1_p3000exe15", "pero_EGF1_h_p1m1_p3000exe16", "pero_EGF1_h_p1m1_p3000exe17", "pero_EGF1_h_p1m1_p3000exe2", "pero_EGF1_h_p1m1_p3000exe3", "pero_EGF1_h_p1m1_p3000exe4", "pero_EGF1_h_p1m1_p3000exe5", "pero_EGF1_h_p1m1_p3000exe6", "pero_EGF1_h_p1m1_p3000exe7", "pero_EGF1_h_p1m1_p3000exe8", "pero_EGF1_h_p1m1_p3000exe9", "pero_EGF1_h_p1m1_p300exe0", "pero_EGF1_h_p1m1_p300exe1", "pero_EGF1_h_p1m1_p300exe10", "pero_EGF1_h_p1m1_p300exe11", "pero_EGF1_h_p1m1_p300exe12", "pero_EGF1_h_p1m1_p300exe13", "pero_EGF1_h_p1m1_p300exe14", "pero_EGF1_h_p1m1_p300exe15", "pero_EGF1_h_p1m1_p300exe16", "pero_EGF1_h_p1m1_p300exe2", "pero_EGF1_h_p1m1_p300exe3", "pero_EGF1_h_p1m1_p300exe4", "pero_EGF1_h_p1m1_p300exe5", "pero_EGF1_h_p1m1_p300exe6", "pero_EGF1_h_p1m1_p300exe7", "pero_EGF1_h_p1m1_p300exe8", "pero_EGF1_h_p1m1_p300exe9", "pero_EGF1_h_p1m1_p320000exe0", "pero_EGF1_h_p1m1_p320000exe1", "pero_EGF1_h_p1m1_p320000exe10", "pero_EGF1_h_p1m1_p320000exe11", "pero_EGF1_h_p1m1_p320000exe12", "pero_EGF1_h_p1m1_p320000exe13", "pero_EGF1_h_p1m1_p320000exe14", "pero_EGF1_h_p1m1_p320000exe15", "pero_EGF1_h_p1m1_p320000exe16", "pero_EGF1_h_p1m1_p320000exe2", "pero_EGF1_h_p1m1_p320000exe3", "pero_EGF1_h_p1m1_p320000exe4", "pero_EGF1_h_p1m1_p320000exe5", "pero_EGF1_h_p1m1_p320000exe6", "pero_EGF1_h_p1m1_p320000exe7", "pero_EGF1_h_p1m1_p320000exe8", "pero_EGF1_h_p1m1_p320000exe9", "pero_EGF1_h_p1m1_p340000exe0", "pero_EGF1_h_p1m1_p340000exe1", "pero_EGF1_h_p1m1_p340000exe10", "pero_EGF1_h_p1m1_p340000exe11", "pero_EGF1_h_p1m1_p340000exe12", "pero_EGF1_h_p1m1_p340000exe13", "pero_EGF1_h_p1m1_p340000exe14", "pero_EGF1_h_p1m1_p340000exe15", "pero_EGF1_h_p1m1_p340000exe16", "pero_EGF1_h_p1m1_p340000exe2", "pero_EGF1_h_p1m1_p340000exe3", "pero_EGF1_h_p1m1_p340000exe4", "pero_EGF1_h_p1m1_p340000exe5", "pero_EGF1_h_p1m1_p340000exe6", "pero_EGF1_h_p1m1_p340000exe7", "pero_EGF1_h_p1m1_p340000exe8", "pero_EGF1_h_p1m1_p340000exe9", "pero_EGF1_h_p1m1_p360000exe0", "pero_EGF1_h_p1m1_p360000exe1", "pero_EGF1_h_p1m1_p360000exe10", "pero_EGF1_h_p1m1_p360000exe11", "pero_EGF1_h_p1m1_p360000exe12", "pero_EGF1_h_p1m1_p360000exe13", "pero_EGF1_h_p1m1_p360000exe14", "pero_EGF1_h_p1m1_p360000exe15", "pero_EGF1_h_p1m1_p360000exe16", "pero_EGF1_h_p1m1_p360000exe2", "pero_EGF1_h_p1m1_p360000exe3", "pero_EGF1_h_p1m1_p360000exe4", "pero_EGF1_h_p1m1_p360000exe5", "pero_EGF1_h_p1m1_p360000exe6", "pero_EGF1_h_p1m1_p360000exe7", "pero_EGF1_h_p1m1_p360000exe8", "pero_EGF1_h_p1m1_p360000exe9", "pero_EGF1_h_p1m1_p380000exe0", "pero_EGF1_h_p1m1_p380000exe1", "pero_EGF1_h_p1m1_p380000exe10", "pero_EGF1_h_p1m1_p380000exe11", "pero_EGF1_h_p1m1_p380000exe12", "pero_EGF1_h_p1m1_p380000exe13", "pero_EGF1_h_p1m1_p380000exe14", "pero_EGF1_h_p1m1_p380000exe15", "pero_EGF1_h_p1m1_p380000exe16", "pero_EGF1_h_p1m1_p380000exe2", "pero_EGF1_h_p1m1_p380000exe3", "pero_EGF1_h_p1m1_p380000exe4", "pero_EGF1_h_p1m1_p380000exe5", "pero_EGF1_h_p1m1_p380000exe6", "pero_EGF1_h_p1m1_p380000exe7", "pero_EGF1_h_p1m1_p380000exe8", "pero_EGF1_h_p1m1_p380000exe9", "pero_EGF1_h_p1m1_p400000exe0", "pero_EGF1_h_p1m1_p400000exe1", "pero_EGF1_h_p1m1_p400000exe10", "pero_EGF1_h_p1m1_p400000exe11", "pero_EGF1_h_p1m1_p400000exe12", "pero_EGF1_h_p1m1_p400000exe13", "pero_EGF1_h_p1m1_p400000exe14", "pero_EGF1_h_p1m1_p400000exe15", "pero_EGF1_h_p1m1_p400000exe16", "pero_EGF1_h_p1m1_p400000exe2", "pero_EGF1_h_p1m1_p400000exe3", "pero_EGF1_h_p1m1_p400000exe4", "pero_EGF1_h_p1m1_p400000exe5", "pero_EGF1_h_p1m1_p400000exe6", "pero_EGF1_h_p1m1_p400000exe7", "pero_EGF1_h_p1m1_p400000exe8", "pero_EGF1_h_p1m1_p400000exe9", "pero_EGF1_h_p1m1_p40000exe0", "pero_EGF1_h_p1m1_p40000exe1", "pero_EGF1_h_p1m1_p40000exe10", "pero_EGF1_h_p1m1_p40000exe11", "pero_EGF1_h_p1m1_p40000exe12", "pero_EGF1_h_p1m1_p40000exe13", "pero_EGF1_h_p1m1_p40000exe14", "pero_EGF1_h_p1m1_p40000exe15", "pero_EGF1_h_p1m1_p40000exe16", "pero_EGF1_h_p1m1_p40000exe2", "pero_EGF1_h_p1m1_p40000exe3", "pero_EGF1_h_p1m1_p40000exe4", "pero_EGF1_h_p1m1_p40000exe5", "pero_EGF1_h_p1m1_p40000exe6", "pero_EGF1_h_p1m1_p40000exe7", "pero_EGF1_h_p1m1_p40000exe8", "pero_EGF1_h_p1m1_p40000exe9", "pero_EGF1_h_p1m1_p4000exe0", "pero_EGF1_h_p1m1_p4000exe1", "pero_EGF1_h_p1m1_p4000exe10", "pero_EGF1_h_p1m1_p4000exe11", "pero_EGF1_h_p1m1_p4000exe12", "pero_EGF1_h_p1m1_p4000exe13", "pero_EGF1_h_p1m1_p4000exe14", "pero_EGF1_h_p1m1_p4000exe15", "pero_EGF1_h_p1m1_p4000exe16", "pero_EGF1_h_p1m1_p4000exe2", "pero_EGF1_h_p1m1_p4000exe3", "pero_EGF1_h_p1m1_p4000exe4", "pero_EGF1_h_p1m1_p4000exe5", "pero_EGF1_h_p1m1_p4000exe6", "pero_EGF1_h_p1m1_p4000exe7", "pero_EGF1_h_p1m1_p4000exe8", "pero_EGF1_h_p1m1_p4000exe9", "pero_EGF1_h_p1m1_p400exe0", "pero_EGF1_h_p1m1_p400exe1", "pero_EGF1_h_p1m1_p400exe10", "pero_EGF1_h_p1m1_p400exe11", "pero_EGF1_h_p1m1_p400exe12", "pero_EGF1_h_p1m1_p400exe13", "pero_EGF1_h_p1m1_p400exe14", "pero_EGF1_h_p1m1_p400exe15", "pero_EGF1_h_p1m1_p400exe16", "pero_EGF1_h_p1m1_p400exe2", "pero_EGF1_h_p1m1_p400exe3", "pero_EGF1_h_p1m1_p400exe4", "pero_EGF1_h_p1m1_p400exe5", "pero_EGF1_h_p1m1_p400exe6", "pero_EGF1_h_p1m1_p400exe7", "pero_EGF1_h_p1m1_p400exe8", "pero_EGF1_h_p1m1_p400exe9", "pero_EGF1_h_p1m1_p420000exe0", "pero_EGF1_h_p1m1_p420000exe1", "pero_EGF1_h_p1m1_p420000exe10", "pero_EGF1_h_p1m1_p420000exe11", "pero_EGF1_h_p1m1_p420000exe12", "pero_EGF1_h_p1m1_p420000exe13", "pero_EGF1_h_p1m1_p420000exe14", "pero_EGF1_h_p1m1_p420000exe15", "pero_EGF1_h_p1m1_p420000exe16", "pero_EGF1_h_p1m1_p420000exe2", "pero_EGF1_h_p1m1_p420000exe3", "pero_EGF1_h_p1m1_p420000exe4", "pero_EGF1_h_p1m1_p420000exe5", "pero_EGF1_h_p1m1_p420000exe6", "pero_EGF1_h_p1m1_p420000exe7", "pero_EGF1_h_p1m1_p420000exe8", "pero_EGF1_h_p1m1_p420000exe9", "pero_EGF1_h_p1m1_p440000exe0", "pero_EGF1_h_p1m1_p440000exe1", "pero_EGF1_h_p1m1_p440000exe10", "pero_EGF1_h_p1m1_p440000exe11", "pero_EGF1_h_p1m1_p440000exe12", "pero_EGF1_h_p1m1_p440000exe13", "pero_EGF1_h_p1m1_p440000exe14", "pero_EGF1_h_p1m1_p440000exe15", "pero_EGF1_h_p1m1_p440000exe16", "pero_EGF1_h_p1m1_p440000exe2", "pero_EGF1_h_p1m1_p440000exe3", "pero_EGF1_h_p1m1_p440000exe4", "pero_EGF1_h_p1m1_p440000exe5", "pero_EGF1_h_p1m1_p440000exe6", "pero_EGF1_h_p1m1_p440000exe7", "pero_EGF1_h_p1m1_p440000exe8", "pero_EGF1_h_p1m1_p440000exe9", "pero_EGF1_h_p1m1_p480000exe0", "pero_EGF1_h_p1m1_p480000exe1", "pero_EGF1_h_p1m1_p480000exe10", "pero_EGF1_h_p1m1_p480000exe11", "pero_EGF1_h_p1m1_p480000exe12", "pero_EGF1_h_p1m1_p480000exe13", "pero_EGF1_h_p1m1_p480000exe14", "pero_EGF1_h_p1m1_p480000exe15", "pero_EGF1_h_p1m1_p480000exe16", "pero_EGF1_h_p1m1_p480000exe2", "pero_EGF1_h_p1m1_p480000exe3", "pero_EGF1_h_p1m1_p480000exe4", "pero_EGF1_h_p1m1_p480000exe5", "pero_EGF1_h_p1m1_p480000exe6", "pero_EGF1_h_p1m1_p480000exe7", "pero_EGF1_h_p1m1_p480000exe8", "pero_EGF1_h_p1m1_p480000exe9", "pero_EGF1_h_p1m1_p500000exe0", "pero_EGF1_h_p1m1_p500000exe1", "pero_EGF1_h_p1m1_p500000exe10", "pero_EGF1_h_p1m1_p500000exe11", "pero_EGF1_h_p1m1_p500000exe12", "pero_EGF1_h_p1m1_p500000exe13", "pero_EGF1_h_p1m1_p500000exe14", "pero_EGF1_h_p1m1_p500000exe15", "pero_EGF1_h_p1m1_p500000exe16", "pero_EGF1_h_p1m1_p500000exe2", "pero_EGF1_h_p1m1_p500000exe3", "pero_EGF1_h_p1m1_p500000exe4", "pero_EGF1_h_p1m1_p500000exe5", "pero_EGF1_h_p1m1_p500000exe6", "pero_EGF1_h_p1m1_p500000exe7", "pero_EGF1_h_p1m1_p500000exe8", "pero_EGF1_h_p1m1_p500000exe9", "pero_EGF1_h_p1m1_p50000exe0", "pero_EGF1_h_p1m1_p50000exe1", "pero_EGF1_h_p1m1_p50000exe10", "pero_EGF1_h_p1m1_p50000exe11", "pero_EGF1_h_p1m1_p50000exe12", "pero_EGF1_h_p1m1_p50000exe13", "pero_EGF1_h_p1m1_p50000exe14", "pero_EGF1_h_p1m1_p50000exe15", "pero_EGF1_h_p1m1_p50000exe16", "pero_EGF1_h_p1m1_p50000exe2", "pero_EGF1_h_p1m1_p50000exe3", "pero_EGF1_h_p1m1_p50000exe4", "pero_EGF1_h_p1m1_p50000exe5", "pero_EGF1_h_p1m1_p50000exe6", "pero_EGF1_h_p1m1_p50000exe7", "pero_EGF1_h_p1m1_p50000exe8", "pero_EGF1_h_p1m1_p50000exe9", "pero_EGF1_h_p1m1_p500exe0", "pero_EGF1_h_p1m1_p500exe1", "pero_EGF1_h_p1m1_p500exe10", "pero_EGF1_h_p1m1_p500exe11", "pero_EGF1_h_p1m1_p500exe12", "pero_EGF1_h_p1m1_p500exe13", "pero_EGF1_h_p1m1_p500exe14", "pero_EGF1_h_p1m1_p500exe15", "pero_EGF1_h_p1m1_p500exe16", "pero_EGF1_h_p1m1_p500exe2", "pero_EGF1_h_p1m1_p500exe3", "pero_EGF1_h_p1m1_p500exe4", "pero_EGF1_h_p1m1_p500exe5", "pero_EGF1_h_p1m1_p500exe6", "pero_EGF1_h_p1m1_p500exe7", "pero_EGF1_h_p1m1_p500exe8", "pero_EGF1_h_p1m1_p500exe9", "pero_EGF1_h_p1m1_p60000exe0", "pero_EGF1_h_p1m1_p60000exe1", "pero_EGF1_h_p1m1_p60000exe10", "pero_EGF1_h_p1m1_p60000exe11", "pero_EGF1_h_p1m1_p60000exe12", "pero_EGF1_h_p1m1_p60000exe13", "pero_EGF1_h_p1m1_p60000exe14", "pero_EGF1_h_p1m1_p60000exe15", "pero_EGF1_h_p1m1_p60000exe16", "pero_EGF1_h_p1m1_p60000exe2", "pero_EGF1_h_p1m1_p60000exe3", "pero_EGF1_h_p1m1_p60000exe4", "pero_EGF1_h_p1m1_p60000exe5", "pero_EGF1_h_p1m1_p60000exe6", "pero_EGF1_h_p1m1_p60000exe7", "pero_EGF1_h_p1m1_p60000exe8", "pero_EGF1_h_p1m1_p60000exe9", "pero_EGF1_h_p1m1_p6000exe0", "pero_EGF1_h_p1m1_p6000exe1", "pero_EGF1_h_p1m1_p6000exe10", "pero_EGF1_h_p1m1_p6000exe11", "pero_EGF1_h_p1m1_p6000exe12", "pero_EGF1_h_p1m1_p6000exe13", "pero_EGF1_h_p1m1_p6000exe14", "pero_EGF1_h_p1m1_p6000exe15", "pero_EGF1_h_p1m1_p6000exe16", "pero_EGF1_h_p1m1_p6000exe2", "pero_EGF1_h_p1m1_p6000exe3", "pero_EGF1_h_p1m1_p6000exe4", "pero_EGF1_h_p1m1_p6000exe5", "pero_EGF1_h_p1m1_p6000exe6", "pero_EGF1_h_p1m1_p6000exe7", "pero_EGF1_h_p1m1_p6000exe8", "pero_EGF1_h_p1m1_p6000exe9", "pero_EGF1_h_p1m1_p600exe0", "pero_EGF1_h_p1m1_p600exe1", "pero_EGF1_h_p1m1_p600exe10", "pero_EGF1_h_p1m1_p600exe11", "pero_EGF1_h_p1m1_p600exe12", "pero_EGF1_h_p1m1_p600exe13", "pero_EGF1_h_p1m1_p600exe14", "pero_EGF1_h_p1m1_p600exe15", "pero_EGF1_h_p1m1_p600exe16", "pero_EGF1_h_p1m1_p600exe17", "pero_EGF1_h_p1m1_p600exe2", "pero_EGF1_h_p1m1_p600exe3", "pero_EGF1_h_p1m1_p600exe4", "pero_EGF1_h_p1m1_p600exe5", "pero_EGF1_h_p1m1_p600exe6", "pero_EGF1_h_p1m1_p600exe7", "pero_EGF1_h_p1m1_p600exe8", "pero_EGF1_h_p1m1_p600exe9", "pero_EGF1_h_p1m1_p700exe0", "pero_EGF1_h_p1m1_p700exe1", "pero_EGF1_h_p1m1_p700exe10", "pero_EGF1_h_p1m1_p700exe11", "pero_EGF1_h_p1m1_p700exe12", "pero_EGF1_h_p1m1_p700exe13", "pero_EGF1_h_p1m1_p700exe14", "pero_EGF1_h_p1m1_p700exe15", "pero_EGF1_h_p1m1_p700exe16", "pero_EGF1_h_p1m1_p700exe2", "pero_EGF1_h_p1m1_p700exe3", "pero_EGF1_h_p1m1_p700exe4", "pero_EGF1_h_p1m1_p700exe5", "pero_EGF1_h_p1m1_p700exe6", "pero_EGF1_h_p1m1_p700exe7", "pero_EGF1_h_p1m1_p700exe8", "pero_EGF1_h_p1m1_p700exe9", "pero_EGF1_h_p1m1_p80000exe0", "pero_EGF1_h_p1m1_p80000exe1", "pero_EGF1_h_p1m1_p80000exe10", "pero_EGF1_h_p1m1_p80000exe11", "pero_EGF1_h_p1m1_p80000exe12", "pero_EGF1_h_p1m1_p80000exe13", "pero_EGF1_h_p1m1_p80000exe14", "pero_EGF1_h_p1m1_p80000exe15", "pero_EGF1_h_p1m1_p80000exe16", "pero_EGF1_h_p1m1_p80000exe2", "pero_EGF1_h_p1m1_p80000exe3", "pero_EGF1_h_p1m1_p80000exe4", "pero_EGF1_h_p1m1_p80000exe5", "pero_EGF1_h_p1m1_p80000exe6", "pero_EGF1_h_p1m1_p80000exe7", "pero_EGF1_h_p1m1_p80000exe8", "pero_EGF1_h_p1m1_p80000exe9", "pero_EGF1_h_p1m1_p800exe0", "pero_EGF1_h_p1m1_p800exe1", "pero_EGF1_h_p1m1_p800exe10", "pero_EGF1_h_p1m1_p800exe11", "pero_EGF1_h_p1m1_p800exe12", "pero_EGF1_h_p1m1_p800exe13", "pero_EGF1_h_p1m1_p800exe14", "pero_EGF1_h_p1m1_p800exe15", "pero_EGF1_h_p1m1_p800exe16", "pero_EGF1_h_p1m1_p800exe2", "pero_EGF1_h_p1m1_p800exe3", "pero_EGF1_h_p1m1_p800exe4", "pero_EGF1_h_p1m1_p800exe5", "pero_EGF1_h_p1m1_p800exe6", "pero_EGF1_h_p1m1_p800exe7", "pero_EGF1_h_p1m1_p800exe8", "pero_EGF1_h_p1m1_p800exe9", "pero_EGF1_h_p1m1_p900exe0", "pero_EGF1_h_p1m1_p900exe1", "pero_EGF1_h_p1m1_p900exe10", "pero_EGF1_h_p1m1_p900exe11", "pero_EGF1_h_p1m1_p900exe12", "pero_EGF1_h_p1m1_p900exe13", "pero_EGF1_h_p1m1_p900exe14", "pero_EGF1_h_p1m1_p900exe15", "pero_EGF1_h_p1m1_p900exe16", "pero_EGF1_h_p1m1_p900exe2", "pero_EGF1_h_p1m1_p900exe3", "pero_EGF1_h_p1m1_p900exe4", "pero_EGF1_h_p1m1_p900exe5", "pero_EGF1_h_p1m1_p900exe6", "pero_EGF1_h_p1m1_p900exe7", "pero_EGF1_h_p1m1_p900exe8", "pero_EGF1_h_p1m1_p900exe9", "pero_EGF1_h_p1p0_m0exe0", "pero_EGF1_h_p1p0_m0exe1", "pero_EGF1_h_p1p0_m0exe10", "pero_EGF1_h_p1p0_m0exe11", "pero_EGF1_h_p1p0_m0exe12", "pero_EGF1_h_p1p0_m0exe13", "pero_EGF1_h_p1p0_m0exe14", "pero_EGF1_h_p1p0_m0exe15", "pero_EGF1_h_p1p0_m0exe16", "pero_EGF1_h_p1p0_m0exe2", "pero_EGF1_h_p1p0_m0exe3", "pero_EGF1_h_p1p0_m0exe4", "pero_EGF1_h_p1p0_m0exe5", "pero_EGF1_h_p1p0_m0exe6", "pero_EGF1_h_p1p0_m0exe7", "pero_EGF1_h_p1p0_m0exe8", "pero_EGF1_h_p1p0_m0exe9", "pero_EGF1_h_p1p0_m100exe0", "pero_EGF1_h_p1p0_m100exe1", "pero_EGF1_h_p1p0_m100exe10", "pero_EGF1_h_p1p0_m100exe11", "pero_EGF1_h_p1p0_m100exe12", "pero_EGF1_h_p1p0_m100exe13", "pero_EGF1_h_p1p0_m100exe14", "pero_EGF1_h_p1p0_m100exe15", "pero_EGF1_h_p1p0_m100exe16", "pero_EGF1_h_p1p0_m100exe2", "pero_EGF1_h_p1p0_m100exe3", "pero_EGF1_h_p1p0_m100exe4", "pero_EGF1_h_p1p0_m100exe5", "pero_EGF1_h_p1p0_m100exe6", "pero_EGF1_h_p1p0_m100exe7", "pero_EGF1_h_p1p0_m100exe8", "pero_EGF1_h_p1p0_m100exe9", "pero_EGF1_h_p1p0_m200exe0", "pero_EGF1_h_p1p0_m200exe1", "pero_EGF1_h_p1p0_m200exe10", "pero_EGF1_h_p1p0_m200exe11", "pero_EGF1_h_p1p0_m200exe12", "pero_EGF1_h_p1p0_m200exe13", "pero_EGF1_h_p1p0_m200exe14", "pero_EGF1_h_p1p0_m200exe15", "pero_EGF1_h_p1p0_m200exe16", "pero_EGF1_h_p1p0_m200exe2", "pero_EGF1_h_p1p0_m200exe3", "pero_EGF1_h_p1p0_m200exe4", "pero_EGF1_h_p1p0_m200exe5", "pero_EGF1_h_p1p0_m200exe6", "pero_EGF1_h_p1p0_m200exe7", "pero_EGF1_h_p1p0_m200exe8", "pero_EGF1_h_p1p0_m200exe9", "pero_EGF1_h_p1p0_m300exe0", "pero_EGF1_h_p1p0_m300exe1", "pero_EGF1_h_p1p0_m300exe10", "pero_EGF1_h_p1p0_m300exe11", "pero_EGF1_h_p1p0_m300exe12", "pero_EGF1_h_p1p0_m300exe13", "pero_EGF1_h_p1p0_m300exe14", "pero_EGF1_h_p1p0_m300exe15", "pero_EGF1_h_p1p0_m300exe16", "pero_EGF1_h_p1p0_m300exe2", "pero_EGF1_h_p1p0_m300exe3", "pero_EGF1_h_p1p0_m300exe4", "pero_EGF1_h_p1p0_m300exe5", "pero_EGF1_h_p1p0_m300exe6", "pero_EGF1_h_p1p0_m300exe7", "pero_EGF1_h_p1p0_m300exe8", "pero_EGF1_h_p1p0_m300exe9", "pero_EGF1_h_p1p0_m5000exe0", "pero_EGF1_h_p1p0_m5000exe1", "pero_EGF1_h_p1p0_m5000exe10", "pero_EGF1_h_p1p0_m5000exe11", "pero_EGF1_h_p1p0_m5000exe12", "pero_EGF1_h_p1p0_m5000exe13", "pero_EGF1_h_p1p0_m5000exe14", "pero_EGF1_h_p1p0_m5000exe15", "pero_EGF1_h_p1p0_m5000exe16", "pero_EGF1_h_p1p0_m5000exe2", "pero_EGF1_h_p1p0_m5000exe3", "pero_EGF1_h_p1p0_m5000exe4", "pero_EGF1_h_p1p0_m5000exe5", "pero_EGF1_h_p1p0_m5000exe6", "pero_EGF1_h_p1p0_m5000exe7", "pero_EGF1_h_p1p0_m5000exe8", "pero_EGF1_h_p1p0_m5000exe9", "pero_EGF1_h_p1p0_m500exe0", "pero_EGF1_h_p1p0_m500exe1", "pero_EGF1_h_p1p0_m500exe10", "pero_EGF1_h_p1p0_m500exe11", "pero_EGF1_h_p1p0_m500exe12", "pero_EGF1_h_p1p0_m500exe13", "pero_EGF1_h_p1p0_m500exe14", "pero_EGF1_h_p1p0_m500exe15", "pero_EGF1_h_p1p0_m500exe16", "pero_EGF1_h_p1p0_m500exe2", "pero_EGF1_h_p1p0_m500exe3", "pero_EGF1_h_p1p0_m500exe4", "pero_EGF1_h_p1p0_m500exe5", "pero_EGF1_h_p1p0_m500exe6", "pero_EGF1_h_p1p0_m500exe7", "pero_EGF1_h_p1p0_m500exe8", "pero_EGF1_h_p1p0_m500exe9", "pero_EGF1_h_p1p0_p100000exe0", "pero_EGF1_h_p1p0_p100000exe1", "pero_EGF1_h_p1p0_p100000exe10", "pero_EGF1_h_p1p0_p100000exe11", "pero_EGF1_h_p1p0_p100000exe12", "pero_EGF1_h_p1p0_p100000exe13", "pero_EGF1_h_p1p0_p100000exe14", "pero_EGF1_h_p1p0_p100000exe15", "pero_EGF1_h_p1p0_p100000exe16", "pero_EGF1_h_p1p0_p100000exe2", "pero_EGF1_h_p1p0_p100000exe3", "pero_EGF1_h_p1p0_p100000exe4", "pero_EGF1_h_p1p0_p100000exe5", "pero_EGF1_h_p1p0_p100000exe6", "pero_EGF1_h_p1p0_p100000exe7", "pero_EGF1_h_p1p0_p100000exe8", "pero_EGF1_h_p1p0_p100000exe9", "pero_EGF1_h_p1p0_p10000exe0", "pero_EGF1_h_p1p0_p10000exe1", "pero_EGF1_h_p1p0_p10000exe10", "pero_EGF1_h_p1p0_p10000exe11", "pero_EGF1_h_p1p0_p10000exe12", "pero_EGF1_h_p1p0_p10000exe13", "pero_EGF1_h_p1p0_p10000exe14", "pero_EGF1_h_p1p0_p10000exe15", "pero_EGF1_h_p1p0_p10000exe16", "pero_EGF1_h_p1p0_p10000exe2", "pero_EGF1_h_p1p0_p10000exe3", "pero_EGF1_h_p1p0_p10000exe4", "pero_EGF1_h_p1p0_p10000exe5", "pero_EGF1_h_p1p0_p10000exe6", "pero_EGF1_h_p1p0_p10000exe7", "pero_EGF1_h_p1p0_p10000exe8", "pero_EGF1_h_p1p0_p10000exe9", "pero_EGF1_h_p1p0_p1000exe0", "pero_EGF1_h_p1p0_p1000exe1", "pero_EGF1_h_p1p0_p1000exe10", "pero_EGF1_h_p1p0_p1000exe11", "pero_EGF1_h_p1p0_p1000exe12", "pero_EGF1_h_p1p0_p1000exe13", "pero_EGF1_h_p1p0_p1000exe14", "pero_EGF1_h_p1p0_p1000exe15", "pero_EGF1_h_p1p0_p1000exe16", "pero_EGF1_h_p1p0_p1000exe17", "pero_EGF1_h_p1p0_p1000exe2", "pero_EGF1_h_p1p0_p1000exe3", "pero_EGF1_h_p1p0_p1000exe4", "pero_EGF1_h_p1p0_p1000exe5", "pero_EGF1_h_p1p0_p1000exe6", "pero_EGF1_h_p1p0_p1000exe7", "pero_EGF1_h_p1p0_p1000exe8", "pero_EGF1_h_p1p0_p1000exe9", "pero_EGF1_h_p1p0_p100exe0", "pero_EGF1_h_p1p0_p100exe1", "pero_EGF1_h_p1p0_p100exe10", "pero_EGF1_h_p1p0_p100exe11", "pero_EGF1_h_p1p0_p100exe12", "pero_EGF1_h_p1p0_p100exe13", "pero_EGF1_h_p1p0_p100exe14", "pero_EGF1_h_p1p0_p100exe15", "pero_EGF1_h_p1p0_p100exe16", "pero_EGF1_h_p1p0_p100exe2", "pero_EGF1_h_p1p0_p100exe3", "pero_EGF1_h_p1p0_p100exe4", "pero_EGF1_h_p1p0_p100exe5", "pero_EGF1_h_p1p0_p100exe6", "pero_EGF1_h_p1p0_p100exe7", "pero_EGF1_h_p1p0_p100exe8", "pero_EGF1_h_p1p0_p100exe9", "pero_EGF1_h_p1p0_p1100exe0", "pero_EGF1_h_p1p0_p1100exe1", "pero_EGF1_h_p1p0_p1100exe10", "pero_EGF1_h_p1p0_p1100exe11", "pero_EGF1_h_p1p0_p1100exe12", "pero_EGF1_h_p1p0_p1100exe13", "pero_EGF1_h_p1p0_p1100exe14", "pero_EGF1_h_p1p0_p1100exe15", "pero_EGF1_h_p1p0_p1100exe16", "pero_EGF1_h_p1p0_p1100exe2", "pero_EGF1_h_p1p0_p1100exe3", "pero_EGF1_h_p1p0_p1100exe4", "pero_EGF1_h_p1p0_p1100exe5", "pero_EGF1_h_p1p0_p1100exe6", "pero_EGF1_h_p1p0_p1100exe7", "pero_EGF1_h_p1p0_p1100exe8", "pero_EGF1_h_p1p0_p1100exe9", "pero_EGF1_h_p1p0_p120000exe0", "pero_EGF1_h_p1p0_p120000exe1", "pero_EGF1_h_p1p0_p120000exe10", "pero_EGF1_h_p1p0_p120000exe11", "pero_EGF1_h_p1p0_p120000exe12", "pero_EGF1_h_p1p0_p120000exe13", "pero_EGF1_h_p1p0_p120000exe14", "pero_EGF1_h_p1p0_p120000exe15", "pero_EGF1_h_p1p0_p120000exe16", "pero_EGF1_h_p1p0_p120000exe2", "pero_EGF1_h_p1p0_p120000exe3", "pero_EGF1_h_p1p0_p120000exe4", "pero_EGF1_h_p1p0_p120000exe5", "pero_EGF1_h_p1p0_p120000exe6", "pero_EGF1_h_p1p0_p120000exe7", "pero_EGF1_h_p1p0_p120000exe8", "pero_EGF1_h_p1p0_p120000exe9", "pero_EGF1_h_p1p0_p1200exe0", "pero_EGF1_h_p1p0_p1200exe1", "pero_EGF1_h_p1p0_p1200exe10", "pero_EGF1_h_p1p0_p1200exe11", "pero_EGF1_h_p1p0_p1200exe12", "pero_EGF1_h_p1p0_p1200exe13", "pero_EGF1_h_p1p0_p1200exe14", "pero_EGF1_h_p1p0_p1200exe15", "pero_EGF1_h_p1p0_p1200exe16", "pero_EGF1_h_p1p0_p1200exe2", "pero_EGF1_h_p1p0_p1200exe3", "pero_EGF1_h_p1p0_p1200exe4", "pero_EGF1_h_p1p0_p1200exe5", "pero_EGF1_h_p1p0_p1200exe6", "pero_EGF1_h_p1p0_p1200exe7", "pero_EGF1_h_p1p0_p1200exe8", "pero_EGF1_h_p1p0_p1200exe9", "pero_EGF1_h_p1p0_p1300exe0", "pero_EGF1_h_p1p0_p1300exe1", "pero_EGF1_h_p1p0_p1300exe10", "pero_EGF1_h_p1p0_p1300exe11", "pero_EGF1_h_p1p0_p1300exe12", "pero_EGF1_h_p1p0_p1300exe13", "pero_EGF1_h_p1p0_p1300exe14", "pero_EGF1_h_p1p0_p1300exe15", "pero_EGF1_h_p1p0_p1300exe16", "pero_EGF1_h_p1p0_p1300exe2", "pero_EGF1_h_p1p0_p1300exe3", "pero_EGF1_h_p1p0_p1300exe4", "pero_EGF1_h_p1p0_p1300exe5", "pero_EGF1_h_p1p0_p1300exe6", "pero_EGF1_h_p1p0_p1300exe7", "pero_EGF1_h_p1p0_p1300exe8", "pero_EGF1_h_p1p0_p1300exe9", "pero_EGF1_h_p1p0_p140000exe0", "pero_EGF1_h_p1p0_p140000exe1", "pero_EGF1_h_p1p0_p140000exe10", "pero_EGF1_h_p1p0_p140000exe11", "pero_EGF1_h_p1p0_p140000exe12", "pero_EGF1_h_p1p0_p140000exe13", "pero_EGF1_h_p1p0_p140000exe14", "pero_EGF1_h_p1p0_p140000exe15", "pero_EGF1_h_p1p0_p140000exe16", "pero_EGF1_h_p1p0_p140000exe2", "pero_EGF1_h_p1p0_p140000exe3", "pero_EGF1_h_p1p0_p140000exe4", "pero_EGF1_h_p1p0_p140000exe5", "pero_EGF1_h_p1p0_p140000exe6", "pero_EGF1_h_p1p0_p140000exe7", "pero_EGF1_h_p1p0_p140000exe8", "pero_EGF1_h_p1p0_p140000exe9", "pero_EGF1_h_p1p0_p1400exe0", "pero_EGF1_h_p1p0_p1400exe1", "pero_EGF1_h_p1p0_p1400exe10", "pero_EGF1_h_p1p0_p1400exe11", "pero_EGF1_h_p1p0_p1400exe12", "pero_EGF1_h_p1p0_p1400exe13", "pero_EGF1_h_p1p0_p1400exe14", "pero_EGF1_h_p1p0_p1400exe15", "pero_EGF1_h_p1p0_p1400exe16", "pero_EGF1_h_p1p0_p1400exe2", "pero_EGF1_h_p1p0_p1400exe3", "pero_EGF1_h_p1p0_p1400exe4", "pero_EGF1_h_p1p0_p1400exe5", "pero_EGF1_h_p1p0_p1400exe6", "pero_EGF1_h_p1p0_p1400exe7", "pero_EGF1_h_p1p0_p1400exe8", "pero_EGF1_h_p1p0_p1400exe9", "pero_EGF1_h_p1p0_p1500exe0", "pero_EGF1_h_p1p0_p1500exe1", "pero_EGF1_h_p1p0_p1500exe10", "pero_EGF1_h_p1p0_p1500exe11", "pero_EGF1_h_p1p0_p1500exe12", "pero_EGF1_h_p1p0_p1500exe13", "pero_EGF1_h_p1p0_p1500exe14", "pero_EGF1_h_p1p0_p1500exe15", "pero_EGF1_h_p1p0_p1500exe16", "pero_EGF1_h_p1p0_p1500exe2", "pero_EGF1_h_p1p0_p1500exe3", "pero_EGF1_h_p1p0_p1500exe4", "pero_EGF1_h_p1p0_p1500exe5", "pero_EGF1_h_p1p0_p1500exe6", "pero_EGF1_h_p1p0_p1500exe7", "pero_EGF1_h_p1p0_p1500exe8", "pero_EGF1_h_p1p0_p1500exe9", "pero_EGF1_h_p1p0_p160000exe0", "pero_EGF1_h_p1p0_p160000exe1", "pero_EGF1_h_p1p0_p160000exe10", "pero_EGF1_h_p1p0_p160000exe11", "pero_EGF1_h_p1p0_p160000exe12", "pero_EGF1_h_p1p0_p160000exe13", "pero_EGF1_h_p1p0_p160000exe14", "pero_EGF1_h_p1p0_p160000exe15", "pero_EGF1_h_p1p0_p160000exe16", "pero_EGF1_h_p1p0_p160000exe2", "pero_EGF1_h_p1p0_p160000exe3", "pero_EGF1_h_p1p0_p160000exe4", "pero_EGF1_h_p1p0_p160000exe5", "pero_EGF1_h_p1p0_p160000exe6", "pero_EGF1_h_p1p0_p160000exe7", "pero_EGF1_h_p1p0_p160000exe8", "pero_EGF1_h_p1p0_p160000exe9", "pero_EGF1_h_p1p0_p1600exe0", "pero_EGF1_h_p1p0_p1600exe1", "pero_EGF1_h_p1p0_p1600exe10", "pero_EGF1_h_p1p0_p1600exe11", "pero_EGF1_h_p1p0_p1600exe12", "pero_EGF1_h_p1p0_p1600exe13", "pero_EGF1_h_p1p0_p1600exe14", "pero_EGF1_h_p1p0_p1600exe15", "pero_EGF1_h_p1p0_p1600exe16", "pero_EGF1_h_p1p0_p1600exe2", "pero_EGF1_h_p1p0_p1600exe3", "pero_EGF1_h_p1p0_p1600exe4", "pero_EGF1_h_p1p0_p1600exe5", "pero_EGF1_h_p1p0_p1600exe6", "pero_EGF1_h_p1p0_p1600exe7", "pero_EGF1_h_p1p0_p1600exe8", "pero_EGF1_h_p1p0_p1600exe9", "pero_EGF1_h_p1p0_p1700exe0", "pero_EGF1_h_p1p0_p1700exe1", "pero_EGF1_h_p1p0_p1700exe10", "pero_EGF1_h_p1p0_p1700exe11", "pero_EGF1_h_p1p0_p1700exe12", "pero_EGF1_h_p1p0_p1700exe13", "pero_EGF1_h_p1p0_p1700exe14", "pero_EGF1_h_p1p0_p1700exe15", "pero_EGF1_h_p1p0_p1700exe16", "pero_EGF1_h_p1p0_p1700exe2", "pero_EGF1_h_p1p0_p1700exe3", "pero_EGF1_h_p1p0_p1700exe4", "pero_EGF1_h_p1p0_p1700exe5", "pero_EGF1_h_p1p0_p1700exe6", "pero_EGF1_h_p1p0_p1700exe7", "pero_EGF1_h_p1p0_p1700exe8", "pero_EGF1_h_p1p0_p1700exe9", "pero_EGF1_h_p1p0_p180000exe0", "pero_EGF1_h_p1p0_p180000exe1", "pero_EGF1_h_p1p0_p180000exe10", "pero_EGF1_h_p1p0_p180000exe11", "pero_EGF1_h_p1p0_p180000exe12", "pero_EGF1_h_p1p0_p180000exe13", "pero_EGF1_h_p1p0_p180000exe14", "pero_EGF1_h_p1p0_p180000exe15", "pero_EGF1_h_p1p0_p180000exe16", "pero_EGF1_h_p1p0_p180000exe2", "pero_EGF1_h_p1p0_p180000exe3", "pero_EGF1_h_p1p0_p180000exe4", "pero_EGF1_h_p1p0_p180000exe5", "pero_EGF1_h_p1p0_p180000exe6", "pero_EGF1_h_p1p0_p180000exe7", "pero_EGF1_h_p1p0_p180000exe8", "pero_EGF1_h_p1p0_p180000exe9", "pero_EGF1_h_p1p0_p1800exe0", "pero_EGF1_h_p1p0_p1800exe1", "pero_EGF1_h_p1p0_p1800exe10", "pero_EGF1_h_p1p0_p1800exe11", "pero_EGF1_h_p1p0_p1800exe12", "pero_EGF1_h_p1p0_p1800exe13", "pero_EGF1_h_p1p0_p1800exe14", "pero_EGF1_h_p1p0_p1800exe15", "pero_EGF1_h_p1p0_p1800exe16", "pero_EGF1_h_p1p0_p1800exe2", "pero_EGF1_h_p1p0_p1800exe3", "pero_EGF1_h_p1p0_p1800exe4", "pero_EGF1_h_p1p0_p1800exe5", "pero_EGF1_h_p1p0_p1800exe6", "pero_EGF1_h_p1p0_p1800exe7", "pero_EGF1_h_p1p0_p1800exe8", "pero_EGF1_h_p1p0_p1800exe9", "pero_EGF1_h_p1p0_p1900exe0", "pero_EGF1_h_p1p0_p1900exe1", "pero_EGF1_h_p1p0_p1900exe10", "pero_EGF1_h_p1p0_p1900exe11", "pero_EGF1_h_p1p0_p1900exe12", "pero_EGF1_h_p1p0_p1900exe13", "pero_EGF1_h_p1p0_p1900exe14", "pero_EGF1_h_p1p0_p1900exe15", "pero_EGF1_h_p1p0_p1900exe16", "pero_EGF1_h_p1p0_p1900exe17", "pero_EGF1_h_p1p0_p1900exe2", "pero_EGF1_h_p1p0_p1900exe3", "pero_EGF1_h_p1p0_p1900exe4", "pero_EGF1_h_p1p0_p1900exe5", "pero_EGF1_h_p1p0_p1900exe6", "pero_EGF1_h_p1p0_p1900exe7", "pero_EGF1_h_p1p0_p1900exe8", "pero_EGF1_h_p1p0_p1900exe9", "pero_EGF1_h_p1p0_p200000exe0", "pero_EGF1_h_p1p0_p200000exe1", "pero_EGF1_h_p1p0_p200000exe10", "pero_EGF1_h_p1p0_p200000exe11", "pero_EGF1_h_p1p0_p200000exe12", "pero_EGF1_h_p1p0_p200000exe13", "pero_EGF1_h_p1p0_p200000exe14", "pero_EGF1_h_p1p0_p200000exe15", "pero_EGF1_h_p1p0_p200000exe16", "pero_EGF1_h_p1p0_p200000exe2", "pero_EGF1_h_p1p0_p200000exe3", "pero_EGF1_h_p1p0_p200000exe4", "pero_EGF1_h_p1p0_p200000exe5", "pero_EGF1_h_p1p0_p200000exe6", "pero_EGF1_h_p1p0_p200000exe7", "pero_EGF1_h_p1p0_p200000exe8", "pero_EGF1_h_p1p0_p200000exe9", "pero_EGF1_h_p1p0_p20000exe0", "pero_EGF1_h_p1p0_p20000exe1", "pero_EGF1_h_p1p0_p20000exe10", "pero_EGF1_h_p1p0_p20000exe11", "pero_EGF1_h_p1p0_p20000exe12", "pero_EGF1_h_p1p0_p20000exe13", "pero_EGF1_h_p1p0_p20000exe14", "pero_EGF1_h_p1p0_p20000exe15", "pero_EGF1_h_p1p0_p20000exe16", "pero_EGF1_h_p1p0_p20000exe2", "pero_EGF1_h_p1p0_p20000exe3", "pero_EGF1_h_p1p0_p20000exe4", "pero_EGF1_h_p1p0_p20000exe5", "pero_EGF1_h_p1p0_p20000exe6", "pero_EGF1_h_p1p0_p20000exe7", "pero_EGF1_h_p1p0_p20000exe8", "pero_EGF1_h_p1p0_p20000exe9", "pero_EGF1_h_p1p0_p2000exe0", "pero_EGF1_h_p1p0_p2000exe1", "pero_EGF1_h_p1p0_p2000exe10", "pero_EGF1_h_p1p0_p2000exe11", "pero_EGF1_h_p1p0_p2000exe12", "pero_EGF1_h_p1p0_p2000exe13", "pero_EGF1_h_p1p0_p2000exe14", "pero_EGF1_h_p1p0_p2000exe15", "pero_EGF1_h_p1p0_p2000exe16", "pero_EGF1_h_p1p0_p2000exe2", "pero_EGF1_h_p1p0_p2000exe3", "pero_EGF1_h_p1p0_p2000exe4", "pero_EGF1_h_p1p0_p2000exe5", "pero_EGF1_h_p1p0_p2000exe6", "pero_EGF1_h_p1p0_p2000exe7", "pero_EGF1_h_p1p0_p2000exe8", "pero_EGF1_h_p1p0_p2000exe9", "pero_EGF1_h_p1p0_p200exe0", "pero_EGF1_h_p1p0_p200exe1", "pero_EGF1_h_p1p0_p200exe10", "pero_EGF1_h_p1p0_p200exe11", "pero_EGF1_h_p1p0_p200exe12", "pero_EGF1_h_p1p0_p200exe13", "pero_EGF1_h_p1p0_p200exe14", "pero_EGF1_h_p1p0_p200exe15", "pero_EGF1_h_p1p0_p200exe16", "pero_EGF1_h_p1p0_p200exe2", "pero_EGF1_h_p1p0_p200exe3", "pero_EGF1_h_p1p0_p200exe4", "pero_EGF1_h_p1p0_p200exe5", "pero_EGF1_h_p1p0_p200exe6", "pero_EGF1_h_p1p0_p200exe7", "pero_EGF1_h_p1p0_p200exe8", "pero_EGF1_h_p1p0_p200exe9", "pero_EGF1_h_p1p0_p2100exe0", "pero_EGF1_h_p1p0_p2100exe1", "pero_EGF1_h_p1p0_p2100exe10", "pero_EGF1_h_p1p0_p2100exe11", "pero_EGF1_h_p1p0_p2100exe12", "pero_EGF1_h_p1p0_p2100exe13", "pero_EGF1_h_p1p0_p2100exe14", "pero_EGF1_h_p1p0_p2100exe15", "pero_EGF1_h_p1p0_p2100exe16", "pero_EGF1_h_p1p0_p2100exe2", "pero_EGF1_h_p1p0_p2100exe3", "pero_EGF1_h_p1p0_p2100exe4", "pero_EGF1_h_p1p0_p2100exe5", "pero_EGF1_h_p1p0_p2100exe6", "pero_EGF1_h_p1p0_p2100exe7", "pero_EGF1_h_p1p0_p2100exe8", "pero_EGF1_h_p1p0_p2100exe9", "pero_EGF1_h_p1p0_p220000exe0", "pero_EGF1_h_p1p0_p220000exe1", "pero_EGF1_h_p1p0_p220000exe10", "pero_EGF1_h_p1p0_p220000exe11", "pero_EGF1_h_p1p0_p220000exe12", "pero_EGF1_h_p1p0_p220000exe13", "pero_EGF1_h_p1p0_p220000exe14", "pero_EGF1_h_p1p0_p220000exe15", "pero_EGF1_h_p1p0_p220000exe16", "pero_EGF1_h_p1p0_p220000exe2", "pero_EGF1_h_p1p0_p220000exe3", "pero_EGF1_h_p1p0_p220000exe4", "pero_EGF1_h_p1p0_p220000exe5", "pero_EGF1_h_p1p0_p220000exe6", "pero_EGF1_h_p1p0_p220000exe7", "pero_EGF1_h_p1p0_p220000exe8", "pero_EGF1_h_p1p0_p220000exe9", "pero_EGF1_h_p1p0_p2200exe0", "pero_EGF1_h_p1p0_p2200exe1", "pero_EGF1_h_p1p0_p2200exe10", "pero_EGF1_h_p1p0_p2200exe11", "pero_EGF1_h_p1p0_p2200exe12", "pero_EGF1_h_p1p0_p2200exe13", "pero_EGF1_h_p1p0_p2200exe14", "pero_EGF1_h_p1p0_p2200exe15", "pero_EGF1_h_p1p0_p2200exe16", "pero_EGF1_h_p1p0_p2200exe2", "pero_EGF1_h_p1p0_p2200exe3", "pero_EGF1_h_p1p0_p2200exe4", "pero_EGF1_h_p1p0_p2200exe5", "pero_EGF1_h_p1p0_p2200exe6", "pero_EGF1_h_p1p0_p2200exe7", "pero_EGF1_h_p1p0_p2200exe8", "pero_EGF1_h_p1p0_p2200exe9", "pero_EGF1_h_p1p0_p2300exe0", "pero_EGF1_h_p1p0_p2300exe1", "pero_EGF1_h_p1p0_p2300exe10", "pero_EGF1_h_p1p0_p2300exe11", "pero_EGF1_h_p1p0_p2300exe12", "pero_EGF1_h_p1p0_p2300exe13", "pero_EGF1_h_p1p0_p2300exe14", "pero_EGF1_h_p1p0_p2300exe15", "pero_EGF1_h_p1p0_p2300exe16", "pero_EGF1_h_p1p0_p2300exe17", "pero_EGF1_h_p1p0_p2300exe2", "pero_EGF1_h_p1p0_p2300exe3", "pero_EGF1_h_p1p0_p2300exe4", "pero_EGF1_h_p1p0_p2300exe5", "pero_EGF1_h_p1p0_p2300exe6", "pero_EGF1_h_p1p0_p2300exe7", "pero_EGF1_h_p1p0_p2300exe8", "pero_EGF1_h_p1p0_p2300exe9", "pero_EGF1_h_p1p0_p240000exe0", "pero_EGF1_h_p1p0_p240000exe1", "pero_EGF1_h_p1p0_p240000exe10", "pero_EGF1_h_p1p0_p240000exe11", "pero_EGF1_h_p1p0_p240000exe12", "pero_EGF1_h_p1p0_p240000exe13", "pero_EGF1_h_p1p0_p240000exe14", "pero_EGF1_h_p1p0_p240000exe15", "pero_EGF1_h_p1p0_p240000exe16", "pero_EGF1_h_p1p0_p240000exe2", "pero_EGF1_h_p1p0_p240000exe3", "pero_EGF1_h_p1p0_p240000exe4", "pero_EGF1_h_p1p0_p240000exe5", "pero_EGF1_h_p1p0_p240000exe6", "pero_EGF1_h_p1p0_p240000exe7", "pero_EGF1_h_p1p0_p240000exe8", "pero_EGF1_h_p1p0_p240000exe9", "pero_EGF1_h_p1p0_p2400exe0", "pero_EGF1_h_p1p0_p2400exe1", "pero_EGF1_h_p1p0_p2400exe10", "pero_EGF1_h_p1p0_p2400exe11", "pero_EGF1_h_p1p0_p2400exe12", "pero_EGF1_h_p1p0_p2400exe13", "pero_EGF1_h_p1p0_p2400exe14", "pero_EGF1_h_p1p0_p2400exe15", "pero_EGF1_h_p1p0_p2400exe16", "pero_EGF1_h_p1p0_p2400exe2", "pero_EGF1_h_p1p0_p2400exe3", "pero_EGF1_h_p1p0_p2400exe4", "pero_EGF1_h_p1p0_p2400exe5", "pero_EGF1_h_p1p0_p2400exe6", "pero_EGF1_h_p1p0_p2400exe7", "pero_EGF1_h_p1p0_p2400exe8", "pero_EGF1_h_p1p0_p2400exe9", "pero_EGF1_h_p1p0_p2500exe0", "pero_EGF1_h_p1p0_p2500exe1", "pero_EGF1_h_p1p0_p2500exe10", "pero_EGF1_h_p1p0_p2500exe11", "pero_EGF1_h_p1p0_p2500exe12", "pero_EGF1_h_p1p0_p2500exe13", "pero_EGF1_h_p1p0_p2500exe14", "pero_EGF1_h_p1p0_p2500exe15", "pero_EGF1_h_p1p0_p2500exe16", "pero_EGF1_h_p1p0_p2500exe2", "pero_EGF1_h_p1p0_p2500exe3", "pero_EGF1_h_p1p0_p2500exe4", "pero_EGF1_h_p1p0_p2500exe5", "pero_EGF1_h_p1p0_p2500exe6", "pero_EGF1_h_p1p0_p2500exe7", "pero_EGF1_h_p1p0_p2500exe8", "pero_EGF1_h_p1p0_p2500exe9", "pero_EGF1_h_p1p0_p260000exe0", "pero_EGF1_h_p1p0_p260000exe1", "pero_EGF1_h_p1p0_p260000exe10", "pero_EGF1_h_p1p0_p260000exe11", "pero_EGF1_h_p1p0_p260000exe12", "pero_EGF1_h_p1p0_p260000exe13", "pero_EGF1_h_p1p0_p260000exe14", "pero_EGF1_h_p1p0_p260000exe15", "pero_EGF1_h_p1p0_p260000exe16", "pero_EGF1_h_p1p0_p260000exe2", "pero_EGF1_h_p1p0_p260000exe3", "pero_EGF1_h_p1p0_p260000exe4", "pero_EGF1_h_p1p0_p260000exe5", "pero_EGF1_h_p1p0_p260000exe6", "pero_EGF1_h_p1p0_p260000exe7", "pero_EGF1_h_p1p0_p260000exe8", "pero_EGF1_h_p1p0_p260000exe9", "pero_EGF1_h_p1p0_p2600exe0", "pero_EGF1_h_p1p0_p2600exe1", "pero_EGF1_h_p1p0_p2600exe10", "pero_EGF1_h_p1p0_p2600exe11", "pero_EGF1_h_p1p0_p2600exe12", "pero_EGF1_h_p1p0_p2600exe13", "pero_EGF1_h_p1p0_p2600exe14", "pero_EGF1_h_p1p0_p2600exe15", "pero_EGF1_h_p1p0_p2600exe16", "pero_EGF1_h_p1p0_p2600exe2", "pero_EGF1_h_p1p0_p2600exe3", "pero_EGF1_h_p1p0_p2600exe4", "pero_EGF1_h_p1p0_p2600exe5", "pero_EGF1_h_p1p0_p2600exe6", "pero_EGF1_h_p1p0_p2600exe7", "pero_EGF1_h_p1p0_p2600exe8", "pero_EGF1_h_p1p0_p2600exe9", "pero_EGF1_h_p1p0_p2700exe0", "pero_EGF1_h_p1p0_p2700exe1", "pero_EGF1_h_p1p0_p2700exe10", "pero_EGF1_h_p1p0_p2700exe11", "pero_EGF1_h_p1p0_p2700exe12", "pero_EGF1_h_p1p0_p2700exe13", "pero_EGF1_h_p1p0_p2700exe14", "pero_EGF1_h_p1p0_p2700exe15", "pero_EGF1_h_p1p0_p2700exe16", "pero_EGF1_h_p1p0_p2700exe2", "pero_EGF1_h_p1p0_p2700exe3", "pero_EGF1_h_p1p0_p2700exe4", "pero_EGF1_h_p1p0_p2700exe5", "pero_EGF1_h_p1p0_p2700exe6", "pero_EGF1_h_p1p0_p2700exe7", "pero_EGF1_h_p1p0_p2700exe8", "pero_EGF1_h_p1p0_p2700exe9", "pero_EGF1_h_p1p0_p280000exe0", "pero_EGF1_h_p1p0_p280000exe1", "pero_EGF1_h_p1p0_p280000exe10", "pero_EGF1_h_p1p0_p280000exe11", "pero_EGF1_h_p1p0_p280000exe12", "pero_EGF1_h_p1p0_p280000exe13", "pero_EGF1_h_p1p0_p280000exe14", "pero_EGF1_h_p1p0_p280000exe15", "pero_EGF1_h_p1p0_p280000exe16", "pero_EGF1_h_p1p0_p280000exe2", "pero_EGF1_h_p1p0_p280000exe3", "pero_EGF1_h_p1p0_p280000exe4", "pero_EGF1_h_p1p0_p280000exe5", "pero_EGF1_h_p1p0_p280000exe6", "pero_EGF1_h_p1p0_p280000exe7", "pero_EGF1_h_p1p0_p280000exe8", "pero_EGF1_h_p1p0_p280000exe9", "pero_EGF1_h_p1p0_p2800exe0", "pero_EGF1_h_p1p0_p2800exe1", "pero_EGF1_h_p1p0_p2800exe10", "pero_EGF1_h_p1p0_p2800exe11", "pero_EGF1_h_p1p0_p2800exe12", "pero_EGF1_h_p1p0_p2800exe13", "pero_EGF1_h_p1p0_p2800exe14", "pero_EGF1_h_p1p0_p2800exe15", "pero_EGF1_h_p1p0_p2800exe16", "pero_EGF1_h_p1p0_p2800exe2", "pero_EGF1_h_p1p0_p2800exe3", "pero_EGF1_h_p1p0_p2800exe4", "pero_EGF1_h_p1p0_p2800exe5", "pero_EGF1_h_p1p0_p2800exe6", "pero_EGF1_h_p1p0_p2800exe7", "pero_EGF1_h_p1p0_p2800exe8", "pero_EGF1_h_p1p0_p2800exe9", "pero_EGF1_h_p1p0_p2900exe0", "pero_EGF1_h_p1p0_p2900exe1", "pero_EGF1_h_p1p0_p2900exe10", "pero_EGF1_h_p1p0_p2900exe11", "pero_EGF1_h_p1p0_p2900exe12", "pero_EGF1_h_p1p0_p2900exe13", "pero_EGF1_h_p1p0_p2900exe14", "pero_EGF1_h_p1p0_p2900exe15", "pero_EGF1_h_p1p0_p2900exe16", "pero_EGF1_h_p1p0_p2900exe2", "pero_EGF1_h_p1p0_p2900exe3", "pero_EGF1_h_p1p0_p2900exe4", "pero_EGF1_h_p1p0_p2900exe5", "pero_EGF1_h_p1p0_p2900exe6", "pero_EGF1_h_p1p0_p2900exe7", "pero_EGF1_h_p1p0_p2900exe8", "pero_EGF1_h_p1p0_p2900exe9", "pero_EGF1_h_p1p0_p300000exe0", "pero_EGF1_h_p1p0_p300000exe1", "pero_EGF1_h_p1p0_p300000exe10", "pero_EGF1_h_p1p0_p300000exe11", "pero_EGF1_h_p1p0_p300000exe12", "pero_EGF1_h_p1p0_p300000exe13", "pero_EGF1_h_p1p0_p300000exe14", "pero_EGF1_h_p1p0_p300000exe15", "pero_EGF1_h_p1p0_p300000exe16", "pero_EGF1_h_p1p0_p300000exe2", "pero_EGF1_h_p1p0_p300000exe3", "pero_EGF1_h_p1p0_p300000exe4", "pero_EGF1_h_p1p0_p300000exe5", "pero_EGF1_h_p1p0_p300000exe6", "pero_EGF1_h_p1p0_p300000exe7", "pero_EGF1_h_p1p0_p300000exe8", "pero_EGF1_h_p1p0_p300000exe9", "pero_EGF1_h_p1p0_p30000exe0", "pero_EGF1_h_p1p0_p30000exe1", "pero_EGF1_h_p1p0_p30000exe10", "pero_EGF1_h_p1p0_p30000exe11", "pero_EGF1_h_p1p0_p30000exe12", "pero_EGF1_h_p1p0_p30000exe13", "pero_EGF1_h_p1p0_p30000exe14", "pero_EGF1_h_p1p0_p30000exe15", "pero_EGF1_h_p1p0_p30000exe16", "pero_EGF1_h_p1p0_p30000exe2", "pero_EGF1_h_p1p0_p30000exe3", "pero_EGF1_h_p1p0_p30000exe4", "pero_EGF1_h_p1p0_p30000exe5", "pero_EGF1_h_p1p0_p30000exe6", "pero_EGF1_h_p1p0_p30000exe7", "pero_EGF1_h_p1p0_p30000exe8", "pero_EGF1_h_p1p0_p30000exe9", "pero_EGF1_h_p1p0_p3000exe0", "pero_EGF1_h_p1p0_p3000exe1", "pero_EGF1_h_p1p0_p3000exe10", "pero_EGF1_h_p1p0_p3000exe11", "pero_EGF1_h_p1p0_p3000exe12", "pero_EGF1_h_p1p0_p3000exe13", "pero_EGF1_h_p1p0_p3000exe14", "pero_EGF1_h_p1p0_p3000exe15", "pero_EGF1_h_p1p0_p3000exe16", "pero_EGF1_h_p1p0_p3000exe17", "pero_EGF1_h_p1p0_p3000exe2", "pero_EGF1_h_p1p0_p3000exe3", "pero_EGF1_h_p1p0_p3000exe4", "pero_EGF1_h_p1p0_p3000exe5", "pero_EGF1_h_p1p0_p3000exe6", "pero_EGF1_h_p1p0_p3000exe7", "pero_EGF1_h_p1p0_p3000exe8", "pero_EGF1_h_p1p0_p3000exe9", "pero_EGF1_h_p1p0_p300exe0", "pero_EGF1_h_p1p0_p300exe1", "pero_EGF1_h_p1p0_p300exe10", "pero_EGF1_h_p1p0_p300exe11", "pero_EGF1_h_p1p0_p300exe12", "pero_EGF1_h_p1p0_p300exe13", "pero_EGF1_h_p1p0_p300exe14", "pero_EGF1_h_p1p0_p300exe15", "pero_EGF1_h_p1p0_p300exe16", "pero_EGF1_h_p1p0_p300exe2", "pero_EGF1_h_p1p0_p300exe3", "pero_EGF1_h_p1p0_p300exe4", "pero_EGF1_h_p1p0_p300exe5", "pero_EGF1_h_p1p0_p300exe6", "pero_EGF1_h_p1p0_p300exe7", "pero_EGF1_h_p1p0_p300exe8", "pero_EGF1_h_p1p0_p300exe9", "pero_EGF1_h_p1p0_p320000exe0", "pero_EGF1_h_p1p0_p320000exe1", "pero_EGF1_h_p1p0_p320000exe10", "pero_EGF1_h_p1p0_p320000exe11", "pero_EGF1_h_p1p0_p320000exe12", "pero_EGF1_h_p1p0_p320000exe13", "pero_EGF1_h_p1p0_p320000exe14", "pero_EGF1_h_p1p0_p320000exe15", "pero_EGF1_h_p1p0_p320000exe16", "pero_EGF1_h_p1p0_p320000exe2", "pero_EGF1_h_p1p0_p320000exe3", "pero_EGF1_h_p1p0_p320000exe4", "pero_EGF1_h_p1p0_p320000exe5", "pero_EGF1_h_p1p0_p320000exe6", "pero_EGF1_h_p1p0_p320000exe7", "pero_EGF1_h_p1p0_p320000exe8", "pero_EGF1_h_p1p0_p320000exe9", "pero_EGF1_h_p1p0_p340000exe0", "pero_EGF1_h_p1p0_p340000exe1", "pero_EGF1_h_p1p0_p340000exe10", "pero_EGF1_h_p1p0_p340000exe11", "pero_EGF1_h_p1p0_p340000exe12", "pero_EGF1_h_p1p0_p340000exe13", "pero_EGF1_h_p1p0_p340000exe14", "pero_EGF1_h_p1p0_p340000exe15", "pero_EGF1_h_p1p0_p340000exe16", "pero_EGF1_h_p1p0_p340000exe2", "pero_EGF1_h_p1p0_p340000exe3", "pero_EGF1_h_p1p0_p340000exe4", "pero_EGF1_h_p1p0_p340000exe5", "pero_EGF1_h_p1p0_p340000exe6", "pero_EGF1_h_p1p0_p340000exe7", "pero_EGF1_h_p1p0_p340000exe8", "pero_EGF1_h_p1p0_p340000exe9", "pero_EGF1_h_p1p0_p360000exe0", "pero_EGF1_h_p1p0_p360000exe1", "pero_EGF1_h_p1p0_p360000exe10", "pero_EGF1_h_p1p0_p360000exe11", "pero_EGF1_h_p1p0_p360000exe12", "pero_EGF1_h_p1p0_p360000exe13", "pero_EGF1_h_p1p0_p360000exe14", "pero_EGF1_h_p1p0_p360000exe15", "pero_EGF1_h_p1p0_p360000exe16", "pero_EGF1_h_p1p0_p360000exe2", "pero_EGF1_h_p1p0_p360000exe3", "pero_EGF1_h_p1p0_p360000exe4", "pero_EGF1_h_p1p0_p360000exe5", "pero_EGF1_h_p1p0_p360000exe6", "pero_EGF1_h_p1p0_p360000exe7", "pero_EGF1_h_p1p0_p360000exe8", "pero_EGF1_h_p1p0_p360000exe9", "pero_EGF1_h_p1p0_p380000exe0", "pero_EGF1_h_p1p0_p380000exe1", "pero_EGF1_h_p1p0_p380000exe10", "pero_EGF1_h_p1p0_p380000exe11", "pero_EGF1_h_p1p0_p380000exe12", "pero_EGF1_h_p1p0_p380000exe13", "pero_EGF1_h_p1p0_p380000exe14", "pero_EGF1_h_p1p0_p380000exe15", "pero_EGF1_h_p1p0_p380000exe16", "pero_EGF1_h_p1p0_p380000exe2", "pero_EGF1_h_p1p0_p380000exe3", "pero_EGF1_h_p1p0_p380000exe4", "pero_EGF1_h_p1p0_p380000exe5", "pero_EGF1_h_p1p0_p380000exe6", "pero_EGF1_h_p1p0_p380000exe7", "pero_EGF1_h_p1p0_p380000exe8", "pero_EGF1_h_p1p0_p380000exe9", "pero_EGF1_h_p1p0_p400000exe0", "pero_EGF1_h_p1p0_p400000exe1", "pero_EGF1_h_p1p0_p400000exe10", "pero_EGF1_h_p1p0_p400000exe11", "pero_EGF1_h_p1p0_p400000exe12", "pero_EGF1_h_p1p0_p400000exe13", "pero_EGF1_h_p1p0_p400000exe14", "pero_EGF1_h_p1p0_p400000exe15", "pero_EGF1_h_p1p0_p400000exe16", "pero_EGF1_h_p1p0_p400000exe2", "pero_EGF1_h_p1p0_p400000exe3", "pero_EGF1_h_p1p0_p400000exe4", "pero_EGF1_h_p1p0_p400000exe5", "pero_EGF1_h_p1p0_p400000exe6", "pero_EGF1_h_p1p0_p400000exe7", "pero_EGF1_h_p1p0_p400000exe8", "pero_EGF1_h_p1p0_p400000exe9", "pero_EGF1_h_p1p0_p40000exe0", "pero_EGF1_h_p1p0_p40000exe1", "pero_EGF1_h_p1p0_p40000exe10", "pero_EGF1_h_p1p0_p40000exe11", "pero_EGF1_h_p1p0_p40000exe12", "pero_EGF1_h_p1p0_p40000exe13", "pero_EGF1_h_p1p0_p40000exe14", "pero_EGF1_h_p1p0_p40000exe15", "pero_EGF1_h_p1p0_p40000exe16", "pero_EGF1_h_p1p0_p40000exe2", "pero_EGF1_h_p1p0_p40000exe3", "pero_EGF1_h_p1p0_p40000exe4", "pero_EGF1_h_p1p0_p40000exe5", "pero_EGF1_h_p1p0_p40000exe6", "pero_EGF1_h_p1p0_p40000exe7", "pero_EGF1_h_p1p0_p40000exe8", "pero_EGF1_h_p1p0_p40000exe9", "pero_EGF1_h_p1p0_p4000exe0", "pero_EGF1_h_p1p0_p4000exe1", "pero_EGF1_h_p1p0_p4000exe10", "pero_EGF1_h_p1p0_p4000exe11", "pero_EGF1_h_p1p0_p4000exe12", "pero_EGF1_h_p1p0_p4000exe13", "pero_EGF1_h_p1p0_p4000exe14", "pero_EGF1_h_p1p0_p4000exe15", "pero_EGF1_h_p1p0_p4000exe16", "pero_EGF1_h_p1p0_p4000exe2", "pero_EGF1_h_p1p0_p4000exe3", "pero_EGF1_h_p1p0_p4000exe4", "pero_EGF1_h_p1p0_p4000exe5", "pero_EGF1_h_p1p0_p4000exe6", "pero_EGF1_h_p1p0_p4000exe7", "pero_EGF1_h_p1p0_p4000exe8", "pero_EGF1_h_p1p0_p4000exe9", "pero_EGF1_h_p1p0_p400exe0", "pero_EGF1_h_p1p0_p400exe1", "pero_EGF1_h_p1p0_p400exe10", "pero_EGF1_h_p1p0_p400exe11", "pero_EGF1_h_p1p0_p400exe12", "pero_EGF1_h_p1p0_p400exe13", "pero_EGF1_h_p1p0_p400exe14", "pero_EGF1_h_p1p0_p400exe15", "pero_EGF1_h_p1p0_p400exe16", "pero_EGF1_h_p1p0_p400exe2", "pero_EGF1_h_p1p0_p400exe3", "pero_EGF1_h_p1p0_p400exe4", "pero_EGF1_h_p1p0_p400exe5", "pero_EGF1_h_p1p0_p400exe6", "pero_EGF1_h_p1p0_p400exe7", "pero_EGF1_h_p1p0_p400exe8", "pero_EGF1_h_p1p0_p400exe9", "pero_EGF1_h_p1p0_p420000exe0", "pero_EGF1_h_p1p0_p420000exe1", "pero_EGF1_h_p1p0_p420000exe10", "pero_EGF1_h_p1p0_p420000exe11", "pero_EGF1_h_p1p0_p420000exe12", "pero_EGF1_h_p1p0_p420000exe13", "pero_EGF1_h_p1p0_p420000exe14", "pero_EGF1_h_p1p0_p420000exe15", "pero_EGF1_h_p1p0_p420000exe16", "pero_EGF1_h_p1p0_p420000exe2", "pero_EGF1_h_p1p0_p420000exe3", "pero_EGF1_h_p1p0_p420000exe4", "pero_EGF1_h_p1p0_p420000exe5", "pero_EGF1_h_p1p0_p420000exe6", "pero_EGF1_h_p1p0_p420000exe7", "pero_EGF1_h_p1p0_p420000exe8", "pero_EGF1_h_p1p0_p420000exe9", "pero_EGF1_h_p1p0_p440000exe0", "pero_EGF1_h_p1p0_p440000exe1", "pero_EGF1_h_p1p0_p440000exe10", "pero_EGF1_h_p1p0_p440000exe11", "pero_EGF1_h_p1p0_p440000exe12", "pero_EGF1_h_p1p0_p440000exe13", "pero_EGF1_h_p1p0_p440000exe14", "pero_EGF1_h_p1p0_p440000exe15", "pero_EGF1_h_p1p0_p440000exe16", "pero_EGF1_h_p1p0_p440000exe2", "pero_EGF1_h_p1p0_p440000exe3", "pero_EGF1_h_p1p0_p440000exe4", "pero_EGF1_h_p1p0_p440000exe5", "pero_EGF1_h_p1p0_p440000exe6", "pero_EGF1_h_p1p0_p440000exe7", "pero_EGF1_h_p1p0_p440000exe8", "pero_EGF1_h_p1p0_p440000exe9", "pero_EGF1_h_p1p0_p480000exe0", "pero_EGF1_h_p1p0_p480000exe1", "pero_EGF1_h_p1p0_p480000exe10", "pero_EGF1_h_p1p0_p480000exe11", "pero_EGF1_h_p1p0_p480000exe12", "pero_EGF1_h_p1p0_p480000exe13", "pero_EGF1_h_p1p0_p480000exe14", "pero_EGF1_h_p1p0_p480000exe15", "pero_EGF1_h_p1p0_p480000exe16", "pero_EGF1_h_p1p0_p480000exe2", "pero_EGF1_h_p1p0_p480000exe3", "pero_EGF1_h_p1p0_p480000exe4", "pero_EGF1_h_p1p0_p480000exe5", "pero_EGF1_h_p1p0_p480000exe6", "pero_EGF1_h_p1p0_p480000exe7", "pero_EGF1_h_p1p0_p480000exe8", "pero_EGF1_h_p1p0_p480000exe9", "pero_EGF1_h_p1p0_p500000exe0", "pero_EGF1_h_p1p0_p500000exe1", "pero_EGF1_h_p1p0_p500000exe10", "pero_EGF1_h_p1p0_p500000exe11", "pero_EGF1_h_p1p0_p500000exe12", "pero_EGF1_h_p1p0_p500000exe13", "pero_EGF1_h_p1p0_p500000exe14", "pero_EGF1_h_p1p0_p500000exe15", "pero_EGF1_h_p1p0_p500000exe16", "pero_EGF1_h_p1p0_p500000exe2", "pero_EGF1_h_p1p0_p500000exe3", "pero_EGF1_h_p1p0_p500000exe4", "pero_EGF1_h_p1p0_p500000exe5", "pero_EGF1_h_p1p0_p500000exe6", "pero_EGF1_h_p1p0_p500000exe7", "pero_EGF1_h_p1p0_p500000exe8", "pero_EGF1_h_p1p0_p500000exe9", "pero_EGF1_h_p1p0_p50000exe0", "pero_EGF1_h_p1p0_p50000exe1", "pero_EGF1_h_p1p0_p50000exe10", "pero_EGF1_h_p1p0_p50000exe11", "pero_EGF1_h_p1p0_p50000exe12", "pero_EGF1_h_p1p0_p50000exe13", "pero_EGF1_h_p1p0_p50000exe14", "pero_EGF1_h_p1p0_p50000exe15", "pero_EGF1_h_p1p0_p50000exe16", "pero_EGF1_h_p1p0_p50000exe2", "pero_EGF1_h_p1p0_p50000exe3", "pero_EGF1_h_p1p0_p50000exe4", "pero_EGF1_h_p1p0_p50000exe5", "pero_EGF1_h_p1p0_p50000exe6", "pero_EGF1_h_p1p0_p50000exe7", "pero_EGF1_h_p1p0_p50000exe8", "pero_EGF1_h_p1p0_p50000exe9", "pero_EGF1_h_p1p0_p500exe0", "pero_EGF1_h_p1p0_p500exe1", "pero_EGF1_h_p1p0_p500exe10", "pero_EGF1_h_p1p0_p500exe11", "pero_EGF1_h_p1p0_p500exe12", "pero_EGF1_h_p1p0_p500exe13", "pero_EGF1_h_p1p0_p500exe14", "pero_EGF1_h_p1p0_p500exe15", "pero_EGF1_h_p1p0_p500exe16", "pero_EGF1_h_p1p0_p500exe2", "pero_EGF1_h_p1p0_p500exe3", "pero_EGF1_h_p1p0_p500exe4", "pero_EGF1_h_p1p0_p500exe5", "pero_EGF1_h_p1p0_p500exe6", "pero_EGF1_h_p1p0_p500exe7", "pero_EGF1_h_p1p0_p500exe8", "pero_EGF1_h_p1p0_p500exe9", "pero_EGF1_h_p1p0_p60000exe0", "pero_EGF1_h_p1p0_p60000exe1", "pero_EGF1_h_p1p0_p60000exe10", "pero_EGF1_h_p1p0_p60000exe11", "pero_EGF1_h_p1p0_p60000exe12", "pero_EGF1_h_p1p0_p60000exe13", "pero_EGF1_h_p1p0_p60000exe14", "pero_EGF1_h_p1p0_p60000exe15", "pero_EGF1_h_p1p0_p60000exe16", "pero_EGF1_h_p1p0_p60000exe2", "pero_EGF1_h_p1p0_p60000exe3", "pero_EGF1_h_p1p0_p60000exe4", "pero_EGF1_h_p1p0_p60000exe5", "pero_EGF1_h_p1p0_p60000exe6", "pero_EGF1_h_p1p0_p60000exe7", "pero_EGF1_h_p1p0_p60000exe8", "pero_EGF1_h_p1p0_p60000exe9", "pero_EGF1_h_p1p0_p6000exe0", "pero_EGF1_h_p1p0_p6000exe1", "pero_EGF1_h_p1p0_p6000exe10", "pero_EGF1_h_p1p0_p6000exe11", "pero_EGF1_h_p1p0_p6000exe12", "pero_EGF1_h_p1p0_p6000exe13", "pero_EGF1_h_p1p0_p6000exe14", "pero_EGF1_h_p1p0_p6000exe15", "pero_EGF1_h_p1p0_p6000exe16", "pero_EGF1_h_p1p0_p6000exe2", "pero_EGF1_h_p1p0_p6000exe3", "pero_EGF1_h_p1p0_p6000exe4", "pero_EGF1_h_p1p0_p6000exe5", "pero_EGF1_h_p1p0_p6000exe6", "pero_EGF1_h_p1p0_p6000exe7", "pero_EGF1_h_p1p0_p6000exe8", "pero_EGF1_h_p1p0_p6000exe9", "pero_EGF1_h_p1p0_p600exe0", "pero_EGF1_h_p1p0_p600exe1", "pero_EGF1_h_p1p0_p600exe10", "pero_EGF1_h_p1p0_p600exe11", "pero_EGF1_h_p1p0_p600exe12", "pero_EGF1_h_p1p0_p600exe13", "pero_EGF1_h_p1p0_p600exe14", "pero_EGF1_h_p1p0_p600exe15", "pero_EGF1_h_p1p0_p600exe16", "pero_EGF1_h_p1p0_p600exe17", "pero_EGF1_h_p1p0_p600exe2", "pero_EGF1_h_p1p0_p600exe3", "pero_EGF1_h_p1p0_p600exe4", "pero_EGF1_h_p1p0_p600exe5", "pero_EGF1_h_p1p0_p600exe6", "pero_EGF1_h_p1p0_p600exe7", "pero_EGF1_h_p1p0_p600exe8", "pero_EGF1_h_p1p0_p600exe9", "pero_EGF1_h_p1p0_p700exe0", "pero_EGF1_h_p1p0_p700exe1", "pero_EGF1_h_p1p0_p700exe10", "pero_EGF1_h_p1p0_p700exe11", "pero_EGF1_h_p1p0_p700exe12", "pero_EGF1_h_p1p0_p700exe13", "pero_EGF1_h_p1p0_p700exe14", "pero_EGF1_h_p1p0_p700exe15", "pero_EGF1_h_p1p0_p700exe16", "pero_EGF1_h_p1p0_p700exe2", "pero_EGF1_h_p1p0_p700exe3", "pero_EGF1_h_p1p0_p700exe4", "pero_EGF1_h_p1p0_p700exe5", "pero_EGF1_h_p1p0_p700exe6", "pero_EGF1_h_p1p0_p700exe7", "pero_EGF1_h_p1p0_p700exe8", "pero_EGF1_h_p1p0_p700exe9", "pero_EGF1_h_p1p0_p80000exe0", "pero_EGF1_h_p1p0_p80000exe1", "pero_EGF1_h_p1p0_p80000exe10", "pero_EGF1_h_p1p0_p80000exe11", "pero_EGF1_h_p1p0_p80000exe12", "pero_EGF1_h_p1p0_p80000exe13", "pero_EGF1_h_p1p0_p80000exe14", "pero_EGF1_h_p1p0_p80000exe15", "pero_EGF1_h_p1p0_p80000exe16", "pero_EGF1_h_p1p0_p80000exe2", "pero_EGF1_h_p1p0_p80000exe3", "pero_EGF1_h_p1p0_p80000exe4", "pero_EGF1_h_p1p0_p80000exe5", "pero_EGF1_h_p1p0_p80000exe6", "pero_EGF1_h_p1p0_p80000exe7", "pero_EGF1_h_p1p0_p80000exe8", "pero_EGF1_h_p1p0_p80000exe9", "pero_EGF1_h_p1p0_p800exe0", "pero_EGF1_h_p1p0_p800exe1", "pero_EGF1_h_p1p0_p800exe10", "pero_EGF1_h_p1p0_p800exe11", "pero_EGF1_h_p1p0_p800exe12", "pero_EGF1_h_p1p0_p800exe13", "pero_EGF1_h_p1p0_p800exe14", "pero_EGF1_h_p1p0_p800exe15", "pero_EGF1_h_p1p0_p800exe16", "pero_EGF1_h_p1p0_p800exe2", "pero_EGF1_h_p1p0_p800exe3", "pero_EGF1_h_p1p0_p800exe4", "pero_EGF1_h_p1p0_p800exe5", "pero_EGF1_h_p1p0_p800exe6", "pero_EGF1_h_p1p0_p800exe7", "pero_EGF1_h_p1p0_p800exe8", "pero_EGF1_h_p1p0_p800exe9", "pero_EGF1_h_p1p0_p900exe0", "pero_EGF1_h_p1p0_p900exe1", "pero_EGF1_h_p1p0_p900exe10", "pero_EGF1_h_p1p0_p900exe11", "pero_EGF1_h_p1p0_p900exe12", "pero_EGF1_h_p1p0_p900exe13", "pero_EGF1_h_p1p0_p900exe14", "pero_EGF1_h_p1p0_p900exe15", "pero_EGF1_h_p1p0_p900exe16", "pero_EGF1_h_p1p0_p900exe2", "pero_EGF1_h_p1p0_p900exe3", "pero_EGF1_h_p1p0_p900exe4", "pero_EGF1_h_p1p0_p900exe5", "pero_EGF1_h_p1p0_p900exe6", "pero_EGF1_h_p1p0_p900exe7", "pero_EGF1_h_p1p0_p900exe8", "pero_EGF1_h_p1p0_p900exe9", "pero_EGF1_h_p1p1_m0exe0", "pero_EGF1_h_p1p1_m0exe1", "pero_EGF1_h_p1p1_m0exe10", "pero_EGF1_h_p1p1_m0exe11", "pero_EGF1_h_p1p1_m0exe12", "pero_EGF1_h_p1p1_m0exe13", "pero_EGF1_h_p1p1_m0exe14", "pero_EGF1_h_p1p1_m0exe15", "pero_EGF1_h_p1p1_m0exe16", "pero_EGF1_h_p1p1_m0exe2", "pero_EGF1_h_p1p1_m0exe3", "pero_EGF1_h_p1p1_m0exe4", "pero_EGF1_h_p1p1_m0exe5", "pero_EGF1_h_p1p1_m0exe6", "pero_EGF1_h_p1p1_m0exe7", "pero_EGF1_h_p1p1_m0exe8", "pero_EGF1_h_p1p1_m0exe9", "pero_EGF1_h_p1p1_m100exe0", "pero_EGF1_h_p1p1_m100exe1", "pero_EGF1_h_p1p1_m100exe10", "pero_EGF1_h_p1p1_m100exe11", "pero_EGF1_h_p1p1_m100exe12", "pero_EGF1_h_p1p1_m100exe13", "pero_EGF1_h_p1p1_m100exe14", "pero_EGF1_h_p1p1_m100exe15", "pero_EGF1_h_p1p1_m100exe16", "pero_EGF1_h_p1p1_m100exe2", "pero_EGF1_h_p1p1_m100exe3", "pero_EGF1_h_p1p1_m100exe4", "pero_EGF1_h_p1p1_m100exe5", "pero_EGF1_h_p1p1_m100exe6", "pero_EGF1_h_p1p1_m100exe7", "pero_EGF1_h_p1p1_m100exe8", "pero_EGF1_h_p1p1_m100exe9", "pero_EGF1_h_p1p1_m200exe0", "pero_EGF1_h_p1p1_m200exe1", "pero_EGF1_h_p1p1_m200exe10", "pero_EGF1_h_p1p1_m200exe11", "pero_EGF1_h_p1p1_m200exe12", "pero_EGF1_h_p1p1_m200exe13", "pero_EGF1_h_p1p1_m200exe14", "pero_EGF1_h_p1p1_m200exe15", "pero_EGF1_h_p1p1_m200exe16", "pero_EGF1_h_p1p1_m200exe2", "pero_EGF1_h_p1p1_m200exe3", "pero_EGF1_h_p1p1_m200exe4", "pero_EGF1_h_p1p1_m200exe5", "pero_EGF1_h_p1p1_m200exe6", "pero_EGF1_h_p1p1_m200exe7", "pero_EGF1_h_p1p1_m200exe8", "pero_EGF1_h_p1p1_m200exe9", "pero_EGF1_h_p1p1_m300exe0", "pero_EGF1_h_p1p1_m300exe1", "pero_EGF1_h_p1p1_m300exe10", "pero_EGF1_h_p1p1_m300exe11", "pero_EGF1_h_p1p1_m300exe12", "pero_EGF1_h_p1p1_m300exe13", "pero_EGF1_h_p1p1_m300exe14", "pero_EGF1_h_p1p1_m300exe15", "pero_EGF1_h_p1p1_m300exe16", "pero_EGF1_h_p1p1_m300exe2", "pero_EGF1_h_p1p1_m300exe3", "pero_EGF1_h_p1p1_m300exe4", "pero_EGF1_h_p1p1_m300exe5", "pero_EGF1_h_p1p1_m300exe6", "pero_EGF1_h_p1p1_m300exe7", "pero_EGF1_h_p1p1_m300exe8", "pero_EGF1_h_p1p1_m300exe9", "pero_EGF1_h_p1p1_m5000exe0", "pero_EGF1_h_p1p1_m5000exe1", "pero_EGF1_h_p1p1_m5000exe10", "pero_EGF1_h_p1p1_m5000exe11", "pero_EGF1_h_p1p1_m5000exe12", "pero_EGF1_h_p1p1_m5000exe13", "pero_EGF1_h_p1p1_m5000exe14", "pero_EGF1_h_p1p1_m5000exe15", "pero_EGF1_h_p1p1_m5000exe16", "pero_EGF1_h_p1p1_m5000exe2", "pero_EGF1_h_p1p1_m5000exe3", "pero_EGF1_h_p1p1_m5000exe4", "pero_EGF1_h_p1p1_m5000exe5", "pero_EGF1_h_p1p1_m5000exe6", "pero_EGF1_h_p1p1_m5000exe7", "pero_EGF1_h_p1p1_m5000exe8", "pero_EGF1_h_p1p1_m5000exe9", "pero_EGF1_h_p1p1_m500exe0", "pero_EGF1_h_p1p1_m500exe1", "pero_EGF1_h_p1p1_m500exe10", "pero_EGF1_h_p1p1_m500exe11", "pero_EGF1_h_p1p1_m500exe12", "pero_EGF1_h_p1p1_m500exe13", "pero_EGF1_h_p1p1_m500exe14", "pero_EGF1_h_p1p1_m500exe15", "pero_EGF1_h_p1p1_m500exe16", "pero_EGF1_h_p1p1_m500exe2", "pero_EGF1_h_p1p1_m500exe3", "pero_EGF1_h_p1p1_m500exe4", "pero_EGF1_h_p1p1_m500exe5", "pero_EGF1_h_p1p1_m500exe6", "pero_EGF1_h_p1p1_m500exe7", "pero_EGF1_h_p1p1_m500exe8", "pero_EGF1_h_p1p1_m500exe9", "pero_EGF1_h_p1p1_p100000exe0", "pero_EGF1_h_p1p1_p100000exe1", "pero_EGF1_h_p1p1_p100000exe10", "pero_EGF1_h_p1p1_p100000exe11", "pero_EGF1_h_p1p1_p100000exe12", "pero_EGF1_h_p1p1_p100000exe13", "pero_EGF1_h_p1p1_p100000exe14", "pero_EGF1_h_p1p1_p100000exe15", "pero_EGF1_h_p1p1_p100000exe16", "pero_EGF1_h_p1p1_p100000exe2", "pero_EGF1_h_p1p1_p100000exe3", "pero_EGF1_h_p1p1_p100000exe4", "pero_EGF1_h_p1p1_p100000exe5", "pero_EGF1_h_p1p1_p100000exe6", "pero_EGF1_h_p1p1_p100000exe7", "pero_EGF1_h_p1p1_p100000exe8", "pero_EGF1_h_p1p1_p100000exe9", "pero_EGF1_h_p1p1_p10000exe0", "pero_EGF1_h_p1p1_p10000exe1", "pero_EGF1_h_p1p1_p10000exe10", "pero_EGF1_h_p1p1_p10000exe11", "pero_EGF1_h_p1p1_p10000exe12", "pero_EGF1_h_p1p1_p10000exe13", "pero_EGF1_h_p1p1_p10000exe14", "pero_EGF1_h_p1p1_p10000exe15", "pero_EGF1_h_p1p1_p10000exe16", "pero_EGF1_h_p1p1_p10000exe2", "pero_EGF1_h_p1p1_p10000exe3", "pero_EGF1_h_p1p1_p10000exe4", "pero_EGF1_h_p1p1_p10000exe5", "pero_EGF1_h_p1p1_p10000exe6", "pero_EGF1_h_p1p1_p10000exe7", "pero_EGF1_h_p1p1_p10000exe8", "pero_EGF1_h_p1p1_p10000exe9", "pero_EGF1_h_p1p1_p1000exe0", "pero_EGF1_h_p1p1_p1000exe1", "pero_EGF1_h_p1p1_p1000exe10", "pero_EGF1_h_p1p1_p1000exe11", "pero_EGF1_h_p1p1_p1000exe12", "pero_EGF1_h_p1p1_p1000exe13", "pero_EGF1_h_p1p1_p1000exe14", "pero_EGF1_h_p1p1_p1000exe15", "pero_EGF1_h_p1p1_p1000exe16", "pero_EGF1_h_p1p1_p1000exe17", "pero_EGF1_h_p1p1_p1000exe2", "pero_EGF1_h_p1p1_p1000exe3", "pero_EGF1_h_p1p1_p1000exe4", "pero_EGF1_h_p1p1_p1000exe5", "pero_EGF1_h_p1p1_p1000exe6", "pero_EGF1_h_p1p1_p1000exe7", "pero_EGF1_h_p1p1_p1000exe8", "pero_EGF1_h_p1p1_p1000exe9", "pero_EGF1_h_p1p1_p100exe0", "pero_EGF1_h_p1p1_p100exe1", "pero_EGF1_h_p1p1_p100exe10", "pero_EGF1_h_p1p1_p100exe11", "pero_EGF1_h_p1p1_p100exe12", "pero_EGF1_h_p1p1_p100exe13", "pero_EGF1_h_p1p1_p100exe14", "pero_EGF1_h_p1p1_p100exe15", "pero_EGF1_h_p1p1_p100exe16", "pero_EGF1_h_p1p1_p100exe2", "pero_EGF1_h_p1p1_p100exe3", "pero_EGF1_h_p1p1_p100exe4", "pero_EGF1_h_p1p1_p100exe5", "pero_EGF1_h_p1p1_p100exe6", "pero_EGF1_h_p1p1_p100exe7", "pero_EGF1_h_p1p1_p100exe8", "pero_EGF1_h_p1p1_p100exe9", "pero_EGF1_h_p1p1_p1100exe0", "pero_EGF1_h_p1p1_p1100exe1", "pero_EGF1_h_p1p1_p1100exe10", "pero_EGF1_h_p1p1_p1100exe11", "pero_EGF1_h_p1p1_p1100exe12", "pero_EGF1_h_p1p1_p1100exe13", "pero_EGF1_h_p1p1_p1100exe14", "pero_EGF1_h_p1p1_p1100exe15", "pero_EGF1_h_p1p1_p1100exe16", "pero_EGF1_h_p1p1_p1100exe2", "pero_EGF1_h_p1p1_p1100exe3", "pero_EGF1_h_p1p1_p1100exe4", "pero_EGF1_h_p1p1_p1100exe5", "pero_EGF1_h_p1p1_p1100exe6", "pero_EGF1_h_p1p1_p1100exe7", "pero_EGF1_h_p1p1_p1100exe8", "pero_EGF1_h_p1p1_p1100exe9", "pero_EGF1_h_p1p1_p120000exe0", "pero_EGF1_h_p1p1_p120000exe1", "pero_EGF1_h_p1p1_p120000exe10", "pero_EGF1_h_p1p1_p120000exe11", "pero_EGF1_h_p1p1_p120000exe12", "pero_EGF1_h_p1p1_p120000exe13", "pero_EGF1_h_p1p1_p120000exe14", "pero_EGF1_h_p1p1_p120000exe15", "pero_EGF1_h_p1p1_p120000exe16", "pero_EGF1_h_p1p1_p120000exe2", "pero_EGF1_h_p1p1_p120000exe3", "pero_EGF1_h_p1p1_p120000exe4", "pero_EGF1_h_p1p1_p120000exe5", "pero_EGF1_h_p1p1_p120000exe6", "pero_EGF1_h_p1p1_p120000exe7", "pero_EGF1_h_p1p1_p120000exe8", "pero_EGF1_h_p1p1_p120000exe9", "pero_EGF1_h_p1p1_p1200exe0", "pero_EGF1_h_p1p1_p1200exe1", "pero_EGF1_h_p1p1_p1200exe10", "pero_EGF1_h_p1p1_p1200exe11", "pero_EGF1_h_p1p1_p1200exe12", "pero_EGF1_h_p1p1_p1200exe13", "pero_EGF1_h_p1p1_p1200exe14", "pero_EGF1_h_p1p1_p1200exe15", "pero_EGF1_h_p1p1_p1200exe16", "pero_EGF1_h_p1p1_p1200exe2", "pero_EGF1_h_p1p1_p1200exe3", "pero_EGF1_h_p1p1_p1200exe4", "pero_EGF1_h_p1p1_p1200exe5", "pero_EGF1_h_p1p1_p1200exe6", "pero_EGF1_h_p1p1_p1200exe7", "pero_EGF1_h_p1p1_p1200exe8", "pero_EGF1_h_p1p1_p1200exe9", "pero_EGF1_h_p1p1_p1300exe0", "pero_EGF1_h_p1p1_p1300exe1", "pero_EGF1_h_p1p1_p1300exe10", "pero_EGF1_h_p1p1_p1300exe11", "pero_EGF1_h_p1p1_p1300exe12", "pero_EGF1_h_p1p1_p1300exe13", "pero_EGF1_h_p1p1_p1300exe14", "pero_EGF1_h_p1p1_p1300exe15", "pero_EGF1_h_p1p1_p1300exe16", "pero_EGF1_h_p1p1_p1300exe2", "pero_EGF1_h_p1p1_p1300exe3", "pero_EGF1_h_p1p1_p1300exe4", "pero_EGF1_h_p1p1_p1300exe5", "pero_EGF1_h_p1p1_p1300exe6", "pero_EGF1_h_p1p1_p1300exe7", "pero_EGF1_h_p1p1_p1300exe8", "pero_EGF1_h_p1p1_p1300exe9", "pero_EGF1_h_p1p1_p140000exe0", "pero_EGF1_h_p1p1_p140000exe1", "pero_EGF1_h_p1p1_p140000exe10", "pero_EGF1_h_p1p1_p140000exe11", "pero_EGF1_h_p1p1_p140000exe12", "pero_EGF1_h_p1p1_p140000exe13", "pero_EGF1_h_p1p1_p140000exe14", "pero_EGF1_h_p1p1_p140000exe15", "pero_EGF1_h_p1p1_p140000exe16", "pero_EGF1_h_p1p1_p140000exe2", "pero_EGF1_h_p1p1_p140000exe3", "pero_EGF1_h_p1p1_p140000exe4", "pero_EGF1_h_p1p1_p140000exe5", "pero_EGF1_h_p1p1_p140000exe6", "pero_EGF1_h_p1p1_p140000exe7", "pero_EGF1_h_p1p1_p140000exe8", "pero_EGF1_h_p1p1_p140000exe9", "pero_EGF1_h_p1p1_p1400exe0", "pero_EGF1_h_p1p1_p1400exe1", "pero_EGF1_h_p1p1_p1400exe10", "pero_EGF1_h_p1p1_p1400exe11", "pero_EGF1_h_p1p1_p1400exe12", "pero_EGF1_h_p1p1_p1400exe13", "pero_EGF1_h_p1p1_p1400exe14", "pero_EGF1_h_p1p1_p1400exe15", "pero_EGF1_h_p1p1_p1400exe16", "pero_EGF1_h_p1p1_p1400exe2", "pero_EGF1_h_p1p1_p1400exe3", "pero_EGF1_h_p1p1_p1400exe4", "pero_EGF1_h_p1p1_p1400exe5", "pero_EGF1_h_p1p1_p1400exe6", "pero_EGF1_h_p1p1_p1400exe7", "pero_EGF1_h_p1p1_p1400exe8", "pero_EGF1_h_p1p1_p1400exe9", "pero_EGF1_h_p1p1_p1500exe0", "pero_EGF1_h_p1p1_p1500exe1", "pero_EGF1_h_p1p1_p1500exe10", "pero_EGF1_h_p1p1_p1500exe11", "pero_EGF1_h_p1p1_p1500exe12", "pero_EGF1_h_p1p1_p1500exe13", "pero_EGF1_h_p1p1_p1500exe14", "pero_EGF1_h_p1p1_p1500exe15", "pero_EGF1_h_p1p1_p1500exe16", "pero_EGF1_h_p1p1_p1500exe2", "pero_EGF1_h_p1p1_p1500exe3", "pero_EGF1_h_p1p1_p1500exe4", "pero_EGF1_h_p1p1_p1500exe5", "pero_EGF1_h_p1p1_p1500exe6", "pero_EGF1_h_p1p1_p1500exe7", "pero_EGF1_h_p1p1_p1500exe8", "pero_EGF1_h_p1p1_p1500exe9", "pero_EGF1_h_p1p1_p160000exe0", "pero_EGF1_h_p1p1_p160000exe1", "pero_EGF1_h_p1p1_p160000exe10", "pero_EGF1_h_p1p1_p160000exe11", "pero_EGF1_h_p1p1_p160000exe12", "pero_EGF1_h_p1p1_p160000exe13", "pero_EGF1_h_p1p1_p160000exe14", "pero_EGF1_h_p1p1_p160000exe15", "pero_EGF1_h_p1p1_p160000exe16", "pero_EGF1_h_p1p1_p160000exe2", "pero_EGF1_h_p1p1_p160000exe3", "pero_EGF1_h_p1p1_p160000exe4", "pero_EGF1_h_p1p1_p160000exe5", "pero_EGF1_h_p1p1_p160000exe6", "pero_EGF1_h_p1p1_p160000exe7", "pero_EGF1_h_p1p1_p160000exe8", "pero_EGF1_h_p1p1_p160000exe9", "pero_EGF1_h_p1p1_p1600exe0", "pero_EGF1_h_p1p1_p1600exe1", "pero_EGF1_h_p1p1_p1600exe10", "pero_EGF1_h_p1p1_p1600exe11", "pero_EGF1_h_p1p1_p1600exe12", "pero_EGF1_h_p1p1_p1600exe13", "pero_EGF1_h_p1p1_p1600exe14", "pero_EGF1_h_p1p1_p1600exe15", "pero_EGF1_h_p1p1_p1600exe16", "pero_EGF1_h_p1p1_p1600exe2", "pero_EGF1_h_p1p1_p1600exe3", "pero_EGF1_h_p1p1_p1600exe4", "pero_EGF1_h_p1p1_p1600exe5", "pero_EGF1_h_p1p1_p1600exe6", "pero_EGF1_h_p1p1_p1600exe7", "pero_EGF1_h_p1p1_p1600exe8", "pero_EGF1_h_p1p1_p1600exe9", "pero_EGF1_h_p1p1_p1700exe0", "pero_EGF1_h_p1p1_p1700exe1", "pero_EGF1_h_p1p1_p1700exe10", "pero_EGF1_h_p1p1_p1700exe11", "pero_EGF1_h_p1p1_p1700exe12", "pero_EGF1_h_p1p1_p1700exe13", "pero_EGF1_h_p1p1_p1700exe14", "pero_EGF1_h_p1p1_p1700exe15", "pero_EGF1_h_p1p1_p1700exe16", "pero_EGF1_h_p1p1_p1700exe2", "pero_EGF1_h_p1p1_p1700exe3", "pero_EGF1_h_p1p1_p1700exe4", "pero_EGF1_h_p1p1_p1700exe5", "pero_EGF1_h_p1p1_p1700exe6", "pero_EGF1_h_p1p1_p1700exe7", "pero_EGF1_h_p1p1_p1700exe8", "pero_EGF1_h_p1p1_p1700exe9", "pero_EGF1_h_p1p1_p180000exe0", "pero_EGF1_h_p1p1_p180000exe1", "pero_EGF1_h_p1p1_p180000exe10", "pero_EGF1_h_p1p1_p180000exe11", "pero_EGF1_h_p1p1_p180000exe12", "pero_EGF1_h_p1p1_p180000exe13", "pero_EGF1_h_p1p1_p180000exe14", "pero_EGF1_h_p1p1_p180000exe15", "pero_EGF1_h_p1p1_p180000exe16", "pero_EGF1_h_p1p1_p180000exe2", "pero_EGF1_h_p1p1_p180000exe3", "pero_EGF1_h_p1p1_p180000exe4", "pero_EGF1_h_p1p1_p180000exe5", "pero_EGF1_h_p1p1_p180000exe6", "pero_EGF1_h_p1p1_p180000exe7", "pero_EGF1_h_p1p1_p180000exe8", "pero_EGF1_h_p1p1_p180000exe9", "pero_EGF1_h_p1p1_p1800exe0", "pero_EGF1_h_p1p1_p1800exe1", "pero_EGF1_h_p1p1_p1800exe10", "pero_EGF1_h_p1p1_p1800exe11", "pero_EGF1_h_p1p1_p1800exe12", "pero_EGF1_h_p1p1_p1800exe13", "pero_EGF1_h_p1p1_p1800exe14", "pero_EGF1_h_p1p1_p1800exe15", "pero_EGF1_h_p1p1_p1800exe16", "pero_EGF1_h_p1p1_p1800exe2", "pero_EGF1_h_p1p1_p1800exe3", "pero_EGF1_h_p1p1_p1800exe4", "pero_EGF1_h_p1p1_p1800exe5", "pero_EGF1_h_p1p1_p1800exe6", "pero_EGF1_h_p1p1_p1800exe7", "pero_EGF1_h_p1p1_p1800exe8", "pero_EGF1_h_p1p1_p1800exe9", "pero_EGF1_h_p1p1_p1900exe0", "pero_EGF1_h_p1p1_p1900exe1", "pero_EGF1_h_p1p1_p1900exe10", "pero_EGF1_h_p1p1_p1900exe11", "pero_EGF1_h_p1p1_p1900exe12", "pero_EGF1_h_p1p1_p1900exe13", "pero_EGF1_h_p1p1_p1900exe14", "pero_EGF1_h_p1p1_p1900exe15", "pero_EGF1_h_p1p1_p1900exe16", "pero_EGF1_h_p1p1_p1900exe17", "pero_EGF1_h_p1p1_p1900exe2", "pero_EGF1_h_p1p1_p1900exe3", "pero_EGF1_h_p1p1_p1900exe4", "pero_EGF1_h_p1p1_p1900exe5", "pero_EGF1_h_p1p1_p1900exe6", "pero_EGF1_h_p1p1_p1900exe7", "pero_EGF1_h_p1p1_p1900exe8", "pero_EGF1_h_p1p1_p1900exe9", "pero_EGF1_h_p1p1_p200000exe0", "pero_EGF1_h_p1p1_p200000exe1", "pero_EGF1_h_p1p1_p200000exe10", "pero_EGF1_h_p1p1_p200000exe11", "pero_EGF1_h_p1p1_p200000exe12", "pero_EGF1_h_p1p1_p200000exe13", "pero_EGF1_h_p1p1_p200000exe14", "pero_EGF1_h_p1p1_p200000exe15", "pero_EGF1_h_p1p1_p200000exe16", "pero_EGF1_h_p1p1_p200000exe2", "pero_EGF1_h_p1p1_p200000exe3", "pero_EGF1_h_p1p1_p200000exe4", "pero_EGF1_h_p1p1_p200000exe5", "pero_EGF1_h_p1p1_p200000exe6", "pero_EGF1_h_p1p1_p200000exe7", "pero_EGF1_h_p1p1_p200000exe8", "pero_EGF1_h_p1p1_p200000exe9", "pero_EGF1_h_p1p1_p20000exe0", "pero_EGF1_h_p1p1_p20000exe1", "pero_EGF1_h_p1p1_p20000exe10", "pero_EGF1_h_p1p1_p20000exe11", "pero_EGF1_h_p1p1_p20000exe12", "pero_EGF1_h_p1p1_p20000exe13", "pero_EGF1_h_p1p1_p20000exe14", "pero_EGF1_h_p1p1_p20000exe15", "pero_EGF1_h_p1p1_p20000exe16", "pero_EGF1_h_p1p1_p20000exe2", "pero_EGF1_h_p1p1_p20000exe3", "pero_EGF1_h_p1p1_p20000exe4", "pero_EGF1_h_p1p1_p20000exe5", "pero_EGF1_h_p1p1_p20000exe6", "pero_EGF1_h_p1p1_p20000exe7", "pero_EGF1_h_p1p1_p20000exe8", "pero_EGF1_h_p1p1_p20000exe9", "pero_EGF1_h_p1p1_p2000exe0", "pero_EGF1_h_p1p1_p2000exe1", "pero_EGF1_h_p1p1_p2000exe10", "pero_EGF1_h_p1p1_p2000exe11", "pero_EGF1_h_p1p1_p2000exe12", "pero_EGF1_h_p1p1_p2000exe13", "pero_EGF1_h_p1p1_p2000exe14", "pero_EGF1_h_p1p1_p2000exe15", "pero_EGF1_h_p1p1_p2000exe16", "pero_EGF1_h_p1p1_p2000exe2", "pero_EGF1_h_p1p1_p2000exe3", "pero_EGF1_h_p1p1_p2000exe4", "pero_EGF1_h_p1p1_p2000exe5", "pero_EGF1_h_p1p1_p2000exe6", "pero_EGF1_h_p1p1_p2000exe7", "pero_EGF1_h_p1p1_p2000exe8", "pero_EGF1_h_p1p1_p2000exe9", "pero_EGF1_h_p1p1_p200exe0", "pero_EGF1_h_p1p1_p200exe1", "pero_EGF1_h_p1p1_p200exe10", "pero_EGF1_h_p1p1_p200exe11", "pero_EGF1_h_p1p1_p200exe12", "pero_EGF1_h_p1p1_p200exe13", "pero_EGF1_h_p1p1_p200exe14", "pero_EGF1_h_p1p1_p200exe15", "pero_EGF1_h_p1p1_p200exe16", "pero_EGF1_h_p1p1_p200exe2", "pero_EGF1_h_p1p1_p200exe3", "pero_EGF1_h_p1p1_p200exe4", "pero_EGF1_h_p1p1_p200exe5", "pero_EGF1_h_p1p1_p200exe6", "pero_EGF1_h_p1p1_p200exe7", "pero_EGF1_h_p1p1_p200exe8", "pero_EGF1_h_p1p1_p200exe9", "pero_EGF1_h_p1p1_p2100exe0", "pero_EGF1_h_p1p1_p2100exe1", "pero_EGF1_h_p1p1_p2100exe10", "pero_EGF1_h_p1p1_p2100exe11", "pero_EGF1_h_p1p1_p2100exe12", "pero_EGF1_h_p1p1_p2100exe13", "pero_EGF1_h_p1p1_p2100exe14", "pero_EGF1_h_p1p1_p2100exe15", "pero_EGF1_h_p1p1_p2100exe16", "pero_EGF1_h_p1p1_p2100exe2", "pero_EGF1_h_p1p1_p2100exe3", "pero_EGF1_h_p1p1_p2100exe4", "pero_EGF1_h_p1p1_p2100exe5", "pero_EGF1_h_p1p1_p2100exe6", "pero_EGF1_h_p1p1_p2100exe7", "pero_EGF1_h_p1p1_p2100exe8", "pero_EGF1_h_p1p1_p2100exe9", "pero_EGF1_h_p1p1_p220000exe0", "pero_EGF1_h_p1p1_p220000exe1", "pero_EGF1_h_p1p1_p220000exe10", "pero_EGF1_h_p1p1_p220000exe11", "pero_EGF1_h_p1p1_p220000exe12", "pero_EGF1_h_p1p1_p220000exe13", "pero_EGF1_h_p1p1_p220000exe14", "pero_EGF1_h_p1p1_p220000exe15", "pero_EGF1_h_p1p1_p220000exe16", "pero_EGF1_h_p1p1_p220000exe2", "pero_EGF1_h_p1p1_p220000exe3", "pero_EGF1_h_p1p1_p220000exe4", "pero_EGF1_h_p1p1_p220000exe5", "pero_EGF1_h_p1p1_p220000exe6", "pero_EGF1_h_p1p1_p220000exe7", "pero_EGF1_h_p1p1_p220000exe8", "pero_EGF1_h_p1p1_p220000exe9", "pero_EGF1_h_p1p1_p2200exe0", "pero_EGF1_h_p1p1_p2200exe1", "pero_EGF1_h_p1p1_p2200exe10", "pero_EGF1_h_p1p1_p2200exe11", "pero_EGF1_h_p1p1_p2200exe12", "pero_EGF1_h_p1p1_p2200exe13", "pero_EGF1_h_p1p1_p2200exe14", "pero_EGF1_h_p1p1_p2200exe15", "pero_EGF1_h_p1p1_p2200exe16", "pero_EGF1_h_p1p1_p2200exe2", "pero_EGF1_h_p1p1_p2200exe3", "pero_EGF1_h_p1p1_p2200exe4", "pero_EGF1_h_p1p1_p2200exe5", "pero_EGF1_h_p1p1_p2200exe6", "pero_EGF1_h_p1p1_p2200exe7", "pero_EGF1_h_p1p1_p2200exe8", "pero_EGF1_h_p1p1_p2200exe9", "pero_EGF1_h_p1p1_p2300exe0", "pero_EGF1_h_p1p1_p2300exe1", "pero_EGF1_h_p1p1_p2300exe10", "pero_EGF1_h_p1p1_p2300exe11", "pero_EGF1_h_p1p1_p2300exe12", "pero_EGF1_h_p1p1_p2300exe13", "pero_EGF1_h_p1p1_p2300exe14", "pero_EGF1_h_p1p1_p2300exe15", "pero_EGF1_h_p1p1_p2300exe16", "pero_EGF1_h_p1p1_p2300exe17", "pero_EGF1_h_p1p1_p2300exe2", "pero_EGF1_h_p1p1_p2300exe3", "pero_EGF1_h_p1p1_p2300exe4", "pero_EGF1_h_p1p1_p2300exe5", "pero_EGF1_h_p1p1_p2300exe6", "pero_EGF1_h_p1p1_p2300exe7", "pero_EGF1_h_p1p1_p2300exe8", "pero_EGF1_h_p1p1_p2300exe9", "pero_EGF1_h_p1p1_p240000exe0", "pero_EGF1_h_p1p1_p240000exe1", "pero_EGF1_h_p1p1_p240000exe10", "pero_EGF1_h_p1p1_p240000exe11", "pero_EGF1_h_p1p1_p240000exe12", "pero_EGF1_h_p1p1_p240000exe13", "pero_EGF1_h_p1p1_p240000exe14", "pero_EGF1_h_p1p1_p240000exe15", "pero_EGF1_h_p1p1_p240000exe16", "pero_EGF1_h_p1p1_p240000exe2", "pero_EGF1_h_p1p1_p240000exe3", "pero_EGF1_h_p1p1_p240000exe4", "pero_EGF1_h_p1p1_p240000exe5", "pero_EGF1_h_p1p1_p240000exe6", "pero_EGF1_h_p1p1_p240000exe7", "pero_EGF1_h_p1p1_p240000exe8", "pero_EGF1_h_p1p1_p240000exe9", "pero_EGF1_h_p1p1_p2400exe0", "pero_EGF1_h_p1p1_p2400exe1", "pero_EGF1_h_p1p1_p2400exe10", "pero_EGF1_h_p1p1_p2400exe11", "pero_EGF1_h_p1p1_p2400exe12", "pero_EGF1_h_p1p1_p2400exe13", "pero_EGF1_h_p1p1_p2400exe14", "pero_EGF1_h_p1p1_p2400exe15", "pero_EGF1_h_p1p1_p2400exe16", "pero_EGF1_h_p1p1_p2400exe2", "pero_EGF1_h_p1p1_p2400exe3", "pero_EGF1_h_p1p1_p2400exe4", "pero_EGF1_h_p1p1_p2400exe5", "pero_EGF1_h_p1p1_p2400exe6", "pero_EGF1_h_p1p1_p2400exe7", "pero_EGF1_h_p1p1_p2400exe8", "pero_EGF1_h_p1p1_p2400exe9", "pero_EGF1_h_p1p1_p2500exe0", "pero_EGF1_h_p1p1_p2500exe1", "pero_EGF1_h_p1p1_p2500exe10", "pero_EGF1_h_p1p1_p2500exe11", "pero_EGF1_h_p1p1_p2500exe12", "pero_EGF1_h_p1p1_p2500exe13", "pero_EGF1_h_p1p1_p2500exe14", "pero_EGF1_h_p1p1_p2500exe15", "pero_EGF1_h_p1p1_p2500exe16", "pero_EGF1_h_p1p1_p2500exe2", "pero_EGF1_h_p1p1_p2500exe3", "pero_EGF1_h_p1p1_p2500exe4", "pero_EGF1_h_p1p1_p2500exe5", "pero_EGF1_h_p1p1_p2500exe6", "pero_EGF1_h_p1p1_p2500exe7", "pero_EGF1_h_p1p1_p2500exe8", "pero_EGF1_h_p1p1_p2500exe9", "pero_EGF1_h_p1p1_p260000exe0", "pero_EGF1_h_p1p1_p260000exe1", "pero_EGF1_h_p1p1_p260000exe10", "pero_EGF1_h_p1p1_p260000exe11", "pero_EGF1_h_p1p1_p260000exe12", "pero_EGF1_h_p1p1_p260000exe13", "pero_EGF1_h_p1p1_p260000exe14", "pero_EGF1_h_p1p1_p260000exe15", "pero_EGF1_h_p1p1_p260000exe16", "pero_EGF1_h_p1p1_p260000exe2", "pero_EGF1_h_p1p1_p260000exe3", "pero_EGF1_h_p1p1_p260000exe4", "pero_EGF1_h_p1p1_p260000exe5", "pero_EGF1_h_p1p1_p260000exe6", "pero_EGF1_h_p1p1_p260000exe7", "pero_EGF1_h_p1p1_p260000exe8", "pero_EGF1_h_p1p1_p260000exe9", "pero_EGF1_h_p1p1_p2600exe0", "pero_EGF1_h_p1p1_p2600exe1", "pero_EGF1_h_p1p1_p2600exe10", "pero_EGF1_h_p1p1_p2600exe11", "pero_EGF1_h_p1p1_p2600exe12", "pero_EGF1_h_p1p1_p2600exe13", "pero_EGF1_h_p1p1_p2600exe14", "pero_EGF1_h_p1p1_p2600exe15", "pero_EGF1_h_p1p1_p2600exe16", "pero_EGF1_h_p1p1_p2600exe2", "pero_EGF1_h_p1p1_p2600exe3", "pero_EGF1_h_p1p1_p2600exe4", "pero_EGF1_h_p1p1_p2600exe5", "pero_EGF1_h_p1p1_p2600exe6", "pero_EGF1_h_p1p1_p2600exe7", "pero_EGF1_h_p1p1_p2600exe8", "pero_EGF1_h_p1p1_p2600exe9", "pero_EGF1_h_p1p1_p2700exe0", "pero_EGF1_h_p1p1_p2700exe1", "pero_EGF1_h_p1p1_p2700exe10", "pero_EGF1_h_p1p1_p2700exe11", "pero_EGF1_h_p1p1_p2700exe12", "pero_EGF1_h_p1p1_p2700exe13", "pero_EGF1_h_p1p1_p2700exe14", "pero_EGF1_h_p1p1_p2700exe15", "pero_EGF1_h_p1p1_p2700exe16", "pero_EGF1_h_p1p1_p2700exe2", "pero_EGF1_h_p1p1_p2700exe3", "pero_EGF1_h_p1p1_p2700exe4", "pero_EGF1_h_p1p1_p2700exe5", "pero_EGF1_h_p1p1_p2700exe6", "pero_EGF1_h_p1p1_p2700exe7", "pero_EGF1_h_p1p1_p2700exe8", "pero_EGF1_h_p1p1_p2700exe9", "pero_EGF1_h_p1p1_p280000exe0", "pero_EGF1_h_p1p1_p280000exe1", "pero_EGF1_h_p1p1_p280000exe10", "pero_EGF1_h_p1p1_p280000exe11", "pero_EGF1_h_p1p1_p280000exe12", "pero_EGF1_h_p1p1_p280000exe13", "pero_EGF1_h_p1p1_p280000exe14", "pero_EGF1_h_p1p1_p280000exe15", "pero_EGF1_h_p1p1_p280000exe16", "pero_EGF1_h_p1p1_p280000exe2", "pero_EGF1_h_p1p1_p280000exe3", "pero_EGF1_h_p1p1_p280000exe4", "pero_EGF1_h_p1p1_p280000exe5", "pero_EGF1_h_p1p1_p280000exe6", "pero_EGF1_h_p1p1_p280000exe7", "pero_EGF1_h_p1p1_p280000exe8", "pero_EGF1_h_p1p1_p280000exe9", "pero_EGF1_h_p1p1_p2800exe0", "pero_EGF1_h_p1p1_p2800exe1", "pero_EGF1_h_p1p1_p2800exe10", "pero_EGF1_h_p1p1_p2800exe11", "pero_EGF1_h_p1p1_p2800exe12", "pero_EGF1_h_p1p1_p2800exe13", "pero_EGF1_h_p1p1_p2800exe14", "pero_EGF1_h_p1p1_p2800exe15", "pero_EGF1_h_p1p1_p2800exe16", "pero_EGF1_h_p1p1_p2800exe2", "pero_EGF1_h_p1p1_p2800exe3", "pero_EGF1_h_p1p1_p2800exe4", "pero_EGF1_h_p1p1_p2800exe5", "pero_EGF1_h_p1p1_p2800exe6", "pero_EGF1_h_p1p1_p2800exe7", "pero_EGF1_h_p1p1_p2800exe8", "pero_EGF1_h_p1p1_p2800exe9", "pero_EGF1_h_p1p1_p2900exe0", "pero_EGF1_h_p1p1_p2900exe1", "pero_EGF1_h_p1p1_p2900exe10", "pero_EGF1_h_p1p1_p2900exe11", "pero_EGF1_h_p1p1_p2900exe12", "pero_EGF1_h_p1p1_p2900exe13", "pero_EGF1_h_p1p1_p2900exe14", "pero_EGF1_h_p1p1_p2900exe15", "pero_EGF1_h_p1p1_p2900exe16", "pero_EGF1_h_p1p1_p2900exe2", "pero_EGF1_h_p1p1_p2900exe3", "pero_EGF1_h_p1p1_p2900exe4", "pero_EGF1_h_p1p1_p2900exe5", "pero_EGF1_h_p1p1_p2900exe6", "pero_EGF1_h_p1p1_p2900exe7", "pero_EGF1_h_p1p1_p2900exe8", "pero_EGF1_h_p1p1_p2900exe9", "pero_EGF1_h_p1p1_p300000exe0", "pero_EGF1_h_p1p1_p300000exe1", "pero_EGF1_h_p1p1_p300000exe10", "pero_EGF1_h_p1p1_p300000exe11", "pero_EGF1_h_p1p1_p300000exe12", "pero_EGF1_h_p1p1_p300000exe13", "pero_EGF1_h_p1p1_p300000exe14", "pero_EGF1_h_p1p1_p300000exe15", "pero_EGF1_h_p1p1_p300000exe16", "pero_EGF1_h_p1p1_p300000exe2", "pero_EGF1_h_p1p1_p300000exe3", "pero_EGF1_h_p1p1_p300000exe4", "pero_EGF1_h_p1p1_p300000exe5", "pero_EGF1_h_p1p1_p300000exe6", "pero_EGF1_h_p1p1_p300000exe7", "pero_EGF1_h_p1p1_p300000exe8", "pero_EGF1_h_p1p1_p300000exe9", "pero_EGF1_h_p1p1_p30000exe0", "pero_EGF1_h_p1p1_p30000exe1", "pero_EGF1_h_p1p1_p30000exe10", "pero_EGF1_h_p1p1_p30000exe11", "pero_EGF1_h_p1p1_p30000exe12", "pero_EGF1_h_p1p1_p30000exe13", "pero_EGF1_h_p1p1_p30000exe14", "pero_EGF1_h_p1p1_p30000exe15", "pero_EGF1_h_p1p1_p30000exe16", "pero_EGF1_h_p1p1_p30000exe2", "pero_EGF1_h_p1p1_p30000exe3", "pero_EGF1_h_p1p1_p30000exe4", "pero_EGF1_h_p1p1_p30000exe5", "pero_EGF1_h_p1p1_p30000exe6", "pero_EGF1_h_p1p1_p30000exe7", "pero_EGF1_h_p1p1_p30000exe8", "pero_EGF1_h_p1p1_p30000exe9", "pero_EGF1_h_p1p1_p3000exe0", "pero_EGF1_h_p1p1_p3000exe1", "pero_EGF1_h_p1p1_p3000exe10", "pero_EGF1_h_p1p1_p3000exe11", "pero_EGF1_h_p1p1_p3000exe12", "pero_EGF1_h_p1p1_p3000exe13", "pero_EGF1_h_p1p1_p3000exe14", "pero_EGF1_h_p1p1_p3000exe15", "pero_EGF1_h_p1p1_p3000exe16", "pero_EGF1_h_p1p1_p3000exe17", "pero_EGF1_h_p1p1_p3000exe2", "pero_EGF1_h_p1p1_p3000exe3", "pero_EGF1_h_p1p1_p3000exe4", "pero_EGF1_h_p1p1_p3000exe5", "pero_EGF1_h_p1p1_p3000exe6", "pero_EGF1_h_p1p1_p3000exe7", "pero_EGF1_h_p1p1_p3000exe8", "pero_EGF1_h_p1p1_p3000exe9", "pero_EGF1_h_p1p1_p300exe0", "pero_EGF1_h_p1p1_p300exe1", "pero_EGF1_h_p1p1_p300exe10", "pero_EGF1_h_p1p1_p300exe11", "pero_EGF1_h_p1p1_p300exe12", "pero_EGF1_h_p1p1_p300exe13", "pero_EGF1_h_p1p1_p300exe14", "pero_EGF1_h_p1p1_p300exe15", "pero_EGF1_h_p1p1_p300exe16", "pero_EGF1_h_p1p1_p300exe2", "pero_EGF1_h_p1p1_p300exe3", "pero_EGF1_h_p1p1_p300exe4", "pero_EGF1_h_p1p1_p300exe5", "pero_EGF1_h_p1p1_p300exe6", "pero_EGF1_h_p1p1_p300exe7", "pero_EGF1_h_p1p1_p300exe8", "pero_EGF1_h_p1p1_p300exe9", "pero_EGF1_h_p1p1_p320000exe0", "pero_EGF1_h_p1p1_p320000exe1", "pero_EGF1_h_p1p1_p320000exe10", "pero_EGF1_h_p1p1_p320000exe11", "pero_EGF1_h_p1p1_p320000exe12", "pero_EGF1_h_p1p1_p320000exe13", "pero_EGF1_h_p1p1_p320000exe14", "pero_EGF1_h_p1p1_p320000exe15", "pero_EGF1_h_p1p1_p320000exe16", "pero_EGF1_h_p1p1_p320000exe2", "pero_EGF1_h_p1p1_p320000exe3", "pero_EGF1_h_p1p1_p320000exe4", "pero_EGF1_h_p1p1_p320000exe5", "pero_EGF1_h_p1p1_p320000exe6", "pero_EGF1_h_p1p1_p320000exe7", "pero_EGF1_h_p1p1_p320000exe8", "pero_EGF1_h_p1p1_p320000exe9", "pero_EGF1_h_p1p1_p340000exe0", "pero_EGF1_h_p1p1_p340000exe1", "pero_EGF1_h_p1p1_p340000exe10", "pero_EGF1_h_p1p1_p340000exe11", "pero_EGF1_h_p1p1_p340000exe12", "pero_EGF1_h_p1p1_p340000exe13", "pero_EGF1_h_p1p1_p340000exe14", "pero_EGF1_h_p1p1_p340000exe15", "pero_EGF1_h_p1p1_p340000exe16", "pero_EGF1_h_p1p1_p340000exe2", "pero_EGF1_h_p1p1_p340000exe3", "pero_EGF1_h_p1p1_p340000exe4", "pero_EGF1_h_p1p1_p340000exe5", "pero_EGF1_h_p1p1_p340000exe6", "pero_EGF1_h_p1p1_p340000exe7", "pero_EGF1_h_p1p1_p340000exe8", "pero_EGF1_h_p1p1_p340000exe9", "pero_EGF1_h_p1p1_p360000exe0", "pero_EGF1_h_p1p1_p360000exe1", "pero_EGF1_h_p1p1_p360000exe10", "pero_EGF1_h_p1p1_p360000exe11", "pero_EGF1_h_p1p1_p360000exe12", "pero_EGF1_h_p1p1_p360000exe13", "pero_EGF1_h_p1p1_p360000exe14", "pero_EGF1_h_p1p1_p360000exe15", "pero_EGF1_h_p1p1_p360000exe16", "pero_EGF1_h_p1p1_p360000exe2", "pero_EGF1_h_p1p1_p360000exe3", "pero_EGF1_h_p1p1_p360000exe4", "pero_EGF1_h_p1p1_p360000exe5", "pero_EGF1_h_p1p1_p360000exe6", "pero_EGF1_h_p1p1_p360000exe7", "pero_EGF1_h_p1p1_p360000exe8", "pero_EGF1_h_p1p1_p360000exe9", "pero_EGF1_h_p1p1_p380000exe0", "pero_EGF1_h_p1p1_p380000exe1", "pero_EGF1_h_p1p1_p380000exe10", "pero_EGF1_h_p1p1_p380000exe11", "pero_EGF1_h_p1p1_p380000exe12", "pero_EGF1_h_p1p1_p380000exe13", "pero_EGF1_h_p1p1_p380000exe14", "pero_EGF1_h_p1p1_p380000exe15", "pero_EGF1_h_p1p1_p380000exe16", "pero_EGF1_h_p1p1_p380000exe2", "pero_EGF1_h_p1p1_p380000exe3", "pero_EGF1_h_p1p1_p380000exe4", "pero_EGF1_h_p1p1_p380000exe5", "pero_EGF1_h_p1p1_p380000exe6", "pero_EGF1_h_p1p1_p380000exe7", "pero_EGF1_h_p1p1_p380000exe8", "pero_EGF1_h_p1p1_p380000exe9", "pero_EGF1_h_p1p1_p400000exe0", "pero_EGF1_h_p1p1_p400000exe1", "pero_EGF1_h_p1p1_p400000exe10", "pero_EGF1_h_p1p1_p400000exe11", "pero_EGF1_h_p1p1_p400000exe12", "pero_EGF1_h_p1p1_p400000exe13", "pero_EGF1_h_p1p1_p400000exe14", "pero_EGF1_h_p1p1_p400000exe15", "pero_EGF1_h_p1p1_p400000exe16", "pero_EGF1_h_p1p1_p400000exe2", "pero_EGF1_h_p1p1_p400000exe3", "pero_EGF1_h_p1p1_p400000exe4", "pero_EGF1_h_p1p1_p400000exe5", "pero_EGF1_h_p1p1_p400000exe6", "pero_EGF1_h_p1p1_p400000exe7", "pero_EGF1_h_p1p1_p400000exe8", "pero_EGF1_h_p1p1_p400000exe9", "pero_EGF1_h_p1p1_p40000exe0", "pero_EGF1_h_p1p1_p40000exe1", "pero_EGF1_h_p1p1_p40000exe10", "pero_EGF1_h_p1p1_p40000exe11", "pero_EGF1_h_p1p1_p40000exe12", "pero_EGF1_h_p1p1_p40000exe13", "pero_EGF1_h_p1p1_p40000exe14", "pero_EGF1_h_p1p1_p40000exe15", "pero_EGF1_h_p1p1_p40000exe16", "pero_EGF1_h_p1p1_p40000exe2", "pero_EGF1_h_p1p1_p40000exe3", "pero_EGF1_h_p1p1_p40000exe4", "pero_EGF1_h_p1p1_p40000exe5", "pero_EGF1_h_p1p1_p40000exe6", "pero_EGF1_h_p1p1_p40000exe7", "pero_EGF1_h_p1p1_p40000exe8", "pero_EGF1_h_p1p1_p40000exe9", "pero_EGF1_h_p1p1_p4000exe0", "pero_EGF1_h_p1p1_p4000exe1", "pero_EGF1_h_p1p1_p4000exe10", "pero_EGF1_h_p1p1_p4000exe11", "pero_EGF1_h_p1p1_p4000exe12", "pero_EGF1_h_p1p1_p4000exe13", "pero_EGF1_h_p1p1_p4000exe14", "pero_EGF1_h_p1p1_p4000exe15", "pero_EGF1_h_p1p1_p4000exe16", "pero_EGF1_h_p1p1_p4000exe2", "pero_EGF1_h_p1p1_p4000exe3", "pero_EGF1_h_p1p1_p4000exe4", "pero_EGF1_h_p1p1_p4000exe5", "pero_EGF1_h_p1p1_p4000exe6", "pero_EGF1_h_p1p1_p4000exe7", "pero_EGF1_h_p1p1_p4000exe8", "pero_EGF1_h_p1p1_p4000exe9", "pero_EGF1_h_p1p1_p400exe0", "pero_EGF1_h_p1p1_p400exe1", "pero_EGF1_h_p1p1_p400exe10", "pero_EGF1_h_p1p1_p400exe11", "pero_EGF1_h_p1p1_p400exe12", "pero_EGF1_h_p1p1_p400exe13", "pero_EGF1_h_p1p1_p400exe14", "pero_EGF1_h_p1p1_p400exe15", "pero_EGF1_h_p1p1_p400exe16", "pero_EGF1_h_p1p1_p400exe2", "pero_EGF1_h_p1p1_p400exe3", "pero_EGF1_h_p1p1_p400exe4", "pero_EGF1_h_p1p1_p400exe5", "pero_EGF1_h_p1p1_p400exe6", "pero_EGF1_h_p1p1_p400exe7", "pero_EGF1_h_p1p1_p400exe8", "pero_EGF1_h_p1p1_p400exe9", "pero_EGF1_h_p1p1_p420000exe0", "pero_EGF1_h_p1p1_p420000exe1", "pero_EGF1_h_p1p1_p420000exe10", "pero_EGF1_h_p1p1_p420000exe11", "pero_EGF1_h_p1p1_p420000exe12", "pero_EGF1_h_p1p1_p420000exe13", "pero_EGF1_h_p1p1_p420000exe14", "pero_EGF1_h_p1p1_p420000exe15", "pero_EGF1_h_p1p1_p420000exe16", "pero_EGF1_h_p1p1_p420000exe2", "pero_EGF1_h_p1p1_p420000exe3", "pero_EGF1_h_p1p1_p420000exe4", "pero_EGF1_h_p1p1_p420000exe5", "pero_EGF1_h_p1p1_p420000exe6", "pero_EGF1_h_p1p1_p420000exe7", "pero_EGF1_h_p1p1_p420000exe8", "pero_EGF1_h_p1p1_p420000exe9", "pero_EGF1_h_p1p1_p440000exe0", "pero_EGF1_h_p1p1_p440000exe1", "pero_EGF1_h_p1p1_p440000exe10", "pero_EGF1_h_p1p1_p440000exe11", "pero_EGF1_h_p1p1_p440000exe12", "pero_EGF1_h_p1p1_p440000exe13", "pero_EGF1_h_p1p1_p440000exe14", "pero_EGF1_h_p1p1_p440000exe15", "pero_EGF1_h_p1p1_p440000exe16", "pero_EGF1_h_p1p1_p440000exe2", "pero_EGF1_h_p1p1_p440000exe3", "pero_EGF1_h_p1p1_p440000exe4", "pero_EGF1_h_p1p1_p440000exe5", "pero_EGF1_h_p1p1_p440000exe6", "pero_EGF1_h_p1p1_p440000exe7", "pero_EGF1_h_p1p1_p440000exe8", "pero_EGF1_h_p1p1_p440000exe9", "pero_EGF1_h_p1p1_p480000exe0", "pero_EGF1_h_p1p1_p480000exe1", "pero_EGF1_h_p1p1_p480000exe10", "pero_EGF1_h_p1p1_p480000exe11", "pero_EGF1_h_p1p1_p480000exe12", "pero_EGF1_h_p1p1_p480000exe13", "pero_EGF1_h_p1p1_p480000exe14", "pero_EGF1_h_p1p1_p480000exe15", "pero_EGF1_h_p1p1_p480000exe16", "pero_EGF1_h_p1p1_p480000exe2", "pero_EGF1_h_p1p1_p480000exe3", "pero_EGF1_h_p1p1_p480000exe4", "pero_EGF1_h_p1p1_p480000exe5", "pero_EGF1_h_p1p1_p480000exe6", "pero_EGF1_h_p1p1_p480000exe7", "pero_EGF1_h_p1p1_p480000exe8", "pero_EGF1_h_p1p1_p480000exe9", "pero_EGF1_h_p1p1_p500000exe0", "pero_EGF1_h_p1p1_p500000exe1", "pero_EGF1_h_p1p1_p500000exe10", "pero_EGF1_h_p1p1_p500000exe11", "pero_EGF1_h_p1p1_p500000exe12", "pero_EGF1_h_p1p1_p500000exe13", "pero_EGF1_h_p1p1_p500000exe14", "pero_EGF1_h_p1p1_p500000exe15", "pero_EGF1_h_p1p1_p500000exe16", "pero_EGF1_h_p1p1_p500000exe2", "pero_EGF1_h_p1p1_p500000exe3", "pero_EGF1_h_p1p1_p500000exe4", "pero_EGF1_h_p1p1_p500000exe5", "pero_EGF1_h_p1p1_p500000exe6", "pero_EGF1_h_p1p1_p500000exe7", "pero_EGF1_h_p1p1_p500000exe8", "pero_EGF1_h_p1p1_p500000exe9", "pero_EGF1_h_p1p1_p50000exe0", "pero_EGF1_h_p1p1_p50000exe1", "pero_EGF1_h_p1p1_p50000exe10", "pero_EGF1_h_p1p1_p50000exe11", "pero_EGF1_h_p1p1_p50000exe12", "pero_EGF1_h_p1p1_p50000exe13", "pero_EGF1_h_p1p1_p50000exe14", "pero_EGF1_h_p1p1_p50000exe15", "pero_EGF1_h_p1p1_p50000exe16", "pero_EGF1_h_p1p1_p50000exe2", "pero_EGF1_h_p1p1_p50000exe3", "pero_EGF1_h_p1p1_p50000exe4", "pero_EGF1_h_p1p1_p50000exe5", "pero_EGF1_h_p1p1_p50000exe6", "pero_EGF1_h_p1p1_p50000exe7", "pero_EGF1_h_p1p1_p50000exe8", "pero_EGF1_h_p1p1_p50000exe9", "pero_EGF1_h_p1p1_p500exe0", "pero_EGF1_h_p1p1_p500exe1", "pero_EGF1_h_p1p1_p500exe10", "pero_EGF1_h_p1p1_p500exe11", "pero_EGF1_h_p1p1_p500exe12", "pero_EGF1_h_p1p1_p500exe13", "pero_EGF1_h_p1p1_p500exe14", "pero_EGF1_h_p1p1_p500exe15", "pero_EGF1_h_p1p1_p500exe16", "pero_EGF1_h_p1p1_p500exe2", "pero_EGF1_h_p1p1_p500exe3", "pero_EGF1_h_p1p1_p500exe4", "pero_EGF1_h_p1p1_p500exe5", "pero_EGF1_h_p1p1_p500exe6", "pero_EGF1_h_p1p1_p500exe7", "pero_EGF1_h_p1p1_p500exe8", "pero_EGF1_h_p1p1_p500exe9", "pero_EGF1_h_p1p1_p60000exe0", "pero_EGF1_h_p1p1_p60000exe1", "pero_EGF1_h_p1p1_p60000exe10", "pero_EGF1_h_p1p1_p60000exe11", "pero_EGF1_h_p1p1_p60000exe12", "pero_EGF1_h_p1p1_p60000exe13", "pero_EGF1_h_p1p1_p60000exe14", "pero_EGF1_h_p1p1_p60000exe15", "pero_EGF1_h_p1p1_p60000exe16", "pero_EGF1_h_p1p1_p60000exe2", "pero_EGF1_h_p1p1_p60000exe3", "pero_EGF1_h_p1p1_p60000exe4", "pero_EGF1_h_p1p1_p60000exe5", "pero_EGF1_h_p1p1_p60000exe6", "pero_EGF1_h_p1p1_p60000exe7", "pero_EGF1_h_p1p1_p60000exe8", "pero_EGF1_h_p1p1_p60000exe9", "pero_EGF1_h_p1p1_p6000exe0", "pero_EGF1_h_p1p1_p6000exe1", "pero_EGF1_h_p1p1_p6000exe10", "pero_EGF1_h_p1p1_p6000exe11", "pero_EGF1_h_p1p1_p6000exe12", "pero_EGF1_h_p1p1_p6000exe13", "pero_EGF1_h_p1p1_p6000exe14", "pero_EGF1_h_p1p1_p6000exe15", "pero_EGF1_h_p1p1_p6000exe16", "pero_EGF1_h_p1p1_p6000exe2", "pero_EGF1_h_p1p1_p6000exe3", "pero_EGF1_h_p1p1_p6000exe4", "pero_EGF1_h_p1p1_p6000exe5", "pero_EGF1_h_p1p1_p6000exe6", "pero_EGF1_h_p1p1_p6000exe7", "pero_EGF1_h_p1p1_p6000exe8", "pero_EGF1_h_p1p1_p6000exe9", "pero_EGF1_h_p1p1_p600exe0", "pero_EGF1_h_p1p1_p600exe1", "pero_EGF1_h_p1p1_p600exe10", "pero_EGF1_h_p1p1_p600exe11", "pero_EGF1_h_p1p1_p600exe12", "pero_EGF1_h_p1p1_p600exe13", "pero_EGF1_h_p1p1_p600exe14", "pero_EGF1_h_p1p1_p600exe15", "pero_EGF1_h_p1p1_p600exe16", "pero_EGF1_h_p1p1_p600exe17", "pero_EGF1_h_p1p1_p600exe2", "pero_EGF1_h_p1p1_p600exe3", "pero_EGF1_h_p1p1_p600exe4", "pero_EGF1_h_p1p1_p600exe5", "pero_EGF1_h_p1p1_p600exe6", "pero_EGF1_h_p1p1_p600exe7", "pero_EGF1_h_p1p1_p600exe8", "pero_EGF1_h_p1p1_p600exe9", "pero_EGF1_h_p1p1_p700exe0", "pero_EGF1_h_p1p1_p700exe1", "pero_EGF1_h_p1p1_p700exe10", "pero_EGF1_h_p1p1_p700exe11", "pero_EGF1_h_p1p1_p700exe12", "pero_EGF1_h_p1p1_p700exe13", "pero_EGF1_h_p1p1_p700exe14", "pero_EGF1_h_p1p1_p700exe15", "pero_EGF1_h_p1p1_p700exe16", "pero_EGF1_h_p1p1_p700exe2", "pero_EGF1_h_p1p1_p700exe3", "pero_EGF1_h_p1p1_p700exe4", "pero_EGF1_h_p1p1_p700exe5", "pero_EGF1_h_p1p1_p700exe6", "pero_EGF1_h_p1p1_p700exe7", "pero_EGF1_h_p1p1_p700exe8", "pero_EGF1_h_p1p1_p700exe9", "pero_EGF1_h_p1p1_p80000exe0", "pero_EGF1_h_p1p1_p80000exe1", "pero_EGF1_h_p1p1_p80000exe10", "pero_EGF1_h_p1p1_p80000exe11", "pero_EGF1_h_p1p1_p80000exe12", "pero_EGF1_h_p1p1_p80000exe13", "pero_EGF1_h_p1p1_p80000exe14", "pero_EGF1_h_p1p1_p80000exe15", "pero_EGF1_h_p1p1_p80000exe16", "pero_EGF1_h_p1p1_p80000exe2", "pero_EGF1_h_p1p1_p80000exe3", "pero_EGF1_h_p1p1_p80000exe4", "pero_EGF1_h_p1p1_p80000exe5", "pero_EGF1_h_p1p1_p80000exe6", "pero_EGF1_h_p1p1_p80000exe7", "pero_EGF1_h_p1p1_p80000exe8", "pero_EGF1_h_p1p1_p80000exe9", "pero_EGF1_h_p1p1_p800exe0", "pero_EGF1_h_p1p1_p800exe1", "pero_EGF1_h_p1p1_p800exe10", "pero_EGF1_h_p1p1_p800exe11", "pero_EGF1_h_p1p1_p800exe12", "pero_EGF1_h_p1p1_p800exe13", "pero_EGF1_h_p1p1_p800exe14", "pero_EGF1_h_p1p1_p800exe15", "pero_EGF1_h_p1p1_p800exe16", "pero_EGF1_h_p1p1_p800exe2", "pero_EGF1_h_p1p1_p800exe3", "pero_EGF1_h_p1p1_p800exe4", "pero_EGF1_h_p1p1_p800exe5", "pero_EGF1_h_p1p1_p800exe6", "pero_EGF1_h_p1p1_p800exe7", "pero_EGF1_h_p1p1_p800exe8", "pero_EGF1_h_p1p1_p800exe9", "pero_EGF1_h_p1p1_p900exe0", "pero_EGF1_h_p1p1_p900exe1", "pero_EGF1_h_p1p1_p900exe10", "pero_EGF1_h_p1p1_p900exe11", "pero_EGF1_h_p1p1_p900exe12", "pero_EGF1_h_p1p1_p900exe13", "pero_EGF1_h_p1p1_p900exe14", "pero_EGF1_h_p1p1_p900exe15", "pero_EGF1_h_p1p1_p900exe16", "pero_EGF1_h_p1p1_p900exe2", "pero_EGF1_h_p1p1_p900exe3", "pero_EGF1_h_p1p1_p900exe4", "pero_EGF1_h_p1p1_p900exe5", "pero_EGF1_h_p1p1_p900exe6", "pero_EGF1_h_p1p1_p900exe7", "pero_EGF1_h_p1p1_p900exe8", "pero_EGF1_h_p1p1_p900exe9"]
  out "Raw Data":dbl[][](graph)
  in  "List of Files":i32(listbox)
  in  "Batch 'em":bool
  in  "Load the batch":bool
  in  "List of Batch Files":i32(listbox)
  in  "Initial Vx":dbl
  in  "Final Vx":dbl
  in  "x rows":dbl
  in  "Initial Vy":dbl
  in  "Final Vy":dbl
  in  "y columns":dbl
  out "X Array (mV)":dbl[](array[numeric])
  out "Y Array (mV)":dbl[](array[numeric])
  in  "File Name":string
  in  "No. of Sets":i32
  in  "No. of Gr":i32
  in  "Flip?":bool
  out "String 2":string
  out "String":string
  out "Averaged Graph":cluster{"Shiftx":dbl[], "first row":dbl[]}(graph)
  in  "Load Sub":bool
  in  "List of Substracted Files":i32(listbox)
  in  "Folder - Substracted":path
  in  "Folder - Averaged":path
  in  "List of Averaged Files":i32(listbox)
  in  "?":bool
  in  "Subtract":bool
  in  "Average":bool
  out "Substracted Graph":cluster{"Value":dbl[], "first row":dbl[]}(graph)
  in  "Folder - TA":path
  in  "TA":bool
  out "Intensity Graph":dbl[][](graph)
  in  "Save Matrix?":bool
  out "3D Scatter":refnum<class "3D Plot Datatype.lvclass">[](xcontrol)
  in  "Time point":u16(ring) items=["-5000", "-500", "-300", "-200", "-100", "0", "100", "200", "300", "400", "500", "600", "700", "800", "900", "1000", "1100", "1200", "1300", "1400", "1500", "1600", "1700", "1800", "1900", "2000", "2100", "2200", "2300", "2400", "2500", "2600", "2700", "2800", "2900", "3000", "4000", "6000", "10000", "20000", "30000", "40000", "50000", "60000", "80000", "100000", "120000", "140000", "160000", "180000", "200000", "220000", "240000", "260000", "280000", "300000", "320000", "340000", "360000", "380000", "400000", "420000", "440000", "480000", "500000"]
  out "3D Surface":refnum<class "3D Plot Datatype.lvclass">[](xcontrol)
  out "Raman Shift":dbl
  in  "Position Number (From 0 to 1328)":i32
  in  "You may begin":bool
  in  "Curve Fitting Time":bool
  in  "Curve Fitting\nOptions":enum32{"Batch", "XY Graphs", "XYZ Graphs"}(tab)
  in  "Batch Options":enum16{""}(ring)
  in  "XY Graph File":path
  in  "X axis":enum32{"shiftx", "times"}(radio)
  in  "Choose":enum32{"Standard Functions", "Custom Functions"}(radio)
  in  "Fitting method":u16(ring) items=["Least Square", "Least Absolute Residual", "Bisquare"]
  in  "Order":i32=2
  in  "Models":T3(radio)
  out "Equation of fit":string
  out "XY Graph":T4(graph)
  in  "Display Precision":i32=3 min=0
  out "Weighted Mean Square Error":dbl format="%#.3g"
  out "error information":string
  out "Fitted Y Values":dbl[](array[numeric]) format="%#.6g"
  in  "XYZ Graph File":path
  out "XYZ Fit Scatter":refnum<class "3D Plot Datatype.lvclass">[](xcontrol)
  in  "Vy Values":u16(ring) items=["0", "0", "0"]
  in  "Vx Values":u16(ring) items=["0", "0", "0"]
  in  "Time Delay":u16(ring) items=["-5000", "-500", "-300", "-200", "-100", "0", "100", "200", "300", "400", "500", "600", "700", "800", "900", "1000", "1100", "1200", "1300", "1400", "1500", "1600", "1700", "1800", "1900", "2000", "2100", "2200", "2300", "2400", "2500", "2600", "2700", "2800", "2900", "3000", "4000", "6000", "10000", "20000", "30000", "40000", "50000", "60000", "80000", "100000", "120000", "140000", "160000", "180000", "200000", "220000", "240000", "260000", "280000", "300000", "320000", "340000", "360000", "380000", "400000", "420000", "440000", "480000", "500000"]
  in  "?":bool
  in  "Time points":T1=[-400.0, -600.0, -200.0, -2100.0, -10.0, 570.0, 1700.0, 980.0, 10000.0, -1100.0, 150.0, 320.0, -850.0, -1500.0, -5000.0]
  in  "Load":bool
  in  "Main Folder":T5
  # "Raster Scan Parameters"
  # "The first 2 distinct features you see are the probe spectrum \nwith the Raman pump on and off.\nThe Raman gain is shown too, but its amplitude is so \nmuch smaller it almost seems like it does not exist."
  # "Currently, this is linked to the Subtracted Folder. You can change it if that's not what you want."
  # "What I want on this page -  An X cross section, An Y cross section\n   I can move cursor to choose time and wavenumber  and checkfit\n\nWant a subset...Make a list of equations and fitting parameters fit wrt to timepoints, + x n y values....then,  plot what was plotted over there."
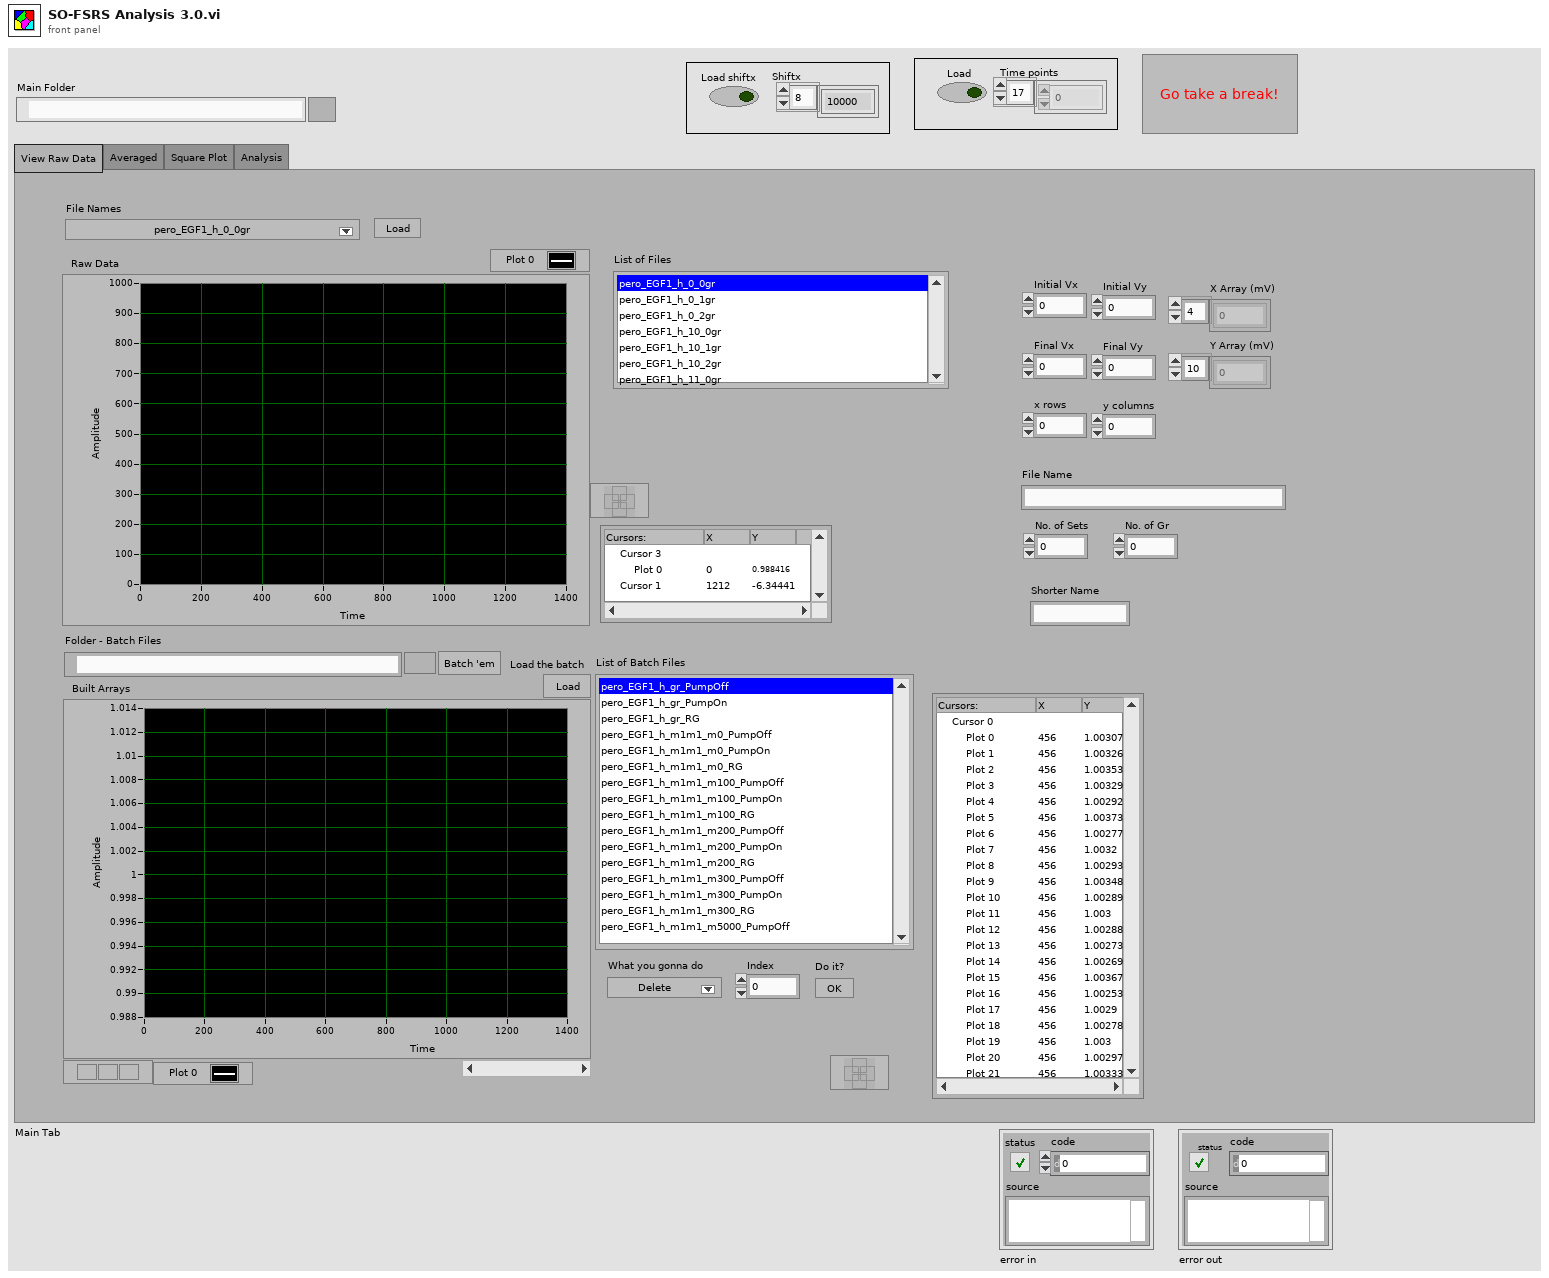
[diagram p1: front panel]
types:
  T1 = typedef "Control 3.ctl" = dbl[]
  T2 = enum32{"View Raw Data", "Averaged", "Square Plot", "Analysis"}
  T3 = enum32{"Linear", "Polynomial", "Exponential", "Power"}
  T4 = cluster{"Data":dbl[], "Best Exponential Fit":dbl[]}[]
  T5 = typedef "Control 1.ctl" = path
  T6 = typedef "NI_Gmath.lvlib/LM model function reference.ctl" = refnum<vi>
  T7 = cluster{"best nonlinear fit":dbl[], "best fit parameters":dbl[]}
  T8 = cluster{"best nonlinear fit":dbl[], "best fit parameters":dbl[]}[]
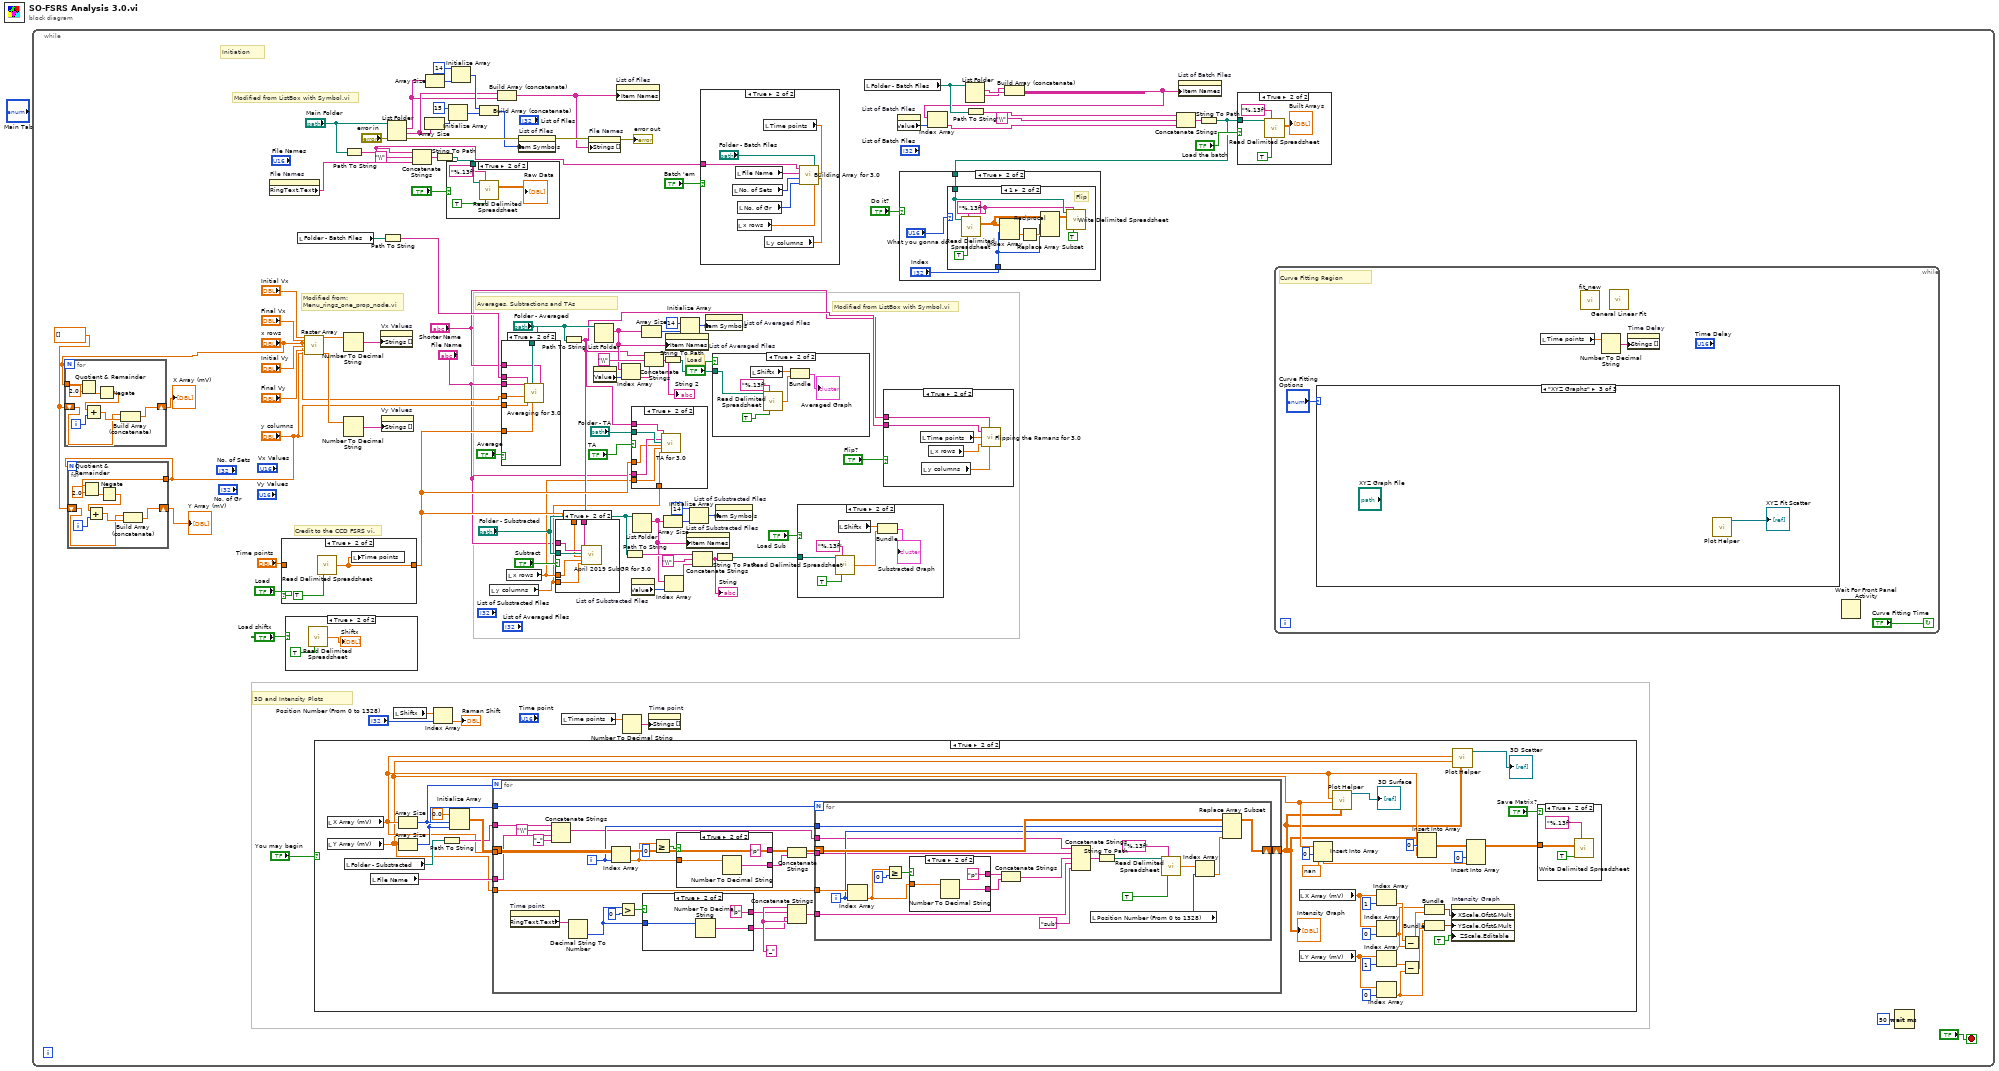
[diagram p0: block diagram]
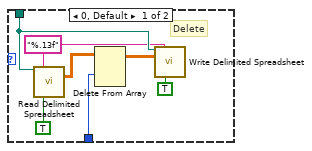
[diagram p5: hidden frame]
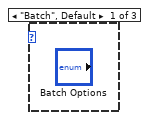
[diagram p9: hidden frame]
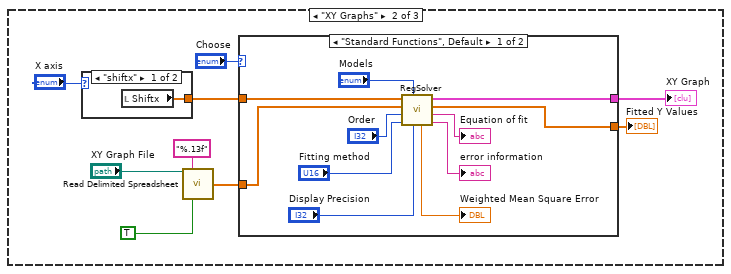
[diagram p10: hidden frame]
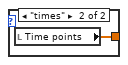
[diagram p11: hidden frame]
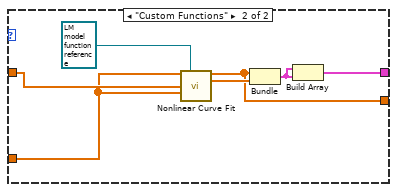
[diagram p12: hidden frame]
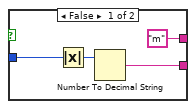
[diagram p15: hidden frame]
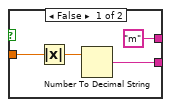
[diagram p16: hidden frame]
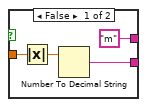
[diagram p17: hidden frame]
diagram:
  n1 = while {
    stop <- "?" stop-if-true
    w4 = dbl[] []
    # "Load"
    # "Initiation"
    # "3D and Intensity Plots"
    # "Averages, Subtractions and TAs"
    # "Modified from:\nMenu_rings_one_prop_node.vi"
    # "Modified from ListBox with Symbol.vi"
    # "Credit to the CCD FSRS vi."
    # "Modified from ListBox with Symbol.vi"
    n2 = for {
      N: "x rows" -> [_]
      tunnel: "x rows" -> [w108]
      shift-right: [w104] -> w5
      shift-left: w4 -> [w103]
      i -> [w106]
      n3 = Quotient & Remainder(x=w108, y=2.0) -> (floor(x/y)=w110:dbl)  [unwired: 1 out]
      n4 = Negate(x=w110) -> (-x=w107:dbl)
      n5 = Add(x=w107, y=w106) -> (x+y=w105:dbl)
      n6 = Build Array (concatenate)(w103, w105) -> (w104:dbl[])
    }
    "X Array (mV)" <- w5
    n7 = for {
      N: "y columns" -> [_]
      shift-right: [w97] -> w3
      shift-left: w4 -> [w96]
      tunnel: "y columns" -> [w95]
      i -> [w99]
      n8 = Quotient & Remainder(x=w95, y=2.0) -> (floor(x/y)=w102:dbl)  [unwired: 1 out]
      n9 = Negate(x=w102) -> (-x=w100:dbl)
      n10 = Add(x=w100, y=w99) -> (x+y=w98:dbl)
      n11 = Build Array (concatenate)(w96, w98) -> (w97:dbl[])
    }
    "Y Array (mV)" <- w3
    n12 = property on="File Names" class="Ring (strict)"() -> ("RingText.Text"=w74:string)  [unwired: 2 in, 2 out]
    n13 = case shown="True" "Load" {
      tunnel: [w324 w325] -> w18
      tunnel: "Time points" -> [w324 _]
      frame False {
      }
      frame True {
        n14 = call-poly <vilib>:"Read Delimited Spreadsheet.vi"("transpose? (F)"=TRUE ("transpose (no:F)")) -> ("first row"=w325:dbl[])  [unwired: 9 in, 5 out]
        n15 = local write "Time points"(w325) -> ()
      }
    }
    n16 = case shown="True" "Load shiftx" {
      frame False {
      }
      frame True {
        n17 = call-poly <vilib>:"Read Delimited Spreadsheet.vi"("transpose? (F)"=TRUE) -> ("first row"=→"Shiftx":dbl[])  [unwired: 9 in, 5 out]
      }
    }
    n18 = local read "Folder - Batch Files"() -> (w21:path)
    n19 = call "Raster Array.vi"("Initial Vx"="Initial Vx", "Final Vx"="Final Vx", "x rows"="x rows", "Initial Vy"="Initial Vy", "Final Vy"="Final Vy", "y columns"="y columns") -> ("X Array"=w17:dbl[], "Y Array"=w9:dbl[])  [unwired: 12 in]
    n20 = case shown="True" "You may begin" {
      frame False {
      }
      frame True {
        n21 = local read "X Array (mV)"() -> (w194:dbl[])
        n22 = local read "Y Array (mV)"() -> (w193:dbl[])
        n23 = local read "Folder - Substracted"() -> (w220:path)
        n24 = local read "File Name"() -> (w218:string)
        n25 = Array Size(array=w194) -> (size(s)=w217:i32)
        n26 = Array Size(array=w193) -> (size(s)=w216:i32)
        n27 = Path To String(path=w220) -> (string=w219:string)
        n28 = Initialize Array(0.0 ("element"), w217, w216) -> (w221:dbl[][])
        n29 = for {
          N: w217 -> [_]
          shift-right: [w250] -> w189
          shift-left: w221 -> [w251]
          tunnel: w194 -> [w247]
          tunnel: w193 -> [w244]
          tunnel: w219 -> [w243]
          tunnel: w218 -> [w242]
          tunnel: w216 -> [w229]
          i -> [w246]
          w235 = "_" ("string")
          n30 = property on="Time point" class="Ring (strict)"() -> ("RingText.Text"=w228:string)  [unwired: 2 in, 2 out]
          n31 = Concatenate Strings(w243, "\\", w242, "_" ("string")) -> (w237:string)
          n32 = Decimal String To Number(string=w228) -> (number=w227:i32)  [unwired: 2 in, 1 out]
          n33 = Index Array(array=w247, index=w246) -> (element=w245:dbl)
          n34 = Greater?(x=w227, y=0) -> (0:w233:bool)
          n35 = case shown="True" w233 {
            tunnel: ["m" "p"] -> w232
            tunnel: w227 -> [w254 w257]
            tunnel: [w252 w256] -> w231
            frame False {
              n36 = Absolute Value(x=w254) -> (abs(x)=w253:i32)
              n37 = Number To Decimal String(number=w253) -> (decimal integer string=w252:string)  [unwired: 1 in]
            }
            frame True {
              n38 = Number To Decimal String(number=w257) -> (decimal integer string=w256:string)  [unwired: 1 in]
            }
          }
          n39 = Greater Or Equal?(x=w245, y=0) -> (x >= y?=w249:bool)
          n40 = case shown="True" w249 {
            tunnel: ["m" "p"] -> w239
            tunnel: w245 -> [w261 w263]
            tunnel: [w259 w264] -> w238
            frame False {
              n41 = Absolute Value(x=w261) -> (abs(x)=w260:dbl)
              n42 = Number To Decimal String(number=w260) -> (decimal integer string=w259:string)  [unwired: 1 in]
            }
            frame True {
              n43 = Number To Decimal String(number=w263) -> (decimal integer string=w264:string)  [unwired: 1 in]
            }
          }
          n44 = Concatenate Strings(w239, w238) -> (w236:string)
          n45 = Concatenate Strings(w235, w232, w231, w235) -> (w230:string)
          n46 = for {
            N: w229 -> [_]
            shift-right: [w286] -> w250
            shift-left: w251 -> [w287]
            tunnel: w246 -> [w285]
            tunnel: w244 -> [w282]
            tunnel: w237 -> [w277]
            tunnel: w236 -> [w276]
            tunnel: w230 -> [w273]
            i -> [w281]
            n47 = Index Array(array=w282, index=w281) -> (element=w280:dbl)
            n48 = Greater Or Equal?(x=w280, y=0) -> (x >= y?=w284:bool)
            n49 = case shown="True" w284 {
              tunnel: ["m" "p"] -> w279
              tunnel: w280 -> [w290 w292]
              tunnel: [w288 w293] -> w278
              frame False {
                n50 = Absolute Value(x=w290) -> (abs(x)=w289:dbl)
                n51 = Number To Decimal String(number=w289) -> (decimal integer string=w288:string)  [unwired: 1 in]
              }
              frame True {
                n52 = Number To Decimal String(number=w292) -> (decimal integer string=w293:string)  [unwired: 1 in]
              }
            }
            n53 = Concatenate Strings(w279, w278) -> (w275:string)
            n54 = Concatenate Strings(w277, w276, w275, w273, "sub" ("string")) -> (w266:string)
            n55 = local read "Position Number (From 0 to 1328)"() -> (w268:i32)
            n56 = String To Path(string=w266) -> (path=w272:path)
            n57 = call-poly <vilib>:"Read Delimited Spreadsheet.vi"("file path (dialog if empty)"=w272, "format (%.3f)"="%.13f", "transpose? (F)"=TRUE) -> ("first row"=w269:dbl[])  [unwired: 7 in, 5 out]
            n58 = Index Array(array=w269, index=w268) -> (element=w267:dbl)
            n59 = Replace Array Subset(array=w287, new element=w267, index (row)=w285, index (col)=w281) -> (w286:dbl[][])
          }
        }
        "Intensity Graph" <- w189
        n60 = local read "X Array (mV)"() -> (w215:dbl[])
        n61 = local read "Y Array (mV)"() -> (w209:dbl[])
        n62 = Insert Into Array(array=w193, index=0, new element=nan ("new element/subarray")) -> (w190:dbl[])
        n63 = call-poly <vilib>:"Plot Helper.vi"("z matrix"=w189, "y vector"=w193, "x vector"=w194) -> ("3D Plot lvclass Array out"=→"3D Surface":refnum<class "3D Plot Datatype.lvclass">[])  [unwired: 3 in, 5 out]
        n64 = Index Array(array=w215, index=1) -> (element=w212:dbl)
        n65 = Index Array(array=w215, index=0) -> (element=w210:dbl)
        n66 = Index Array(array=w209, index=1) -> (element=w205:dbl)
        n67 = Index Array(array=w209, index=0) -> (element=w204:dbl)
        n68 = Subtract(x=w212, y=w210) -> (x-y=w211:dbl)
        n69 = Subtract(x=w205, y=w204) -> (x-y=w206:dbl)
        n70 = Insert Into Array(array=w189, index (row)=0, new element=w194) -> (w198:dbl[][])  [unwired: 1 in]
        n71 = Bundle("Numeric"=w210, w211) -> (w202:cluster{"Numeric":dbl, dbl})  [unwired: 1 in]
        n72 = Bundle("Numeric"=w204, w206) -> (w201:cluster{"Numeric":dbl, dbl})  [unwired: 1 in]
        n73 = property on="Intensity Graph" class="IntGraph (strict)"("XScale.Ofst&Mult"=w202, "YScale.Ofst&Mult"=w201, "ZScale.Editable"=TRUE ("Z Scale.Editable")) -> ()  [unwired: 2 in, 2 out]
        n74 = call-poly <vilib>:"Plot Helper.vi"("z matrix"=w189, "y vector"=w193, "x vector"=w194) -> ("3D Plot lvclass Array out"=→"3D Scatter":refnum<class "3D Plot Datatype.lvclass">[])  [unwired: 3 in, 5 out]
        n75 = Insert Into Array(array=w198, index (col)=0 ("disabled index (col)"), new element=w190) -> (w197:dbl[][])  [unwired: 1 in]
        n76 = case shown="True" "Save Matrix?" {
          tunnel: w197 -> [_ w224]
          frame False {
          }
          frame True {
            n77 = call-poly <vilib>:"Write Delimited Spreadsheet.vi"("format (%.3f)"="%.13f", "2D data"=w224, "transpose? (F)"=TRUE) -> ()  [unwired: 11 in, 2 out]
          }
        }
      }
    }
    n78 = Number To Decimal String(number=w17) -> (decimal integer string=w60:string[])  [unwired: 1 in]
    n79 = Number To Decimal String(number=w9) -> (decimal integer string=w59:string[])  [unwired: 1 in]
    n80 = Path To String(path="Main Folder") -> (string=w41:string)
    n81 = property on="Vx Values" class="Ring (strict)"("Strings []"=w60) -> ()  [unwired: 2 in, 2 out]
    n82 = property on="Vy Values" class="Ring (strict)"("Strings []"=w59) -> ()  [unwired: 2 in, 2 out]
    n83 = Path To String(path=w21) -> (string=w22:string)
    n84 = List Folder(path="Main Folder", error in="error in") -> (filenames=w81:string[], folder names=w85:string[], error out=w89:errorcluster)  [unwired: 2 in, 1 out]
    n85 = local read "Shiftx"() -> (w45:T1)
    n86 = Concatenate Strings(w41, "\\", w74) -> (w79:string)
    n87 = Array Size(array=w85) -> (size(s)=w83:i32)
    n88 = Array Size(array=w81) -> (size(s)=w82:i32)
    n89 = Index Array(array=w45, index="Position Number (From 0 to 1328)") -> (element=→"Raman Shift":dbl)
    n90 = String To Path(string=w79) -> (path=w78:path)
    n91 = case shown="True" "?" {
      tunnel: w78 -> [_ w323]
      frame False {
      }
      frame True {
        n92 = call-poly <vilib>:"Read Delimited Spreadsheet.vi"("file path (dialog if empty)"=w323, "format (%.3f)"="%.13f", "transpose? (F)"=TRUE) -> ("all rows"=→"Raw Data":dbl[][])  [unwired: 7 in, 5 out]
      }
    }
    n93 = Initialize Array(15 ("Numeric"), w83) -> (w87:i32[])
    n94 = Initialize Array(14 ("Numeric 2"), w82) -> (w86:i32[])
    n95 = Build Array (concatenate)(w86, w87) -> (w88:i32[])
    n96 = local read "y columns"() -> (w7:dbl)
    n97 = Build Array (concatenate)(w85, w81) -> (w66:string[])
    n98 = case shown="True" "Average" {
      tunnel: "File Name" -> [_ w319]
      tunnel: w22 -> [_ w318]
      tunnel: w18 -> [_ w316]
      tunnel: "x rows" -> [_ w314]
      tunnel: "y columns" -> [_ w315]
      tunnel: "Folder - Averaged" -> [_ w317]
      tunnel: "Shorter Name" -> [_ w313]
      frame False {
      }
      frame True {
        n99 = call "Averaging for 3.0.vi"("Shorter Name"=w313, "Timepoints"=w316, "Folder to Save"=w317, "number of y"=w315, "number of x"=w314, "Name of File"=w319, "Folder Name"=w318) -> ()
      }
    }
    n100 = local read "x rows"() -> (w8:dbl)
    n101 = property on="List of Files" class="LstBox (strict)"(error in=w89, "Item Symbols"=w88) -> (error out=w76:errorcluster)  [unwired: 1 in, 1 out]
    n102 = local read "Time points"() -> (w48:T1)
    n103 = Path To String(path="Folder - Averaged") -> (string=w13:string)
    n104 = case shown="True" "Subtract" {
      tunnel: "Folder - Substracted" -> [_ w306]
      tunnel: w13 -> [_ w305]
      tunnel: "File Name" -> [_ w304]
      tunnel: w18 -> [_ w303]
      tunnel: w8 -> [_ w302]
      tunnel: w7 -> [_ w301]
      frame False {
      }
      frame True {
        n105 = call "April 2019 SubGR for 3.0.vi"("Folder Name"=w305, "Name of File"=w304, "Folder to Save"=w306, "Timepoints"=w303, "number of x"=w302, "number of y"=w301) -> ()  [unwired: 14 in]
      }
    }
    n106 = property on="File Names" class="Ring (strict)"(error in=w76, "Strings []"=w66) -> (error out=→"error out":errorcluster)  [unwired: 1 in, 1 out]
    n107 = property on="List of Averaged Files" class="LstBox (strict)"() -> ("Value"=w27:i32)  [unwired: 2 in, 2 out]
    n108 = List Folder(path="Folder - Averaged") -> (filenames=w28:string[])  [unwired: 3 in, 3 out]
    n109 = property on="List of Files" class="LstBox (strict)"("Item Names"=w66) -> ()  [unwired: 2 in, 2 out]
    n110 = Index Array(array=w28, index=w27) -> (element=w26:string)
    n111 = Number To Decimal String(number=w48) -> (decimal integer string=w49:string[])  [unwired: 1 in]
    n112 = Path To String(path="Folder - Substracted") -> (string=w52:string)
    n113 = case shown="True" "TA" {
      tunnel: "Folder - TA" -> [_ w121]
      tunnel: "File Name" -> [_ w120]
      tunnel: w13 -> [_ w119]
      tunnel: w18 -> [_ w118]
      tunnel: w8 -> [_ w117]
      tunnel: w7 -> [_ w116]
      frame False {
      }
      frame True {
        n114 = call "TA for 3.0.vi"("Folder Name"=w119, "Name of File"=w120, "Folder to Save"=w121, "Timepoints"=w118, "Vx array"=w117, "Vy array"=w116) -> ()  [unwired: 14 in]
      }
    }
    n115 = property on="List of Substracted Files" class="LstBox (strict)"() -> ("Value"=w25:i32)  [unwired: 2 in, 2 out]
    n116 = List Folder(path="Folder - Substracted") -> (filenames=w24:string[])  [unwired: 3 in, 3 out]
    n117 = Array Size(array=w28) -> (size(s)=w71:i32)
    n118 = Concatenate Strings(w13, "\\", w26) -> (w15:string)
    "String 2" <- w15
    n119 = property on="Time point" class="Ring (strict)"("Strings []"=w49) -> ()  [unwired: 2 in, 2 out]
    n120 = String To Path(string=w15) -> (path=w69:path)
    n121 = Array Size(array=w24) -> (size(s)=w57:i32)
    n122 = Index Array(array=w24, index=w25) -> (element=w23:string)
    n123 = property on="List of Averaged Files" class="LstBox (strict)"("Item Names"=w28) -> ()  [unwired: 2 in, 2 out]
    n124 = Initialize Array(14 ("Numeric 2"), w71) -> (w72:i32[])
    n125 = property on="List of Substracted Files" class="LstBox (strict)"("Item Names"=w24) -> ()  [unwired: 2 in, 2 out]
    n126 = Initialize Array(14 ("Numeric 2"), w57) -> (w55:i32[])
    n127 = Concatenate Strings(w52, "\\", w23) -> (w14:string)
    "String" <- w14
    n128 = case shown="True" "Batch 'em" {
      tunnel: w41 -> [_ w152]
      frame False {
      }
      frame True {
        n129 = local read "No. of Sets"() -> (w146:i32)
        n130 = local read "File Name"() -> (w151:string)
        n131 = local read "x rows"() -> (w147:dbl)
        n132 = local read "No. of Gr"() -> (w145:i32)
        n133 = local read "Time points"() -> (w149:T1)
        n134 = local read "y columns"() -> (w148:dbl)
        n135 = call "Building Array for 3.0.vi"("Number of y"=w147, "Number of x"=w148, "Timepoints"=w149, "Folder to Save"="Folder - Batch Files", "No. of Gr"=w145, "No. of Sets"=w146, "Name of File"=w151, "Folder Name"=w152) -> ()
      }
    }
    n136 = property on="List of Averaged Files" class="LstBox (strict)"("Item Symbols"=w72) -> ()  [unwired: 2 in, 2 out]
    n137 = case shown="True" "?" {
      tunnel: w69 -> [_ w312]
      frame False {
      }
      frame True {
        n138 = local read "Shiftx"() -> (w308:T1)
        n139 = call-poly <vilib>:"Read Delimited Spreadsheet.vi"("file path (dialog if empty)"=w312, "format (%.3f)"="%.13f", "transpose? (F)"=TRUE) -> ("first row"=w307:dbl[])  [unwired: 7 in, 5 out]
        n140 = Bundle("Shiftx"=w308, "first row"=w307) -> (→"Averaged Graph":cluster{"Shiftx":T1, "first row":dbl[]})  [unwired: 1 in]
      }
    }
    n141 = String To Path(string=w14) -> (path=w44:path)
    n142 = property on="List of Substracted Files" class="LstBox (strict)"("Item Symbols"=w55) -> ()  [unwired: 2 in, 2 out]
    n143 = case shown="True" "Load Sub" {
      tunnel: w44 -> [_ w300]
      frame False {
      }
      frame True {
        n144 = call-poly <vilib>:"Read Delimited Spreadsheet.vi"("file path (dialog if empty)"=w300, "format (%.3f)"="%.13f", "transpose? (F)"=TRUE) -> ("first row"=w297:dbl[])  [unwired: 7 in, 5 out]
        n145 = local read "Shiftx"() -> (w295:T1)
        n146 = Bundle("Shiftx"=w295, "first row"=w297) -> (→"Substracted Graph":cluster{"Shiftx":T1, "first row":dbl[]})  [unwired: 1 in]
      }
    }
    n147 = local read "Folder - Batch Files"() -> (w38:path)
    n148 = case shown="True" "Flip?" {
      tunnel: w13 -> [_ w115]
      tunnel: "Shorter Name" -> [_ w114]
      frame False {
      }
      frame True {
        n149 = local read "Time points"() -> (w113:T1)
        n150 = local read "y columns"() -> (w111:dbl)
        n151 = local read "x rows"() -> (w112:dbl)
        n152 = call "Flipping the Ramans for 3.0.vi"("Folder Name"=w115, "Name of File"=w114, "Timepoints"=w113, "Vx array"=w112, "Vy array"=w111) -> ()  [unwired: 1 in]
      }
    }
    n153 = property on="List of Batch Files" class="LstBox (strict)"() -> ("Value"=w31:i32)  [unwired: 2 in, 2 out]
    n154 = List Folder(path=w38) -> (filenames=w34:string[], folder names=w10:string[])  [unwired: 3 in, 2 out]
    n155 = Path To String(path=w38) -> (string=w37:string)
    n156 = Build Array (concatenate)(w10, w34) -> (w30:string[])
    n157 = Index Array(array=w30, index=w31) -> (element=w29:string)
    n158 = Concatenate Strings(w37, "\\", w29) -> (w35:string)
    n159 = property on="List of Batch Files" class="LstBox (strict)"("Item Names"=w30) -> ()  [unwired: 2 in, 2 out]
    n160 = String To Path(string=w35) -> (path=w32:path)
    n161 = case shown="True" "Do it?" {
      tunnel: w32 -> [_ w123]
      frame False {
      }
      frame True {
        n162 = case shown="1" "What you gonna do" {
          tunnel: w123 -> [w127 w133]
          tunnel: "Index" -> [w129 w136]
          frame 0, Default {
            w126 = "%.13f" ("format (%.3f)")
            # "Delete"
            n163 = call-poly <vilib>:"Read Delimited Spreadsheet.vi"("file path (dialog if empty)"=w127, "format (%.3f)"=w126, "transpose? (F)"=TRUE) -> ("all rows"=w130:dbl[][])  [unwired: 7 in, 5 out]
            n164 = Delete From Array(array=w130, index (row)=w129) -> (array with subset deleted=w128:dbl[][])  [unwired: 2 in, 1 out]
            n165 = call-poly <vilib>:"Write Delimited Spreadsheet.vi"("file path (dialog if empty)"=w127, "format (%.3f)"=w126, "2D data"=w128, "transpose? (F)"=TRUE) -> ()  [unwired: 10 in, 2 out]
          }
          frame 1 {
            w132 = "%.13f" ("format (%.3f)")
            # "Flip"
            n166 = call-poly <vilib>:"Read Delimited Spreadsheet.vi"("file path (dialog if empty)"=w133, "format (%.3f)"=w132, "transpose? (F)"=TRUE) -> ("all rows"=w138:dbl[][])  [unwired: 7 in, 5 out]
            n167 = Index Array(array=w138, index (row)=w136) -> (element=w139:dbl[])  [unwired: 1 in]
            n168 = Reciprocal(x=w139) -> (1/x=w137:dbl[])
            n169 = Replace Array Subset(array=w138, new element=w137, index (row)=w136) -> (w134:dbl[][])  [unwired: 1 in]
            n170 = call-poly <vilib>:"Write Delimited Spreadsheet.vi"("file path (dialog if empty)"=w133, "format (%.3f)"=w132, "2D data"=w134, "transpose? (F)"=TRUE) -> ()  [unwired: 10 in, 2 out]
          }
        }
      }
    }
    n171 = case shown="True" "Load the batch" {
      tunnel: w32 -> [_ w141]
      frame False {
      }
      frame True {
        n172 = call-poly <vilib>:"Read Delimited Spreadsheet.vi"("file path (dialog if empty)"=w141, "format (%.3f)"="%.13f", "transpose? (F)"=TRUE) -> ("all rows"=→"Built Arrays":dbl[][])  [unwired: 7 in, 5 out]
      }
    }
    n173 = while {
      stop <- "Curve Fitting Time" continue-if-true
      # "Curve Fitting Region"
      n174 = case shown="\"XYZ Graphs\"" "Curve Fitting\nOptions" {
        frame "Batch", Default {
        }
        frame "XY Graphs" {
          n175 = case shown="\"shiftx\"" "X axis" {
            tunnel: [w168 w169] -> w162
            frame "shiftx" {
              n176 = local read "Shiftx"() -> (w168:T1)
            }
            frame "times" {
              n177 = local read "Time points"() -> (w169:T1)
            }
          }
          n178 = call-poly <vilib>:"Read Delimited Spreadsheet.vi"("file path (dialog if empty)"="XY Graph File", "format (%.3f)"="%.13f", "transpose? (F)"=TRUE) -> ("first row"=w164:dbl[])  [unwired: 7 in, 5 out]
          n179 = case shown="\"Standard Functions\", Default" "Choose" {
            tunnel: [w174 w186] -> w160
            tunnel: [w173 w185] -> w161
            tunnel: w164 -> [w171 w181]
            tunnel: w162 -> [w170 w184]
            frame "Standard Functions", Default {
              n180 = call "RegSolver.vi"("Display Precision"="Display Precision", "Models"="Models", "Fitting method"="Fitting method", "Order"="Order", "Y Data"=w171, "X Data"=w170) -> ("error information"=→"error information":string, "Equation of fit"=→"Equation of fit":string, "Fitted Data"=w173:dbl[], "XY Graph"=w174:T4, "MSE"=→"Weighted Mean Square Error":dbl)  [unwired: 1 in]
            }
            frame "Custom Functions" {
              n181 = call-poly <vilib>:"Nonlinear Curve Fit.vi"("Y"=w181, "f(x,a)"=T6 refnum, "Weight"=w184, "initial parameters"=w181) -> ("best nonlinear fit"=w185:dbl[], "best fit parameters"=w187:dbl[])  [unwired: 6 in, 4 out]
              n182 = Bundle("best nonlinear fit"=w185, "best fit parameters"=w187) -> (w183:T7)  [unwired: 1 in]
              n183 = Build Array(w183, w183) -> (w186:T8)
            }
          }
          "Fitted Y Values" <- w161
          "XY Graph" <- w160
        }
        frame "XYZ Graphs" {
          n184 = call-poly <vilib>:"Plot Helper.vi"() -> ("3D Plot lvclass Array out"=→"XYZ Fit Scatter":refnum<class "3D Plot Datatype.lvclass">[])  [unwired: 6 in, 5 out]
        }
      }
      n185 = local read "Time points"() -> (w157:T1)
      n186 = call "fit_new.vi"() -> ()  [unwired: 10 in, 2 out]
      n187 = Number To Decimal String(number=w157) -> (decimal integer string=w158:string[])  [unwired: 1 in]
      n188 = call <vilib>:"General Linear Fit.vi"() -> ()  [unwired: 10 in, 6 out]
      n189 = property on="Time Delay" class="Ring (strict)"("Strings []"=w158) -> ()  [unwired: 2 in, 2 out]
      n190 = Wait For Front Panel Activity() -> ()  [unwired: 3 in, 1 out]
    }
    n191 = Wait (ms)(milliseconds to wait=u32 50) -> ()  [unwired: 1 out]
  }
